vi "main4Ch_GainAtSameTime.vi"() -> ()   [LabVIEW 2024]
doc: "Main VI for FLS imaging system."
uses:
  <userlib>/_OpenG.lib/file/file.llb/openg_file.lvlib
  <vilib>/event_ctls.llb/usereventprio.ctl
  <instrlib>/niScope/Acquire/Fetch/niScope Multi Fetch Binary 16.vi
  <instrlib>/niScope/Controls/niScope trigger source.ctl
  <userlib>/_OpenG.lib/time/time.llb/openg_time.lvlib
  LaguerreDeconLib/DeconEngineClass/LaguerreDeconEngineClass.lvclass
  SubVI/GlobalVariables.vi
  SubVI/LabJack/LJ Pin Setting.ctl
  <vilib>/Utility/error.llb/DialogType.ctl
  <vilib>/Analysis/NI_AALBase.lvlib
  <vilib>/Utility/miscctls.llb/LVMinMaxIncTypeDef.ctl
  <vilib>/Analysis/baseanly.llb/Mean (DBL).vi
  <vilib>/Utility/miscctls.llb/LVPointTypeDef.ctl
  SubVI/APD/APDClass.lvclass
  ConfigFiles/AimingBeamVideoConfig.ctl
  <vilib>/addons/control/pid/NI_PID_pid.lvlib
  <vilib>/addons/control/pid/pid.llb/PID (DBL).vi
  <vilib>/Instr/_visa.llb/VISA Configure Serial Port (Instr).vi
  SubVI/DigitizerConfiguration/FLImDAQ.ctl
panel:
  out "Record Backlog 2":i32
  in  "Auto gain ch4":bool=TRUE caption="Auto gain ch3"
  in  "V 4":dbl caption="Gain 3" min=0.0 max=4.66 step=0.1
  out "Gain4":dbl
  out "Lifetime 4":dbl caption="Lifetime 3"
  out "IntR4":dbl format="%#_2g"
  out "SNR4":dbl format="%#_3g"
  out "Channel 4":dbl[][](graph) caption="Channel 3"
  out "RunStartTime":u32
  out "Dig1 Temp":dbl
  out "Dig2 Temp":dbl
  out "Visualization PC video source":T1
  in  "V target(1.0)":dbl=1.0 caption="V target(1.5)" min=0.3 max=1.5 step=0.1 format="%#_4g"
  out "SNR3":dbl format="%#_3g"
  out "SNR2":dbl format="%#_3g"
  out "SNR1":dbl format="%#_3g"
  in  "Show BG removed?":bool=TRUE
  out "IntR3":dbl format="%#_2g"
  out "IntR2":dbl format="%#_2g"
  out "IntR1":dbl format="%#_2g"
  in  "Video Display":bool
  out "Gain3":dbl
  out "Gain2":dbl
  out "Gain1":dbl
  in  "Skip Data Save?":bool
  out "Aq Loop?":bool
  out "ML?":bool
  out "aquisition loop Error Out":errorcluster
  out "Laser f (Hz)":dbl
  out "Record Backlog":i32
  out "Fetch Record #":i32
  out "Sync Success?":bool
  out "Disclamer":picture
  out "Calibration #":i8
  out "BG #":i8
  in  "TCP Connect":bool
  out "Help":string
  in  "355nm Laser toggle":bool caption="355nm 460Hz"
  in  "Cali&iRF alignment":bool
  in  "Background":bool
  in  "Aiming beam toggle":bool caption="445nm 15Hz 20mA"
  out "Lifetime 3":dbl
  out "Lifetime 2":dbl
  in  "Auto gain ch3":bool=TRUE
  in  "Auto gain ch2":bool=TRUE
  in  "Auto gain ch1":bool=TRUE
  out "Run #":i8
  in  "StopButton":bool caption="Stop"
  out "Aquisition Status:":bool
  in  "StartButton":bool caption="Start"
  in  "V 3":dbl caption="Gain 3" min=0.0 max=4.65 step=0.1
  in  "V 2":dbl caption="Gain 2" min=0.0 max=4.59 step=0.1
  out "Lifetime 1":dbl
  in  "V 1":dbl caption="Gain 1" min=0.0 max=4.63 step=0.1 format="%#_4g"
  in  "Video Source":enum32{"Camera", "FrameGrabber"}(radio)
  out "Case #":string
  out "System Hardware Connection Status":T2
  out "Channel 3":dbl[][](graph)
  out "Channel 2":dbl[][](graph)
  out "Channel 1":dbl[][](graph)
  in  "Tab Control":T3(tab)
  out "display loop timing(ms)":u32
  out "Aquisition loop timing(ms)":u32 format="%.2f"
  out "DisplayLoop":i32
  out "PID loop":i32 caption="processing loop"
  out "PID loop timing(ms)":u32 caption="processing loop timing(ms)"
  out "Communication loop(ms)":u32
  out "laser EM lamp V":dbl format="%0.6f"
  out "Decon Loop timing (ms)":dbl
  out "Auisition Loop idx":i32
  out "LJ process (ms)":u32
  out "LJ time(ms)":u32[](array[numeric])
  in  "Show BG":bool
  out "iRF length":i32
  out "BG length":i32
  out "data length":i32
  out "SysConfigCluster":T4
  out "LJ Pinout":T5={"Ch1 Bias"="DAC0", "Ch2 Bias"="DAC1", "Ch3 Bias"="DAC2", "Ch4 Bias"="DAC0", "355 PWM"="FIO0", "AimingBeam PWM"="FIO2", "Laser Ready"="FIO3", "Interlock"="FIO1", "Laser Start/Stop"="FIO1", "Red LED"="FIO1", "Green LED"="DIO3", "Foot Pedal"="DIO15"}
  out "FLImDAQ":T6={"Digitizer 1"="", "Digitizer 2"="", "Channel"=enum."Channel 0", "trigger source"="VAL_EXTERNAL", "trigger level"=0.5, "trigger delay"=1.35e-07, "min sample rate"=12500000000.0, "min record length"=2500, "vertical range"=1.0, "vertical offset"=-0.25, "Waveform to Avg"=2000} caption="FLIm DAQ Configuration" {"trigger delay" format="%^#.4e"; "trigger level" min=0.0 max=3.5 step=0.5 format="%.2f"; "vertical offset" format="%.4f"; "vertical range" format="%.2f"; "min sample rate" format="%#.2p"}
  in  "Sys Reconfig":bool
  out "data out(communcation loop)":string
  out "PID loop error out":errorcluster caption="processing Error Out"
  out "decon error out":errorcluster
  out "Laser Rep Rate":dbl
  out "V4 Size":i32 caption="V3 Size"
  in  "Data Class":enum16{"Data", "BG", "Cali"}(ring)
  out "V1 Size":i32
  out "V2 Size":i32
  out "V3 Size":i32
  out "data Size":i32[](array[numeric])
  out "State log":string
  in  "Ch4 PID gains":T8={"proportional gain (Kc)"=30.0, "integral time (Ti, min)"=0.0003, "derivative time (Td, min)"=1e-05}
  in  "Ch3 PID gains":T8={"proportional gain (Kc)"=30.0, "integral time (Ti, min)"=0.0003, "derivative time (Td, min)"=1e-05}
  in  "Ch2 PID gains":T8={"proportional gain (Kc)"=30.0, "integral time (Ti, min)"=0.0003, "derivative time (Td, min)"=1e-05}
  in  "Ch1 PID gains":T8={"proportional gain (Kc)"=30.0, "integral time (Ti, min)"=0.0003, "derivative time (Td, min)"=1e-05}
  in  "Quit":bool
  in  "Radio Buttons":T9(radio)=enum."Ch2" caption="DeCon Chan"
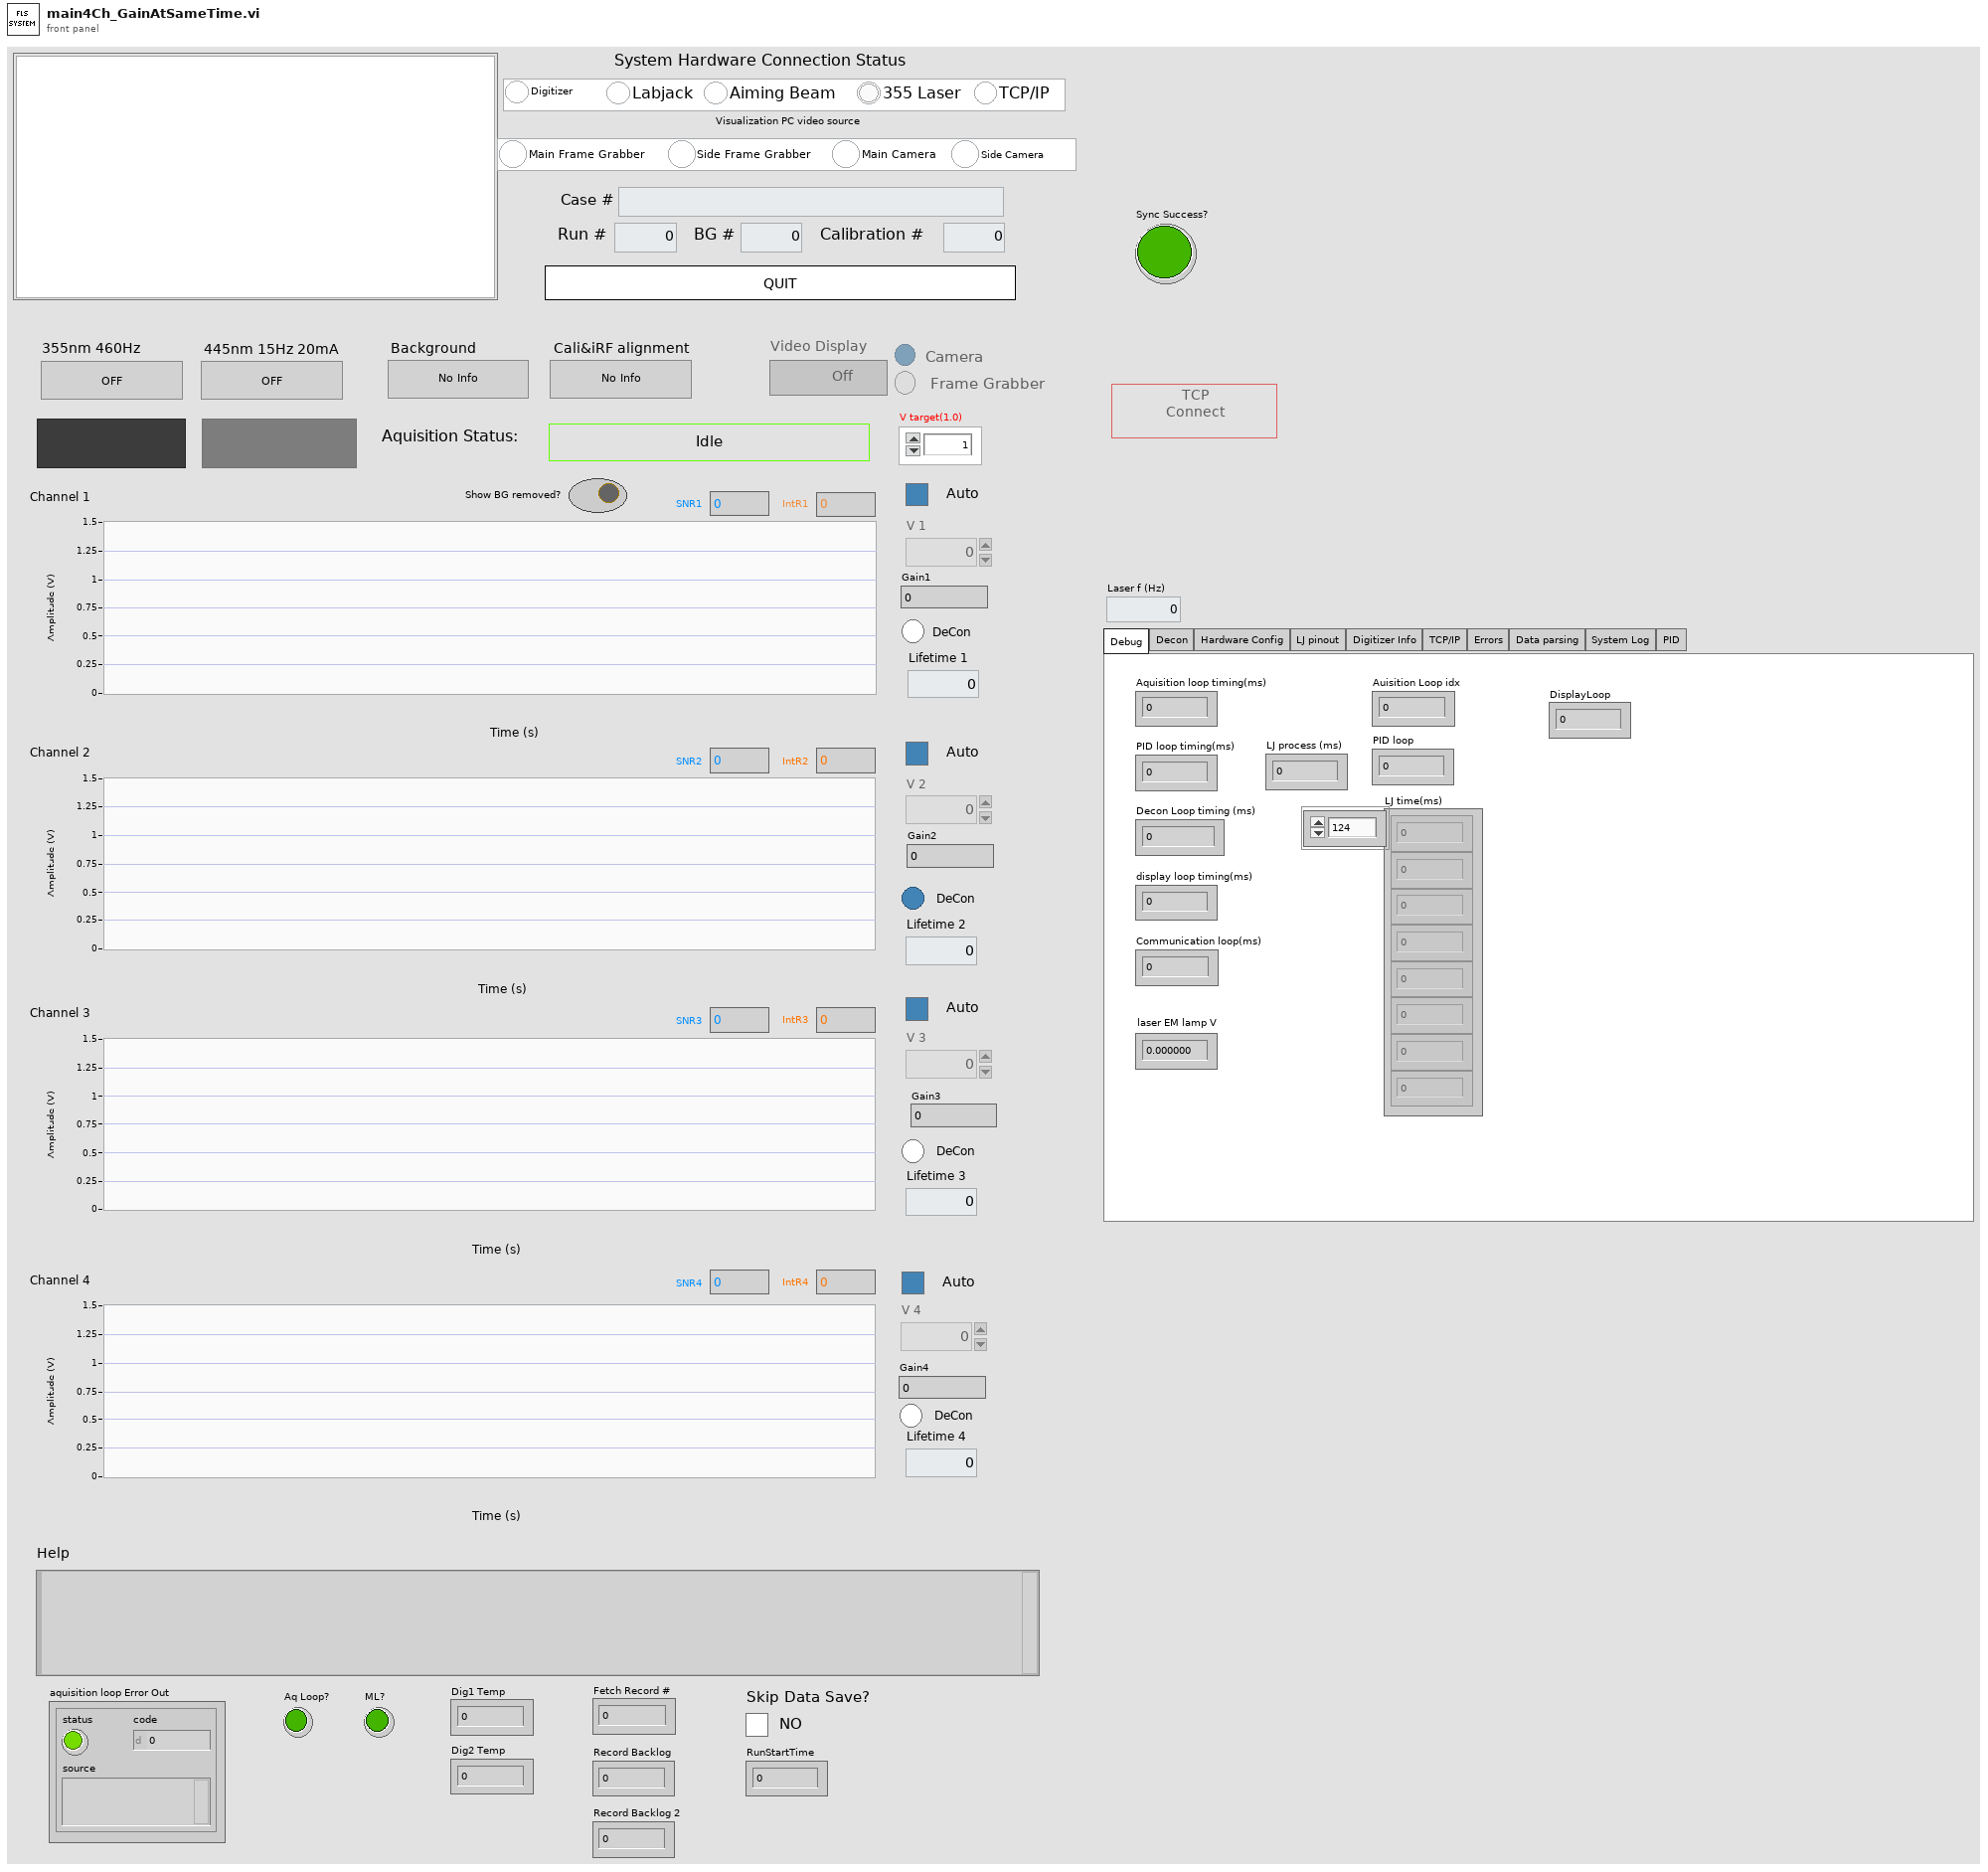
[diagram p1: front panel]
types:
  T1 = cluster{"Main Frame Grabber":bool, "Side Frame Grabber":bool, "Main Camera":bool, "Side Camera":bool}
  T2 = cluster{"Digitizer":bool, "Labjack":bool, "Aiming Beam":bool, "355 Laser":bool, "TCP/IP":bool}
  T3 = enum32{"Debug", "Decon", "Hardware Config", "LJ pinout", "Digitizer Info", "TCP/IP", "Errors", "Data parsing", "System Log", "PID"}
  T4 = cluster{"Ch1Enable?":bool, "Ch2Enable?":bool, "Ch3Enable?":bool, "Ch1AutoGain?":bool, "Ch2AutoGain?":bool, "Ch3AutoGain?":bool, "AimingBeamEnable?":bool}
  T5 = typedef "LJ Pin Setting.ctl" = cluster{"Ch1 Bias":string, "Ch2 Bias":string, "Ch3 Bias":string, "Ch4 Bias":string, "355 PWM":string, "AimingBeam PWM":string, "Laser Ready":string, "Interlock":string, "Laser Start/Stop":string, "Red LED":string, "Green LED":string, "Foot Pedal":string}
  T6 = typedef "FLImDAQ.ctl" = cluster{"Digitizer 1":refnum<k15>, "Digitizer 2":refnum<k15>, "Channel":enum16{"Channel 0", "Channel 1", "Channel 0&1"}, "trigger source":T7, "trigger level":dbl, "trigger delay":dbl, "min sample rate":dbl, "min record length":i32, "vertical range":dbl, "vertical offset":dbl, "Waveform to Avg":i16}
  T7 = typedef "niScope trigger source.ctl" = string
  T8 = cluster{"proportional gain (Kc)":dbl, "integral time (Ti, min)":dbl, "derivative time (Td, min)":dbl}
  T9 = enum32{"No Selection", "Ch1", "Ch2", "Ch3", "Ch4"}
  T10 = cluster{"remote start event":refnum<user-event>, "remote stop  event":refnum<user-event>}
  T11 = enum8{"Enabled", "Disabled", "Disabled and Grayed Out"}
  T12 = enum16{"open", "replace", "create", "open or create", "replace or create", "replace or create with confirmation"}
  T13 = cluster{"CH1":dbl[][], "CH2":dbl[][], "CH3":dbl[][], "CH4":dbl[][], "Gain cluster":cluster{"V1":dbl, "V2":dbl, "V3":dbl, "V4":dbl}}
  T14 = cluster{"idx":i32, "CH1&2":dbl[][], "CH3":dbl[][], "V cluster":cluster{"V1":dbl, "V2":dbl, "V3":dbl, "V4":dbl}}
  T15 = cluster{"Ch1 iRF":dbl[], "Ch2 iRF":dbl[], "Ch3 iRF":dbl[], "Ch4 iRF":dbl[]}
  T16 = enum16{"open", "open or create", "create or replace", "create", "open (read-only)"}
  T17 = enum32{"Invalid", "Standard", "Closed", "Hidden", "Minimized", "Maximized"}
  T18 = enum32{"invalid app kind", "Development System", "Run Time System", "Student Edition", "Embedded LabVIEW", "Evaluation", "Custom"}
  T19 = typedef "usereventprio.ctl" = enum32{"high priority", "normal priority"}
  T20 = enum32{"Bad", "Idle", "Run top level", "Running"}
  T21 = enum16{"Standard", "Buffered", "CRLF", "Immediate"}
  T22 = typedef "AimingBeamVideoConfig.ctl" = cluster{"DeCon Channel":enum16{"1", "2", "3"}, "Scale Bar":bool, "Scale Low":dbl, "Scale High":dbl, "ANSI":dbl, "Radius":dbl, "3D?":bool, "Firefly?":bool, "Pentero?":bool}
  T23 = cluster{"Core":cluster{"Current VI Reference":refnum<vi>, "Close Panel on Exit?":bool}, "SysConfigCluster":cluster{"Ch1Enable?":bool, "Ch2Enable?":bool, "Ch3Enable?":bool, "Ch1AutoGain?":bool, "Ch2AutoGain?":bool, "Ch3AutoGain?":bool, "AimingBeamEnable?":bool}, "System Status":cluster{"Digitizer":bool, "Labjack":bool, "Aiming Beam":bool, "355 Laser":bool, "TCP/IP":bool}, "IDs":cluster{"RunID":i8, "BG ID":i8, "Cali ID":i8}, "CaseID":string, "DefaultPath":path, "Pathes":cluster{"DataPath":path, "BG Path":path, "iRFPath":path, "CaliPath":path}, "FLImDAQ":cluster{"resource name":refnum<k15>, "resource name 2":refnum<k15>, "Channel":enum16{"Channel 0", "Channel 1", "Channel 0&1"}, "trigger source":T7, "trigger level":dbl, "trigger delay":dbl, "min sample rate":dbl, "min record length":i32, "vertical range":dbl, "vertical offset":dbl, "Waveform to Avg":i32}, "SysRunning?":bool, "AB Cluster":cluster{"Aiming Beam COM Port":refnum<visa-resource-name>, "Min Current":dbl, "Max Current":dbl, "Default Current":dbl, "Freq":i32}, "LJ Pinout":T5, "355 PWM setting":cluster{"DIO_EF_CLOCK1_DIVISOR":i16, "DIO_EF_CLOCK1_ROLL_VALUE":i32, "DIO#_EF_INDEX":i16, "DIO#_EF_OPTIONS":i16, "DIO#_EF_CONFIG_A":i32}, "AB PWM setting":cluster{"DIO_EF_CLOCK1_DIVISOR":i16, "DIO_EF_CLOCK1_ROLL_VALUE":i32, "DIO#_EF_INDEX":i16, "DIO#_EF_OPTIONS":i16, "DIO#_EF_CONFIG_A":i32}, "Last Trigger":u32, "niTClk sessions":refnum<k20>[], "Laser start tic":u32, "TCP attempt count":i32, "Ch1Data":dbl[][], "Ch2Data":dbl[][], "Ch3Data":dbl[][], "Ch4Data":dbl[][], "V1":dbl[], "V2":dbl[], "V3":dbl[], "V4":dbl[], "SlowTimer":u32, "FastTimer":u32, "listener ID":refnum<k5>, "TempPath":path, "CaliPath":path, "LED vi reference":refnum<vi>, "Aquisition Timer":u32, "APDSerialNum":cluster{"Ch1APDSerial#":string, "Ch2APDSerial#":string, "Ch3APDSerial#":string, "Ch4APDSerial#":string}, "VideoConfig":T22, "LED vi ref open?":bool, "video source":cluster{"Main Frame Grabber":bool, "Side Frame Grabber":bool, "Main Camera":bool, "Side Camera":bool}, "bothVidSourceAvail":bool}
  T24 = typedef "LVCursorListTypeDef.ctl" = cluster{"Name":string, "Color":u32, "Style":u8, "Point Style":u8, "Name Visible":bool, "Allow Drag":bool, "Cursor Mode":u32, "Plot":i32, "Index":i32, "Position":cluster{"X":dbl, "Y":dbl}, "X Scale":u32, "Y Scale":u32, "Watch Plots":i32[], "Watch All Plots":bool, "Plot Area":i32, "Label Offset":cluster{"X":dbl, "Y":dbl}}[]
  T25 = cluster{"Name":string, "Color":u32, "Style":u8, "Point Style":u8, "Name Visible":bool, "Allow Drag":bool, "Cursor Mode":u32, "Plot":i32, "Index":i32, "Position":cluster{"X":dbl, "Y":dbl}, "X Scale":u32, "Y Scale":u32, "Watch Plots":i32[], "Watch All Plots":bool, "Plot Area":i32, "Label Offset":cluster{"X":dbl, "Y":dbl}}
  T26 = cluster{"Ch1APDSerial#":string, "Ch2APDSerial#":string, "Ch3APDSerial#":string, "Ch4APDSerial#":string}
  T27 = cluster{"DataPath":path, "BG Path":path, "iRFPath":path, "CaliPath":path}
  T28 = cluster{"DIO_EF_CLOCK1_DIVISOR":i16, "DIO_EF_CLOCK1_ROLL_VALUE":i32, "DIO#_EF_INDEX":i16, "DIO#_EF_OPTIONS":i16, "DIO#_EF_CONFIG_A":i32}
  T29 = cluster{"Aiming Beam COM Port":refnum<visa-resource-name>, "Min Current":dbl, "Max Current":dbl, "Default Current":dbl, "Freq":i32}
  T30 = cluster{"resource name":refnum<k15>, "resource name 2":refnum<k15>, "Channel":enum16{"Channel 0", "Channel 1", "Channel 0&1"}, "trigger source":T7, "trigger level":dbl, "trigger delay":dbl, "min sample rate":dbl, "min record length":i32, "vertical range":dbl, "vertical offset":dbl, "Waveform to Avg":i32}
  T31 = cluster{"Current VI Reference":refnum<vi>, "Close Panel on Exit?":bool}
  T32 = typedef "iRFData.ctl" = cluster{"dt":dbl, "NumOfWFs":i32, "WFLength":i32, "iRFCtrlV":dbl[], "iRFWFsAvg":dbl[][], "iRFRaw":dbl[][]}
  T33 = cluster{"V 1":dbl[], "V 2":dbl[], "V 3":dbl[], "V 4":dbl[]}
  T34 = cluster{"Channel 1":dbl[], "Channel 2":dbl[], "Channel 3":dbl[], "Channel 4":dbl[]}
  T35 = cluster{"Ch1 WF":dbl[], "Ch2 WF":dbl[], "Ch3 WF":dbl[], "Ch4 WF":dbl[], "V1":dbl, "V2":dbl, "V3":dbl, "V4":dbl}
  T36 = cluster{"mean":dbl, "mean":dbl, "mean":dbl, "mean":dbl}
  T37 = cluster{"V1":dbl, "V2":dbl, "V3":dbl, "V4":dbl}[]
  T38 = cluster{"DataPath":path, "CaseID":string, "RunID":i16, "Ch1Data":dbl[][], "Ch2Data":dbl[][], "Ch3Data":dbl[][], "Ch4Data":dbl[][], "V1":dbl[], "V2":dbl[], "V3":dbl[], "V4":dbl[], "LaserRepRate":u16, "WFAverage":i16, "RunStartTime":u64}
  T39 = typedef "DialogType.ctl" = u16
  T40 = typedef "LJ PWM Setting.ctl" = cluster{"DIO_EF_CLOCK1_DIVISOR":i16, "DIO_EF_CLOCK1_ROLL_VALUE":i32, "DIO#_EF_INDEX":i16, "DIO#_EF_OPTIONS":i16, "DIO#_EF_CONFIG_A":i32}
  T41 = typedef "AimingBeam.ctl" = cluster{"Aiming Beam COM Port":refnum<visa-resource-name>, "Min Current":dbl, "Max Current":dbl, "Default Current":dbl, "Frequency(Hz)":u32}
  T42 = cluster{"DC1":i32, "DC2":i32, "BG1":i32, "BG2":i32}
  T43 = typedef "LVMinMaxIncTypeDef.ctl" = cluster{"Minimum":dbl, "Maximum":dbl, "Increment":dbl}
  T44 = typedef "LVBoundsTypeDef.ctl" = cluster{"Width":u32, "Height":u32}
  T45 = typedef "imagedata.ctl" = cluster{"image type":i32, "image depth":i32, "image":u8[], "mask":u8[], "colors":u32[], "Rectangle":cluster{"left":i16, "top":i16, "right":i16, "bottom":i16}}
  T46 = cluster{"DC Idx1":i32, "DC Idx2":i32, "BG Idx1":i32, "BG Idx2":i32}
  T47 = cluster{dbl[][], dbl[][], dbl[][], dbl[][], "V cluster":cluster{"V1":dbl, "V2":dbl, "V3":dbl, "V4":dbl}}
  T48 = typedef "LVPointTypeDef.ctl" = cluster{"Horizontal":i16, "Vertical":i16}
  T49 = cluster{"actualSamples":i32, "absoluteInitialX":dbl, "relativeInitialX":dbl, "xIncrement":dbl, "offset":dbl, "gain":dbl, "reserved1":dbl, "reserved2":dbl}[]
  T50 = cluster{"V1 out":dbl, "V2 out":dbl, "V3 out":dbl, "V3 out":dbl}
  T51 = cluster{i32, dbl[][], dbl[][], cluster{"V1 out":dbl, "V2 out":dbl, "V3 out":dbl, "V3 out":dbl}}
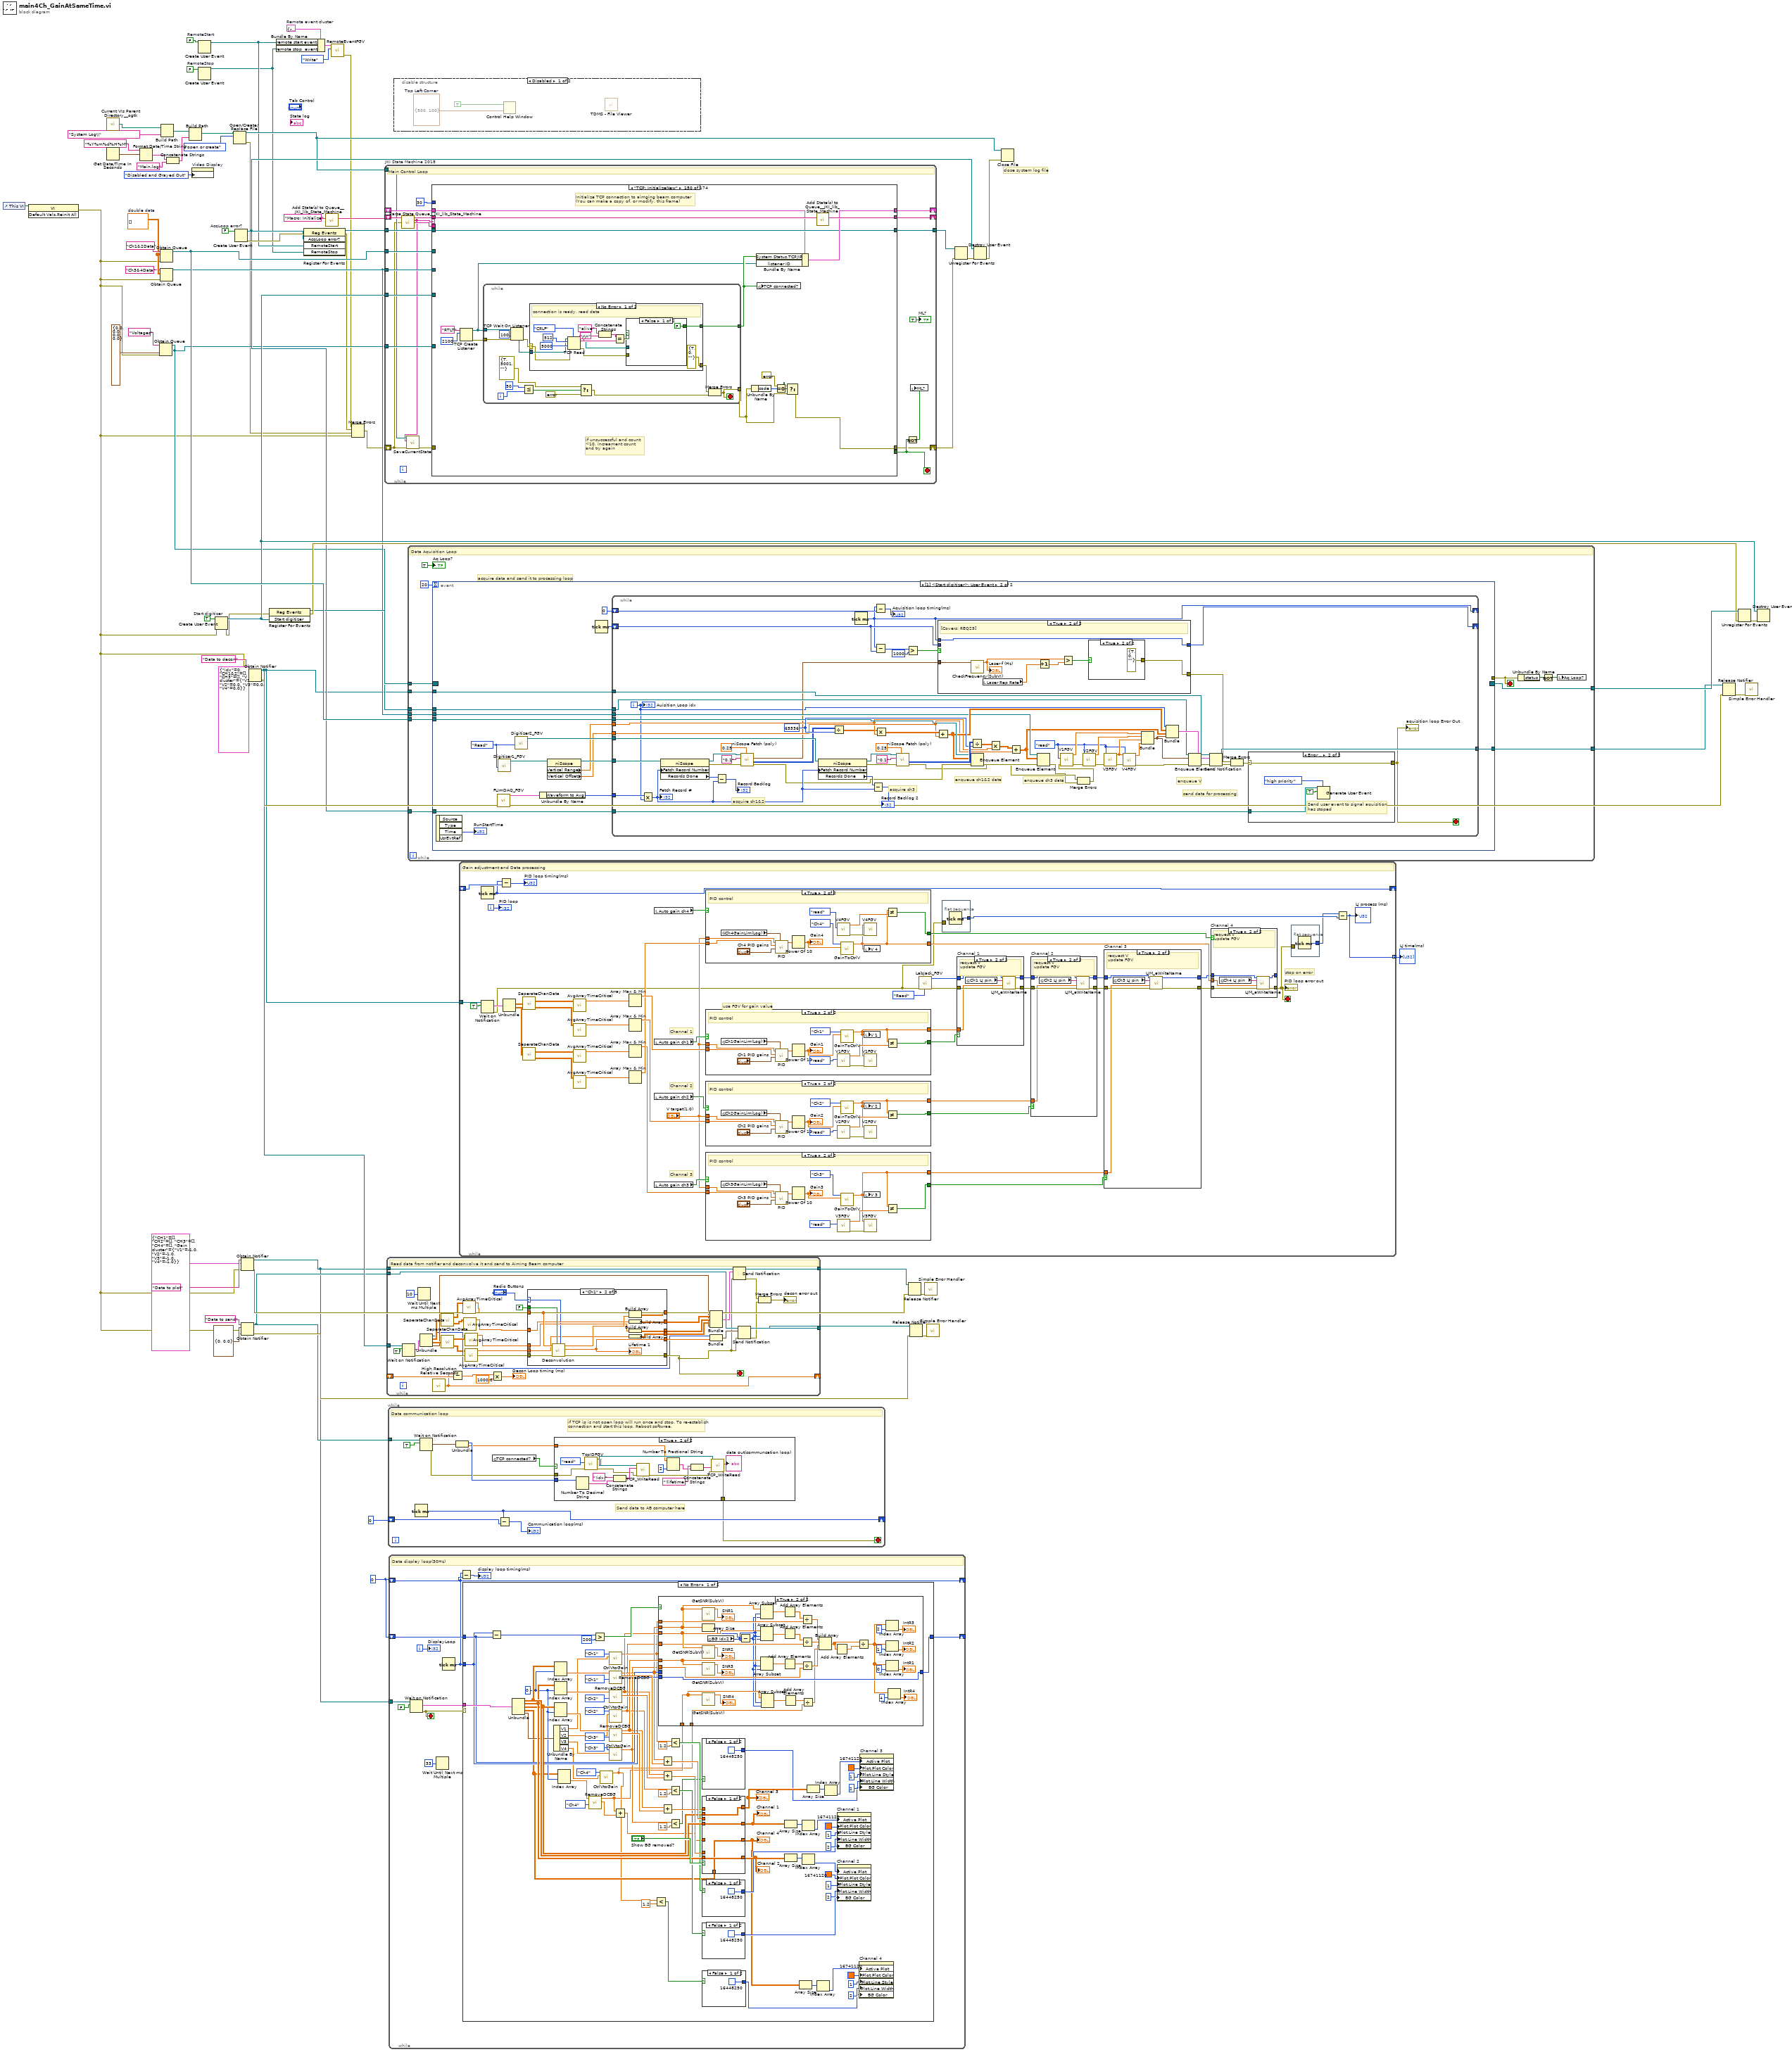
[diagram p0: block diagram]
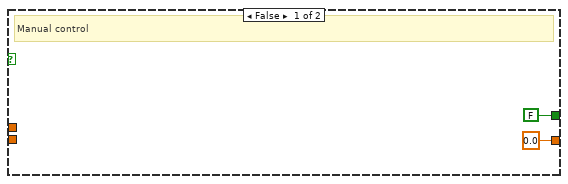
[diagram p6: hidden frame]
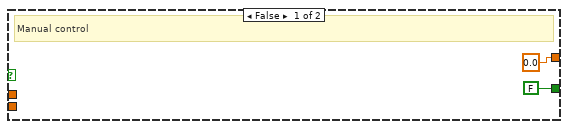
[diagram p7: hidden frame]
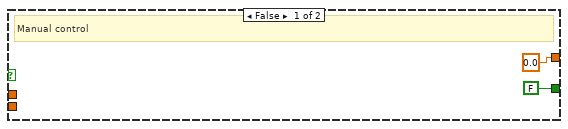
[diagram p8: hidden frame]
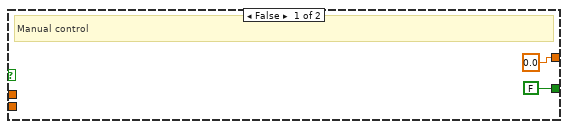
[diagram p9: hidden frame]
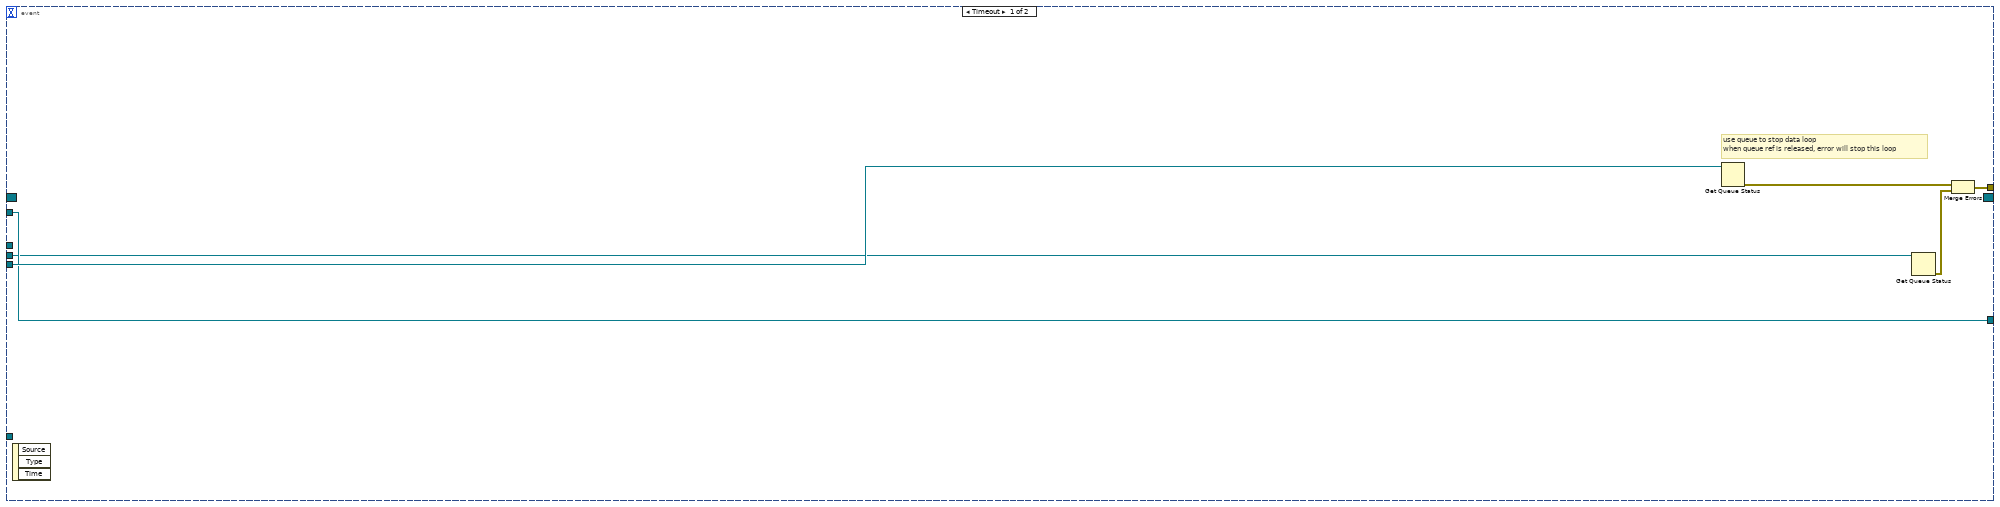
[diagram p10: hidden frame]
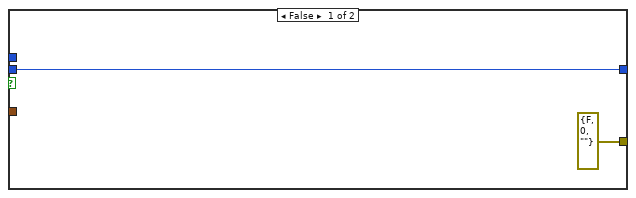
[diagram p11: hidden frame]
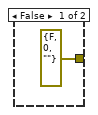
[diagram p12: hidden frame]
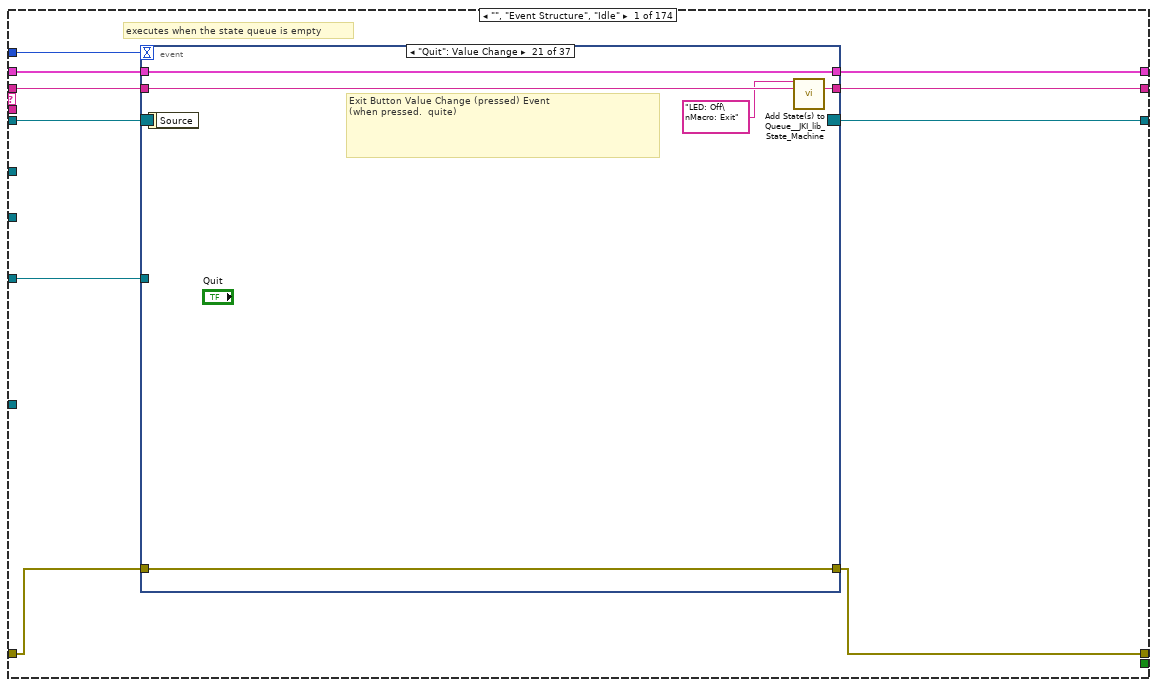
[diagram p14: hidden frame]
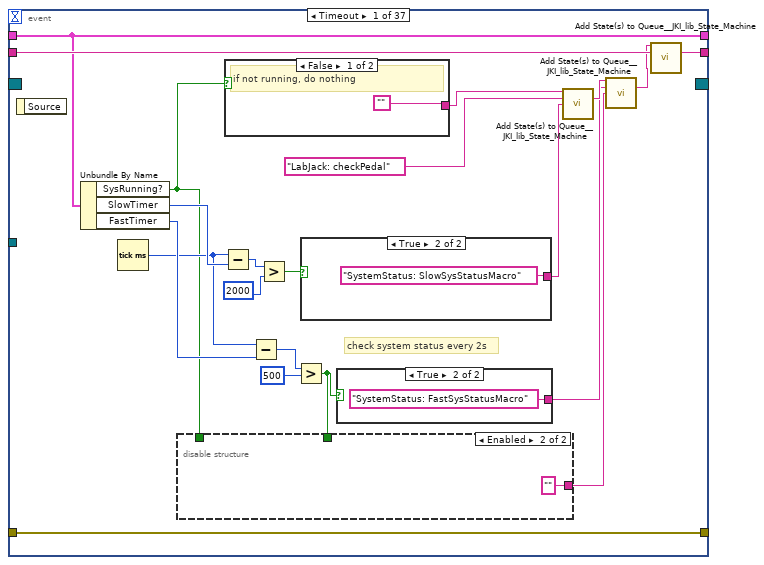
[diagram p15: hidden frame]
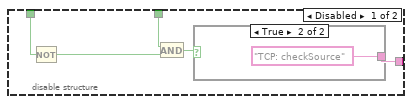
[diagram p16: hidden frame]
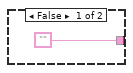
[diagram p17: hidden frame]
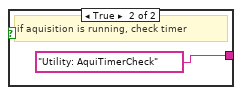
[diagram p18: hidden frame]
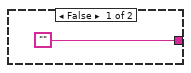
[diagram p19: hidden frame]
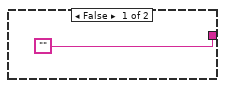
[diagram p20: hidden frame]
diagram:
  w8 = T10 {"remote start event"=refnum, "remote stop  event"=refnum}  # Remote event cluster
  w11 = FALSE  # RemoteStop
  w12 = FALSE  # RemoteStart
  w15 = u32 0 ("millisecond timer value")
  w54 = FALSE  # AcqLoop error?
  w64 = TRUE  # Start digitizer
  w67 = dbl[][] []  # double data
  # "close system log file"
  n1 = control-ref of="This VI"() -> (w69:refnum<vi>)
  n2 = invoke on="Invoke Node" class="VI" method="Default Vals.Reinit All"(reference=w69) -> (error out=w23:errorcluster)  [unwired: 2 in, 2 out]
  n3 = call <userlib>:"Current VIs Parent Directory__ogtk.vi"() -> ("Parent Directory (+ Relative)"=w34:path)  [unwired: 5 in]
  n4 = Get Date/Time In Seconds() -> (seconds since 1Jan1904=w32:timestamp)
  n5 = Format Date/Time String(time format string (%c)="%Y%m%d%H%M", seconds (now)=w32) -> (date/time string=w29:string)  [unwired: 1 in]
  n6 = Obtain Queue(name (unnamed)="Voltages", element data type=cluster{"V1":dbl, "V2":dbl, "V3":dbl, "V4":dbl} {"V1"=0.0, "V2"=0.0, "V3"=0.0, "V4"=0.0}, error in (no error)=w23) -> (queue out=w35:refnum<queue>)  [unwired: 2 in, 2 out]
  n7 = Obtain Queue(name (unnamed)="Ch3&4Data", element data type=w67, error in (no error)=w23) -> (queue out=w48:refnum<queue>)  [unwired: 2 in, 2 out]
  n8 = Obtain Queue(name (unnamed)="Ch1&2Data", element data type=w67, error in (no error)=w23) -> (queue out=w65:refnum<queue>)  [unwired: 2 in, 2 out]
  n9 = Build Path(base path=w34, name or relative path="System Log\\") -> (appended path=w25:path)
  n10 = Concatenate Strings(w29, "Main.log" ("string")) -> (w27:string)
  n11 = Build Path(base path=w25, name or relative path=w27) -> (appended path=w30:path)
  n12 = property on="Video Display" class="Bool (strict)"("DisabledEnum"=T11."Disabled and Grayed Out" ("Disabled")) -> ()  [unwired: 2 in, 2 out]
  n13 = Create User Event(user event datatype=w12) -> (user event=w10:refnum<user-event>)  [unwired: 1 in, 1 out]
  n14 = Create User Event(user event datatype=w11) -> (user event=w9:refnum<user-event>)  [unwired: 1 in, 1 out]
  n15 = Create User Event(user event datatype=w64, error in=w23) -> (user event=w53:refnum<user-event>, error out=w40:errorcluster)
  n16 = Open/Create/Replace File(file path (use dialog)=w30, operation (0:open)=T12."open or create") -> (refnum out=w21:refnum<file>, error out=w22:errorcluster)  [unwired: 4 in, 1 out]
  n17 = Create User Event(user event datatype=w54) -> (user event=w39:refnum<user-event>, error out=w41:errorcluster)  [unwired: 1 in]
  n18 = Obtain Notifier(name (unnamed)="Data to plot", notification data type=T13 {"CH1"=[], "CH2"=[], "CH3"=[], "CH4"=[], "Gain cluster"={"V1"=-1.0, "V2"=-1.0, "V3"=-1.0, "V4"=-1.0}}, error in (no error)=w23) -> (notifier out=w13:refnum<notifier>, error out=w49:errorcluster)  [unwired: 1 in, 1 out]
  n19 = Obtain Notifier(name (unnamed)="Data to send", notification data type=cluster{"idx":i32, "lifetime":dbl} {"idx"=0, "lifetime"=0.0}, error in (no error)=w23) -> (notifier out=w18:refnum<notifier>, error out=w38:errorcluster)  [unwired: 1 in, 1 out]
  n20 = Obtain Notifier(name (unnamed)="Data to decon", notification data type=T14 {"idx"=0, "CH1&2"=[], "CH3"=[], "V cluster"={"V1"=0.0, "V2"=0.0, "V3"=0.0, "V4"=0.0}}, error in (no error)=w23) -> (notifier out=w19:refnum<notifier>, error out=w58:errorcluster)  [unwired: 1 in, 1 out]
  n21 = register-events(error in=w40, w53) -> (reference out=w55:refnum<event-registration>, error out=w61:errorcluster)  [unwired: 1 in]
  n22 = Bundle By Name(cluster=w8, "remote start event"=w10, "remote stop  event"=w9) -> (w6:T10)
  n23 = register-events(error in=w41, w39, w10, w9) -> (reference out=w47:refnum<event-registration>, error out=w5:errorcluster)  [unwired: 1 in]
  n24 = call <vilib>:"Add State(s) to Queue__JKI_lib_State_Machine.vi"("State(s) in (\"\")"="Macro: Initialize") -> ("States Out"=w71:string)  [unwired: 14 in]
  n25 = call "RemoteEventFGV.vi"("Operation (Read)"=enum16{"Read", "Write"}."Write", "Remote Event in"=w6) -> ("Error Out"=w2:errorcluster)  [unwired: 8 in, 1 out]
  n26 = Merge Errors(w2, w5, w22, w23) -> (w24:errorcluster)
  n27 = while "JKI State Machine 2018" {
    shift-right: [w88] -> _
    shift-left: _ -> [w87]
    shift-right: [w72] -> w4
    shift-left: w24 -> [w74]
    shift-right: [w89] -> _
    shift-left: w71 -> [w90]
    tunnel: w65 -> [w85]
    tunnel: w48 -> [w84]
    tunnel: w53 -> [w83]
    tunnel: w47 -> [w82]
    tunnel: [w81] -> w46
    tunnel: w35 -> [w77]
    tunnel: w21 -> [w76]
    stop <- w80 stop-if-true
    # "Main Control Loop"
    n28 = call <vilib>:"Parse State Queue__JKI_lib_State_Machine.vi"("State Queue"=w90, "Error In (no error)"=w74) -> ("Remaining States"=w92:string, "Current State"=w75:string, "Arguments"=w91:string)  [unwired: 11 in]
    n29 = call "SaveCurrentState.vi"("error in (no error)"=w74, "Current State"=w75, "Byte Stream File in"=w76) -> ("error out"=w73:errorcluster)  [unwired: 8 in]
    n30 = case shown="\"TCP: InitializeNew\"" w75 {
      selector: w75 -> [_ _ _ _ _ _ _ _ _ _ _ _ _ _ _ _ _ _ _ _ _ _ _ w1018 _ _ _ _ _ _ _ _ _ _ _ _ _ _ _ _ _ _ _ _ _ _ _ _ _ _ _ _ _ _ _ _ _ _ _ _ _ _ _ _ _ _ _ _ _ _ _ _ _ _ _ _ _ _ _ _ _ _ _ _ _ _ _ _ _ _ _ _ _ _ _ _ _ _ _ _ _ _ _ _ _ _ _ _ _ _ _ _ _ _ _ _ _ _ _ _ _ _ _ _ _ _ _ _ _ _ _ _ _ _ _ _ _ _ _ _ _ _ _ _ _ _ _ _ _ _ _ _ _ _ _ _ _ _ _ _ _ _ _ _ _ _ _ _ _ _ _ _ _ _]
      tunnel: w92 -> [w102 w478 w487 w493 w499 w521 w534 w576 w620 w635 w665 w708 w721 w748 w780 w794 w823 w837 w922 w959 w998 w1011 w1016 w1022 w1049 w1057 w1080 w1085 w1098 w1117 w1145 w1173 w1211 w1216 w1222 w1248 w1274 w1300 w1326 w1331 w1348 w1395 w1417 w1433 w1448 w1468 w1473 w1485 w1514 w1540 w1552 w1590 w1603 w1609 w1620 w1632 w1663 w1676 w1690 w1705 w1724 w1759 w1764 w1778 w1788 w1804 w1816 w1828 w1856 w1871 w1876 w1887 w1899 w1904 w1912 w1920 w1929 w1938 w1943 w1951 w1960 w1978 w1995 w2015 w2026 w2048 w2063 w2080 w2085 w2093 w2101 w2106 w2114 w2121 w2129 w2136 w2146 w2174 w2182 w2189 w2197 w2202 w2210 w2217 w2223 w2232 w2248 w2253 w2260 w2272 w2342 w2354 w2363 w2380 w2389 w2412 w2429 w2440 w2453 w2478 w2501 w2507 w2523 w2545 w2553 w2559 w2564 w2571 w2581 w2593 w2602 w2607 w2619 w2624 w2634 w2640 w2646 w2651 w2656 w2661 w2671 w2693 w2712 w2717 w2728 w2753 w2780 w2803 w2808 w2823 w2874 w2920 w2965 w2976 w2994 w3014 w3028 w3041 w3049 w3066 w3088 w3112 w3131 w3149 w3167 w3185 w3199 w3213 w3232 w3246 w3261 w3276 w3285 w3290]
      tunnel: w91 -> [_ _ _ _ _ _ _ _ _ _ _ _ _ _ _ _ _ _ _ _ _ _ _ _ _ _ _ _ _ _ _ _ _ _ _ _ _ _ _ _ _ _ _ _ _ _ _ _ _ _ _ _ _ _ _ w1630 _ _ _ _ _ _ _ _ _ _ _ _ _ _ _ _ _ _ _ _ _ _ _ _ _ _ _ _ _ _ _ _ _ _ _ _ _ _ _ _ w2137 _ _ _ _ _ _ _ _ _ _ _ w2255 w2266 _ _ _ _ w2386 _ _ _ _ _ w2497 _ _ _ _ _ _ w2566 _ _ _ _ _ _ w2630 _ _ _ _ _ _ _ _ _ _ _ _ _ _ _ _ _ _ _ _ _ _ _ _ _ _ _ _ _ _ _ _ _ _ _ _ _ _ _]
      tunnel: w87 -> [w100 w475 w483 w490 w496 w518 w531 _ w617 w625 w661 w704 w717 w740 w771 w791 w820 w834 w882 w951 w986 w1006 w1013 w1020 w1042 w1054 w1078 w1082 w1086 w1107 w1137 w1165 w1207 w1213 w1219 w1226 w1253 w1279 w1305 w1328 w1341 w1385 w1414 w1418 w1445 w1465 w1470 w1474 w1503 w1530 w1545 w1573 w1601 w1606 w1613 w1628 w1646 w1671 w1682 w1700 w1717 w1742 w1761 w1774 w1782 w1801 w1813 w1825 w1844 w1860 w1873 w1885 w1897 w1901 w1906 w1913 w1925 w1934 w1940 w1947 w1957 w1965 w1982 w2010 w2016 w2045 w2056 w2078 w2082 w2086 w2094 w2103 w2112 w2118 w2126 w2133 w2143 w2171 w2179 w2186 w2194 w2199 w2204 w2215 w2220 w2226 w2245 w2250 w2258 w2268 w2339 w2344 w2357 w2378 w2387 w2402 w2426 w2437 w2447 w2471 w2498 w2504 w2516 w2541 w2550 w2556 w2561 w2568 w2575 w2589 w2599 w2604 w2616 w2621 w2627 w2637 w2643 w2648 w2653 w2658 w2668 w2691 w2710 w2714 w2726 w2751 w2778 w2801 w2805 w2816 w2868 w2916 w2962 w2972 w2989 w3009 w3023 w3037 w3043 w3061 w3083 w3107 w3126 w3144 w3162 w3180 w3194 w3208 w3227 w3241 w3256 w3273 w3283 w3287]
      tunnel: [w93 w476 w485 w491 w497 w519 w532 w574 w586 w633 w657 w700 w719 w728 w760 w784 w811 w835 w858 w948 w985 w1007 w1014 w1024 w1046 errorcluster {"status"=FALSE, "code"=0, "source"=""} ("error out") w1077 w1083 w1096 w1115 w1129 w1152 w1209 w1214 w1220 w1227 w1254 w1280 w1306 w1329 w1332 w1377 w1408 w1422 w1446 w1456 w1471 w1477 w1501 w1529 w1544 w1560 w1595 w1607 w1618 w1622 w1637 w1666 w1678 w1696 w1716 w1733 w1762 w1766 w1784 w1799 w1811 w1823 w1846 w1861 w1874 w1877 w1894 w1902 w1910 w1918 w1922 w1931 w1941 w1944 w1953 w1968 w1990 w2009 w2020 w2038 w2060 w2076 w2083 w2091 w2099 w2104 w2111 w2119 w2127 w2134 w2144 w2172 w2180 w2187 w2195 w2200 w2208 w2214 w2221 w2229 w2246 w2251 w2256 w2269 w2340 w2348 w2360 w2370 w2383 w2403 w2427 w2436 w2449 w2473 w2499 w2505 w2513 w2535 w2551 w2557 w2562 w2569 w2579 w2591 w2600 w2605 w2617 w2622 w2632 w2638 w2644 w2649 w2654 w2659 w2669 w2681 w2703 w2715 w2719 w2738 w2770 w2795 w2806 w2810 w2869 w2917 w2963 w2971 w2991 w3011 w3025 w3039 w3045 w3063 w3085 w3109 w3128 w3146 w3164 w3182 w3196 w3210 w3229 w3243 w3257 w3274 w3281 w3288] -> w72
      tunnel: w73 -> [w99 w476 w485 w491 w497 w519 w532 w574 w586 w633 w655 w701 w719 w729 w767 w784 w801 w835 w858 w949 w988 w1008 w1014 w1023 w1046 w1050 w1077 w1083 w1096 w1115 w1128 w1164 w1209 w1214 w1220 w1231 w1258 w1284 w1310 w1329 w1339 w1380 w1407 w1421 w1446 w1458 w1471 w1476 w1502 w1520 w1550 w1571 w1594 w1607 w1615 w1625 w1636 w1665 w1681 w1695 w1715 w1732 w1762 w1772 w1785 w1798 w1810 w1822 w1845 w1862 w1874 w1881 w1889 w1902 w1910 w1918 w1921 w1930 w1941 w1945 w1954 w1973 w1989 w2008 w2019 w2044 w2059 w2075 w2083 w2091 w2099 w2104 w2111 w2119 w2127 w2134 w2144 w2172 w2180 w2187 w2195 w2200 w2208 w2214 w2221 w2229 w2246 w2251 w2257 w2270 w2340 w2349 w2359 w2366 w2382 w2404 w2427 w2436 w2444 w2476 w2499 w2505 w2518 w2534 w2551 w2557 w2562 w2569 w2579 w2591 w2600 w2605 w2617 w2622 w2632 w2638 w2644 w2649 w2654 w2659 w2669 w2680 w2702 w2715 w2718 w2737 w2760 w2786 w2806 _ w2870 w2917 w2963 w2970 w2990 w3010 w3024 w3039 w3044 w3062 w3084 w3108 w3127 w3145 w3163 w3181 w3195 w3209 w3228 w3242 w3255 w3274 w3280 w3288]
      tunnel: [w101 w477 w486 w492 w498 w520 w533 w575 w619 w634 w664 w707 w720 w747 w779 w793 w822 w836 w921 w958 w997 w1010 w1015 w1021 w1048 w1056 w1079 w1084 w1097 w1116 w1144 w1172 w1210 w1215 w1221 w1247 w1273 w1299 w1325 w1330 w1347 w1394 w1416 w1432 w1447 w1467 w1472 w1484 w1513 w1539 w1551 w1589 w1602 w1608 w1619 w1631 w1662 w1675 w1689 w1704 w1723 w1758 w1763 w1777 w1787 w1803 w1815 w1827 w1855 w1870 w1875 w1886 w1898 w1903 w1911 w1919 w1928 w1937 w1942 w1950 w1959 w1977 w1994 w2014 w2025 w2047 w2062 w2079 w2084 w2092 w2100 w2105 w2113 w2120 w2128 w2135 w2145 w2173 w2181 w2188 w2196 w2201 w2209 w2216 w2222 w2231 w2247 w2252 w2259 w2271 w2341 w2353 w2362 w2379 w2388 w2411 w2428 w2439 w2452 w2477 w2500 w2506 w2522 w2544 w2552 w2558 w2563 w2570 w2580 w2592 w2601 w2606 w2618 w2623 w2633 w2639 w2645 w2650 w2655 w2660 w2670 w2692 w2711 w2716 w2727 w2752 w2779 w2802 w2807 w2822 w2873 w2919 w2964 w2975 w2993 w3013 w3027 w3040 w3048 w3065 w3087 w3111 w3130 w3148 w3166 w3184 w3198 w3212 w3231 w3245 w3260 w3275 w3284 w3289] -> w89
      tunnel: [_ _ _ _ _ _ _ _ _ _ _ _ _ _ _ _ _ _ _ _ _ _ _ _ _ _ TRUE _ _ _ _ _ _ _ _ _ _ _ _ _ _ _ _ _ _ _ _ _ _ _ _ _ _ _ _ _ _ _ _ _ _ _ _ _ _ _ _ _ _ _ _ _ _ _ _ _ _ _ _ _ _ _ _ _ _ _ _ _ _ _ _ _ _ _ _ _ _ _ _ _ _ _ _ _ _ _ _ _ _ _ _ _ _ _ _ _ _ _ _ _ _ _ _ _ _ _ _ _ _ _ _ _ _ _ _ _ _ _ _ _ _ _ _ _ _ _ _ _ _ _ _ _ _ _ _ _ _ _ _ _ _ _ _ _ _ _ _ _ _ _ _ _ _ _] -> w80
      tunnel: [w98 w475 w483 w490 w496 w518 w531 w549 w617 w625 w661 w704 w717 w740 w771 w791 w820 w834 w882 w952 w987 w1006 w1013 w1020 w1047 w1054 w1078 w1082 w1087 w1108 w1138 w1166 w1208 w1213 w1219 w1226 w1253 w1279 w1305 w1328 w1341 w1386 w1414 w1419 w1445 w1466 w1470 w1475 w1503 w1530 w1549 w1573 w1601 w1606 w1616 w1628 w1646 w1671 w1682 w1700 w1717 w1742 w1761 w1775 w1782 w1801 w1813 w1825 w1844 w1860 w1873 w1885 w1897 w1901 w1907 w1914 w1926 w1935 w1940 w1948 w1958 w1966 w1988 w1997 w2021 w2046 w2057 w2078 w2082 w2087 w2095 w2103 w2112 w2118 w2126 w2133 w2143 w2171 w2179 w2186 w2194 w2199 w2204 w2215 w2220 w2226 w2245 w2250 w2258 w2268 w2339 w2345 w2358 w2378 w2387 w2402 w2426 w2437 w2448 w2472 w2498 w2504 w2517 w2541 w2550 w2556 w2561 w2568 w2576 w2589 w2599 w2604 w2616 w2621 w2627 w2637 w2643 w2648 w2653 w2658 w2668 w2691 w2710 w2714 w2726 w2751 w2778 w2801 w2805 w2821 w2867 w2916 w2962 w2972 w2989 w3009 w3023 w3037 w3043 w3061 w3083 w3107 w3126 w3144 w3162 w3180 w3194 w3208 w3227 w3241 w3258 w3273 w3283 w3287] -> w88
      tunnel: 30 ("Timeout") -> [w97 _ _ _ _ _ _ _ _ _ _ _ _ _ _ _ _ _ _ _ _ _ _ _ _ _ _ _ _ _ _ _ _ _ _ _ _ _ _ _ _ _ _ _ _ _ _ _ _ _ _ _ _ _ _ _ _ _ _ _ _ _ _ _ _ _ _ _ _ _ _ _ _ _ _ _ _ _ _ _ _ _ _ _ _ _ _ _ _ _ _ _ _ _ _ _ _ _ _ _ _ _ _ _ _ _ _ _ _ _ _ _ _ _ _ _ _ _ _ _ _ _ _ _ _ _ _ _ _ _ _ _ _ _ _ _ _ _ _ _ _ _ _ _ _ _ _ _ _ _ _ _ _ _ _ _ _ _ _ _ _ _ _ _ _ _ _ _ _ _ _ _ _ _]
      tunnel: w85 -> [_ _ _ _ _ _ _ _ _ _ _ _ _ _ _ _ _ _ _ w956 _ _ _ _ _ _ _ _ _ _ _ _ _ _ _ _ _ _ _ _ _ _ _ _ _ _ _ _ _ _ _ _ _ _ _ _ _ _ _ _ _ _ _ _ _ _ _ _ _ _ _ w1882 w1893 _ _ _ _ _ _ _ _ _ _ _ _ _ _ _ _ _ _ _ _ _ _ _ _ _ _ _ _ _ _ _ _ _ _ _ _ _ _ _ _ _ _ _ _ _ _ _ _ _ _ _ _ _ _ _ _ _ _ _ _ _ _ _ _ _ _ _ _ _ _ _ _ _ _ _ _ _ _ _ _ _ _ _ _ _ _ _ _ _ _ _ _ _ _ _ _ _ _ _ _ _]
      tunnel: w84 -> [_ _ _ _ _ _ _ _ _ _ _ _ _ _ _ _ _ _ _ w955 _ _ _ _ _ _ _ _ _ _ _ _ _ _ _ _ _ _ _ _ _ _ _ _ _ _ _ _ _ _ _ _ _ _ _ _ _ _ _ _ _ _ _ _ _ _ _ _ _ _ _ w1883 w1892 _ _ _ _ _ _ _ _ _ _ _ _ _ _ _ _ _ _ _ _ _ _ _ _ _ _ _ _ _ _ _ _ _ _ _ _ _ _ _ _ _ _ _ _ _ _ _ _ _ _ _ _ _ _ _ _ _ _ _ _ _ _ _ _ _ _ _ _ _ _ _ _ _ _ _ _ _ _ _ _ _ _ _ _ _ _ _ _ _ _ _ _ _ _ _ _ _ _ _ _ _]
      tunnel: w83 -> [w96 _ _ _ _ _ _ _ _ _ _ _ _ _ _ _ _ _ _ _ _ _ _ _ _ _ _ _ _ _ _ _ _ _ _ _ _ _ _ _ _ _ w1410 _ _ _ _ _ _ _ _ _ _ _ _ _ _ _ _ _ _ _ _ _ _ _ _ _ _ _ _ _ _ _ _ _ _ _ _ _ _ _ _ _ _ _ _ _ _ _ _ _ _ _ _ _ _ _ _ _ _ _ _ _ _ _ _ _ _ _ _ _ _ _ _ _ _ _ _ _ _ _ _ _ _ _ _ _ _ _ _ _ _ _ _ _ _ _ _ _ _ _ _ _ _ _ _ _ _ _ _ _ _ _ _ _ _ _ _ _ _ _ _ _ _ _ _ _ _ _ _ _ _ _]
      tunnel: w82 -> [w95 w474 w484 w489 w495 w510 w530 w559 w618 w632 w663 w706 w718 w746 w778 w792 w821 w833 w920 w957 w996 w1005 w1012 w1017 w1034 w1053 w1076 w1081 w1095 w1114 w1143 w1163 w1206 w1212 w1218 w1225 w1252 w1278 w1304 w1327 w1336 w1360 w1415 w1431 w1444 w1453 w1469 w1483 w1512 w1538 w1543 w1588 w1593 w1605 w1612 w1621 w1633 w1664 w1680 w1694 w1714 w1729 w1760 w1776 w1786 w1802 w1814 w1826 w1854 w1857 w1872 w1884 w1891 w1900 w1909 w1917 w1924 w1933 w1939 w1949 w1952 w1964 w1983 w1998 w2017 w2043 w2061 w2077 w2081 w2089 w2097 w2102 w2110 w2117 w2125 w2132 w2142 w2170 w2178 w2185 w2190 w2198 w2207 w2213 w2219 w2228 w2240 w2249 w2254 w2265 w2338 w2343 w2355 w2365 w2381 w2410 w2425 w2438 w2450 w2474 w2494 w2502 w2515 w2543 w2548 w2554 w2560 w2567 w2578 w2590 w2598 w2603 w2615 w2620 w2631 w2636 w2642 w2647 w2652 w2657 w2667 w2690 w2709 w2713 w2725 w2750 w2777 w2800 w2804 w2820 w2872 w2918 w2959 w2974 w2992 w3012 w3026 w3038 w3047 w3064 w3086 w3110 w3129 w3147 w3165 w3183 w3197 w3211 w3230 w3244 w3259 w3272 w3282 w3286]
      tunnel: [w94 w474 w484 w489 w495 w510 w530 w559 w618 w632 w663 w706 w718 w746 w778 w792 w821 w833 w920 w957 w996 w1005 w1012 w1017 w1034 w1053 w1076 w1081 w1095 w1114 w1143 w1163 w1206 w1212 w1218 w1225 w1252 w1278 w1304 w1327 w1336 w1360 w1415 w1431 w1444 w1453 w1469 w1483 w1512 w1538 w1543 w1588 w1593 w1605 w1612 w1621 w1633 w1664 w1680 w1694 w1714 w1729 w1760 w1776 w1786 w1802 w1814 w1826 w1854 w1857 w1872 w1884 w1891 w1900 w1909 w1917 w1924 w1933 w1939 w1949 w1952 w1964 w1983 w1998 w2017 w2043 w2061 w2077 w2081 w2089 w2097 w2102 w2110 w2117 w2125 w2132 w2142 w2170 w2178 w2185 w2190 w2198 w2207 w2213 w2219 w2228 w2240 w2249 w2254 w2265 w2338 w2343 w2355 w2365 w2381 w2410 w2425 w2438 w2450 w2474 w2494 w2502 w2515 w2543 w2548 w2554 w2560 w2567 w2578 w2590 w2598 w2603 w2615 w2620 w2631 w2636 w2642 w2647 w2652 w2657 w2667 w2690 w2709 w2713 w2725 w2750 w2777 w2800 w2804 w2820 w2872 w2918 w2959 w2974 w2992 w3012 w3026 w3038 w3047 w3064 w3086 w3110 w3129 w3147 w3165 w3183 w3197 w3211 w3230 w3244 w3259 w3272 w3282 w3286] -> w81
      tunnel: w77 -> [_ _ _ _ _ _ _ _ _ _ _ _ _ _ _ _ _ _ _ w950 _ _ _ _ _ _ _ _ _ _ _ _ _ _ _ _ _ _ _ _ _ _ _ _ _ _ _ _ _ _ _ _ _ _ _ _ _ _ _ _ _ _ _ _ _ _ _ _ _ _ _ w1879 w1890 _ _ _ _ _ _ _ _ _ _ _ _ _ _ _ _ _ _ _ _ _ _ _ _ _ _ _ _ _ _ _ _ _ _ _ _ _ _ _ _ _ _ _ _ _ _ _ _ _ _ _ _ _ _ _ _ _ _ _ _ _ _ _ _ _ _ _ _ _ _ _ _ _ _ _ _ _ _ _ _ _ _ _ _ _ _ _ _ _ _ _ _ _ _ _ _ _ _ _ _ _]
      frame "", "Event Structure", "Idle" {
        # "executes when the state queue is empty"
        n31 = event shown="[20] \"Quit\": Value Change" {
          selector: w95 -> [_ _ _ _ _ _ _ _ _ _ _ _ _ _ _ _ _ _ _ _ _ _ _ _ _ _ _ _ _ _ _ _ _ _ _ _ _]
          dyn-events: [_ _ _ _ _ _ _ _ _ _ _ _ _ _ _ _ _ _ _ _ _ _ _ _ _ _ _ _ _ _ _ _ _ _ _ _ _] -> w94
          timeout: w97 -> [_ _ _ _ _ _ _ _ _ _ _ _ _ _ _ _ _ _ _ _ _ _ _ _ _ _ _ _ _ _ _ _ _ _ _ _ _]
          tunnel: w102 -> [w122 w141 w149 w153 w157 w165 w171 w179 w187 w197 w204 w229 w245 w261 w265 w272 w295 w309 w323 w337 w342 w345 w351 w358 w365 w371 w377 w383 w390 w403 w414 w426 w433 w437 w441 w457 w473]
          tunnel: [w123 w141 w148 w153 w156 w165 w171 w179 w187 w197 w203 w229 w245 w261 w265 w271 w295 w309 w323 w337 w341 w344 w351 w359 w366 w370 w376 w383 w391 w404 w414 w427 w433 w437 w440 w458 w472] -> w101
          tunnel: w100 -> [w106 w139 w143 w151 w158 w164 w172 w180 w188 w195 w199 w227 w243 w259 w263 w267 w294 w308 w322 w336 w338 w346 w349 w354 w361 w373 w378 w381 w385 w398 w412 w422 w431 w435 w442 w455 w470]
          tunnel: [w121 w140 w144 w152 w159 w163 w170 w178 w186 w196 w205 w228 w244 w260 w264 w273 w292 w296 w319 w334 w340 w347 w350 w355 w362 w374 w379 w382 w389 w402 w413 w423 w432 w436 w443 w459 w471] -> w93
          tunnel: w99 -> [w121 w140 w144 w152 w159 w163 w170 w178 w186 w196 w205 w228 w244 w260 w264 w273 w289 w298 w310 w326 w340 w347 w350 w355 w362 w374 w379 w382 w389 w402 w413 w425 w432 w436 w443 w459 w471]
          tunnel: [w106 w139 w143 w151 w158 w164 w172 w180 w188 w195 w200 w227 w243 w259 w263 w268 w294 w308 w322 w336 w338 w346 w349 w356 w363 w373 w378 w381 w386 w399 w412 w428 w431 w435 w442 w456 w470] -> w98
          tunnel: w96 -> [_ _ _ _ _ _ _ _ _ _ _ _ _ _ _ _ _ _ _ _ _ _ _ _ _ _ _ _ _ _ _ _ _ _ _ _ _]
          event Timeout {
            # "check system status every 2s"
            n32 = event-data() -> ()  [unwired: 1 in, 1 out]
            n33 = Unbundle By Name(w106) -> ("SysRunning?"=w104:bool, "SlowTimer"=w120:u32, "FastTimer"=w114:u32)
            n34 = Tick Count (ms)() -> (millisecond timer value=w107:u32)
            n35 = Subtract(x=w107, y=w120) -> (x-y=w117:u32)
            n36 = case shown="False" w104 {
              tunnel: ["" "Utility: AquiTimerCheck" ("State(s) in Front (\"\")")] -> w112
              frame False {
                # "if not running, do nothing"
              }
              frame True {
                # "if aquisition is running, check timer"
              }
            }
            n37 = Subtract(x=w107, y=w114) -> (x-y=w115:u32)
            n38 = Greater?(x=w117, y=u32 2000) -> (0:w118:bool)
            n39 = Greater?(x=w115, y=u32 500) -> (0:w105:bool)
            n40 = disable-structure shown="Enabled" {
              disable-tunnel: w105 -> [w128 _]
              disable-tunnel: w104 -> [w127 _]
              disable-tunnel: [w124 "" ("State(s) at Back (\"\")")] -> w103
              frame Disabled {
                n41 = Not(x=w127) -> (.not. x?=w126:bool)
                n42 = And(x=w128, y=w126) -> (x .and. y?=w125:bool)
                n43 = case shown="True" w125 {
                  tunnel: ["" ("Empty String Constant") "TCP: checkSource" ("State(s) in Front (\"\")")] -> w124
                  frame False {
                  }
                  frame True {
                  }
                }
              }
              frame Enabled {
              }
            }
            n44 = case shown="True" w118 {
              tunnel: ["" ("Empty String Constant") "SystemStatus: SlowSysStatusMacro" ("State(s) in Front (\"\")")] -> w110
              frame False {
              }
              frame True {
              }
            }
            n45 = case shown="True" w105 {
              tunnel: ["" ("Empty String Constant") "SystemStatus: FastSysStatusMacro" ("State(s) in Front (\"\")")] -> w108
              frame False {
              }
              frame True {
              }
            }
            n46 = call <vilib>:"Add State(s) to Queue__JKI_lib_State_Machine.vi"("State(s) in Front (\"\")"=w112, "State(s) in (\"\")"="LabJack: checkPedal" ("State(s) in Front (\"\")"), "State(s) at Back (\"\")"=w110) -> ("States Out"=w109:string)  [unwired: 12 in]
            n47 = call <vilib>:"Add State(s) to Queue__JKI_lib_State_Machine.vi"("State(s) in Front (\"\")"=w109, "State(s) in (\"\")"=w108, "State(s) at Back (\"\")"=w103) -> ("States Out"=w113:string)  [unwired: 12 in]
            n48 = call <vilib>:"Add State(s) to Queue__JKI_lib_State_Machine.vi"("State(s) in Front (\"\")"=w113, "State(s) in (\"\")"=w122) -> ("States Out"=w123:string)  [unwired: 13 in]
          }
          event "355nm Laser toggle": Mouse Enter {
            n49 = event-data() -> ()  [unwired: 1 in, 4 out]
            n50 = local write "Help"("Toggle 355nm laser." ("Help")) -> ()
          }
          event "355nm Laser toggle": Value Change {
            # "[Covers: REQ34]"
            n51 = event-data() -> ()  [unwired: 1 in, 6 out]
            n52 = Select(t="LabJack: 355_PWM_Start\nLabJack: AB_Start", s="355nm Laser toggle", f="LabJack: 355_PWM_Stop\nLabJack: AB_Stop") -> (s? t:f=w146:string)
            n53 = call <vilib>:"Add State(s) to Queue__JKI_lib_State_Machine.vi"("State(s) in Front (\"\")"=w146, "State(s) in (\"\")"=w149) -> ("States Out"=w148:string)  [unwired: 13 in]
          }
          event "Aiming beam toggle": Mouse Enter {
            n54 = event-data() -> ()  [unwired: 1 in, 4 out]
            n55 = local write "Help"("Toggle aiming beam laser." ("Help")) -> ()
          }
          event "Aiming beam toggle": Value Change {
            # "[Covers: REQ33]"
            n56 = event-data() -> ()  [unwired: 1 in, 6 out]
            n57 = case shown="True" "Aiming beam toggle" {
              tunnel: ["LabJack: AB_Stop" ("State(s) in Front (\"\")") "LabJack: AB_Start" ("State(s) in Front (\"\")")] -> w155
              frame False {
              }
              frame True {
              }
            }
            n58 = call <vilib>:"Add State(s) to Queue__JKI_lib_State_Machine.vi"("State(s) in Front (\"\")"=w155, "State(s) in (\"\")"=w157) -> ("States Out"=w156:string)  [unwired: 13 in]
          }
          event "Auto gain ch1": Value Change {
            n59 = event-data() -> ("NewVal"=w162:bool)  [unwired: 1 in, 5 out]
            n60 = case shown="True" w162 {
              frame False {
                n61 = local read "V 1"() -> (w166:dbl)
                n62 = call "V1FGV.vi"("action (write)"=enum16{"write", "read"}."write" ("action"), "V1 in"=w166) -> ()  [unwired: 8 in, 2 out]
                n63 = property on="V 1" class="DigNum (strict)"("DisabledEnum"=T11."Enabled" ("Disabled")) -> ()  [unwired: 2 in, 2 out]
              }
              frame True {
                n64 = property on="V 1" class="DigNum (strict)"("DisabledEnum"=T11."Disabled and Grayed Out" ("Disabled")) -> ()  [unwired: 2 in, 2 out]
              }
            }
          }
          event "Auto gain ch2": Value Change {
            n65 = event-data() -> ("NewVal"=w173:bool)  [unwired: 1 in, 5 out]
            n66 = case shown="False" w173 {
              frame False {
                n67 = local read "V 2"() -> (w174:dbl)
                n68 = property on="V 2" class="DigNum (strict)"("DisabledEnum"=T11."Enabled" ("Disabled")) -> ()  [unwired: 2 in, 2 out]
                n69 = call "V2FGV.vi"("action(write)"=enum16{"write", "read"}."write" ("action"), "V2 in"=w174) -> ()  [unwired: 8 in, 2 out]
              }
              frame True {
                n70 = property on="V 2" class="DigNum (strict)"("DisabledEnum"=T11."Disabled and Grayed Out" ("Disabled")) -> ()  [unwired: 2 in, 2 out]
              }
            }
          }
          event "Auto gain ch3": Value Change {
            n71 = event-data() -> ("NewVal"=w181:bool)  [unwired: 1 in, 5 out]
            n72 = case shown="False" w181 {
              frame False {
                n73 = local read "V 3"() -> (w182:dbl)
                n74 = property on="V 3" class="DigNum (strict)"("DisabledEnum"=T11."Enabled" ("Disabled")) -> ()  [unwired: 2 in, 2 out]
                n75 = call "V3FGV.vi"("action(write)"=enum16{"write", "read"}."write" ("action"), "V3 in"=w182) -> ()  [unwired: 8 in, 2 out]
              }
              frame True {
                n76 = property on="V 3" class="DigNum (strict)"("DisabledEnum"=T11."Disabled and Grayed Out" ("Disabled")) -> ()  [unwired: 2 in, 2 out]
              }
            }
          }
          event "Auto gain ch4": Value Change {
            n77 = event-data() -> ("NewVal"=w189:bool)  [unwired: 1 in, 5 out]
            n78 = case shown="False" w189 {
              frame False {
                n79 = local read "V 4"() -> (w190:dbl)
                n80 = property on="V 4" class="DigNum (strict)"("DisabledEnum"=T11."Enabled" ("Disabled")) -> ()  [unwired: 2 in, 2 out]
                n81 = call "V4FGV.vi"("action(write)"=enum16{"write", "read"}."write" ("action"), "V3 in"=w190) -> ()  [unwired: 8 in, 2 out]
              }
              frame True {
                n82 = property on="V 4" class="DigNum (strict)"("DisabledEnum"=T11."Disabled and Grayed Out" ("Disabled")) -> ()  [unwired: 2 in, 2 out]
              }
            }
          }
          event "Background": Mouse Enter {
            n83 = event-data() -> ()  [unwired: 1 in, 4 out]
            n84 = local write "Help"("Click to record a background." ("Help")) -> ()
          }
          event "Background": Value Change {
            n85 = event-data() -> ("NewVal"=w201:bool)  [unwired: 1 in, 5 out]
            n86 = case shown="True" w201 {
              tunnel: ["Utility: SetAllChanManualGain\nQueue: Flash\nUtility: Dewelling >> 2500\nLabJack: 355_PWM_Stop\nLabJack: AB_Stop" "Utility: SetDataClass >> Bg\nUI: Update\nLabJack: 355_PWM_Start\nLabJack: AB_Start\nUtility: SaveDeconChan\nUtility: Dewelling >> 50\nLabJack: SetV\nDigitizer: Start\nUtility: AquiTimerReset\nLED: BreathGreen\nUI: duringBGAcquire"] -> w202
              tunnel: [FALSE TRUE] -> w198
              frame False {
                n87 = local read "Skip Data Save?"() -> (w206:bool)
                n88 = case shown="False" w206 {
                  frame False {
                    n89 = property on="Background" class="Bool (strict)"("BoolText.Text"="Done!" ("Boolean Text.Text")) -> ()  [unwired: 2 in, 2 out]
                  }
                  frame True {
                  }
                }
              }
              frame True {
                # "[Covers: REQ6]"
                n90 = property on="Background" class="Bool (strict)"("BoolText.Text"="Running" ("Boolean Text.Text"), "Colors [4]"=cluster{u32, u32}[] [{6618880, 6618880}, {16711680, 16711680}]) -> ()  [unwired: 2 in, 2 out]
              }
            }
            n91 = Bundle By Name(cluster=w199, "SysRunning?"=w198) -> (w200:T23)
            n92 = call <vilib>:"Add State(s) to Queue__JKI_lib_State_Machine.vi"("State(s) in Front (\"\")"=w202, "State(s) in (\"\")"=w204) -> ("States Out"=w203:string)  [unwired: 13 in]
          }
          event "Channel 1": Cursor Move {
            n93 = event-data() -> ("CursIdx"=w218:i32, "CursLoc"=w225:cluster{"X":dbl, "Y":dbl})  [unwired: 1 in, 7 out]
            n94 = Unbundle By Name(w225) -> ("X"=w223:dbl)
            n95 = property on="Channel 2" class="WFGraph (strict)"() -> ("CrsrList"=w222:T24)  [unwired: 2 in, 2 out]
            n96 = property on="Channel 3" class="WFGraph (strict)"() -> ("CrsrList"=w219:T24)  [unwired: 2 in, 2 out]
            n97 = Index Array(array=w222, index=w218) -> (element=w226:T25)
            n98 = Index Array(array=w219, index=w218) -> (element=w224:T25)
            n99 = Bundle By Name(cluster=w224, "Position.X"=w223) -> (w217:T25)
            n100 = Bundle By Name(cluster=w226, "Position.X"=w223) -> (w221:T25)
            n101 = control-ref of="Channel 1"() -> (w214:refnum<vi>)
            n102 = Replace Array Subset(array=w222, new element=w221, index=w218) -> (w220:T24)
            n103 = Replace Array Subset(array=w219, new element=w217, index=w218) -> (w216:T24)
            n104 = property on="Channel 2" class="WFGraph (strict)"("CrsrList"=w220) -> ()  [unwired: 2 in, 2 out]
            n105 = property on="Channel 3" class="WFGraph (strict)"("CrsrList"=w216) -> (error out=w215:errorcluster)  [unwired: 2 in, 1 out]
            n106 = call "UpdateCurserIdx(SubVI).vi"("error in (no error)"=w215, "WaveformGraph in"=w214) -> ()  [unwired: 9 in, 1 out]
          }
          event "Channel 2": Cursor Move {
            n107 = event-data() -> ("CursIdx"=w236:i32, "CursLoc"=w242:cluster{"X":dbl, "Y":dbl})  [unwired: 1 in, 7 out]
            n108 = Unbundle By Name(w242) -> ("X"=w239:dbl)
            n109 = property on="Channel 1" class="WFGraph (strict)"() -> ("CrsrList"=w234:T24)  [unwired: 2 in, 2 out]
            n110 = property on="Channel 3" class="WFGraph (strict)"() -> ("CrsrList"=w237:T24)  [unwired: 2 in, 2 out]
            n111 = Index Array(array=w234, index=w236) -> (element=w241:T25)
            n112 = Index Array(array=w237, index=w236) -> (element=w240:T25)
            n113 = Bundle By Name(cluster=w241, "Position.X"=w239) -> (w238:T25)
            n114 = Bundle By Name(cluster=w240, "Position.X"=w239) -> (w235:T25)
            n115 = Replace Array Subset(array=w234, new element=w238, index=w236) -> (w233:T24)
            n116 = Replace Array Subset(array=w237, new element=w235, index=w236) -> (w232:T24)
            n117 = control-ref of="Channel 1"() -> (w231:refnum<vi>)
            n118 = property on="Channel 1" class="WFGraph (strict)"("CrsrList"=w233) -> ()  [unwired: 2 in, 2 out]
            n119 = property on="Channel 3" class="WFGraph (strict)"("CrsrList"=w232) -> (error out=w230:errorcluster)  [unwired: 2 in, 1 out]
            n120 = call "UpdateCurserIdx(SubVI).vi"("error in (no error)"=w230, "WaveformGraph in"=w231) -> ()  [unwired: 9 in, 1 out]
          }
          event "Channel 3": Cursor Move {
            n121 = event-data() -> ("CursIdx"=w251:i32, "CursLoc"=w258:cluster{"X":dbl, "Y":dbl})  [unwired: 1 in, 7 out]
            n122 = Unbundle By Name(w258) -> ("X"=w255:dbl)
            n123 = property on="Channel 1" class="WFGraph (strict)"() -> ("CrsrList"=w254:T24)  [unwired: 2 in, 2 out]
            n124 = property on="Channel 2" class="WFGraph (strict)"() -> ("CrsrList"=w252:T24)  [unwired: 2 in, 2 out]
            n125 = Index Array(array=w254, index=w251) -> (element=w257:T25)
            n126 = Index Array(array=w252, index=w251) -> (element=w256:T25)
            n127 = Bundle By Name(cluster=w257, "Position.X"=w255) -> (w253:T25)
            n128 = Bundle By Name(cluster=w256, "Position.X"=w255) -> (w250:T25)
            n129 = Replace Array Subset(array=w254, new element=w253, index=w251) -> (w249:T24)
            n130 = Replace Array Subset(array=w252, new element=w250, index=w251) -> (w248:T24)
            n131 = control-ref of="Channel 1"() -> (w246:refnum<vi>)
            n132 = property on="Channel 1" class="WFGraph (strict)"("CrsrList"=w249) -> ()  [unwired: 2 in, 2 out]
            n133 = property on="Channel 2" class="WFGraph (strict)"("CrsrList"=w248) -> (error out=w247:errorcluster)  [unwired: 2 in, 1 out]
            n134 = call "UpdateCurserIdx(SubVI).vi"("error in (no error)"=w247, "WaveformGraph in"=w246) -> ()  [unwired: 9 in, 1 out]
          }
          event "Cali&iRF alignment": Mouse Enter {
            n135 = event-data() -> ()  [unwired: 1 in, 4 out]
            n136 = local write "Help"("Click to run system intensity calibration and irf alignment" ("Help")) -> ()
          }
          event "Cali&iRF alignment": Value Change {
            n137 = event-data() -> ("NewVal"=w269:bool)  [unwired: 1 in, 5 out]
            n138 = case shown="False" w269 {
              tunnel: ["Utility: SetAllChanManualGain\nQueue: Flash\nUtility: Dewelling >> 2500\nLabJack: 355_PWM_Stop\nLabJack: AB_Stop" "Utility: SetDataClass >> Cali\nUI: Update\nUtility: SaveDeconChan\nLabJack: 355_PWM_Start\nLabJack: AB_Start\nLabJack: SetV\nDigitizer: Start\nUtility: AquiTimerReset\nLED: BreathGreen\nUI: duringIRFAlign"] -> w270
              tunnel: [FALSE TRUE] -> w266
              frame False {
                n139 = local read "Skip Data Save?"() -> (w274:bool)
                n140 = case shown="False" w274 {
                  frame False {
                    n141 = property on="Cali&iRF alignment" class="Bool (strict)"("BoolText.Text"="Done!" ("Boolean Text.Text")) -> ()  [unwired: 2 in, 2 out]
                  }
                  frame True {
                  }
                }
              }
              frame True {
                n142 = property on="Cali&iRF alignment" class="Bool (strict)"("BoolText.Text"="Running" ("Boolean Text.Text"), "Colors [4]"=cluster{u32, u32}[] [{6618880, 6618880}, {16711680, 16711680}]) -> ()  [unwired: 2 in, 2 out]
              }
            }
            n143 = Bundle By Name(cluster=w267, "SysRunning?"=w266) -> (w268:T23)
            n144 = call <vilib>:"Add State(s) to Queue__JKI_lib_State_Machine.vi"("State(s) in Front (\"\")"=w270, "State(s) in (\"\")"=w272) -> ("States Out"=w271:string)  [unwired: 13 in]
          }
          event "V 1": Value Change {
            n145 = event-data() -> ()  [unwired: 1 in, 6 out]
            n146 = call "LabJack_FGV.vi"("Operation(Read)"=enum16{"Write", "Read"}."Read" ("Operation"), "error in (no error)"=w289) -> ("error out"=w286:errorcluster, "Read data"=w287:i32)  [unwired: 8 in]
            n147 = global read "GlobalVariables.vi" "Ch1 LJ pin"() -> (w285:string)
            n148 = call "LJM_eWriteName.vi"("Handle In"=w287, "Name"=w285, "Value"="V 1", "error in"=w286) -> ("error out"=w283:errorcluster)  [unwired: 10 in, 1 out]
            n149 = call "V1FGV.vi"("Error In"=w283, "action (write)"=enum16{"write", "read"}."write" ("action"), "V1 in"="V 1") -> ("Error Out"=w282:errorcluster)  [unwired: 7 in, 1 out]
            n150 = call "CtrlVtoGain.vi"("error in (no error)"=w282, "CtrlV(V)"="V 1", "Channel"=enum16{"Ch1", "Ch2", "Ch3"}."Ch1" ("Enum")) -> ("error out"=w292:errorcluster, "Gain"=w291:dbl)  [unwired: 7 in]
            n151 = local write "Gain1"(w291) -> ()
          }
          event "V 2": Value Change {
            n152 = event-data() -> ()  [unwired: 1 in, 6 out]
            n153 = call "LabJack_FGV.vi"("Operation(Read)"=enum16{"Write", "Read"}."Read" ("Operation"), "error in (no error)"=w298) -> ("error out"=w303:errorcluster, "Read data"=w304:i32)  [unwired: 8 in]
            n154 = global read "GlobalVariables.vi" "Ch2 LJ pin"() -> (w302:string)
            n155 = call "LJM_eWriteName.vi"("Handle In"=w304, "Name"=w302, "Value"="V 2", "error in"=w303) -> ("error out"=w301:errorcluster)  [unwired: 10 in, 1 out]
            n156 = call "V2FGV.vi"("Error In"=w301, "action(write)"=enum16{"write", "read"}."write" ("action"), "V2 in"="V 2") -> ("Error Out"=w300:errorcluster)  [unwired: 7 in, 1 out]
            n157 = call "CtrlVtoGain.vi"("error in (no error)"=w300, "CtrlV(V)"="V 2", "Channel"=enum16{"Ch1", "Ch2", "Ch3"}."Ch2" ("Enum")) -> ("error out"=w296:errorcluster, "Gain"=w297:dbl)  [unwired: 7 in]
            n158 = local write "Gain2"(w297) -> ()
          }
          event "V 3": Value Change {
            n159 = event-data() -> ()  [unwired: 1 in, 6 out]
            n160 = call "LabJack_FGV.vi"("Operation(Read)"=enum16{"Write", "Read"}."Read" ("Operation"), "error in (no error)"=w310) -> ("error out"=w315:errorcluster, "Read data"=w316:i32)  [unwired: 8 in]
            n161 = global read "GlobalVariables.vi" "Ch3 LJ pin"() -> (w314:string)
            n162 = call "LJM_eWriteName.vi"("Handle In"=w316, "Name"=w314, "Value"="V 3", "error in"=w315) -> ("error out"=w312:errorcluster)  [unwired: 10 in, 1 out]
            n163 = call "V3FGV.vi"("Error In"=w312, "action(write)"=enum16{"write", "read"}."write" ("action"), "V3 in"="V 3") -> ("Error Out"=w311:errorcluster)  [unwired: 7 in, 1 out]
            n164 = call "CtrlVtoGain.vi"("error in (no error)"=w311, "CtrlV(V)"="V 3", "Channel"=enum16{"Ch1", "Ch2", "Ch3"}."Ch3" ("Enum")) -> ("error out"=w319:errorcluster, "Gain"=w318:dbl)  [unwired: 7 in]
            n165 = local write "Gain3"(w318) -> ()
          }
          event "V 4": Value Change {
            n166 = event-data() -> ()  [unwired: 1 in, 6 out]
            n167 = call "LabJack_FGV.vi"("Operation(Read)"=enum16{"Write", "Read"}."Read" ("Operation"), "error in (no error)"=w326) -> ("error out"=w330:errorcluster, "Read data"=w331:i32)  [unwired: 8 in]
            n168 = global read "GlobalVariables.vi" "Ch4 LJ pin"() -> (w329:string)
            n169 = call "LJM_eWriteName.vi"("Handle In"=w331, "Name"=w329, "Value"="V 4", "error in"=w330) -> ("error out"=w328:errorcluster)  [unwired: 10 in, 1 out]
            n170 = call "V4FGV.vi"("Error In"=w328, "action(write)"=enum16{"write", "read"}."write" ("action"), "V3 in"="V 4") -> ("Error Out"=w327:errorcluster)  [unwired: 7 in, 1 out]
            n171 = call "CtrlVtoGain.vi"("error in (no error)"=w327, "CtrlV(V)"="V 4", "Channel"=enum16{"Ch1", "Ch2", "Ch3", "Ch4"}."Ch4") -> ("error out"=w334:errorcluster, "Gain"=w333:dbl)  [unwired: 7 in]
            n172 = local write "Gain4"(w333) -> ()
          }
          event "Quit": Value Change {
            # "Exit Button Value Change (pressed) Event\n(when pressed.  quite)"
            n173 = event-data() -> ()  [unwired: 1 in, 1 out]
            n174 = call <vilib>:"Add State(s) to Queue__JKI_lib_State_Machine.vi"("State(s) in Front (\"\")"="LED: Off\nMacro: Exit", "State(s) in (\"\")"=w342) -> ("States Out"=w341:string)  [unwired: 13 in]
          }
          event "Show BG": Value Change {
            n175 = event-data() -> ()  [unwired: 1 in, 6 out]
            n176 = call <vilib>:"Add State(s) to Queue__JKI_lib_State_Machine.vi"("State(s) in Front (\"\")"="Data: showBG" ("State(s) in Front (\"\")"), "State(s) in (\"\")"=w345) -> ("States Out"=w344:string)  [unwired: 13 in]
          }
          event "StartButton": Mouse Enter {
            n177 = event-data() -> ()  [unwired: 1 in, 4 out]
            n178 = local write "Help"("Press to start aquisition." ("Help")) -> ()
          }
          event "StartButton": Value Change {
            # "[Covers: REQ32]"
            # "start PWM before acquisition"
            # "Initialize both digitizer aquisition and\n send user event to trigger aquisition loop"
            n179 = event-data() -> ()  [unwired: 1 in, 6 out]
            n180 = local write "StartButton"(FALSE ("StartButton")) -> ()
            n181 = Bundle By Name(cluster=w354, "SysRunning?"=TRUE) -> (w356:T23)
            n182 = call <vilib>:"Add State(s) to Queue__JKI_lib_State_Machine.vi"("State(s) in Front (\"\")"="TCP: stopCam\nUtility: SetDataClass >> Data\nQueue: Flash\nUI: Update\nUtility: StartBeep\nLabJack: 355_PWM_Start\nLabJack: AB_Start\nLabJack: SetV\nDigitizer: Start\nUtility: AquiTimerReset\nUI: DuringAquisition\nLED: BreathGreen\nTCP: sendRunNum\nTCP: sendVideoSource\nTCP: sendChannel\nTCP: startRun", "State(s) in (\"\")"=w358) -> ("States Out"=w359:string)  [unwired: 13 in]
          }
          event User Event {
            # "[Covers: REQ32]"
            # "start PWM before acquisition"
            # "Initialize both digitizer aquisition and\n send user event to trigger aquisition loop"
            n183 = event-data() -> ()  [unwired: 1 in, 5 out]
            n184 = Bundle By Name(cluster=w361, "SysRunning?"=TRUE) -> (w363:T23)
            n185 = call <vilib>:"Add State(s) to Queue__JKI_lib_State_Machine.vi"("State(s) in Front (\"\")"="TCP: stopCam\nUtility: SetDataClass >> Data\nQueue: Flash\nUI: Update\nUtility: StartBeep\nLabJack: 355_PWM_Start\nLabJack: AB_Start\nLabJack: SetV\nDigitizer: Start\nUtility: AquiTimerReset\nUI: DuringAquisition\nLED: BreathGreen\nTCP: sendRunNum\nTCP: sendVideoSource\nTCP: sendChannel\nTCP: startRun", "State(s) in (\"\")"=w365) -> ("States Out"=w366:string)  [unwired: 13 in]
          }
          event "Video Display": Value Change {
            n186 = event-data() -> ("NewVal"=w372:bool)  [unwired: 1 in, 5 out]
            n187 = Select(t="TCP: startCam", s=w372, f="TCP: stopCam") -> (s? t:f=w369:string)
            n188 = call <vilib>:"Add State(s) to Queue__JKI_lib_State_Machine.vi"("State(s) in (\"\")"=w371, "State(s) at Back (\"\")"=w369) -> ("States Out"=w370:string)  [unwired: 13 in]
          }
          event "Video Source": Value Change {
            n189 = event-data() -> ()  [unwired: 1 in, 6 out]
            n190 = call <vilib>:"Add State(s) to Queue__JKI_lib_State_Machine.vi"("State(s) in Front (\"\")"="TCP: sendVideoSource" ("State(s) in Front (\"\")"), "State(s) in (\"\")"=w377) -> ("States Out"=w376:string)  [unwired: 13 in]
          }
          event "StopButton": Mouse Enter {
            n191 = event-data() -> ()  [unwired: 1 in, 4 out]
            n192 = local write "Help"("Press to stop data aquisition." ("Help")) -> ()
          }
          event "StopButton": Value Change {
            # "if system is running, send stop command, if not do nothing."
            # "stop aquisition\nupdate UI"
            n193 = event-data() -> ()  [unwired: 1 in, 6 out]
            n194 = Unbundle By Name(w385) -> ("SysRunning?"=w387:bool)
            n195 = case shown="True" w387 {
              tunnel: ["" ("Empty String Constant") "LabJack: AB_Stop\nLabJack: 355_PWM_Stop\n/*Digitizer: Abort"] -> w388
              tunnel: w385 -> [w392 w396]
              tunnel: [w392 w395] -> w386
              frame False {
              }
              frame True {
                n196 = Bundle By Name(cluster=w396, "SysRunning?"=FALSE) -> (w395:T23)
              }
            }
            n197 = call <vilib>:"Add State(s) to Queue__JKI_lib_State_Machine.vi"("State(s) in Front (\"\")"=w388, "State(s) in (\"\")"=w390) -> ("States Out"=w391:string)  [unwired: 13 in]
            n198 = local write "StopButton"(FALSE ("StopButton")) -> ()
          }
          event User Event {
            # "if system is running, send stop command, if not do nothing."
            # "stop aquisition\nupdate UI"
            n199 = event-data() -> ()  [unwired: 1 in, 5 out]
            n200 = Unbundle By Name(w398) -> ("SysRunning?"=w400:bool)
            n201 = case shown="True" w400 {
              tunnel: ["" ("Empty String Constant") "LabJack: AB_Stop\nLabJack: 355_PWM_Stop\n/*Digitizer: Abort"] -> w401
              tunnel: w398 -> [w405 w409]
              tunnel: [w405 w408] -> w399
              frame False {
              }
              frame True {
                n202 = Bundle By Name(cluster=w409, "SysRunning?"=FALSE) -> (w408:T23)
              }
            }
            n203 = call <vilib>:"Add State(s) to Queue__JKI_lib_State_Machine.vi"("State(s) in Front (\"\")"=w401, "State(s) in (\"\")"=w403) -> ("States Out"=w404:string)  [unwired: 13 in]
          }
          event "Sys Reconfig": Mouse Enter {
            n204 = event-data() -> ()  [unwired: 1 in, 4 out]
            n205 = local write "Help"("Click to reconfig digitizer settings." ("Help")) -> ()
          }
          event "Sys Reconfig": Value Change {
            # "everytime the user change data aquisition setting, need to reinitilize decon engine and realign iRF.\ncheck whether data length has changed, if changed, reinitialize Decon engine\nreset BG ready, need a new BG"
            # "update DAQ FGV"
            n206 = event-data() -> ()  [unwired: 1 in, 6 out]
            n207 = call "SystemConfigEditorV6.vi"("error in"=w425) -> ("error out"=w424:errorcluster, "FLImDAQ out"=w419:T6)  [unwired: 1 in]
            n208 = Unbundle By Name(w422) -> ("FLImDAQ.min record length"=w421:i32)
            n209 = Unbundle By Name(w419) -> ("min record length"=w420:i32)
            n210 = call "FLImDAQ_FGV.vi"("error in (no error)"=w424, "Operation (Read)"=enum16{"Write", "Read"}."Write" ("Operation"), "Write data"=w419) -> ("error out"=w423:errorcluster, "Read data"=w418:T6)  [unwired: 7 in]
            n211 = Equal?(x=w421, y=w420) -> (x = y?=w417:bool)
            n212 = case shown="False" w417 {
              tunnel: ["UI: Cursor Set >> Busy\nDigitizer: Config\nDeconEngine: InitializeCh1\nDeconEngine: InitializeCh2\nDeconEngine: InitializeCh3\nUI: CaliAndiRFNotReady\n/*UI iRF not ready\nUI: Update\nUI: Cursor Set >> Idle" "UI: Cursor Set >> Busy\nDigitizer: Config\nUI: Update\nUI: Cursor Set >> Idle"] -> w416
              frame False {
              }
              frame True {
              }
            }
            n213 = Bundle By Name(cluster=w422, "FLImDAQ"=w418) -> (w428:T23)
            n214 = call <vilib>:"Add State(s) to Queue__JKI_lib_State_Machine.vi"("State(s) in Front (\"\")"=w416, "State(s) in (\"\")"=w426) -> ("States Out"=w427:string)  [unwired: 13 in]
          }
          event "System Hardware Connection Status", "StartButton", "StopButton", "355nm Laser toggle", "Aiming beam toggle", "Cali&iRF alignment", "Background", "Sys Reconfig": Mouse Leave {
            n215 = event-data() -> ()  [unwired: 1 in, 4 out]
            n216 = invoke on="Help" class="Str" method="Reinit To Default"() -> ()  [unwired: 3 in, 3 out]
          }
          event "System Hardware Connection Status.Digitizer": Mouse Enter {
            n217 = event-data() -> ()  [unwired: 1 in, 4 out]
            n218 = local write "Help"("Status of hardware connections. TCP/IP is optional." ("Help")) -> ()
          }
          event "TCP Connect": Value Change {
            n219 = event-data() -> ("NewVal"=w438:bool)  [unwired: 1 in, 5 out]
            n220 = case shown="True" w438 {
              tunnel: ["TCP: Close\nUI: Update" ("State(s) in Front (\"\")") "TCP: SendSettingMacro\nUI: Update" ("State(s) in Front (\"\")")] -> w439
              frame False {
              }
              frame True {
              }
            }
            n221 = call <vilib>:"Add State(s) to Queue__JKI_lib_State_Machine.vi"("State(s) in Front (\"\")"=w439, "State(s) in (\"\")"=w441) -> ("States Out"=w440:string)  [unwired: 13 in]
          }
          event User Event {
            # "if aquisition loop is error out. Stop digitizer, update front panel indicator, stop both laser and \nOption 1: parse and save data\nOption 2: Flash queue if scout run. [Covers: REQ23]"
            n222 = event-data() -> ()  [unwired: 1 in, 5 out]
            n223 = case shown="\"Data\", Default" "Data Class" {
              tunnel: [w463 "UI: Cursor Set >> Busy\nUtility: SetAllChanAutoGain\nUtility: RestoreDeConChan\nData: parseRunData\nData: irfAlignment\nUI: Cursor Set >> Idle" "UI: Cursor Set >> Busy\nUtility: SetAllChanAutoGain\nUtility: RestoreDeConChan\nData: parseRunData\nData: saveBGtoFGV\nData: saveBGtoFile\nUI: Cursor Set >> Idle\nData: showBG\nRun: BGIncrement"] -> w453
              frame "Data", Default {
                n224 = local read "Video Display"() -> (w465:bool)
                n225 = Select(t="TCP: startCam", s=w465, f="") -> (s? t:f=w461:string)
                n226 = call <vilib>:"Add State(s) to Queue__JKI_lib_State_Machine.vi"("State(s) in Front (\"\")"="UI: Cursor Set >> Busy\nData: parseRunData\nData: saveRunData\nUI: Cursor Set>>Idle" ("State(s) in Front (\"\")"), "State(s) in (\"\")"=w461) -> ("States Out"=w463:string)  [unwired: 13 in]
              }
              frame "Cali" {
              }
              frame "BG" {
              }
            }
            n227 = Bundle By Name(cluster=w455, "SysRunning?"=FALSE) -> (w456:T23)
            n228 = Select(t="" ("State(s) in Front (\"\")"), s="Skip Data Save?", f=w453) -> (s? t:f=w450:string)
            n229 = call <vilib>:"Add State(s) to Queue__JKI_lib_State_Machine.vi"("State(s) in Front (\"\")"="TCP: stopRun\nUI: Update\nLabJack: AB_Stop\nLabJack: 355_PWM_Stop\nDigitizer: Abort\nLabJack: ZeroV\nUtility: EndBeep\nLED: BreathOff" ("State(s) in Front (\"\")"), "State(s) in (\"\")"=w450, "State(s) at Back (\"\")"="Macro: SysReadyForAq\nUI: Update" ("State(s) in Front (\"\")")) -> ("States Out"=w448:string)  [unwired: 12 in]
            n230 = call <vilib>:"Add State(s) to Queue__JKI_lib_State_Machine.vi"("State(s) in Front (\"\")"=w448, "State(s) in (\"\")"=w457) -> ("States Out"=w458:string)  [unwired: 13 in]
          }
          event Panel Close? {
            # "Discard the event because we'll close the front panel ourselves in Macro: Exit"
            # "Close Panel button (pressed) Event\n(this executes Macro: Exit to terminate the VI)"
            n231 = event-data() -> ()  [unwired: 1 in, 1 out]
            n232 = event-data ("Event Filter Node")("Discard?"=TRUE) -> ()  [unwired: 1 in, 1 out]
            n233 = call <vilib>:"Add State(s) to Queue__JKI_lib_State_Machine.vi"("State(s) in Front (\"\")"="Macro: Exit", "State(s) in (\"\")"=w473) -> ("States Out"=w472:string)  [unwired: 13 in]
          }
        }
      }
      frame "---------- Macro ----------" {
        # "Do not put any code in this frame.\n(It is a separator no-op. You can make a copy of this frame to create a new Macro frame)"
        n234 = call <vilib>:"Add State(s) to Queue__JKI_lib_State_Machine.vi"("State(s) in (\"\")"=w478) -> ("States Out"=w477:string)  [unwired: 14 in]
      }
      frame "Macro: Initialize" {
        # "load Labjack setting 1st as it contaisn laser pin infortmation"
        # "start laser 1st, need 7.5s for laser to get ready"
        # "Initialization Macro\n(This is called once, when the VI starts)"
        n235 = call <vilib>:"Add State(s) to Queue__JKI_lib_State_Machine.vi"("State(s) in Front (\"\")"="UI: showDisclaimer\nUI: Cursor Set >> Busy\nData: Initialize\nInitialize Core Data\nUI: Initialize\nUI: Front Panel State >> Open\nMacro: LoadSysConfig\nTCP: InitializeNew\nTCP: checkSource\nUI: Update\nLabJack: Open\nLabJack: SetDefaultSub\nLED: OpenVIRef\nLED: BreathOrange\nUI: Update\n355 Laser: CheckControllerStatus\n355 Laser: Laser enable\n355 Laser: Dewelling>>500\n355 Laser: CheckControllerStatus\nUI: Update\nLabJack: 355_PWM_Config\nLabJack: AB_PWM_Config\nUI: Update", "State(s) in (\"\")"="Digitizer: Initialize\nDigitizer: Config\nUI: Update\n/*AimingBeam: Initialize\n/*AimingBeam: Set Status>>Enable\n/*AimingBeam: Set Current\nUI: Update\n355 Laser: Check Dewelling\nUI: Cursor Set >> Idle\nCase: GetID\nUI: Update\nTCP: SendSettingMacro\nCase: CreatFileStruct\nUI: Update\nData: loadLastUseMacro\nDeconEngine: InitilizeMacro\nGraph: SetXMultiplier\nGraph: AddCursors\nAPD: Initialize\nAPD: LoadFromSerial\nAPD: UpdateCtrlVLimit\nAPD: GetGainLimits\nPID: loadPID\nLED: BreathOff\nMacro: SysReadyForAq") -> ("States Out"=w479:string)  [unwired: 13 in]
        n236 = call <vilib>:"Add State(s) to Queue__JKI_lib_State_Machine.vi"("State(s) in Front (\"\")"=w479, "State(s) in (\"\")"=w487) -> ("States Out"=w486:string)  [unwired: 13 in]
        "Help" <- "Hover over controls to see help!" ("Help")
      }
      frame "Macro: LoadSysConfig" {
        # "System configuration Macro. [Covers: REQ15]\n(Load configurations for different component of the system)"
        n237 = call <vilib>:"Add State(s) to Queue__JKI_lib_State_Machine.vi"("State(s) in Front (\"\")"="SysConfig: Load Sys Config\nSysConfig: Load Digitizer Setting\nSysConfig: Load AB setting\nSysConfig: Load LJ Pinout\nSysConfig: Load 355 PWM\nSysConfig: LoadAPDSerialNumber\nSysConfig: LoadABVideoSetting\nSysConfig: LoadCursorLocation", "State(s) in (\"\")"=w493) -> ("States Out"=w492:string)  [unwired: 13 in]
      }
      frame "Macro: SysReadyForAq" {
        # "Macro for system ready\n(It is a separator no-op. You can make a copy of this frame to create a new Macro frame)"
        n238 = call <vilib>:"Add State(s) to Queue__JKI_lib_State_Machine.vi"("State(s) in Front (\"\")"="UI: ReadyForAquisition\nLED: Green" ("State(s) in Front (\"\")"), "State(s) in (\"\")"=w499) -> ("States Out"=w498:string)  [unwired: 13 in]
      }
      frame "Macro: Exit" {
        # "close LJ last"
        # "check whether hardware is initilized, if so close, if not do nothing"
        # "Exit Macro, close all hardware\n(This is called once, when the VI exits)"
        n239 = Unbundle By Name(w518) -> ("System Status.Digitizer"=w514:bool, "System Status.Aiming Beam"=w513:bool, "System Status.355 Laser"=w512:bool, "System Status.Labjack"=w503:bool, "Core.Close Panel on Exit?"=w507:bool)
        n240 = case shown="True" w514 {
          tunnel: ["" ("Empty String Constant") "Digitizer: Close"] -> w509
          frame False {
          }
          frame True {
          }
        }
        n241 = case shown="True" w503 {
          tunnel: ["" ("Empty String Constant") "LabJack: SetDefaultAndClose"] -> w500
          frame False {
          }
          frame True {
          }
        }
        n242 = case shown="True" w513 {
          tunnel: ["" ("Empty String Constant") "/*AimingBeam: Set Status >> Disable\n/*AimingBeam: Close"] -> w502
          frame False {
          }
          frame True {
          }
        }
        n243 = case shown="True" w512 {
          tunnel: ["" ("Empty String Constant") "355 Laser: Close\n355 Laser: CheckControllerStatus"] -> w501
          frame False {
          }
          frame True {
          }
        }
        n244 = Select(t="UI: Front Panel State >> Close", s=w507, f="" ("Empty String Constant")) -> (s? t:f=w504:string)
        n245 = call <vilib>:"Add State(s) to Queue__JKI_lib_State_Machine.vi"("State(s) in Front (\"\")"="TCP: Close", "State(s) in (\"\")"=w509, "State(s) at Back (\"\")"=w502) -> ("States Out"=w511:string)  [unwired: 12 in]
        n246 = call <vilib>:"Add State(s) to Queue__JKI_lib_State_Machine.vi"("State(s) in Front (\"\")"=w511, "State(s) in (\"\")"=w501, "State(s) at Back (\"\")"=w500) -> ("States Out"=w506:string)  [unwired: 12 in]
        n247 = call <vilib>:"Add State(s) to Queue__JKI_lib_State_Machine.vi"("State(s) in Front (\"\")"=w506, "State(s) in (\"\")"="UI: Update\nUI: Reset\nGraph: SaveCursorLoc\nLED: CloseVIRef\nQueue: Destory\nData: Cleanup\nExit", "State(s) at Back (\"\")"=w504) -> ("States Out"=w515:string)  [unwired: 12 in]
        n248 = call <vilib>:"Add State(s) to Queue__JKI_lib_State_Machine.vi"("State(s) in Front (\"\")"=w515, "State(s) in (\"\")"=w521) -> ("States Out"=w520:string)  [unwired: 13 in]
      }
      frame "---------- Data ----------" {
        # "Do not put any code in this frame.\n(It is a separator no-op. You can make a copy of this frame to create a new Data frame)"
        n249 = call <vilib>:"Add State(s) to Queue__JKI_lib_State_Machine.vi"("State(s) in (\"\")"=w534) -> ("States Out"=w533:string)  [unwired: 14 in]
      }
      frame "Data: Initialize" {
        w535 = path ""  # CaliPath
        w536 = dbl[] []  # V4
        w537 = dbl[][] []  # Ch4Data
        w538 = FALSE  # bothVidSourceAvail
        w539 = T1 {"Main Frame Grabber"=FALSE, "Side Frame Grabber"=FALSE, "Main Camera"=FALSE, "Side Camera"=FALSE}  # video source
        w540 = FALSE  # LED vi ref open?
        w542 = T22 {"DeCon Channel"=enum."1", "Scale Bar"=FALSE, "Scale Low"=3.0, "Scale High"=8.0, "ANSI"=20.0, "Radius"=1.0, "3D?"=FALSE, "Firefly?"=FALSE, "Pentero?"=FALSE}  # VideoConfig
        w543 = T26 {"Ch1APDSerial#"="", "Ch2APDSerial#"="", "Ch3APDSerial#"="", "Ch4APDSerial#"=""}  # APDSerialNum
        w544 = u32 0  # Aquisition Timer
        w545 = cluster{"RunID":i8, "BG ID":i8, "Cali ID":i8} {"RunID"=1, "BG ID"=1, "Cali ID"=1}  # IDs
        w546 = refnum<vi> refnum  # LED vi reference
        w547 = path ""  # TempPath
        w548 = T27 {"DataPath"=path "", "BG Path"=path "", "iRFPath"=path "", "CaliPath"=path ""}  # Pathes
        w550 = dbl[] []  # V3
        w551 = dbl[] []  # V2
        w552 = dbl[] []  # V1
        w554 = u32 0  # FastTimer
        w555 = u32 0  # SlowTimer
        w556 = dbl[][] []  # Ch3Data
        w557 = dbl[][] []  # Ch2Data
        w541 = dbl[][] []  # Ch1Data
        w560 = T2 {"Digitizer"=FALSE, "Labjack"=FALSE, "Aiming Beam"=FALSE, "355 Laser"=FALSE, "TCP/IP"=FALSE}  # System Status
        w561 = T28 {"DIO_EF_CLOCK1_DIVISOR"=16, "DIO_EF_CLOCK1_ROLL_VALUE"=25000, "DIO#_EF_INDEX"=0, "DIO#_EF_OPTIONS"=1, "DIO#_EF_CONFIG_A"=6250}  # AB PWM setting
        w562 = T5 {"Ch1 Bias"="TDA11", "Ch2 Bias"="DAC10", "Ch3 Bias"="DAC0", "Ch4 Bias"="DAC0", "355 PWM"="FIO0", "AimingBeam PWM"="FIO2", "Laser Ready"="FIO3", "Interlock"="FIO1", "Laser Start/Stop"="FIO1", "Red LED"="FIO1", "Green LED"="FIO1", "Foot Pedal"="DIO15"}  # LJ Pinout
        w563 = 0  # TCP attempt count
        w564 = u32 0  # Laser start tic
        w565 = refnum<k20>[] []  # niTClk sessions
        w566 = u32 0  # Last Trigger
        w567 = T28 {"DIO_EF_CLOCK1_DIVISOR"=16, "DIO_EF_CLOCK1_ROLL_VALUE"=25000, "DIO#_EF_INDEX"=0, "DIO#_EF_OPTIONS"=1, "DIO#_EF_CONFIG_A"=6250}  # 355 PWM setting
        w568 = T29 {"Aiming Beam COM Port"="COM3", "Min Current"=0.0, "Max Current"=63.0, "Default Current"=20.0, "Freq"=0}  # AB Cluster
        w569 = T30 {"resource name"="", "resource name 2"="", "Channel"=enum."Channel 0", "trigger source"="VAL_EXTERNAL", "trigger level"=0.5, "trigger delay"=1.35e-07, "min sample rate"=12500000000.0, "min record length"=2500, "vertical range"=1.0, "vertical offset"=-0.25, "Waveform to Avg"=2000}  # FLImDAQ
        w570 = FALSE  # SysRunning?
        w558 = path ""  # DefaultPath
        w571 = ""  # CaseID
        w572 = T4 {"Ch1Enable?"=FALSE, "Ch2Enable?"=FALSE, "Ch3Enable?"=FALSE, "Ch1AutoGain?"=FALSE, "Ch2AutoGain?"=FALSE, "Ch3AutoGain?"=FALSE, "AimingBeamEnable?"=FALSE}  # SysConfigCluster
        w573 = T31 {"Current VI Reference"=refnum, "Close Panel on Exit?"=FALSE}  # Core
        # "Initialize the shift-register data, here.\n(data names are defined by what you wire into the bundle function)"
        n250 = Bundle("Core"=w573, "SysConfigCluster"=w572, "System Status"=w560, "IDs"=w545, "CaseID"=w571, "DefaultPath"=w558, "Pathes"=w548, "FLImDAQ"=w569, "SysRunning?"=w570, "AB Cluster"=w568, "LJ Pinout"=w562, "355 PWM setting"=w567, "AB PWM setting"=w561, "Last Trigger"=w566, "niTClk sessions"=w565, "Laser start tic"=w564, "TCP attempt count"=w563, "Ch1Data"=w541, "Ch2Data"=w557, "Ch3Data"=w556, "Ch4Data"=w537, "V1"=w552, "V2"=w551, "V3"=w550, "V4"=w536, "SlowTimer"=w555, "FastTimer"=w554, "listener ID"=refnum<k5> refnum, "TempPath"=w547, "CaliPath"=w535, "LED vi reference"=w546, "Aquisition Timer"=w544, "APDSerialNum"=w543, "VideoConfig"=w542, "LED vi ref open?"=w540, "video source"=w539, "bothVidSourceAvail"=w538) -> (w549:T23)  [unwired: 1 in]
        n251 = call <vilib>:"Add State(s) to Queue__JKI_lib_State_Machine.vi"("State(s) in (\"\")"=w576) -> ("States Out"=w575:string)  [unwired: 14 in]
      }
      frame "Data: LoadAPDData" {
        w587 = T15 {"Ch1 iRF"=[], "Ch2 iRF"=[], "Ch3 iRF"=[], "Ch4 iRF"=[]}  # LastUseiRF
        # "only load the last iRF for the moment"
        # "Load APD detector data\n(It is a separator no-op. You can make a copy of this frame to create a new Data frame)"
        n252 = Unbundle By Name(w617) -> ("APDSerialNum.Ch1APDSerial#"=w616:string, "APDSerialNum.Ch2APDSerial#"=w590:string, "APDSerialNum.Ch3APDSerial#"=w589:string, "APDSerialNum.Ch4APDSerial#"=w585:string)
        n253 = call "CreatFromSerialNumNoRaw.vi"("error in (no error)"=w586, "APD Serial #"=w616) -> ("error out"=w614:errorcluster, "APDClass out"=w615:refnum<class "APDClass.lvclass">)  [unwired: 8 in]
        n254 = call "CreatFromSerialNumNoRaw.vi"("error in (no error)"=w586, "APD Serial #"=w590) -> ("error out"=w603:errorcluster, "APDClass out"=w604:refnum<class "APDClass.lvclass">)  [unwired: 8 in]
        n255 = call "CreatFromSerialNumNoRaw.vi"("error in (no error)"=w586, "APD Serial #"=w589) -> ("error out"=w596:errorcluster, "APDClass out"=w597:refnum<class "APDClass.lvclass">)  [unwired: 8 in]
        n256 = call "CreatFromSerialNumNoRaw.vi"("error in (no error)"=w586, "APD Serial #"=w585) -> ("error out"=w583:errorcluster, "APDClass out"=w584:refnum<class "APDClass.lvclass">)  [unwired: 8 in]
        n257 = call-dynamic "Read iRFData.vi"("error in (no error)"=w614, "APDClass in"=w615) -> ("iRFData"=w613:T32)  [unwired: 7 in, 2 out]
        n258 = call-dynamic "Read iRFData.vi"("error in (no error)"=w603, "APDClass in"=w604) -> ("iRFData"=w608:T32)  [unwired: 7 in, 2 out]
        n259 = call-dynamic "Read iRFData.vi"("error in (no error)"=w596, "APDClass in"=w597) -> ("iRFData"=w601:T32)  [unwired: 7 in, 2 out]
        n260 = call-dynamic "Read iRFData.vi"("error in (no error)"=w583, "APDClass in"=w584) -> ("iRFData"=w582:T32)  [unwired: 7 in, 2 out]
        n261 = Unbundle By Name(w613) -> ("iRFWFsAvg"=w612:dbl[][])
        n262 = Unbundle By Name(w608) -> ("iRFWFsAvg"=w607:dbl[][])
        n263 = Unbundle By Name(w601) -> ("iRFWFsAvg"=w600:dbl[][])
        n264 = Unbundle By Name(w582) -> ("iRFWFsAvg"=w578:dbl[][])
        n265 = Array Size(array=w612) -> (size(s)=w611:i32[])
        n266 = Array Size(array=w607) -> (size(s)=w602:i32[])
        n267 = Array Size(array=w600) -> (size(s)=w595:i32[])
        n268 = Array Size(array=w578) -> (size(s)=w579:i32[])
        n269 = Index Array(array=w611, index=1) -> (element=w609:i32)
        n270 = Index Array(array=w602, index=1) -> (element=w605:i32)
        n271 = Index Array(array=w595, index=1) -> (element=w598:i32)
        n272 = Index Array(array=w579, index=1) -> (element=w580:i32)
        n273 = Index Array(array=w612, index (row)=w609) -> (element=w594:dbl[])  [unwired: 1 in]
        n274 = Index Array(array=w607, index (row)=w605) -> (element=w593:dbl[])  [unwired: 1 in]
        n275 = Index Array(array=w600, index (row)=w598) -> (element=w592:dbl[])  [unwired: 1 in]
        n276 = Index Array(array=w578, index (row)=w580) -> (element=w577:dbl[])  [unwired: 1 in]
        n277 = Bundle(cluster=w587, "Ch1 iRF"=w594, "Ch2 iRF"=w593, "Ch3 iRF"=w592, "Ch4 iRF"=w577) -> (w588:T15)
        n278 = global write "GlobalVariables.vi" "LastUseiRF"(w588) -> ()
        n279 = call <vilib>:"Add State(s) to Queue__JKI_lib_State_Machine.vi"("State(s) in Front (\"\")"="UI: CaliAndiRFLoaded" ("State(s) in Front (\"\")"), "State(s) in (\"\")"=w620) -> ("States Out"=w619:string)  [unwired: 13 in]
      }
      frame "Data: loadLastUseiRF" {
        # "Load last use iRF.\n()"
        n280 = Unbundle By Name(w625) -> ("TempPath"=w624:path)
        n281 = Build Path(base path=w624, name or relative path="iRF.tdms") -> (appended path=w630:path)
        n282 = TDMS Open(11:w630) -> (0:w628:errorcluster, 3:w629:refnum<k34>)  [unwired: 6 in]
        n283 = TDMS Read(0:w629, 11:w628, 12:dbl[][] []) -> (4:w622:refnum<k34>, 10:w626:dbl[][], 15:w621:errorcluster)  [unwired: 5 in, 3 out]
        n284 = TDMS Close(8:w621, 11:w622) -> ()  [unwired: 2 out]
        n285 = case shown="No Error" w621 {
          tunnel: w626 -> [w649 _]
          tunnel: ["UI: CaliAndiRFLoaded" ("State(s) in Front (\"\")") "" ("Empty String Constant")] -> w623
          frame No Error {
            w636 = T15 {"Ch1 iRF"=[], "Ch2 iRF"=[], "Ch3 iRF"=[], "Ch4 iRF"=[]}  # LastUseiRF
            n286 = Index Array(array=w649, index (row)=0) -> (element=w645:dbl[])  [unwired: 1 in]
            n287 = Index Array(array=w649, index (row)=1) -> (element=w642:dbl[])  [unwired: 1 in]
            n288 = Index Array(array=w649, index (row)=2) -> (element=w639:dbl[])  [unwired: 1 in]
            n289 = Add Array Elements(numeric array=w645) -> (sum=w644:dbl)
            n290 = Add Array Elements(numeric array=w642) -> (sum=w641:dbl)
            n291 = Add Array Elements(numeric array=w639) -> (sum=w638:dbl)
            n292 = Divide(x=w645, y=w644) -> (x/y=w643:dbl[])
            n293 = Divide(x=w642, y=w641) -> (x/y=w640:dbl[])
            n294 = Divide(x=w639, y=w638) -> (x/y=w637:dbl[])
            n295 = Bundle(cluster=w636, "Ch1 iRF"=w643, "Ch2 iRF"=w640, "Ch3 iRF"=w637) -> (w648:T15)  [unwired: 1 in]
            n296 = Array Size(array=w645) -> (size(s)=→"iRF length":i32)
            n297 = global write "GlobalVariables.vi" "LastUseiRF"(w648) -> ()
          }
          frame Error {
          }
        }
        n298 = call <vilib>:"Add State(s) to Queue__JKI_lib_State_Machine.vi"("State(s) in Front (\"\")"=w623, "State(s) in (\"\")"=w635) -> ("States Out"=w634:string)  [unwired: 13 in]
      }
      frame "Data: loadSystemCali" {
        # "Load last use calibration.\n()"
        n299 = Unbundle By Name(w661) -> ("CaliPath"=w660:path)
        n300 = Build Path(base path=w660, name or relative path="Calibration.tdms") -> (appended path=w656:path)
        n301 = call "ReadBGorCali (SubVI).vi"("DataType"=enum16{"BG", "Cali"}."Cali", "error in (no error)"=w655, "file path in"=w656) -> ("error out"=w657:errorcluster, "CtrlVCluster"=w659:T33, "AvgDataCluster"=w658:T34)  [unwired: 6 in]
        n302 = case shown="No Error" w657 {
          tunnel: w659 -> [w680 _]
          tunnel: w658 -> [w679 _]
          frame No Error {
            w670 = T35 {"Ch1 WF"=[], "Ch2 WF"=[], "Ch3 WF"=[], "Ch4 WF"=[], "V1"=0.0, "V2"=0.0, "V3"=0.0, "V4"=0.0}  # SysCaliData
            n303 = Unbundle By Name(w679) -> ("Channel 1"=w678:dbl[], "Channel 2"=w677:dbl[], "Channel 3"=w676:dbl[], "Channel 4"=w669:dbl[])
            n304 = Unbundle By Name(w680) -> ("V 1"=w675:dbl[], "V 2"=w674:dbl[], "V 3"=w668:dbl[], "V 4"=w666:dbl[])
            n305 = Index Array(array=w675) -> (element=w673:dbl)  [unwired: 1 in]
            n306 = Index Array(array=w674) -> (element=w672:dbl)  [unwired: 1 in]
            n307 = Index Array(array=w668) -> (element=w671:dbl)  [unwired: 1 in]
            n308 = Index Array(array=w666) -> (element=w667:dbl)  [unwired: 1 in]
            n309 = Bundle By Name(cluster=w670, "Ch1 WF"=w678, "Ch2 WF"=w677, "Ch3 WF"=w676, "Ch4 WF"=w669, "V1"=w673, "V2"=w672, "V3"=w671, "V4"=w667) -> (w681:T35)
            n310 = global write "GlobalVariables.vi" "SysCaliData"(w681) -> ()
          }
          frame Error {
          }
        }
        n311 = call <vilib>:"Add State(s) to Queue__JKI_lib_State_Machine.vi"("State(s) in (\"\")"=w665) -> ("States Out"=w664:string)  [unwired: 14 in]
      }
      frame "Data: loadLastUseBG" {
        w684 = enum16{"write", "read"}."write" ("action")
        # "Load last use BG.\n()"
        n312 = Unbundle By Name(w704) -> ("TempPath"=w703:path)
        n313 = call "FLImDAQ_FGV.vi"() -> ("Read data"=w699:T6)  [unwired: 10 in, 1 out]
        n314 = Build Path(base path=w703, name or relative path="Background.tdms") -> (appended path=w702:path)
        n315 = call "ReadBGorCali (SubVI).vi"("DataType"=enum16{"BG", "Cali"}."BG", "error in (no error)"=w701, "file path in"=w702) -> ("error out"=w700:errorcluster, "AvgDataCluster"=w695:T34)  [unwired: 6 in, 1 out]
        n316 = Unbundle By Name(w695) -> ("Channel 1"=w687:dbl[], "Channel 2"=w694:dbl[], "Channel 3"=w686:dbl[], "Channel 4"=w683:dbl[])
        n317 = Unbundle By Name(w699) -> ("min record length"=w691:i32)
        n318 = Array Size(array=w686) -> (size(s)=w693:i32)
        "BG length" <- w693
        n319 = Equal?(x=w693, y=w691) -> (x = y?=w692:bool)
        n320 = Select(t="UI: BGLoaded" ("State(s) in Front (\"\")"), s=w692, f="UI: BGSizeError" ("State(s) in Front (\"\")")) -> (s? t:f=w696:string)
        n321 = case shown="False" w692 {
          tunnel: w687 -> [_ w715]
          tunnel: w694 -> [_ w714]
          tunnel: w686 -> [_ w713]
          tunnel: w691 -> [w710 _]
          tunnel: [w709 w715] -> w690
          tunnel: [w709 w714] -> w689
          tunnel: [w709 w713] -> w688
          tunnel: w683 -> [_ w712]
          tunnel: [w709 w712] -> w682
          frame False {
            # "If error set BG all 0, update UI"
            n322 = for {
              N: w710 -> [_]
              tunnel: [0.0] -> w709 mode=indexing
            }
          }
          frame True {
            # "If no error, check size match"
          }
        }
        n323 = call "BG4FGV.vi"("action"=w684, "BG4 in"=w682) -> ()  [unwired: 8 in, 2 out]
        n324 = call "BG3FGV.vi"("action"=w684, "BG3 in"=w688) -> ()  [unwired: 8 in, 2 out]
        n325 = call "BG1FGV.vi"("action"=w684, "BG1 in"=w690) -> ()  [unwired: 8 in, 2 out]
        n326 = call "BG2FGV.vi"("action"=w684, "BG2 in"=w689) -> ()  [unwired: 8 in, 2 out]
        n327 = call <vilib>:"Add State(s) to Queue__JKI_lib_State_Machine.vi"("State(s) in Front (\"\")"=w696, "State(s) in (\"\")"=w708) -> ("States Out"=w707:string)  [unwired: 13 in]
      }
      frame "Data: loadLastUseMacro" {
        # "Load last use BG and Cali and iRF.\n(It is a separator no-op. You can make a copy of this frame to create a new Data frame)"
        n328 = call <vilib>:"Add State(s) to Queue__JKI_lib_State_Machine.vi"("State(s) in Front (\"\")"="Data: loadLastUseBG\nData: loadSystemCali\nData: loadLastUseiRF\n/*Data: LoadAPDData" ("State(s) in Front (\"\")"), "State(s) in (\"\")"=w721) -> ("States Out"=w720:string)  [unwired: 13 in]
      }
      frame "Data: saveCalibration" {
        # "Average data and save calibration file. [Covers: REQ11]\n(It is a separator no-op. You can make a copy of this frame to create a new Data frame)"
        n329 = Unbundle By Name(w740) -> ("Ch1Data"=w739:dbl[][], "V1"=w738:dbl[], "Ch2Data"=w737:dbl[][], "V2"=w736:dbl[], "Ch3Data"=w735:dbl[][], "V3"=w734:dbl[], "Ch4Data"=w725:dbl[][], "V4"=w724:dbl[], "Pathes.CaliPath"=w743:path, "IDs.Cali ID"=w742:i8)
        n330 = Increment(x=w742) -> (x+1=w726:i8)
        n331 = Bundle("Ch1Data"=w739, "V1"=w738) -> (w733:cluster{"Ch1Data":dbl[][], "V1":dbl[]})  [unwired: 1 in]
        n332 = Bundle("Ch4Data"=w725, "V4"=w724) -> (w723:cluster{"Ch4Data":dbl[][], "V4":dbl[]})  [unwired: 1 in]
        n333 = Bundle("Ch2Data"=w737, "V2"=w736) -> (w732:cluster{"Ch2Data":dbl[][], "V2":dbl[]})  [unwired: 1 in]
        n334 = Bundle("Ch3Data"=w735, "V3"=w734) -> (w731:cluster{"Ch3Data":dbl[][], "V3":dbl[]})  [unwired: 1 in]
        n335 = Format Value(string ("")="Calibration" ("default name"), format string="%02d", value (0)=w726) -> (output string=w745:string)
        n336 = Build Path(base path=w743, name or relative path=w745) -> (appended path=w730:path)
        n337 = call "SaveBGorCali (SubVI).vi"("Channel1"=w733, "BG path"=w730, "DataType"=enum16{"BG", "Cali"}."Cali", "Channel 2"=w732, "Channel 3"=w731, "Channel 4"=w723, "error in (no error)"=w729, "SytemID"="UCDVetMed") -> ("error out"=w728:errorcluster)  [unwired: 7 in]
        n338 = call <vilib>:"Add State(s) to Queue__JKI_lib_State_Machine.vi"("State(s) in (\"\")"=w748) -> ("States Out"=w747:string)  [unwired: 14 in]
      }
      frame "Data: saveiRF" {
        w754 = enum16{"write", "read"}."read" ("action")
        # "Get iRF from decon stracture and save it on disk.\n(It is a separator no-op. You can make a copy of this frame to create a new Data frame)"
        n339 = Unbundle By Name(w771) -> ("TempPath"=w770:path)
        n340 = call "Ch1DeconEngineFGV.vi"("action(read)"=w754) -> ("Error Out"=w776:errorcluster, "Ch1DeconEngine out"=w777:refnum<class "LaguerreDeconEngineClass.lvclass">)  [unwired: 9 in]
        n341 = call "Ch2DeconEngineFGV.vi"("action(read)"=w754) -> ("Error Out"=w774:errorcluster, "Ch2DeconEngine out"=w775:refnum<class "LaguerreDeconEngineClass.lvclass">)  [unwired: 9 in]
        n342 = call "Ch3DeconEngineFGV.vi"("action(read)"=w754) -> ("Error Out"=w772:errorcluster, "Ch3DeconEngine out"=w773:refnum<class "LaguerreDeconEngineClass.lvclass">)  [unwired: 9 in]
        n343 = call "Ch4DeconEngineFGV.vi"("action(read)"=w754) -> ("Error Out"=w753:errorcluster, "Ch3DeconEngine out"=w752:refnum<class "LaguerreDeconEngineClass.lvclass">)  [unwired: 9 in]
        n344 = Build Path(base path=w770, name or relative path="iRF" ("default name")) -> (appended path=w768:path)
        n345 = call "getIRF.vi"("error in (no error)"=w753, "LaguerreDeconEngineClass in"=w752) -> ("iRF"=w751:dbl[])  [unwired: 7 in, 2 out]
        n346 = call "getIRF.vi"("error in (no error)"=w776, "LaguerreDeconEngineClass in"=w777) -> ("iRF"=w759:dbl[])  [unwired: 7 in, 2 out]
        n347 = call "getIRF.vi"("error in (no error)"=w774, "LaguerreDeconEngineClass in"=w775) -> ("iRF"=w758:dbl[])  [unwired: 7 in, 2 out]
        n348 = call "getIRF.vi"("error in (no error)"=w772, "LaguerreDeconEngineClass in"=w773) -> ("iRF"=w757:dbl[])  [unwired: 7 in, 2 out]
        n349 = TDMS Open(8:w767, 10:T16."create or replace" ("operation (0:open)"), 11:w768) -> (0:w764:errorcluster, 3:w765:refnum<k34>)  [unwired: 4 in]
        n350 = Bundle(cluster=T15 {"Ch1 iRF"=[], "Ch2 iRF"=[], "Ch3 iRF"=[], "Ch4 iRF"=[]} ("LastUseiRF"), "Ch1 iRF"=w759, "Ch2 iRF"=w758, "Ch3 iRF"=w757, "Ch4 iRF"=w751) -> (w755:T15)
        n351 = Build Array(w759, w758, w757, w751) -> (w763:dbl[][])
        n352 = global write "GlobalVariables.vi" "LastUseiRF"(w755) -> ()
        n353 = TDMS Write(0:w765, 5:"iRF" ("group name in (Untitled)"), 7:string[] ["Ch1", "Ch2", "Ch3", "Ch4"] ("channel name(s) in (Untitled)"), 9:w763, 11:w764) -> (4:w762:refnum<k34>, 15:w761:errorcluster)  [unwired: 1 in, 2 out]
        n354 = TDMS Close(8:w761, 11:w762) -> (0:w760:errorcluster)  [unwired: 1 out]
        n355 = call <vilib>:"Add State(s) to Queue__JKI_lib_State_Machine.vi"("State(s) in (\"\")"=w780) -> ("States Out"=w779:string)  [unwired: 14 in]
      }
      frame "Data: saveBGtoFGV" {
        w781 = enum16{"write", "read"}."write" ("action")
        # "Save BG and pass it to FGV.\n(save BG to disk and set it to FGV)"
        n356 = Unbundle By Name(w791) -> ("Ch1Data"=w790:dbl[][], "Ch2Data"=w789:dbl[][], "Ch3Data"=w788:dbl[][], "Ch4Data"=w783:dbl[][])
        n357 = call "AvgArrayTimeCritical.vi"("2D array"=w790) -> ("1D Avg"=w787:dbl[])  [unwired: 10 in]
        n358 = call "AvgArrayTimeCritical.vi"("2D array"=w789) -> ("1D Avg"=w786:dbl[])  [unwired: 10 in]
        n359 = call "AvgArrayTimeCritical.vi"("2D array"=w788) -> ("1D Avg"=w785:dbl[])  [unwired: 10 in]
        n360 = call "AvgArrayTimeCritical.vi"("2D array"=w783) -> ("1D Avg"=w782:dbl[])  [unwired: 10 in]
        n361 = call "BG1FGV.vi"("action"=w781, "BG1 in"=w787) -> ()  [unwired: 8 in, 2 out]
        n362 = call "BG2FGV.vi"("action"=w781, "BG2 in"=w786) -> ()  [unwired: 8 in, 2 out]
        n363 = call "BG3FGV.vi"("action"=w781, "BG3 in"=w785) -> ()  [unwired: 8 in, 2 out]
        n364 = call "BG4FGV.vi"("action"=w781, "BG4 in"=w782) -> ()  [unwired: 8 in, 2 out]
        n365 = call <vilib>:"Add State(s) to Queue__JKI_lib_State_Machine.vi"("State(s) in (\"\")"=w794) -> ("States Out"=w793:string)  [unwired: 14 in]
      }
      frame "Data: saveBGtoFile" {
        w816 = "Background" ("name or relative path")
        # "Save BG to file.\n(save BG to disk both data folder and temp folder)"
        n366 = Unbundle By Name(w820) -> ("Pathes.BG Path"=w813:path, "IDs.BG ID"=w812:i8, "Ch1Data"=w810:dbl[][], "V1"=w809:dbl[], "Ch2Data"=w808:dbl[][], "V2"=w807:dbl[], "Ch3Data"=w806:dbl[][], "V3"=w805:dbl[], "Ch4Data"=w797:dbl[][], "V4"=w796:dbl[], "TempPath"=w818:path)
        n367 = Increment(x=w812) -> (x+1=w817:i8)
        n368 = Format Value(string ("")=w816, format string="%02d", value (0)=w817) -> (output string=w815:string)
        n369 = Build Path(base path=w818, name or relative path=w816) -> (appended path=w799:path)
        n370 = call "File Dialog2"("start path"=w813, "prompt"="Please select BG name, DO NOT CANCEL!", "default name"=w815) -> ("selected path"=w800:path)  [unwired: 9 in, 3 out]
        n371 = Bundle("Ch1Data"=w810, "V1"=w809) -> (w804:cluster{"Ch1Data":dbl[][], "V1":dbl[]})  [unwired: 1 in]
        n372 = Bundle("Ch4Data"=w797, "V4"=w796) -> (w795:cluster{"Ch4Data":dbl[][], "V4":dbl[]})  [unwired: 1 in]
        n373 = Bundle("Ch2Data"=w808, "V2"=w807) -> (w803:cluster{"Ch2Data":dbl[][], "V2":dbl[]})  [unwired: 1 in]
        n374 = Bundle("Ch3Data"=w806, "V3"=w805) -> (w802:cluster{"Ch3Data":dbl[][], "V3":dbl[]})  [unwired: 1 in]
        n375 = Build Array(w800, w799) -> (w798:path[])
        n376 = for {
          tunnel: w804 -> [w831]
          tunnel: w803 -> [w830]
          tunnel: w802 -> [w829]
          shift-right: [w832] -> w811
          shift-left: w801 -> [w828]
          tunnel: w798 -> [w827] mode=indexing
          tunnel: w795 -> [w825]
          n377 = call "SaveBGorCali (SubVI).vi"("Channel1"=w831, "BG path"=w827, "DataType"=enum16{"BG", "Cali"}."BG", "Channel 2"=w830, "Channel 3"=w829, "Channel 4"=w825, "error in (no error)"=w828, "SytemID"="UCDVetMed") -> ("error out"=w832:errorcluster)  [unwired: 7 in]
        }
        n378 = call <vilib>:"Add State(s) to Queue__JKI_lib_State_Machine.vi"("State(s) in (\"\")"=w823) -> ("States Out"=w822:string)  [unwired: 14 in]
      }
      frame "Data: showBG" {
        # "Show BG in seperate window.\n()"
        n379 = call "showBG.vi"() -> ()  [unwired: 12 in]
        n380 = call <vilib>:"Add State(s) to Queue__JKI_lib_State_Machine.vi"("State(s) in (\"\")"=w837) -> ("States Out"=w836:string)  [unwired: 14 in]
      }
      frame "Data: irfAlignment" {
        w904 = enum16{"write", "read"}."write" ("action")
        # "do iRF alignment in this state\n(It is a separator no-op. You can make a copy of this frame to create a new Data frame)"
        n381 = Unbundle By Name(w882) -> ("Ch1Data"=w919:dbl[][], "Ch2Data"=w918:dbl[][], "Ch3Data"=w917:dbl[][], "Ch4Data"=w859:dbl[][])
        n382 = call "Ch1DeconEngineFGV.vi"("Error In"=w858) -> ("Error Out"=w915:errorcluster, "Ch1DeconEngine out"=w916:refnum<class "LaguerreDeconEngineClass.lvclass">)  [unwired: 9 in]
        n383 = call "Ch2DeconEngineFGV.vi"("Error In"=w858) -> ("Error Out"=w913:errorcluster, "Ch2DeconEngine out"=w914:refnum<class "LaguerreDeconEngineClass.lvclass">)  [unwired: 9 in]
        n384 = call "Ch3DeconEngineFGV.vi"("Error In"=w858) -> ("Error Out"=w911:errorcluster, "Ch3DeconEngine out"=w912:refnum<class "LaguerreDeconEngineClass.lvclass">)  [unwired: 9 in]
        n385 = call "Ch4DeconEngineFGV.vi"("Error In"=w858) -> ("Error Out"=w849:errorcluster, "Ch3DeconEngine out"=w848:refnum<class "LaguerreDeconEngineClass.lvclass">)  [unwired: 9 in]
        n386 = call "AvgArray.vi"("2D array in"=w918) -> ("1D Avg out"=w864:dbl[])  [unwired: 10 in]
        n387 = call "AvgArray.vi"("2D array in"=w917) -> ("1D Avg out"=w863:dbl[])  [unwired: 10 in]
        n388 = call "AvgArray.vi"("2D array in"=w859) -> ("1D Avg out"=w838:dbl[])  [unwired: 10 in]
        n389 = call "AvgArray.vi"("2D array in"=w919) -> ("1D Avg out"=w865:dbl[])  [unwired: 10 in]
        n390 = call "RemoveDCBG.vi"("WF in"=w865) -> ("DC"=w872:dbl, "WF out"=w862:dbl[])  [unwired: 8 in, 1 out]
        n391 = call "RemoveDCBG.vi"("WF in"=w864) -> ("DC"=w869:dbl, "WF out"=w875:dbl[])  [unwired: 8 in, 1 out]
        n392 = call "RemoveDCBG.vi"("WF in"=w863) -> ("DC"=w867:dbl, "WF out"=w874:dbl[])  [unwired: 8 in, 1 out]
        n393 = call "RemoveDCBG.vi"("WF in"=w838) -> ("DC"=w842:dbl, "WF out"=w840:dbl[])  [unwired: 8 in, 1 out]
        n394 = call "computeIRFAlignment.vi"("error in (no error)"=w915, "fIRF temp"=w862, "LaguerreDeconEngineClass in"=w916) -> ("error out"=w907:errorcluster, "LaguerreDeconEngineClass out"=w908:refnum<class "LaguerreDeconEngineClass.lvclass">)  [unwired: 6 in, 1 out]
        n395 = call "computeIRFAlignment.vi"("error in (no error)"=w913, "fIRF temp"=w875, "LaguerreDeconEngineClass in"=w914) -> ("error out"=w905:errorcluster, "LaguerreDeconEngineClass out"=w906:refnum<class "LaguerreDeconEngineClass.lvclass">)  [unwired: 6 in, 1 out]
        n396 = call "computeIRFAlignment.vi"("error in (no error)"=w911, "fIRF temp"=w874, "LaguerreDeconEngineClass in"=w912) -> ("error out"=w909:errorcluster, "LaguerreDeconEngineClass out"=w910:refnum<class "LaguerreDeconEngineClass.lvclass">)  [unwired: 6 in, 1 out]
        n397 = call "computeIRFAlignment.vi"("error in (no error)"=w849, "fIRF temp"=w840, "LaguerreDeconEngineClass in"=w848) -> ("error out"=w856:errorcluster, "LaguerreDeconEngineClass out"=w857:refnum<class "LaguerreDeconEngineClass.lvclass">)  [unwired: 6 in, 1 out]
        n398 = call "Ch1DeconEngineFGV.vi"("Error In"=w907, "action(read)"=w904, "Ch1DeconEngine in"=w908) -> ("Error Out"=w902:errorcluster, "Ch1DeconEngine out"=w903:refnum<class "LaguerreDeconEngineClass.lvclass">)  [unwired: 7 in]
        n399 = call "Ch2DeconEngineFGV.vi"("Error In"=w905, "action(read)"=w904, "Ch2DeconEngine in"=w906) -> ("Error Out"=w892:errorcluster, "Ch2DeconEngine out"=w893:refnum<class "LaguerreDeconEngineClass.lvclass">)  [unwired: 7 in]
        n400 = call "Ch3DeconEngineFGV.vi"("Error In"=w909, "action(read)"=w904, "Ch3DeconEngine in"=w910) -> ("Error Out"=w886:errorcluster, "Ch3DeconEngine out"=w887:refnum<class "LaguerreDeconEngineClass.lvclass">)  [unwired: 7 in]
        n401 = call "Ch3DeconEngineFGV.vi"("Error In"=w856, "Ch3DeconEngine in"=w857) -> ("Error Out"=w850:errorcluster, "Ch3DeconEngine out"=w851:refnum<class "LaguerreDeconEngineClass.lvclass">)  [unwired: 8 in]
        n402 = call "setfIRF.vi"("error in (no error)"=w886, "fIRF"=w874, "LaguerreDeconEngineClass in"=w887) -> ("error out"=w890:errorcluster, "LaguerreDeconEngineClass out"=w891:refnum<class "LaguerreDeconEngineClass.lvclass">)  [unwired: 7 in]
        n403 = call "setfIRF.vi"("error in (no error)"=w850, "fIRF"=w840, "LaguerreDeconEngineClass in"=w851) -> ("error out"=w854:errorcluster, "LaguerreDeconEngineClass out"=w855:refnum<class "LaguerreDeconEngineClass.lvclass">)  [unwired: 7 in]
        n404 = call "setfIRF.vi"("error in (no error)"=w892, "fIRF"=w875, "LaguerreDeconEngineClass in"=w893) -> ("error out"=w896:errorcluster, "LaguerreDeconEngineClass out"=w897:refnum<class "LaguerreDeconEngineClass.lvclass">)  [unwired: 7 in]
        n405 = call "setfIRF.vi"("error in (no error)"=w902, "fIRF"=w862, "LaguerreDeconEngineClass in"=w903) -> ("error out"=w900:errorcluster, "LaguerreDeconEngineClass out"=w901:refnum<class "LaguerreDeconEngineClass.lvclass">)  [unwired: 7 in]
        n406 = Unbundle By Name(w882) -> ("V1"=w861:dbl[], "V2"=w881:dbl[], "V3"=w880:dbl[], "V4"=w847:dbl[])
        n407 = call "computeLCs.vi"("error in (no error)"=w900, "LaguerreDeconClass in"=w901) -> ("error out"=w898:errorcluster, "LaguerreDeconClass out"=w899:refnum<class "LaguerreDeconEngineClass.lvclass">)  [unwired: 8 in]
        n408 = call "computeLCs.vi"("error in (no error)"=w896, "LaguerreDeconClass in"=w897) -> ("error out"=w894:errorcluster, "LaguerreDeconClass out"=w895:refnum<class "LaguerreDeconEngineClass.lvclass">)  [unwired: 8 in]
        n409 = call "computeLCs.vi"("error in (no error)"=w890, "LaguerreDeconClass in"=w891) -> ("error out"=w888:errorcluster, "LaguerreDeconClass out"=w889:refnum<class "LaguerreDeconEngineClass.lvclass">)  [unwired: 8 in]
        n410 = call "computeLCs.vi"("error in (no error)"=w854, "LaguerreDeconClass in"=w855) -> ("error out"=w852:errorcluster, "LaguerreDeconClass out"=w853:refnum<class "LaguerreDeconEngineClass.lvclass">)  [unwired: 8 in]
        n411 = call-poly <vilib>:"Mean.vi"("X"=w861) -> ("mean"=w860:dbl)  [unwired: 1 out]
        n412 = call-poly <vilib>:"Mean.vi"("X"=w847) -> ("mean"=w846:dbl)  [unwired: 1 out]
        n413 = call-poly <vilib>:"Mean.vi"("X"=w881) -> ("mean"=w879:dbl)  [unwired: 1 out]
        n414 = call "getFitting.vi"("error in (no error)"=w898, "LaguerreDeconEngineClass in"=w899) -> ("Fitting"=w871:dbl[])  [unwired: 7 in, 2 out]
        n415 = call "getFitting.vi"("error in (no error)"=w894, "LaguerreDeconEngineClass in"=w895) -> ("Fitting"=w868:dbl[])  [unwired: 7 in, 2 out]
        n416 = call "getFitting.vi"("error in (no error)"=w888, "LaguerreDeconEngineClass in"=w889) -> ("Fitting"=w844:dbl[])  [unwired: 7 in, 2 out]
        n417 = call "getFitting.vi"("error in (no error)"=w852, "LaguerreDeconEngineClass in"=w853) -> ("Fitting"=w843:dbl[])  [unwired: 7 in, 2 out]
        n418 = Add(x=w872, y=w871) -> (x+y=w873:dbl[])
        n419 = Add(x=w869, y=w868) -> (x+y=w870:dbl[])
        n420 = call-poly <vilib>:"Mean.vi"("X"=w880) -> ("mean"=w878:dbl)  [unwired: 1 out]
        n421 = Add(x=w867, y=w844) -> (x+y=w866:dbl[])
        n422 = Build Array(w865, w873) -> (w885:dbl[][])
        n423 = Build Array(w864, w870) -> (w884:dbl[][])
        n424 = Build Array(w863, w866) -> (w883:dbl[][])
        n425 = Add(x=w842, y=w843) -> (x+y=w841:dbl[])
        n426 = Bundle("mean"=w860, "mean"=w879, "mean"=w878, "mean"=w846) -> (w845:T36)  [unwired: 1 in]
        n427 = Build Array(w838, w841) -> (w839:dbl[][])
        n428 = call "Calib_and_iRFAlign_confirm.vi"("Current V"=w845, "Ch4 Data"=w839, "Ch3 Data"=w883, "Ch2 Data"=w884, "Ch1 Data"=w885) -> ("Save?"=w877:bool)  [unwired: 6 in]
        n429 = case shown="True" w877 {
          tunnel: ["" ("Empty String Constant") "Data: saveCalibration\nData: saveiRF\nRun: CaliIncrement"] -> w876
          frame False {
          }
          frame True {
            # "[Covers: REQ2]"
          }
        }
        n430 = call <vilib>:"Add State(s) to Queue__JKI_lib_State_Machine.vi"("State(s) in Front (\"\")"=w876, "State(s) in (\"\")"=w922) -> ("States Out"=w921:string)  [unwired: 13 in]
      }
      frame "Data: parseRunData" {
        # "All APD bias"
        # "flash queue"
        # "Ch3&4"
        # "Ch1&2"
        # "Flash data from queue and save it in structure\n()"
        n431 = Flush Queue(queue=w950, error in (no error)=w949) -> (remaining elements=w944:T37, error out=w945:errorcluster)  [unwired: 1 out]
        n432 = Flush Queue(queue=w955, error in (no error)=w949) -> (remaining elements=w953:cluster{"double data":dbl[][]}[], error out=w946:errorcluster)  [unwired: 1 out]
        n433 = Flush Queue(queue=w956, error in (no error)=w949) -> (remaining elements=w954:cluster{"double data":dbl[][]}[], error out=w947:errorcluster)  [unwired: 1 out]
        n434 = for {
          tunnel: w954 -> [w972] mode=indexing
          tunnel: [w970] -> w939 mode=concatenating
          tunnel: [w969] -> w940 mode=concatenating
          n435 = Unbundle By Name(w972) -> ("double data"=w971:dbl[][])
          n436 = call "SeperateChanData.vi"("Input (Ch1&2)"=w971) -> ("Ch1"=w970:dbl[][], "Ch2"=w969:dbl[][])
        }
        n437 = for {
          tunnel: w953 -> [w968] mode=indexing
          tunnel: [w967] -> w929 mode=concatenating
          tunnel: [w965] -> w930 mode=concatenating
          n438 = Unbundle By Name(w968) -> ("double data"=w966:dbl[][])
          n439 = call "SeperateChanData.vi"("Input (Ch1&2)"=w966) -> ("Ch1"=w967:dbl[][], "Ch2"=w965:dbl[][])
        }
        n440 = call "FLImDAQ_FGV.vi"() -> ("Read data"=w937:T6)  [unwired: 10 in, 1 out]
        n441 = Unbundle By Name(w937) -> ("Waveform to Avg"=w927:i16)
        n442 = for {
          tunnel: w944 -> [w964] mode=indexing
          tunnel: [w963] -> w936 mode=indexing
          tunnel: [w962] -> w934 mode=indexing
          tunnel: [w961] -> w932 mode=indexing
          tunnel: [w960] -> w928 mode=indexing
          n443 = Unbundle By Name(w964) -> ("V1"=w963:dbl, "V2"=w962:dbl, "V3"=w961:dbl, "V4"=w960:dbl)
        }
        n444 = call "DuplicateV(SubVI).vi"("Averaging"=w927, "V in"=w936) -> ("V out"=w935:dbl[])  [unwired: 9 in]
        n445 = Array Size(array=w929) -> (size(s)=→"data Size":i32[])
        n446 = call "DuplicateV(SubVI).vi"("Averaging"=w927, "V in"=w934) -> ("V out"=w933:dbl[])  [unwired: 9 in]
        n447 = call "DuplicateV(SubVI).vi"("Averaging"=w927, "V in"=w932) -> ("V out"=w931:dbl[])  [unwired: 9 in]
        n448 = call "DuplicateV(SubVI).vi"("Averaging"=w927, "V in"=w928) -> ("V out"=w925:dbl[])  [unwired: 9 in]
        n449 = Bundle By Name(cluster=w951, "Ch1Data"=w939, "Ch2Data"=w940, "Ch3Data"=w929, "Ch4Data"=w930, "V1"=w935, "V2"=w933, "V3"=w931, "V4"=w925) -> (w952:T23)
        n450 = Merge Errors(w947, w946, w945) -> (w948:errorcluster)
        n451 = Array Size(array=w935) -> (size(s)=→"V1 Size":i32)
        n452 = Array Size(array=w933) -> (size(s)=→"V2 Size":i32)
        n453 = Array Size(array=w931) -> (size(s)=→"V3 Size":i32)
        n454 = Array Size(array=w925) -> (size(s)=→"V4 Size":i32)
        n455 = call <vilib>:"Add State(s) to Queue__JKI_lib_State_Machine.vi"("State(s) in (\"\")"=w959) -> ("States Out"=w958:string)  [unwired: 14 in]
      }
      frame "Data: saveRunData" {
        w975 = T38 {"DataPath"=path "", "CaseID"="", "RunID"=0, "Ch1Data"=[], "Ch2Data"=[], "Ch3Data"=[], "Ch4Data"=[], "V1"=[], "V2"=[], "V3"=[], "V4"=[], "LaserRepRate"=0, "WFAverage"=0, "RunStartTime"=0}  # Data cluster
        # "Save FLIm data to disk.\n(Save to LV tdms file format)"
        n456 = Unbundle By Name(w986) -> ("Pathes.DataPath"=w982:path, "CaseID"=w994:string, "IDs.RunID"=w984:i8, "Ch1Data"=w993:dbl[][], "Ch2Data"=w992:dbl[][], "Ch3Data"=w981:dbl[][], "Ch4Data"=w974:dbl[][], "V1"=w976:dbl[], "V2"=w991:dbl[], "V3"=w990:dbl[], "V4"=w973:dbl[])
        n457 = call "FLImDAQ_FGV.vi"() -> ("Read data"=w979:T6)  [unwired: 10 in, 1 out]
        n458 = Unbundle By Name(w979) -> ("Waveform to Avg"=w978:i16)
        n459 = local read "RunStartTime"() -> (w977:u32)
        n460 = local read "Laser Rep Rate"() -> (w980:dbl)
        n461 = Increment(x=w984) -> (x+1=w983:i8)
        n462 = Bundle By Name(cluster=w975, "DataPath"=w982, "CaseID"=w994, "RunID"=w983, "Ch1Data"=w993, "Ch2Data"=w992, "Ch3Data"=w981, "Ch4Data"=w974, "V1"=w976, "V2"=w991, "V3"=w990, "V4"=w973, "LaserRepRate"=w980, "WFAverage"=w978, "RunStartTime"=w977) -> (w989:T38)
        n463 = call "SaveRunData(SubVI).vi"("Data cluster"=w989, "error in (no error)"=w988) -> ("error out"=w985:errorcluster)  [unwired: 13 in]
        n464 = flat-sequence {
          tunnel: w986 -> [w1002]
          tunnel: [w1001] -> w987
          tunnel: w985 -> [_]
          frame #0 {
            w999 = dbl[][] [] ("Ch1Data")
            w1000 = dbl[] [] ("V1")
            # "reset local data"
            n465 = Bundle By Name(cluster=w1002, "Ch1Data"=w999, "Ch2Data"=w999, "Ch3Data"=w999, "Ch4Data"=w999, "V1"=w1000, "V2"=w1000, "V3"=w1000, "V4"=w1000) -> (w1001:T23)
          }
        }
        n466 = case shown="No Error" w985 {
          tunnel: ["Run: Increment" "" ("Empty String Constant")] -> w995
          frame No Error {
          }
          frame Error {
          }
        }
        n467 = call <vilib>:"Add State(s) to Queue__JKI_lib_State_Machine.vi"("State(s) in Front (\"\")"=w995, "State(s) in (\"\")"=w998) -> ("States Out"=w997:string)  [unwired: 13 in]
      }
      frame "Data: Cleanup" {
        # "Cleanup any data and references, here.\n(this is called automatically, by the Macro: Exit)"
        n468 = Unbundle By Name(w1006) -> ("Core.Current VI Reference"=w1009:refnum<vi>)
        n469 = Close Reference(reference=w1009, error in (no error)=w1008) -> (error out=w1007:errorcluster)
        n470 = call <vilib>:"Add State(s) to Queue__JKI_lib_State_Machine.vi"("State(s) in (\"\")"=w1011) -> ("States Out"=w1010:string)  [unwired: 14 in]
      }
      frame "---------- Core ----------" {
        # "Do not put any code in this frame.\n(it is a separator no-op)"
        n471 = call <vilib>:"Add State(s) to Queue__JKI_lib_State_Machine.vi"("State(s) in (\"\")"=w1016) -> ("States Out"=w1015:string)  [unwired: 14 in]
      }
      frame Default {
        w1027 = 42 items=["No error", "Argument error", "Memory is full", "Out of zone", "End of file", "File already open", "Generic file I/O error", "File not found", "File permission error", "Disk is full", "Duplicate path", "Too many files open", "System feature not enabled", "Resource file not found", "Cannot add resource", "Resource not found", "Image not found", "Image memory error", "Pen does not exist", "Config type invalid", "Config token not found", "Config parse error", "Config memory error", "Bad external code format", "Bad external code offset", "External code not present", "Null window", "Destroy window error", "Null menu", "Print aborted", "Bad print record", "Print driver error", "Windows error during printing", "Memory error during printing", "Print dialog error", "Generic print error", "Invalid device refnum", "Device not found", "Device parameter error", "Device unit error", "Cannot open device", "Device call aborted", "Generic error", "Cancelled by user", "Object ID too low", "Object ID too high", "Object not in heap", "Unknown heap", "Unknown object (invalid DefProc)", "Unknown object (DefProc not in table)", "Message out of range", "Invalid (null) method", "Unknown message", "Manager call not supported", "Bad address", "Network operation in progress", "Network operation timed out", "Connection is busy", "Network attribute not supported", "Network error", "Address in use", "System out of memory", "Connection aborted", "Connection refused", "Not connected", "Already connected", "Connection closed", "Initialization error (interapplication manager)", "Bad occurrence", "Wait on unbound occurrence handler", "Occurrence queue overflow", "Datalog type conflict", "Unused", "Unrecognized type (interapplication manager)", "Memory corrupt", "Failed to make temporary DLL", "Old CIN version", "Drag socket not found", "Failed to load drop-object", "Failed to register OLE object", "Failed to release OLE object", "Format specifier type mismatch", "Unknown format specifier", "Too few format specifiers", "Too many format specifiers", "Scan failed", "Newer CIN version", "Error converting to variant", "Runtime menu error", "Password tampered", "Variant attribute not found", "Incompatible variant data type", "Event data is not available", "Event Store is not present", "Occurrence is not found", "Event Queue is not created", "Event info is not available", "Refnum passed is NULL", "Error retrieving Class GUID", "Error retrieving CoClass GUID", "Error retrieving TypeLib GUID.", "Bad built application magic bytes.", "Specific driver is different from the specific driver associated with the Logical Name.", "There is no session opened to the class driver.", "Max Error", "MAX - Error with config objects", "MAX - Error loading configuration", "MAX - Group not supported"]
        # "Current State"
        # "Do not delete, rename, or modify this frame.\n(this is used to capture unhandled states and typos)"
        # "Handle mistyped state name (developer tool)"
        n472 = Format Into String(format string="Software Exception: Unhandled State \"%s\"." ("message"), error in=w1023, w1018) -> (resulting string=w1026:string, error out=w1025:errorcluster)  [unwired: 1 in]
        n473 = call <vilib>:"Error Cluster From Error Code.vi"("show call chain? (False)"=TRUE, "error in (no error)"=w1025, "error message (\"\")"=w1026, "error code (0)"=w1027) -> ("error out"=w1024:errorcluster)  [unwired: 5 in]
        n474 = call <vilib>:"Add State(s) to Queue__JKI_lib_State_Machine.vi"("State(s) in (\"\")"=w1022) -> ("States Out"=w1021:string)  [unwired: 14 in]
      }
      frame "Initialize Core Data" {
        # "Build default path based on the location of project"
        # "Do not delete, rename, or modify this frame.\n(this is used to determine panel behavior on exit)"
        # "originally closed?"
        # "exe?"
        # "If panel starts closed or is an EXE, then close it when we exit"
        n475 = call <vilib>:"Application Directory.vi"() -> ("Application Directory"=w1031:path)
        n476 = property on="Property Node" class="App"() -> ("App.Kind"=w1045:T18)  [unwired: 2 in, 2 out]
        n477 = property on="Property Node" class="VI"() -> ("FP.State"=w1039:T17)  [unwired: 2 in, 2 out]
        n478 = control-ref of="Current VI Reference"() -> (w1040:refnum<vi>)
        n479 = Equal?(x=w1039, y=T17."Closed" ("Front Panel Window:State")) -> (x = y?=w1037:bool)
        n480 = Equal?(x=w1045, y=T18."Run Time System" ("Application:Kind")) -> (x = y?=w1043:bool)
        n481 = Build Path(base path=w1031, name or relative path="Data") -> (appended path=w1035:path)
        n482 = Build Path(base path=w1031, name or relative path="SystemTemp") -> (appended path=w1032:path)
        n483 = Build Path(base path=w1031, name or relative path="SystemCalibrationFile") -> (appended path=w1029:path)
        n484 = Or(x=w1037, y=w1043) -> (x .or. y?=w1041:bool)
        n485 = Bundle By Name(cluster=w1042, "Core.Current VI Reference"=w1040, "Core.Close Panel on Exit?"=w1041, "DefaultPath"=w1035, "TempPath"=w1032, "CaliPath"=w1029) -> (w1047:T23)
        n486 = call <vilib>:"Add State(s) to Queue__JKI_lib_State_Machine.vi"("State(s) in (\"\")"=w1049) -> ("States Out"=w1048:string)  [unwired: 14 in]
      }
      frame "Error Handler" {
        # "Unhandled Error -- Display it"
        # "Handle any errors here.\nYou can also output any states to clean-up after errors occur"
        # "Clear error"
        n487 = Unbundle By Name(w1050) -> ("code"=w1052:i32)
        n488 = case shown="Default" w1052 {
          tunnel: ["Macro: Exit" w1062 w1068] -> w1051
          tunnel: w1050 -> [w1058 _ _]
          frame Default {
            w1060 = T39 1 items=["no dialog", "OK message", "continue or stop message", "OK message + warnings", "continue/stop + warnings"] ("type of dialog (OK msg:1)")
            n489 = call <vilib>:"General Error Handler.vi"("type of dialog (OK msg:1)"=w1060, "error in (no error)"=w1058) -> ()  [unwired: 9 in, 5 out]
          }
          frame 5002 {
            n490 = Two Button Dialog(message="Laser interlock open! Please close interlock and try again! ", 1:"Safely Shutdown" ("F button name (\"Cancel\")"), 2:"OK" ("T button name (\"OK\")")) -> (T button?=w1063:bool)
            n491 = case shown="True" w1063 {
              tunnel: ["Macro: Exit" "355 Laser: CheckControllerStatus"] -> w1062
              frame False {
              }
              frame True {
              }
            }
          }
          frame 5001 {
            n492 = Two Button Dialog(message="Unable to connect to imaging computer, do you want to run data aquisiton alone? ", 1:"No" ("F button name (\"Cancel\")"), 2:"Yes" ("T button name (\"OK\")")) -> (T button?=w1069:bool)
            n493 = case shown="False" w1069 {
              tunnel: ["Macro: Exit" "" ("Empty String Constant")] -> w1068
              frame False {
              }
              frame True {
              }
            }
          }
        }
        n494 = call <vilib>:"Add State(s) to Queue__JKI_lib_State_Machine.vi"("State(s) in Front (\"\")"=w1051, "State(s) in (\"\")"=w1057) -> ("States Out"=w1056:string)  [unwired: 13 in]
      }
      frame "Exit" {
        # "Do not put any code in this frame.\n(No errors that occur here will be handled.)"
        n495 = call <vilib>:"Add State(s) to Queue__JKI_lib_State_Machine.vi"("State(s) in (\"\")"=w1080) -> ("States Out"=w1079:string)  [unwired: 14 in]
      }
      frame "---------- Case ----------" {
        # "Template Separator\n(You can make a copy of, or modify, this frame)"
        n496 = call <vilib>:"Add State(s) to Queue__JKI_lib_State_Machine.vi"("State(s) in (\"\")"=w1085) -> ("States Out"=w1084:string)  [unwired: 14 in]
      }
      frame "Case: getCaliID" {
        # "Get Calibration file #\n(You can make a copy of, or modify, this frame)"
        n497 = Unbundle By Name(w1086) -> ("Pathes.CaliPath"=w1089:path)
        n498 = call <vilib>:"Recursive File List.vi"("pattern"="*.tdms", "Treat LLBs as Folders?"=FALSE, "Folder Path"=w1089) -> ("All Files in Dir"=w1094:path[])  [unwired: 4 in, 4 out]
        n499 = for {
          tunnel: w1094 -> [w1104] mode=indexing
          tunnel: [w1103] -> w1093 mode=indexing
          tunnel: "Calibration" -> [w1100]
          n500 = Strip Path(path=w1104) -> (name=w1101:string)  [unwired: 1 out]
          n501 = Search and Replace String(input string=w1101, search string=w1100) -> (result string=w1099:string)  [unwired: 6 in, 3 out]
          n502 = Scan From String(format string="%d" ("string"), input string=w1099) -> (output 1=w1103:i32)  [unwired: 3 in, 3 out]
        }
        n503 = Array Max & Min(array=w1093) -> (max value=w1092:i32)  [unwired: 3 out]
        n504 = Bundle By Name(cluster=w1086, "IDs.Cali ID"=w1092) -> (w1087:T23)
        n505 = call <vilib>:"Add State(s) to Queue__JKI_lib_State_Machine.vi"("State(s) in (\"\")"=w1098) -> ("States Out"=w1097:string)  [unwired: 14 in]
      }
      frame "Case: getBGID" {
        # "Get background #\n(You can make a copy of, or modify, this frame)"
        n506 = Unbundle By Name(w1107) -> ("Pathes.BG Path"=w1112:path)
        n507 = call <vilib>:"Recursive File List.vi"("pattern"="*.tdms", "Treat LLBs as Folders?"=FALSE, "Folder Path"=w1112) -> ("All Files in Dir"=w1110:path[])  [unwired: 4 in, 4 out]
        n508 = for {
          tunnel: w1110 -> [w1127] mode=indexing
          tunnel: "Background" ("name or relative path") -> [w1125]
          shift-right: [w1118] -> w1105
          shift-left: 0 -> [w1122]
          n509 = Strip Path(path=w1127) -> (name=w1126:string)  [unwired: 1 out]
          n510 = Search and Replace String(input string=w1126, search string=w1125) -> (number of replacements=w1124:i32)  [unwired: 6 in, 3 out]
          n511 = Greater Than 0?(x=w1124) -> (x > 0?=w1123:bool)
          n512 = Select(t=1, s=w1123, f=0) -> (s? t:f=w1121:i32)
          n513 = Add(x=w1121, y=w1122) -> (x+y=w1118:i32)
        }
        n514 = Bundle By Name(cluster=w1107, "IDs.BG ID"=w1105) -> (w1108:T23)
        n515 = call <vilib>:"Add State(s) to Queue__JKI_lib_State_Machine.vi"("State(s) in (\"\")"=w1117) -> ("States Out"=w1116:string)  [unwired: 14 in]
      }
      frame "Case: getRunID" {
        # "Check folder for run ID\n(You can make a copy of, or modify, this frame)"
        n516 = Unbundle By Name(w1137) -> ("Pathes.DataPath"=w1136:path, "CaseID"=w1132:string)
        n517 = Build Array("Background" ("name or relative path"), "Calibration", "3DScanData" ("element")) -> (w1142:string[])
        n518 = call <vilib>:"Recursive File List.vi"("Folders to Exclude"=w1142, "pattern"="*.tdms", "Treat LLBs as Folders?"=FALSE, "Folder Path"=w1136) -> ("All Files in Dir"=w1133:path[])  [unwired: 3 in, 4 out]
        n519 = for {
          tunnel: w1133 -> [w1151] mode=indexing
          tunnel: [w1150] -> w1139 mode=indexing
          tunnel: w1132 -> [w1147]
          n520 = Strip Path(path=w1151) -> (name=w1148:string)  [unwired: 1 out]
          n521 = Search and Replace String(input string=w1148, search string=w1147) -> (result string=w1146:string)  [unwired: 6 in, 3 out]
          n522 = Scan From String(format string="_%d" ("string"), input string=w1146) -> (output 1=w1150:i32)  [unwired: 3 in, 3 out]
        }
        n523 = Array Max & Min(array=w1139) -> (max value=w1130:i32)  [unwired: 3 out]
        n524 = Bundle By Name(cluster=w1137, "IDs.RunID"=w1130) -> (w1138:T23)
        n525 = call "RunIDFGV.vi"("Error In"=w1128, "RunID in"=w1130) -> ("Error Out"=w1129:errorcluster)  [unwired: 8 in, 1 out]
        n526 = call <vilib>:"Add State(s) to Queue__JKI_lib_State_Machine.vi"("State(s) in (\"\")"=w1145) -> ("States Out"=w1144:string)  [unwired: 14 in]
      }
      frame "Case: CreatFileStruct" {
        # "Creat case file structure"
        n527 = Unbundle By Name(w1165) -> ("DefaultPath"=w1171:path, "CaseID"=w1158:string)
        n528 = Build Path(base path=w1171, name or relative path=w1158) -> (appended path=w1170:path)
        n529 = call <vilib>:"Check if File or Folder Exists.vi"("error in (no error)"=w1164, "path"=w1170) -> ("error out"=w1167:errorcluster, "file or folder exists?"=w1169:bool, "dup path"=w1168:path)  [unwired: 7 in]
        n530 = case shown="True" w1169 {
          tunnel: w1168 -> [w1188 w1196]
          tunnel: w1167 -> [w1186 w1191]
          tunnel: [w1180 w1196] -> w1156
          tunnel: [w1184 w1198] -> w1155
          tunnel: [u32 0 u32 0] -> w1154
          tunnel: [w1182 w1201] -> w1162
          tunnel: "Background" ("name or relative path") -> [w1181 w1193]
          tunnel: "Calibration" -> [w1179 w1192]
          tunnel: [w1175 w1194] -> w1159
          tunnel: w1158 -> [_ _]
          tunnel: ["" ("Empty String Constant") "Case: getRunID\nCase: getBGID\nCase: getCaliID\nUI: Update"] -> w1157
          frame False {
            # "Folder not exist. Creat folders."
            n531 = Create Folder(path (use dialog)=w1188, error in=w1186) -> (created path=w1180:path, error out=w1177:errorcluster)  [unwired: 1 in, 1 out]
            n532 = Build Path(base path=w1180, name or relative path=w1179) -> (appended path=w1178:path)
            n533 = Build Path(base path=w1180, name or relative path=w1181) -> (appended path=w1187:path)
            n534 = Create Folder(path (use dialog)=w1187, error in=w1177) -> (created path=w1182:path, error out=w1183:errorcluster)  [unwired: 1 in, 1 out]
            n535 = Create Folder(path (use dialog)=w1178, error in=w1177) -> (created path=w1175:path, error out=w1176:errorcluster)  [unwired: 1 in, 1 out]
            n536 = Merge Errors(w1183, w1176) -> (w1184:errorcluster)
          }
          frame True {
            # "Folder exsit, check file #"
            n537 = Build Path(base path=w1196, name or relative path=w1192) -> (appended path=w1197:path)
            n538 = Build Path(base path=w1196, name or relative path=w1193) -> (appended path=w1202:path)
            n539 = call <vilib>:"Check if File or Folder Exists.vi"("path"=w1197) -> ("file or folder exists?"=w1195:bool, "dup path"=w1194:path)  [unwired: 8 in, 1 out]
            n540 = call <vilib>:"Check if File or Folder Exists.vi"("path"=w1202) -> ("file or folder exists?"=w1200:bool, "dup path"=w1201:path)  [unwired: 8 in, 1 out]
            n541 = And(x=w1200, y=w1195) -> (x .and. y?=w1199:bool)
            n542 = case shown="False" w1199 {
              tunnel: w1191 -> [_ w1204]
              tunnel: [errorcluster {"status"=TRUE, "code"=5003, "source"="File structure error."} ("error out") w1204] -> w1198
              frame False {
              }
              frame True {
              }
            }
          }
        }
        n543 = Bundle By Name(cluster=w1165, "Pathes.DataPath"=w1156, "Pathes.BG Path"=w1162, "Pathes.CaliPath"=w1159, "IDs.RunID"=w1154, "IDs.BG ID"=w1154, "IDs.Cali ID"=w1154) -> (w1166:T23)
        n544 = call "DataRootPathFGV.vi"("Error In"=w1155, "PathIn"=w1156) -> ("Error Out"=w1153:errorcluster)  [unwired: 8 in, 1 out]
        n545 = call "RunIDFGV.vi"("Error In"=w1153, "RunID in"=w1154) -> ("Error Out"=w1152:errorcluster)  [unwired: 8 in, 1 out]
        n546 = call <vilib>:"Add State(s) to Queue__JKI_lib_State_Machine.vi"("State(s) in Front (\"\")"=w1157, "State(s) in (\"\")"=w1173) -> ("States Out"=w1172:string)  [unwired: 13 in]
      }
      frame "Case: GetID" {
        # "Template Separator\n(You can make a copy of, or modify, this frame)"
        n547 = call "set_subjectID.vi"() -> ("subject_id"=w1205:string)  [unwired: 10 in]
        n548 = Bundle By Name(cluster=w1207, "CaseID"=w1205) -> (w1208:T23)
        n549 = call <vilib>:"Add State(s) to Queue__JKI_lib_State_Machine.vi"("State(s) in (\"\")"=w1211) -> ("States Out"=w1210:string)  [unwired: 14 in]
      }
      frame "---------- DeconEngine ----------" {
        # "start data aquisition and then set irfAligh to ture and decon channel to 1,2 and 3."
        # "Template Separator\n(You can make a copy of, or modify, this frame)"
        n550 = call <vilib>:"Add State(s) to Queue__JKI_lib_State_Machine.vi"("State(s) in (\"\")"=w1216) -> ("States Out"=w1215:string)  [unwired: 14 in]
      }
      frame "DeconEngine: InitilizeMacro" {
        # "start data aquisition and then set irfAligh to ture and decon channel to 1,2 and 3."
        # "Initilize Decon Engine for all channel\n(You can make a copy of, or modify, this frame)"
        n551 = call <vilib>:"Add State(s) to Queue__JKI_lib_State_Machine.vi"("State(s) in Front (\"\")"="DeconEngine: InitializeCh1\nDeconEngine: InitializeCh2\nDeconEngine: InitializeCh3\nDeconEngine: InitializeCh4" ("State(s) in Front (\"\")"), "State(s) in (\"\")"=w1222) -> ("States Out"=w1221:string)  [unwired: 13 in]
      }
      frame "DeconEngine: InitializeCh1" {
        w1246 = refnum<class "LaguerreDeconEngineClass.lvclass"> refnum  # Ch1DeconObj
        # "Initilize Laguerre Deconvolution engine Object\n(You can make a copy of, or modify, this frame)"
        n552 = call "FLImDAQ_FGV.vi"("error in (no error)"=w1231) -> ("error out"=w1242:errorcluster, "Read data"=w1241:T6)  [unwired: 9 in]
        n553 = global read "GlobalVariables.vi" "LastUseiRF"() -> (w1224:T15)
        n554 = Unbundle By Name(w1241) -> ("min record length"=w1240:i32)
        n555 = call "setLaguerreOrder.vi"("error in (no error)"=w1242, "LaguerreOrder"=u32 12, "LaguerreDeconClass in"=w1246) -> ("error out"=w1243:errorcluster, "LaguerreDeconClass out"=w1244:refnum<class "LaguerreDeconEngineClass.lvclass">)  [unwired: 7 in]
        n556 = Unbundle By Name(w1224) -> ("Ch1 iRF"=w1223:dbl[])
        n557 = call "setDataLength.vi"("error in (no error)"=w1243, "dataLength"=w1240, "LaguerreDeconClass in"=w1244) -> ("error out"=w1239:errorcluster, "LaguerreDeconClass out"=w1238:refnum<class "LaguerreDeconEngineClass.lvclass">)  [unwired: 7 in]
        n558 = call "setIRF.vi"("error in (no error)"=w1239, "iRF"=w1223, "LaguerreDeconClass in"=w1238) -> ("error out"=w1236:errorcluster, "LaguerreDeconClass out"=w1237:refnum<class "LaguerreDeconEngineClass.lvclass">)  [unwired: 7 in]
        n559 = call "computeAlpha.vi"("error in (no error)"=w1236, "LaguerreDeconClass in"=w1237) -> ("error out"=w1234:errorcluster, "LaguerreDeconClass out"=w1235:refnum<class "LaguerreDeconEngineClass.lvclass">)  [unwired: 8 in]
        n560 = call "dataInitilize.vi"("error in (no error)"=w1234, "LaguerreDeconClass in"=w1235) -> ("error out"=w1232:errorcluster, "LaguerreDeconClass out"=w1233:refnum<class "LaguerreDeconEngineClass.lvclass">)  [unwired: 8 in]
        n561 = call "computeDeconMatrix.vi"("error in (no error)"=w1232, "LaguerreDeconClass in"=w1233) -> ("error out"=w1228:errorcluster, "LaguerreDeconClass out"=w1230:refnum<class "LaguerreDeconEngineClass.lvclass">)  [unwired: 8 in]
        n562 = call "Ch1DeconEngineFGV.vi"("Error In"=w1228, "action(read)"=enum16{"write", "read"}."write" ("action"), "Ch1DeconEngine in"=w1230) -> ("Error Out"=w1227:errorcluster)  [unwired: 7 in, 1 out]
        n563 = call <vilib>:"Add State(s) to Queue__JKI_lib_State_Machine.vi"("State(s) in (\"\")"=w1248) -> ("States Out"=w1247:string)  [unwired: 14 in]
      }
      frame "DeconEngine: InitializeCh2" {
        w1272 = refnum<class "LaguerreDeconEngineClass.lvclass"> refnum  # Ch2DeconObj
        # "Initilize Laguerre Deconvolution engine Object\n(You can make a copy of, or modify, this frame)"
        n564 = global read "GlobalVariables.vi" "LastUseiRF"() -> (w1250:T15)
        n565 = call "FLImDAQ_FGV.vi"("error in (no error)"=w1258) -> ("error out"=w1251:errorcluster, "Read data"=w1268:T6)  [unwired: 9 in]
        n566 = call "setLaguerreOrder.vi"("error in (no error)"=w1251, "LaguerreOrder"=u32 12, "LaguerreDeconClass in"=w1272) -> ("error out"=w1269:errorcluster, "LaguerreDeconClass out"=w1270:refnum<class "LaguerreDeconEngineClass.lvclass">)  [unwired: 7 in]
        n567 = Unbundle By Name(w1268) -> ("min record length"=w1267:i32)
        n568 = Unbundle By Name(w1250) -> ("Ch2 iRF"=w1249:dbl[])
        n569 = call "setDataLength.vi"("error in (no error)"=w1269, "dataLength"=w1267, "LaguerreDeconClass in"=w1270) -> ("error out"=w1266:errorcluster, "LaguerreDeconClass out"=w1265:refnum<class "LaguerreDeconEngineClass.lvclass">)  [unwired: 7 in]
        n570 = call "setIRF.vi"("error in (no error)"=w1266, "iRF"=w1249, "LaguerreDeconClass in"=w1265) -> ("error out"=w1263:errorcluster, "LaguerreDeconClass out"=w1264:refnum<class "LaguerreDeconEngineClass.lvclass">)  [unwired: 7 in]
        n571 = call "computeAlpha.vi"("error in (no error)"=w1263, "LaguerreDeconClass in"=w1264) -> ("error out"=w1261:errorcluster, "LaguerreDeconClass out"=w1262:refnum<class "LaguerreDeconEngineClass.lvclass">)  [unwired: 8 in]
        n572 = call "dataInitilize.vi"("error in (no error)"=w1261, "LaguerreDeconClass in"=w1262) -> ("error out"=w1259:errorcluster, "LaguerreDeconClass out"=w1260:refnum<class "LaguerreDeconEngineClass.lvclass">)  [unwired: 8 in]
        n573 = call "computeDeconMatrix.vi"("error in (no error)"=w1259, "LaguerreDeconClass in"=w1260) -> ("error out"=w1255:errorcluster, "LaguerreDeconClass out"=w1257:refnum<class "LaguerreDeconEngineClass.lvclass">)  [unwired: 8 in]
        n574 = call "Ch2DeconEngineFGV.vi"("Error In"=w1255, "action(read)"=enum16{"write", "read"}."write" ("action"), "Ch2DeconEngine in"=w1257) -> ("Error Out"=w1254:errorcluster)  [unwired: 7 in, 1 out]
        n575 = call <vilib>:"Add State(s) to Queue__JKI_lib_State_Machine.vi"("State(s) in (\"\")"=w1274) -> ("States Out"=w1273:string)  [unwired: 14 in]
      }
      frame "DeconEngine: InitializeCh3" {
        w1275 = refnum<class "LaguerreDeconEngineClass.lvclass"> refnum  # Ch3DeconObj
        # "Initilize Laguerre Deconvolution engine Object\n(You can make a copy of, or modify, this frame)"
        n576 = call "FLImDAQ_FGV.vi"("error in (no error)"=w1284) -> ("error out"=w1295:errorcluster, "Read data"=w1294:T6)  [unwired: 9 in]
        n577 = global read "GlobalVariables.vi" "LastUseiRF"() -> (w1277:T15)
        n578 = call "setLaguerreOrder.vi"("error in (no error)"=w1295, "LaguerreOrder"=u32 12, "LaguerreDeconClass in"=w1275) -> ("error out"=w1296:errorcluster, "LaguerreDeconClass out"=w1297:refnum<class "LaguerreDeconEngineClass.lvclass">)  [unwired: 7 in]
        n579 = Unbundle By Name(w1294) -> ("min record length"=w1293:i32)
        n580 = Unbundle By Name(w1277) -> ("Ch3 iRF"=w1276:dbl[])
        n581 = call "setDataLength.vi"("error in (no error)"=w1296, "dataLength"=w1293, "LaguerreDeconClass in"=w1297) -> ("error out"=w1292:errorcluster, "LaguerreDeconClass out"=w1291:refnum<class "LaguerreDeconEngineClass.lvclass">)  [unwired: 7 in]
        n582 = call "setIRF.vi"("error in (no error)"=w1292, "iRF"=w1276, "LaguerreDeconClass in"=w1291) -> ("error out"=w1289:errorcluster, "LaguerreDeconClass out"=w1290:refnum<class "LaguerreDeconEngineClass.lvclass">)  [unwired: 7 in]
        n583 = call "computeAlpha.vi"("error in (no error)"=w1289, "LaguerreDeconClass in"=w1290) -> ("error out"=w1287:errorcluster, "LaguerreDeconClass out"=w1288:refnum<class "LaguerreDeconEngineClass.lvclass">)  [unwired: 8 in]
        n584 = call "dataInitilize.vi"("error in (no error)"=w1287, "LaguerreDeconClass in"=w1288) -> ("error out"=w1285:errorcluster, "LaguerreDeconClass out"=w1286:refnum<class "LaguerreDeconEngineClass.lvclass">)  [unwired: 8 in]
        n585 = call "computeDeconMatrix.vi"("error in (no error)"=w1285, "LaguerreDeconClass in"=w1286) -> ("error out"=w1281:errorcluster, "LaguerreDeconClass out"=w1283:refnum<class "LaguerreDeconEngineClass.lvclass">)  [unwired: 8 in]
        n586 = call "Ch3DeconEngineFGV.vi"("Error In"=w1281, "action(read)"=enum16{"write", "read"}."write" ("action"), "Ch3DeconEngine in"=w1283) -> ("Error Out"=w1280:errorcluster)  [unwired: 7 in, 1 out]
        n587 = call <vilib>:"Add State(s) to Queue__JKI_lib_State_Machine.vi"("State(s) in (\"\")"=w1300) -> ("States Out"=w1299:string)  [unwired: 14 in]
      }
      frame "DeconEngine: InitializeCh4" {
        w1301 = refnum<class "LaguerreDeconEngineClass.lvclass"> refnum  # Ch3DeconObj
        # "Initilize Laguerre Deconvolution engine Object\n(You can make a copy of, or modify, this frame)"
        n588 = call "FLImDAQ_FGV.vi"("error in (no error)"=w1310) -> ("error out"=w1321:errorcluster, "Read data"=w1320:T6)  [unwired: 9 in]
        n589 = global read "GlobalVariables.vi" "LastUseiRF"() -> (w1303:T15)
        n590 = call "setLaguerreOrder.vi"("error in (no error)"=w1321, "LaguerreOrder"=u32 12, "LaguerreDeconClass in"=w1301) -> ("error out"=w1322:errorcluster, "LaguerreDeconClass out"=w1323:refnum<class "LaguerreDeconEngineClass.lvclass">)  [unwired: 7 in]
        n591 = Unbundle By Name(w1320) -> ("min record length"=w1319:i32)
        n592 = Unbundle By Name(w1303) -> ("Ch3 iRF"=w1302:dbl[])
        n593 = call "setDataLength.vi"("error in (no error)"=w1322, "dataLength"=w1319, "LaguerreDeconClass in"=w1323) -> ("error out"=w1318:errorcluster, "LaguerreDeconClass out"=w1317:refnum<class "LaguerreDeconEngineClass.lvclass">)  [unwired: 7 in]
        n594 = call "setIRF.vi"("error in (no error)"=w1318, "iRF"=w1302, "LaguerreDeconClass in"=w1317) -> ("error out"=w1315:errorcluster, "LaguerreDeconClass out"=w1316:refnum<class "LaguerreDeconEngineClass.lvclass">)  [unwired: 7 in]
        n595 = call "computeAlpha.vi"("error in (no error)"=w1315, "LaguerreDeconClass in"=w1316) -> ("error out"=w1313:errorcluster, "LaguerreDeconClass out"=w1314:refnum<class "LaguerreDeconEngineClass.lvclass">)  [unwired: 8 in]
        n596 = call "dataInitilize.vi"("error in (no error)"=w1313, "LaguerreDeconClass in"=w1314) -> ("error out"=w1311:errorcluster, "LaguerreDeconClass out"=w1312:refnum<class "LaguerreDeconEngineClass.lvclass">)  [unwired: 8 in]
        n597 = call "computeDeconMatrix.vi"("error in (no error)"=w1311, "LaguerreDeconClass in"=w1312) -> ("error out"=w1307:errorcluster, "LaguerreDeconClass out"=w1309:refnum<class "LaguerreDeconEngineClass.lvclass">)  [unwired: 8 in]
        n598 = call "Ch3DeconEngineFGV.vi"("Error In"=w1307, "action(read)"=enum16{"write", "read"}."write" ("action"), "Ch3DeconEngine in"=w1309) -> ("Error Out"=w1306:errorcluster)  [unwired: 7 in, 1 out]
        n599 = call <vilib>:"Add State(s) to Queue__JKI_lib_State_Machine.vi"("State(s) in (\"\")"=w1326) -> ("States Out"=w1325:string)  [unwired: 14 in]
      }
      frame "---------- Digitizer ----------" {
        # "Template Separator\n(You can make a copy of, or modify, this frame)"
        n600 = call <vilib>:"Add State(s) to Queue__JKI_lib_State_Machine.vi"("State(s) in (\"\")"=w1331) -> ("States Out"=w1330:string)  [unwired: 14 in]
      }
      frame "Digitizer: Initialize" {
        # "reset digitizer to everytime the system runs"
        # "reset digitizer to everytime the system runs"
        # "Initialize digitizer.\nInitialize both digitizer and update status."
        n601 = call "FLImDAQ_FGV.vi"("error in (no error)"=w1339) -> ("error out"=w1333:errorcluster, "Read data"=w1338:T6)  [unwired: 9 in]
        n602 = Unbundle By Name(w1341) -> ("SysConfigCluster.Ch1Enable?"=w1346:bool, "SysConfigCluster.Ch2Enable?"=w1345:bool, "SysConfigCluster.Ch3Enable?"=w1343:bool)
        n603 = Unbundle By Name(w1338) -> ("Digitizer 1"=w1334:refnum<k15>, "Digitizer 2"=w1337:refnum<k15>)
        n604 = property on="Digitizer" class="Bool (strict)"("Blinking"=TRUE) -> ()  [unwired: 2 in, 2 out]
        n605 = Or(x=w1346, y=w1345) -> (x .or. y?=w1344:bool)
        n606 = case shown="True" w1344 {
          tunnel: w1333 -> [w1354 w1357]
          tunnel: [w1354 w1356] -> w1335
          tunnel: w1334 -> [_ w1358]
          frame False {
          }
          frame True {
            n607 = call <instrlib>:"niScope Initialize.vi"("resource name"=w1358, "reset device"=TRUE, "error in"=w1357) -> ("error out"=w1356:errorcluster)  [unwired: 11 in, 1 out]
          }
        }
        n608 = case shown="True" w1343 {
          tunnel: w1333 -> [w1349 w1351]
          tunnel: [w1349 w1353] -> w1340
          tunnel: w1337 -> [_ w1352]
          frame False {
          }
          frame True {
            n609 = call <instrlib>:"niScope Initialize.vi"("resource name"=w1352, "reset device"=TRUE, "error in"=w1351) -> ("error out"=w1353:errorcluster)  [unwired: 11 in, 1 out]
          }
        }
        n610 = Merge Errors(w1335, w1340) -> (w1332:errorcluster)
        n611 = call <vilib>:"Add State(s) to Queue__JKI_lib_State_Machine.vi"("State(s) in (\"\")"=w1348) -> ("States Out"=w1347:string)  [unwired: 14 in]
      }
      frame "Digitizer: Config" {
        # "Synchronize is taking time ~3s."
        # "Config  digitizer\nCall subVi to config digitizer"
        n612 = call "FLImDAQ_FGV.vi"() -> ("Read data"=w1376:T6)  [unwired: 10 in, 1 out]
        n613 = Unbundle By Name(w1385) -> ("SysConfigCluster.Ch1Enable?"=w1393:bool, "SysConfigCluster.Ch2Enable?"=w1392:bool, "SysConfigCluster.Ch3Enable?"=w1390:bool, "FLImDAQ"=w1387:T30)
        n614 = Unbundle By Name(w1376) -> ("Digitizer 1"=w1379:refnum<k15>, "Digitizer 2"=w1378:refnum<k15>)
        n615 = property on="Digitizer" class="Bool (strict)"(error in=w1380, "Blinking"=TRUE) -> (error out=w1381:errorcluster)  [unwired: 1 in, 1 out]
        n616 = Or(x=w1393, y=w1392) -> (x .or. y?=w1391:bool)
        n617 = case shown="True" w1391 {
          tunnel: w1387 -> [_ w1406]
          tunnel: w1381 -> [w1402 w1405]
          tunnel: [w1402 w1404] -> w1388
          tunnel: w1379 -> [_ w1403]
          frame False {
          }
          frame True {
            n618 = call "DigitizerConfig.vi"("error in (no error)"=w1405, "FLImDAQ"=w1406, "IVI Refnum in"=w1403) -> ("error out"=w1404:errorcluster)  [unwired: 7 in, 1 out]
          }
        }
        n619 = case shown="True" w1390 {
          tunnel: w1387 -> [_ w1401]
          tunnel: w1388 -> [w1396 w1400]
          tunnel: [w1396 w1399] -> w1364
          tunnel: w1378 -> [_ w1397]
          frame False {
          }
          frame True {
            n620 = call "DigitizerConfig.vi"("Config Trigger? (T)"=FALSE ("Config Trigge(T)r:"), "error in (no error)"=w1400, "FLImDAQ"=w1401, "IVI Refnum in"=w1397) -> ("error out"=w1399:errorcluster)  [unwired: 6 in, 1 out]
          }
        }
        n621 = call "Digitizer1_FGV.vi"("error in (no error)"=w1364) -> ("error out"=w1374:errorcluster, "Read data"=w1375:refnum<k15>)  [unwired: 9 in]
        n622 = call <instrlib>:"niScope Get Session Reference.vi"("instrument handle"=w1375, "error in"=w1374) -> ("session reference"=w1368:refnum<k20>, "error out"=w1366:errorcluster)  [unwired: 11 in, 1 out]
        n623 = call "Digitizer2_FGV.vi"("error in (no error)"=w1366) -> ("error out"=w1372:errorcluster, "Read data"=w1373:refnum<k15>)  [unwired: 9 in]
        n624 = call <instrlib>:"niScope Get Session Reference.vi"("instrument handle"=w1373, "error in"=w1372) -> ("session reference"=w1367:refnum<k20>, "error out"=w1365:errorcluster)  [unwired: 11 in, 1 out]
        n625 = Build Array(w1368, w1367) -> (w1371:refnum<k20>[])
        n626 = call <instrlib>:"niTClk Configure For Homogeneous Triggers.vi"("error in (no error)"=w1365, "sessions"=w1371) -> ("error out"=w1370:errorcluster, "sessions out"=w1369:refnum<k20>[])  [unwired: 8 in]
        n627 = call <instrlib>:"niTClk Synchronize.vi"("error in (no error)"=w1370, "sessions"=w1369) -> ("error out"=w1363:errorcluster, "sessions out"=w1361:refnum<k20>[])  [unwired: 8 in]
        n628 = call <userlib>:"Wait (ms)__ogtk.vi"("error in (no error)"=w1363, "milliseconds to wait"=u32 1500) -> ("error out"=w1359:errorcluster)  [unwired: 8 in, 1 out]
        n629 = Unbundle By Name(w1359) -> ("status"=w1384:bool)
        n630 = Not(x=w1384) -> (.not. x?=w1383:bool)
        n631 = Bundle By Name(cluster=w1385, "System Status.Digitizer"=w1383, "niTClk sessions"=w1361) -> (w1386:T23)
        n632 = property on="Digitizer" class="Bool (strict)"(error in=w1359, "Blinking"=FALSE) -> (error out=w1377:errorcluster)  [unwired: 1 in, 1 out]
        n633 = call <vilib>:"Add State(s) to Queue__JKI_lib_State_Machine.vi"("State(s) in (\"\")"=w1395) -> ("States Out"=w1394:string)  [unwired: 14 in]
      }
      frame "Digitizer: Start" {
        # "send trigger to start acquisition loop"
        # "initilize aquisition"
        # "Start Digitizer\n(TClk start)"
        n634 = Unbundle By Name(w1414) -> ("niTClk sessions"=w1413:refnum<k20>[])
        n635 = call <instrlib>:"niTClk Initiate.vi"("error in (no error)"=w1407, "sessions"=w1413) -> ("error out"=w1409:errorcluster)  [unwired: 8 in, 1 out]
        n636 = Generate User Event(priority (normal)=usereventprio."high priority", user event=w1410, event data cluster=TRUE ("event data"), error in=w1409) -> (error out=w1408:errorcluster)  [unwired: 1 out]
        n637 = call <vilib>:"Add State(s) to Queue__JKI_lib_State_Machine.vi"("State(s) in (\"\")"=w1417) -> ("States Out"=w1416:string)  [unwired: 14 in]
      }
      frame "Digitizer: Abort" {
        # "Template Separator\n(You can make a copy of, or modify, this frame)"
        n638 = call "Digitizer1_FGV.vi"("error in (no error)"=w1421, "Operation (Read)"=enum16{"Write", "Read"}."Read" ("Operation")) -> ("error out"=w1428:errorcluster, "Read data"=w1425:refnum<k15>)  [unwired: 8 in]
        n639 = call "Digitizer2_FGV.vi"("error in (no error)"=w1421, "Operation (Read)"=enum16{"Write", "Read"}."Read" ("Operation")) -> ("error out"=w1424:errorcluster, "Read data"=w1426:refnum<k15>)  [unwired: 8 in]
        n640 = Bundle By Name(cluster=w1418, "SysRunning?"=FALSE ("System Status")) -> (w1419:T23)
        n641 = call <instrlib>:"niScope Abort.vi"("instrument handle"=w1425, "error in"=w1428) -> ("error out"=w1430:errorcluster)  [unwired: 12 in, 1 out]
        n642 = call <instrlib>:"niScope Abort.vi"("instrument handle"=w1426, "error in"=w1424) -> ("error out"=w1429:errorcluster)  [unwired: 12 in, 1 out]
        n643 = Merge Errors(w1430, w1429) -> (w1422:errorcluster)
        n644 = call <vilib>:"Add State(s) to Queue__JKI_lib_State_Machine.vi"("State(s) in (\"\")"=w1433) -> ("States Out"=w1432:string)  [unwired: 14 in]
      }
      frame "Digitizer: checkTemp" {
        w1436 = 65.0 ("y")
        w1441 = enum16{"Write", "Read"}."Read" ("Operation")
        # "Template Separator\n(You can make a copy of, or modify, this frame)"
        n645 = call "Digitizer1_FGV.vi"("Operation (Read)"=w1441) -> ("error out"=w1442:errorcluster, "Read data"=w1443:refnum<k15>)  [unwired: 9 in]
        n646 = call "Digitizer2_FGV.vi"("Operation (Read)"=w1441) -> ("error out"=w1439:errorcluster, "Read data"=w1440:refnum<k15>)  [unwired: 9 in]
        n647 = property on="Property Node" class="niScope"(reference=w1440, error in=w1439) -> ("Device Temperature"=w1437:dbl)  [unwired: 2 out]
        "Dig2 Temp" <- w1437
        n648 = property on="Property Node" class="niScope"(reference=w1443, error in=w1442) -> ("Device Temperature"=w1438:dbl)  [unwired: 2 out]
        "Dig1 Temp" <- w1438
        n649 = Greater?(x=w1438, y=w1436) -> (0:w1435:bool)
        n650 = Greater?(x=w1437, y=w1436) -> (0:w1434:bool)
        n651 = case shown="True" w1435 {
          frame False {
          }
          frame True {
            n652 = One Button Dialog(message="Digitizer 1 over heating!", button name ("OK")="OK") -> ()  [unwired: 1 out]
          }
        }
        n653 = case shown="True" w1434 {
          frame False {
          }
          frame True {
            n654 = One Button Dialog(message="Digitizer 2 over heating!", button name ("OK")="OK") -> ()  [unwired: 1 out]
          }
        }
        n655 = call <vilib>:"Add State(s) to Queue__JKI_lib_State_Machine.vi"("State(s) in (\"\")"=w1448) -> ("States Out"=w1447:string)  [unwired: 14 in]
      }
      frame "Digitizer: Close" {
        # "Close Digitizer"
        n656 = call "Digitizer1_FGV.vi"("error in (no error)"=w1458, "Operation (Read)"=enum16{"Write", "Read"}."Read" ("Operation")) -> ("error out"=w1460:errorcluster, "Read data"=w1464:refnum<k15>)  [unwired: 8 in]
        n657 = call "Digitizer2_FGV.vi"("error in (no error)"=w1458, "Operation (Read)"=enum16{"Write", "Read"}."Read" ("Operation")) -> ("error out"=w1459:errorcluster, "Read data"=w1462:refnum<k15>)  [unwired: 8 in]
        n658 = call <instrlib>:"niScope Close.vi"("instrument handle"=w1464, "error in"=w1460) -> ("error out"=w1457:errorcluster)  [unwired: 13 in]
        n659 = call <instrlib>:"niScope Close.vi"("instrument handle"=w1462, "error in"=w1459) -> ("error out"=w1456:errorcluster)  [unwired: 13 in]
        n660 = Merge Errors(w1457, w1456) -> (w1455:errorcluster)
        n661 = Unbundle By Name(w1455) -> ("status"=w1454:bool)
        n662 = Bundle By Name(cluster=w1465, "System Status.Digitizer"=w1454) -> (w1466:T23)
        n663 = call <vilib>:"Add State(s) to Queue__JKI_lib_State_Machine.vi"("State(s) in (\"\")"=w1468) -> ("States Out"=w1467:string)  [unwired: 14 in]
      }
      frame "---------- LabJack ----------" {
        # "Template Separator\n(You can make a copy of, or modify, this frame)"
        n664 = call <vilib>:"Add State(s) to Queue__JKI_lib_State_Machine.vi"("State(s) in (\"\")"=w1473) -> ("States Out"=w1472:string)  [unwired: 14 in]
      }
      frame "LabJack: checkPedal" {
        # "Template Separator\n(You can make a copy of, or modify, this frame)"
        n665 = Unbundle By Name(w1474) -> ("LJ Pinout.Foot Pedal"=w1478:string)
        n666 = call "LabJack_FGV.vi"("Operation(Read)"=enum16{"Write", "Read"}."Read" ("Operation"), "error in (no error)"=w1476) -> ("error out"=w1480:errorcluster, "Read data"=w1481:i32)  [unwired: 8 in]
        n667 = call "LJM_eReadName.vi"("Handle In"=w1481, "Name"=w1478, "error in"=w1480) -> ("Value"=w1479:dbl, "error out"=w1477:errorcluster)  [unwired: 10 in, 1 out]
        n668 = case shown="1" w1479 {
          tunnel: w1474 -> [w1486 w1489]
          tunnel: [w1486 w1487] -> w1475
          frame 0, Default {
          }
          frame 1 {
            # "If Pedal pressed"
            n669 = Tick Count (ms)() -> (millisecond timer value=w1493:u32)
            n670 = Unbundle By Name(w1489) -> ("Last Trigger"=w1488:u32)
            n671 = Subtract(x=w1493, y=w1488) -> (x-y=w1492:u32)
            n672 = Greater Or Equal?(x=w1492, y=u32 2000) -> (x >= y?=w1490:bool)
            n673 = case shown="True" w1490 {
              tunnel: w1489 -> [w1494 w1495]
              tunnel: w1488 -> [_ _]
              tunnel: [w1494 w1496] -> w1487
              frame False {
              }
              frame True {
                n674 = Tick Count (ms)() -> (millisecond timer value=w1497:u32)
                n675 = Unbundle By Name(w1495) -> ("SysRunning?"=w1498:bool)
                n676 = case shown="False" w1498 {
                  frame False {
                    n677 = property on="StartButton" class="Bool (strict)"("Val(Sgnl)"=TRUE ("Value (Signaling)")) -> ()  [unwired: 2 in, 2 out]
                  }
                  frame True {
                    n678 = property on="StopButton" class="Bool (strict)"("Val(Sgnl)"=TRUE ("Value (Signaling)")) -> ()  [unwired: 2 in, 2 out]
                  }
                }
                n679 = Bundle By Name(cluster=w1495, "Last Trigger"=w1497) -> (w1496:T23)
              }
            }
          }
        }
        n680 = call <vilib>:"Add State(s) to Queue__JKI_lib_State_Machine.vi"("State(s) in (\"\")"=w1485) -> ("States Out"=w1484:string)  [unwired: 14 in]
      }
      frame "LabJack: ZeroV" {
        # "Just Zero V\nDO not update FGV and front panel\nWIll resume from last V"
        # "set bias to 0"
        # "Zero APD bias\n(You can make a copy of, or modify, this frame)"
        n681 = Unbundle By Name(w1503) -> ("LJ Pinout.Ch1 Bias"=w1508:string, "LJ Pinout.Ch2 Bias"=w1507:string, "LJ Pinout.Ch3 Bias"=w1506:string)
        n682 = Build Array(w1508, w1507, w1506) -> (w1505:string[])
        n683 = call "LabJack_FGV.vi"("Operation(Read)"=enum16{"Write", "Read"}."Read" ("Operation"), "error in (no error)"=w1502) -> ("error out"=w1509:errorcluster, "Read data"=w1510:i32)  [unwired: 8 in]
        n684 = call "LJM_eWriteNames.vi"("Handle In"=w1510, "aNames"=w1505, "aValuesIn"=dbl[] [0.0, 0.0, 0.0], "error in"=w1509) -> ("error out"=w1501:errorcluster)  [unwired: 9 in, 2 out]
        n685 = call <vilib>:"Add State(s) to Queue__JKI_lib_State_Machine.vi"("State(s) in (\"\")"=w1514) -> ("States Out"=w1513:string)  [unwired: 14 in]
      }
      frame "LabJack: SetV" {
        w1521 = enum16{"write", "read"}."read" ("action (write)")
        # "set bias to user specifid"
        # "Set APD bias\n(You can make a copy of, or modify, this frame)"
        n686 = Unbundle By Name(w1530) -> ("LJ Pinout.Ch1 Bias"=w1534:string, "LJ Pinout.Ch2 Bias"=w1533:string, "LJ Pinout.Ch3 Bias"=w1532:string, "LJ Pinout.Ch4 Bias"=w1524:string)
        n687 = call "V2FGV.vi"("Error In"=w1520, "action(write)"=w1521) -> ("Error Out"=w1518:errorcluster, "V2 out"=w1526:dbl)  [unwired: 8 in]
        n688 = call "V4FGV.vi"("Error In"=w1520, "action(write)"=w1521) -> ("Error Out"=w1516:errorcluster, "V3 out"=w1522:dbl)  [unwired: 8 in]
        n689 = call "V1FGV.vi"("Error In"=w1520, "action (write)"=w1521) -> ("Error Out"=w1519:errorcluster, "V1 out"=w1523:dbl)  [unwired: 8 in]
        n690 = call "V3FGV.vi"("Error In"=w1520, "action(write)"=w1521) -> ("Error Out"=w1517:errorcluster, "V3 out"=w1525:dbl)  [unwired: 8 in]
        n691 = local write "V 3"(w1525) -> ()
        n692 = local write "V 2"(w1526) -> ()
        n693 = local write "V 4"(w1522) -> ()
        n694 = local write "V 1"(w1523) -> ()
        n695 = Build Array(w1534, w1533, w1532, w1524) -> (w1531:string[])
        n696 = call "LabJack_FGV.vi"("Operation(Read)"=enum16{"Write", "Read"}."Read" ("Operation"), "error in (no error)"=w1520) -> ("error out"=w1535:errorcluster, "Read data"=w1536:i32)  [unwired: 8 in]
        n697 = Build Array(w1523, w1526, w1525, w1522) -> (w1527:dbl[])
        n698 = call "LJM_eWriteNames.vi"("Handle In"=w1536, "aNames"=w1531, "aValuesIn"=w1527, "error in"=w1535) -> ("error out"=w1528:errorcluster)  [unwired: 9 in, 2 out]
        n699 = Merge Errors(w1519, w1518, w1517, w1516) -> (w1515:errorcluster)
        n700 = call <vilib>:"Add State(s) to Queue__JKI_lib_State_Machine.vi"("State(s) in (\"\")"=w1540) -> ("States Out"=w1539:string)  [unwired: 14 in]
        n701 = Merge Errors(w1515, w1528) -> (w1529:errorcluster)
      }
      frame "LabJack: Open" {
        # "Initialize LabJack T7\nEstablish connection and initialize pins"
        n702 = call "LJ_Open.vi"("error in"=w1550, "DeviceType"="LJM_dtT7") -> ("error out"=w1547:errorcluster, "Success?"=w1548:bool, "Handle Out"=w1542:i32)  [unwired: 7 in]
        n703 = call "LabJack_FGV.vi"("Operation(Read)"=enum16{"Write", "Read"}."Write" ("Operation"), "error in (no error)"=w1547, "Write data"=w1542) -> ("error out"=w1544:errorcluster)  [unwired: 7 in, 1 out]
        n704 = Bundle By Name(cluster=w1545, "System Status.Labjack"=w1548) -> (w1549:T23)
        n705 = call <vilib>:"Add State(s) to Queue__JKI_lib_State_Machine.vi"("State(s) in (\"\")"=w1552) -> ("States Out"=w1551:string)  [unwired: 14 in]
      }
      frame "LabJack: SetDefaultSub" {
        w1562 = enum16{"write", "read"}."write" ("action")
        w1563 = 0.0 ("V1 in")
        w1576 = "_EF_ENABLE" ("string")
        # "1. Disable PWM\n2. Set all V to 0\n3. Set 355 relay to open\n4. Set LED to off"
        # "read once to set DIO to input"
        # "set all initila V to 0. Set footpedal to input. Set PWM to low. Set laser relay to open. Set LEDs to yellow."
        # "Set Labjack to correct input and output state and initial values"
        n706 = disable-structure shown="Disabled" {
          frame Disabled {
            (unwired) dbl[] [0.0, 0.0, 0.0, 0.0, 0.0, 0.0, 0.0, 0.0, 0.0] ("aValuesIn")
          }
          frame Enabled {
          }
        }
        n707 = Unbundle By Name(w1573) -> ("LJ Pinout.355 PWM"=w1578:string, "LJ Pinout.AimingBeam PWM"=w1577:string, "LJ Pinout.Ch1 Bias"=w1583:string, "LJ Pinout.Ch2 Bias"=w1553:string, "LJ Pinout.Ch3 Bias"=w1587:string, "LJ Pinout.Ch4 Bias"=w1567:string, "LJ Pinout.Laser Start/Stop"=w1586:string, "LJ Pinout.Red LED"=w1585:string, "LJ Pinout.Green LED"=w1584:string)
        n708 = call "V1FGV.vi"("Error In"=w1571, "action (write)"=w1562, "V1 in"=w1563) -> ("Error Out"=w1566:errorcluster, "V1 out"=w1570:dbl)  [unwired: 7 in]
        n709 = local write "V 1"(w1570) -> ()
        n710 = call "V2FGV.vi"("Error In"=w1566, "action(write)"=w1562, "V2 in"=w1563) -> ("Error Out"=w1565:errorcluster, "V2 out"=w1569:dbl)  [unwired: 7 in]
        n711 = call "LabJack_FGV.vi"("Operation(Read)"=enum16{"Write", "Read"}."Read" ("Operation"), "error in (no error)"=w1571) -> ("error out"=w1559:errorcluster, "Read data"=w1581:i32)  [unwired: 8 in]
        n712 = Concatenate Strings(w1578, w1576) -> (w1575:string)
        n713 = Concatenate Strings(w1577, w1576) -> (w1574:string)
        n714 = local write "V 2"(w1569) -> ()
        n715 = call "V3FGV.vi"("Error In"=w1565, "action(write)"=w1562, "V3 in"=w1563) -> ("Error Out"=w1564:errorcluster, "V3 out"=w1568:dbl)  [unwired: 7 in]
        n716 = Build Array(w1575, w1574, w1583, w1553, w1587, w1567, w1586, w1585, w1584) -> (w1557:string[])
        n717 = local write "V 3"(w1568) -> ()
        n718 = call "V4FGV.vi"("Error In"=w1564, "action(write)"=w1562, "V3 in"=w1563) -> ("Error Out"=w1560:errorcluster, "V3 out"=w1561:dbl)  [unwired: 7 in]
        n719 = Array Size(array=w1557) -> (size(s)=w1556:i32)
        n720 = local write "V 4"(w1561) -> ()
        n721 = Initialize Array(0.0 ("element"), w1556) -> (w1554:dbl[])
        n722 = Unbundle By Name(w1573) -> ("LJ Pinout.Foot Pedal"=w1572:string)
        n723 = call "LJM_eWriteNames.vi"("Handle In"=w1581, "aNames"=w1557, "aValuesIn"=w1554, "error in"=w1559) -> ("Handle Out"=w1580:i32, "error out"=w1579:errorcluster)  [unwired: 9 in, 1 out]
        n724 = call "LJM_eReadName.vi"("Handle In"=w1580, "Name"=w1572, "error in"=w1579) -> ("error out"=w1558:errorcluster)  [unwired: 10 in, 2 out]
        n725 = case shown="Error .." w1558 {
          frame No Error {
            # "no error"
          }
          frame Error {
            # "handle error"
            n726 = One Button Dialog(message="Labjack error! The pin assignment is likely wrong. Please check pin setting of Labjack. Program will terminate.", button name ("OK")="OK") -> ()  [unwired: 1 out]
          }
        }
        n727 = call <vilib>:"Add State(s) to Queue__JKI_lib_State_Machine.vi"("State(s) in (\"\")"=w1590) -> ("States Out"=w1589:string)  [unwired: 14 in]
      }
      frame "LabJack: FootPedalConfig" {
        # "Setup footPedal\n(You can make a copy of, or modify, this frame)"
        n728 = call "LabJack_FGV.vi"("Operation(Read)"=enum16{"Write", "Read"}."Read" ("Operation"), "error in (no error)"=w1594) -> ("error out"=w1598:errorcluster, "Read data"=w1599:i32)  [unwired: 8 in]
        n729 = call "LJM_eWriteName.vi"("Handle In"=w1599, "Name"="DIO15", "Value"=1.0, "error in"=w1598) -> ("error out"=w1595:errorcluster)  [unwired: 10 in, 1 out]
        n730 = call <vilib>:"Add State(s) to Queue__JKI_lib_State_Machine.vi"("State(s) in (\"\")"=w1603) -> ("States Out"=w1602:string)  [unwired: 14 in]
      }
      frame "LabJack: SetDefaultAndClose" {
        # "Template Separator\n(You can make a copy of, or modify, this frame)"
        n731 = call <vilib>:"Add State(s) to Queue__JKI_lib_State_Machine.vi"("State(s) in Front (\"\")"="LabJack: SetDefaultSub\nLabJack: Close" ("State(s) in Front (\"\")"), "State(s) in (\"\")"=w1609) -> ("States Out"=w1608:string)  [unwired: 13 in]
      }
      frame "LabJack: Close" {
        # "Close LabJack Refnum"
        n732 = call "LabJack_FGV.vi"("Operation(Read)"=enum16{"Write", "Read"}."Read" ("Operation"), "error in (no error)"=w1615) -> ("error out"=w1610:errorcluster, "Read data"=w1611:i32)  [unwired: 8 in]
        n733 = Bundle By Name(cluster=w1613, "System Status.Labjack"=FALSE ("System Status.Gain Control")) -> (w1616:T23)
        n734 = call "LJM_Close.vi"("error in"=w1610, "Handle"=w1611) -> ("error out"=w1618:errorcluster)  [unwired: 9 in]
        n735 = call <vilib>:"Add State(s) to Queue__JKI_lib_State_Machine.vi"("State(s) in (\"\")"=w1620) -> ("States Out"=w1619:string)  [unwired: 14 in]
      }
      frame "LabJack: Interlock enable/disable" {
        w1629 = i8 0  # int8
        # "[Covers: REQ8]"
        # "Interlock enable/disable\n(Usage: \"LabJack: Interlock enable/disable >> 1|0\")"
        n736 = Fract/Exp String To Number(string=w1630, default (0 dbl)=w1629) -> (number=w1626:i8)  [unwired: 2 in, 1 out]
        n737 = Unbundle By Name(w1628) -> ("LJ Pinout.Interlock"=w1627:string)
        n738 = call "LabJack_FGV.vi"("Operation(Read)"=enum16{"Write", "Read"}."Read" ("Operation")) -> ("Read data"=w1624:i32)  [unwired: 9 in, 1 out]
        n739 = call "LJM_eWriteName.vi"("Handle In"=w1624, "Name"=w1627, "Value"=w1626, "error in"=w1625) -> ("error out"=w1622:errorcluster)  [unwired: 10 in, 1 out]
        n740 = call <vilib>:"Add State(s) to Queue__JKI_lib_State_Machine.vi"("State(s) in (\"\")"=w1632) -> ("States Out"=w1631:string)  [unwired: 14 in]
      }
      frame "LabJack: 355_PWM_Config" {
        w1634 = 0.0 ("element")
        w1654 = "DIO_EF_CLOCK1_ENABLE"
        # "Config PWM frequency"
        n741 = Unbundle By Name(w1646) -> ("LJ Pinout.355 PWM"=w1653:string)
        n742 = Unbundle By Name(w1646) -> ("355 PWM setting.DIO_EF_CLOCK1_DIVISOR"=w1645:i16, "355 PWM setting.DIO_EF_CLOCK1_ROLL_VALUE"=w1644:i32, "355 PWM setting.DIO#_EF_INDEX"=w1641:i16, "355 PWM setting.DIO#_EF_OPTIONS"=w1640:i16, "355 PWM setting.DIO#_EF_CONFIG_A"=w1639:i32)
        n743 = Concatenate Strings(w1653, "_EF_ENABLE" ("string")) -> (w1649:string)
        n744 = Concatenate Strings(w1653, "_EF_INDEX") -> (w1652:string)
        n745 = Concatenate Strings(w1653, "_EF_OPTIONS") -> (w1651:string)
        n746 = Concatenate Strings(w1653, "_EF_CONFIG_A") -> (w1650:string)
        n747 = call "LabJack_FGV.vi"("Operation(Read)"=enum16{"Write", "Read"}."Read" ("Operation")) -> ("Read data"=w1647:i32)  [unwired: 9 in, 1 out]
        n748 = Build Array(w1634, w1634, w1645, w1644, 1.0 ("element"), 0.0 ("element"), w1641, w1640, w1639) -> (w1638:dbl[])
        n749 = Build Array("DIO_EF_CLOCK0_ENABLE", w1654, "DIO_EF_CLOCK1_DIVISOR", "DIO_EF_CLOCK1_ROLL_VALUE", w1654, w1649, w1652, w1651, w1650) -> (w1648:string[])
        n750 = call "LJM_eWriteNames.vi"("Handle In"=w1647, "aNames"=w1648, "aValuesIn"=w1638, "error in"=w1636) -> ("error out"=w1637:errorcluster)  [unwired: 9 in, 2 out]
        n751 = call <vilib>:"Add State(s) to Queue__JKI_lib_State_Machine.vi"("State(s) in (\"\")"=w1663) -> ("States Out"=w1662:string)  [unwired: 14 in]
      }
      frame "LabJack: 355_PWM_Start" {
        # "Template Separator\n(You can make a copy of, or modify, this frame)"
        n752 = Unbundle By Name(w1671) -> ("LJ Pinout.355 PWM"=w1670:string)
        n753 = call "LabJack_FGV.vi"("Operation(Read)"=enum16{"Write", "Read"}."Read" ("Operation"), "error in (no error)"=w1665) -> ("error out"=w1672:errorcluster, "Read data"=w1673:i32)  [unwired: 8 in]
        n754 = Concatenate Strings(w1670, "_EF_ENABLE" ("string")) -> (w1668:string)
        n755 = call "LJM_eWriteName.vi"("Handle In"=w1673, "Name"=w1668, "Value"=1.0, "error in"=w1672) -> ("error out"=w1666:errorcluster)  [unwired: 10 in, 1 out]
        n756 = call <vilib>:"Add State(s) to Queue__JKI_lib_State_Machine.vi"("State(s) in (\"\")"=w1676) -> ("States Out"=w1675:string)  [unwired: 14 in]
      }
      frame "LabJack: 355_PWM_Stop" {
        # "Template Separator\n(You can make a copy of, or modify, this frame)"
        n757 = Unbundle By Name(w1682) -> ("LJ Pinout.355 PWM"=w1686:string)
        n758 = call "LabJack_FGV.vi"("Operation(Read)"=enum16{"Write", "Read"}."Read" ("Operation"), "error in (no error)"=w1681) -> ("error out"=w1687:errorcluster, "Read data"=w1679:i32)  [unwired: 8 in]
        n759 = Concatenate Strings(w1686, "_EF_ENABLE" ("string")) -> (w1684:string)
        n760 = call "LJM_eWriteName.vi"("Handle In"=w1679, "Name"=w1684, "Value"=0.0, "error in"=w1687) -> ("error out"=w1678:errorcluster)  [unwired: 10 in, 1 out]
        n761 = local write "355nm Laser toggle"(FALSE ("355nm Laser toggle")) -> ()
        n762 = call <vilib>:"Add State(s) to Queue__JKI_lib_State_Machine.vi"("State(s) in (\"\")"=w1690) -> ("States Out"=w1689:string)  [unwired: 14 in]
      }
      frame "LabJack: AB_Start" {
        # "Aiming Beam Start\n(Based on aimging beam frequency, set LabJack pin)"
        n763 = Unbundle By Name(w1700) -> ("AB Cluster.Freq"=w1692:i32, "LJ Pinout.AimingBeam PWM"=w1699:string)
        n764 = Greater Than 0?(x=w1692) -> (x > 0?=w1691:bool)
        n765 = case shown="False" w1691 {
          tunnel: w1699 -> [w1706 w1709]
          tunnel: [w1706 w1707] -> w1698
          frame False {
            # "if 0 freq, set PWM pin"
          }
          frame True {
            # "if non zero freq, set PWM enable"
            n766 = Concatenate Strings(w1709, "_EF_ENABLE" ("string")) -> (w1707:string)
          }
        }
        n767 = call "LabJack_FGV.vi"("Operation(Read)"=enum16{"Write", "Read"}."Read" ("Operation"), "error in (no error)"=w1695) -> ("error out"=w1701:errorcluster, "Read data"=w1702:i32)  [unwired: 8 in]
        n768 = call "LJM_eWriteName.vi"("Handle In"=w1702, "Name"=w1698, "Value"=1.0, "error in"=w1701) -> ("error out"=w1696:errorcluster)  [unwired: 10 in, 1 out]
        n769 = local write "Aiming beam toggle"(TRUE ("Aiming beam toggle")) -> ()
        n770 = call <vilib>:"Add State(s) to Queue__JKI_lib_State_Machine.vi"("State(s) in (\"\")"=w1705) -> ("States Out"=w1704:string)  [unwired: 14 in]
      }
      frame "LabJack: AB_Stop" {
        # "Aiming Beam Stop\n(Based on aiming beam frequency, set LabJack pin low)"
        n771 = Unbundle By Name(w1717) -> ("AB Cluster.Freq"=w1712:i32, "LJ Pinout.AimingBeam PWM"=w1719:string)
        n772 = Greater Than 0?(x=w1712) -> (x > 0?=w1711:bool)
        n773 = case shown="False" w1711 {
          tunnel: w1719 -> [w1725 w1728]
          tunnel: [w1725 w1726] -> w1710
          frame False {
          }
          frame True {
            n774 = Concatenate Strings(w1728, "_EF_ENABLE" ("string")) -> (w1726:string)
          }
        }
        n775 = call "LabJack_FGV.vi"("Operation(Read)"=enum16{"Write", "Read"}."Read" ("Operation"), "error in (no error)"=w1715) -> ("error out"=w1720:errorcluster, "Read data"=w1721:i32)  [unwired: 8 in]
        n776 = call "LJM_eWriteName.vi"("Handle In"=w1721, "Name"=w1710, "Value"=0.0, "error in"=w1720) -> ("error out"=w1716:errorcluster)  [unwired: 10 in, 1 out]
        n777 = local write "Aiming beam toggle"(FALSE ("Aiming beam toggle")) -> ()
        n778 = call <vilib>:"Add State(s) to Queue__JKI_lib_State_Machine.vi"("State(s) in (\"\")"=w1724) -> ("States Out"=w1723:string)  [unwired: 14 in]
      }
      frame "LabJack: AB_PWM_Config" {
        w1730 = 0.0 ("element")
        w1750 = "DIO_EF_CLOCK2_ENABLE"
        # "Config PWM frequency"
        n779 = Unbundle By Name(w1742) -> ("LJ Pinout.AimingBeam PWM"=w1749:string)
        n780 = Unbundle By Name(w1742) -> ("AB PWM setting.DIO_EF_CLOCK1_DIVISOR"=w1741:i16, "AB PWM setting.DIO_EF_CLOCK1_ROLL_VALUE"=w1740:i32, "AB PWM setting.DIO#_EF_INDEX"=w1737:i16, "AB PWM setting.DIO#_EF_OPTIONS"=w1736:i16, "AB PWM setting.DIO#_EF_CONFIG_A"=w1735:i32)
        n781 = Concatenate Strings(w1749, "_EF_ENABLE" ("string")) -> (w1745:string)
        n782 = Concatenate Strings(w1749, "_EF_INDEX") -> (w1748:string)
        n783 = Concatenate Strings(w1749, "_EF_OPTIONS") -> (w1747:string)
        n784 = Concatenate Strings(w1749, "_EF_CONFIG_A") -> (w1746:string)
        n785 = call "LabJack_FGV.vi"("Operation(Read)"=enum16{"Write", "Read"}."Read" ("Operation")) -> ("Read data"=w1743:i32)  [unwired: 9 in, 1 out]
        n786 = Build Array(w1730, w1730, w1741, w1740, 1.0 ("element"), 0.0 ("element"), w1737, w1736, w1735) -> (w1734:dbl[])
        n787 = Build Array("DIO_EF_CLOCK0_ENABLE", w1750, "DIO_EF_CLOCK2_DIVISOR", "DIO_EF_CLOCK2_ROLL_VALUE", w1750, w1745, w1748, w1747, w1746) -> (w1744:string[])
        n788 = call "LJM_eWriteNames.vi"("Handle In"=w1743, "aNames"=w1744, "aValuesIn"=w1734, "error in"=w1732) -> ("error out"=w1733:errorcluster)  [unwired: 9 in, 2 out]
        n789 = call <vilib>:"Add State(s) to Queue__JKI_lib_State_Machine.vi"("State(s) in (\"\")"=w1759) -> ("States Out"=w1758:string)  [unwired: 14 in]
      }
      frame "---------- LED ----------" {
        # "Template Separator\n(You can make a copy of, or modify, this frame)"
        n790 = call <vilib>:"Add State(s) to Queue__JKI_lib_State_Machine.vi"("State(s) in (\"\")"=w1764) -> ("States Out"=w1763:string)  [unwired: 14 in]
      }
      frame "LED: OpenVIRef" {
        # "Template Separator\n(You can make a copy of, or modify, this frame)"
        n791 = call <vilib>:"Application Directory.vi"() -> ("Application Directory"=w1771:path)
        n792 = Build Path(base path=w1771, name or relative path="SubVI") -> (appended path=w1769:path)
        n793 = Build Path(base path=w1769, name or relative path="LEDBreath.vi") -> (appended path=w1767:path)
        n794 = Open VI Reference(vi path=w1767, error in (no error)=w1772) -> (vi reference=w1773:refnum<vi>, error out=w1766:errorcluster)  [unwired: 4 in]
        n795 = case shown="Error .." w1766 {
          tunnel: [TRUE FALSE] -> w1765
          frame No Error {
          }
          frame Error {
          }
        }
        n796 = Bundle By Name(cluster=w1774, "LED vi reference"=w1773, "LED vi ref open?"=w1765) -> (w1775:T23)
        n797 = call <vilib>:"Add State(s) to Queue__JKI_lib_State_Machine.vi"("State(s) in (\"\")"=w1778) -> ("States Out"=w1777:string)  [unwired: 14 in]
      }
      frame "LED: CloseVIRef" {
        # "Template Separator\n(You can make a copy of, or modify, this frame)"
        n798 = Unbundle By Name(w1782) -> ("LED vi reference"=w1783:refnum<vi>, "LED vi ref open?"=w1781:bool)
        n799 = case shown="True" w1781 {
          tunnel: w1785 -> [w1789 w1792]
          tunnel: [w1789 w1791] -> w1784
          tunnel: w1783 -> [_ w1790]
          frame False {
          }
          frame True {
            n800 = Close Reference(reference=w1790, error in (no error)=w1792) -> (error out=w1791:errorcluster)
          }
        }
        n801 = call <vilib>:"Add State(s) to Queue__JKI_lib_State_Machine.vi"("State(s) in (\"\")"=w1788) -> ("States Out"=w1787:string)  [unwired: 14 in]
      }
      frame "LED: BreathGreen" {
        w1793 = FALSE ("Wait Until Done")
        # "Breath system LED\n(LED: Breath >> True/False)"
        n802 = Unbundle By Name(w1801) -> ("LED vi reference"=w1800:refnum<vi>)
        n803 = invoke class="VI" method="Ctrl Val.Set"(reference=w1800, error in=w1798, "Control Name"="Color", "Value"=0) -> (reference out=w1797:refnum<vi>, error out=w1796:errorcluster)  [unwired: 1 in, 3 out]
        n804 = invoke on="Invoke Node" class="VI" method="Run VI"(reference=w1797, error in=w1796, "Wait until done"=w1793, "Auto Dispose Ref"=w1793) -> (error out=w1799:errorcluster)  [unwired: 1 in, 4 out]
        n805 = call <vilib>:"Add State(s) to Queue__JKI_lib_State_Machine.vi"("State(s) in (\"\")"=w1804) -> ("States Out"=w1803:string)  [unwired: 14 in]
      }
      frame "LED: BreathOrange" {
        w1805 = FALSE ("Wait Until Done")
        # "Breath system LED\n(LED: Breath >> True/False)"
        n806 = Unbundle By Name(w1813) -> ("LED vi reference"=w1812:refnum<vi>)
        n807 = invoke class="VI" method="Ctrl Val.Set"(reference=w1812, error in=w1810, "Control Name"="Color", "Value"=1) -> (reference out=w1809:refnum<vi>, error out=w1808:errorcluster)  [unwired: 1 in, 3 out]
        n808 = invoke on="Invoke Node" class="VI" method="Run VI"(reference=w1809, error in=w1808, "Wait until done"=w1805, "Auto Dispose Ref"=w1805) -> (error out=w1811:errorcluster)  [unwired: 1 in, 4 out]
        n809 = call <vilib>:"Add State(s) to Queue__JKI_lib_State_Machine.vi"("State(s) in (\"\")"=w1816) -> ("States Out"=w1815:string)  [unwired: 14 in]
      }
      frame "LED: BreathOff" {
        # "System LED Breath Off\n(Breath off, check VI status to make sure it is off)"
        n810 = Unbundle By Name(w1825) -> ("LED vi reference"=w1824:refnum<vi>)
        n811 = invoke on="Invoke Node" class="VI" method="Ctrl Val.Set"(reference=w1824, error in=w1822, "Control Name"="Stop", "Value"=TRUE) -> (reference out=w1817:refnum<vi>, error out=w1818:errorcluster)  [unwired: 1 in, 3 out]
        n812 = case shown="No Error" w1818 {
          selector: w1818 -> [w1830 _]
          tunnel: [w1829 errorcluster {"status"=FALSE, "code"=0, "source"=""} ("error IO")] -> w1823
          tunnel: ["" ("State(s) in Front (\"\")") "LED: BreathOff" ("State(s) in Front (\"\")")] -> w1821
          tunnel: w1817 -> [w1831 _]
          frame No Error {
            # "No error, wait for VI to stop"
            n813 = while {
              tunnel: w1831 -> [w1839]
              shift-right: [w1833] -> w1829
              shift-left: w1830 -> [w1838]
              stop <- w1835 stop-if-true
              # "continue check whether vi is running"
              n814 = property class="VI"(reference=w1839, error in=w1838) -> (error out=w1833:errorcluster, "Exec.State"=w1837:T20)  [unwired: 1 out]
              n815 = Wait (ms)(milliseconds to wait=u32 50) -> ()  [unwired: 1 out]
              n816 = Equal?(x=w1837, y=T20."Idle") -> (x = y?=w1835:bool)
            }
          }
          frame Error {
            # "try again when error"
          }
        }
        n817 = call <vilib>:"Add State(s) to Queue__JKI_lib_State_Machine.vi"("State(s) in Front (\"\")"=w1821, "State(s) in (\"\")"=w1828) -> ("States Out"=w1827:string)  [unwired: 13 in]
      }
      frame "LED: Off" {
        # "set LED to red"
        # "Template Separator\n(You can make a copy of, or modify, this frame)"
        n818 = Unbundle By Name(w1844) -> ("LJ Pinout.Red LED"=w1843:string, "LJ Pinout.Green LED"=w1842:string)
        n819 = call "LabJack_FGV.vi"("Operation(Read)"=enum16{"Write", "Read"}."Read" ("Operation"), "error in (no error)"=w1845) -> ("error out"=w1852:errorcluster, "Read data"=w1851:i32)  [unwired: 8 in]
        n820 = call "LJM_eWriteName.vi"("Handle In"=w1851, "Name"=w1843, "Value"=0.0, "error in"=w1852) -> ("Handle Out"=w1849:i32, "error out"=w1848:errorcluster)  [unwired: 10 in]
        n821 = call "LJM_eWriteName.vi"("Handle In"=w1849, "Name"=w1842, "Value"=0.0, "error in"=w1848) -> ("error out"=w1846:errorcluster)  [unwired: 10 in, 1 out]
        n822 = call <vilib>:"Add State(s) to Queue__JKI_lib_State_Machine.vi"("State(s) in (\"\")"=w1856) -> ("States Out"=w1855:string)  [unwired: 14 in]
      }
      frame "LED: Green" {
        # "set LED to green"
        # "Template Separator\n(You can make a copy of, or modify, this frame)"
        n823 = Unbundle By Name(w1860) -> ("LJ Pinout.Red LED"=w1858:string, "LJ Pinout.Green LED"=w1859:string)
        n824 = call "LabJack_FGV.vi"("Operation(Read)"=enum16{"Write", "Read"}."Read" ("Operation"), "error in (no error)"=w1862) -> ("error out"=w1868:errorcluster, "Read data"=w1867:i32)  [unwired: 8 in]
        n825 = call "LJM_eWriteName.vi"("Handle In"=w1867, "Name"=w1858, "Value"=0.0, "error in"=w1868) -> ("Handle Out"=w1865:i32, "error out"=w1864:errorcluster)  [unwired: 10 in]
        n826 = call "LJM_eWriteName.vi"("Handle In"=w1865, "Name"=w1859, "Value"=9.0, "error in"=w1864) -> ("error out"=w1861:errorcluster)  [unwired: 10 in, 1 out]
        n827 = call <vilib>:"Add State(s) to Queue__JKI_lib_State_Machine.vi"("State(s) in (\"\")"=w1871) -> ("States Out"=w1870:string)  [unwired: 14 in]
      }
      frame "---------- Queue ----------" {
        # "Template Separator\n(You can make a copy of, or modify, this frame)"
        n828 = call <vilib>:"Add State(s) to Queue__JKI_lib_State_Machine.vi"("State(s) in (\"\")"=w1876) -> ("States Out"=w1875:string)  [unwired: 14 in]
      }
      frame "Queue: Flash" {
        # "Clear queue contnet\n(clear queue content by flash it)"
        n829 = Flush Queue(queue=w1882, error in (no error)=w1881) -> (error out=w1880:errorcluster)  [unwired: 2 out]
        n830 = Flush Queue(queue=w1883, error in (no error)=w1880) -> (error out=w1878:errorcluster)  [unwired: 2 out]
        n831 = Flush Queue(queue=w1879, error in (no error)=w1878) -> (error out=w1877:errorcluster)  [unwired: 2 out]
        n832 = call <vilib>:"Add State(s) to Queue__JKI_lib_State_Machine.vi"("State(s) in (\"\")"=w1887) -> ("States Out"=w1886:string)  [unwired: 14 in]
      }
      frame "Queue: Destory" {
        # "Destory Data Queue\nDistory data queue ref so the aquisition loop stop"
        n833 = Release Queue(queue=w1893, error in (no error)=w1889) -> (error out=w1896:errorcluster)  [unwired: 1 in, 2 out]
        n834 = Release Queue(queue=w1892, error in (no error)=w1889) -> (error out=w1895:errorcluster)  [unwired: 1 in, 2 out]
        n835 = Release Queue(queue=w1890, error in (no error)=w1889) -> (error out=w1888:errorcluster)  [unwired: 1 in, 2 out]
        n836 = Merge Errors(w1896, w1895, w1888) -> (w1894:errorcluster)
        n837 = call <vilib>:"Simple Error Handler.vi"("error in (no error)"=w1894) -> ()  [unwired: 4 in, 5 out]
        n838 = call <vilib>:"Add State(s) to Queue__JKI_lib_State_Machine.vi"("State(s) in (\"\")"=w1899) -> ("States Out"=w1898:string)  [unwired: 14 in]
      }
      frame "---------- Run ----------" {
        # "Template Separator\n(You can make a copy of, or modify, this frame)"
        n839 = call <vilib>:"Add State(s) to Queue__JKI_lib_State_Machine.vi"("State(s) in (\"\")"=w1904) -> ("States Out"=w1903:string)  [unwired: 14 in]
      }
      frame "Run: CaliIncrement" {
        # "Increment Calibration #\n(You can make a copy of, or modify, this frame)"
        n840 = Unbundle By Name(w1906) -> ("IDs.Cali ID"=w1908:i8)
        n841 = Increment(x=w1908) -> (x+1=w1905:i8)
        n842 = Bundle By Name(cluster=w1906, "IDs.Cali ID"=w1905) -> (w1907:T23)
        n843 = call <vilib>:"Add State(s) to Queue__JKI_lib_State_Machine.vi"("State(s) in (\"\")"=w1912) -> ("States Out"=w1911:string)  [unwired: 14 in]
      }
      frame "Run: BGIncrement" {
        # "Increment BG #\n(You can make a copy of, or modify, this frame)"
        n844 = Unbundle By Name(w1913) -> ("IDs.BG ID"=w1916:i8)
        n845 = Increment(x=w1916) -> (x+1=w1915:i8)
        n846 = Bundle By Name(cluster=w1913, "IDs.BG ID"=w1915) -> (w1914:T23)
        n847 = call <vilib>:"Add State(s) to Queue__JKI_lib_State_Machine.vi"("State(s) in (\"\")"=w1920) -> ("States Out"=w1919:string)  [unwired: 14 in]
      }
      frame "Run: Increment" {
        # "Increase Run# by 1"
        n848 = Unbundle By Name(w1925) -> ("IDs.RunID"=w1927:i8)
        n849 = Increment(x=w1927) -> (x+1=w1923:i8)
        n850 = Bundle By Name(cluster=w1925, "IDs.RunID"=w1923) -> (w1926:T23)
        n851 = call "RunIDFGV.vi"("Error In"=w1921, "RunID in"=w1923) -> ("Error Out"=w1922:errorcluster)  [unwired: 8 in, 1 out]
        n852 = call <vilib>:"Add State(s) to Queue__JKI_lib_State_Machine.vi"("State(s) in (\"\")"=w1929) -> ("States Out"=w1928:string)  [unwired: 14 in]
      }
      frame "Run: Decrement" {
        # "Increase Run# by 1"
        n853 = Unbundle By Name(w1934) -> ("IDs.RunID"=w1936:i8)
        n854 = Decrement(x=w1936) -> (x-1=w1932:i8)
        n855 = Bundle By Name(cluster=w1934, "IDs.RunID"=w1932) -> (w1935:T23)
        n856 = call "RunIDFGV.vi"("Error In"=w1930, "RunID in"=w1932) -> ("Error Out"=w1931:errorcluster)  [unwired: 8 in, 1 out]
        n857 = call <vilib>:"Add State(s) to Queue__JKI_lib_State_Machine.vi"("State(s) in (\"\")"=w1938) -> ("States Out"=w1937:string)  [unwired: 14 in]
      }
      frame "---------- SysConfig ----------" {
        # "Template Separator\n(You can make a copy of, or modify, this frame)"
        n858 = call <vilib>:"Add State(s) to Queue__JKI_lib_State_Machine.vi"("State(s) in (\"\")"=w1943) -> ("States Out"=w1942:string)  [unwired: 14 in]
      }
      frame "SysConfig: LoadAPDSerialNumber" {
        # "Template Separator\n(You can make a copy of, or modify, this frame)"
        n859 = call "readAPDSerial.vi"("Error In"=w1945) -> ("Error Out"=w1944:errorcluster, "output cluster"=w1946:T26)  [unwired: 9 in]
        n860 = Bundle By Name(cluster=w1947, "APDSerialNum"=w1946) -> (w1948:T23)
        n861 = call <vilib>:"Add State(s) to Queue__JKI_lib_State_Machine.vi"("State(s) in (\"\")"=w1951) -> ("States Out"=w1950:string)  [unwired: 14 in]
      }
      frame "SysConfig: Load Sys Config" {
        # "[Covers: REQ5]"
        # "Load System config"
        # "Load system configuration\n(Load both hardware and DAQ config)"
        n862 = call "LoadSysConfig.vi"("Error In"=w1954, "Enum"=enum16{"LastUse", "Default"}."LastUse") -> ("Error Out"=w1953:errorcluster, "SysConfigCluster"=w1956:T4)  [unwired: 8 in]
        "SysConfigCluster" <- w1956
        n863 = Bundle By Name(cluster=w1957, "SysConfigCluster"=w1956) -> (w1958:T23)
        n864 = call <vilib>:"Add State(s) to Queue__JKI_lib_State_Machine.vi"("State(s) in (\"\")"=w1960) -> ("States Out"=w1959:string)  [unwired: 14 in]
      }
      frame "SysConfig: Load Digitizer Setting" {
        w1961 = enum16{"Write", "Read"}."Write" ("Operation")
        # "Load DAQ config\nSave to FGV"
        # "Template Separator\n(You can make a copy of, or modify, this frame)"
        n865 = call <userlib>:"Current VIs Parent Directory__ogtk.vi"() -> ("Parent Directory (+ Relative)"=w1975:path)  [unwired: 5 in]
        n866 = Build Path(base path=w1975, name or relative path="SubVI\\DigitizerConfiguration\\V6_Scope_last_use.config") -> (appended path=w1976:path)
        n867 = call "ReadDigitizerConfig(SubVI).vi"("error in (no error)"=w1973, "appended path"=w1976) -> ("error out"=w1969:errorcluster, "FLImDAQ"=w1967:T6)  [unwired: 8 in]
        n868 = call "FLImDAQ_FGV.vi"("error in (no error)"=w1969, "Operation (Read)"=w1961, "Write data"=w1967) -> ("error out"=w1971:errorcluster)  [unwired: 7 in, 1 out]
        n869 = Unbundle By Name(w1967) -> ("min record length"=→"data length":i32, "Digitizer 1"=w1963:refnum<k15>, "Digitizer 2"=w1970:refnum<k15>)
        n870 = Bundle By Name(cluster=w1965, "FLImDAQ"=w1967) -> (w1966:T23)
        n871 = call "Digitizer1_FGV.vi"("error in (no error)"=w1971, "Operation (Read)"=w1961, "Write data"=w1963) -> ("error out"=w1972:errorcluster)  [unwired: 7 in, 1 out]
        n872 = call "Digitizer2_FGV.vi"("error in (no error)"=w1972, "Operation (Read)"=w1961, "Write data"=w1970) -> ("error out"=w1968:errorcluster)  [unwired: 7 in, 1 out]
        n873 = call <vilib>:"Add State(s) to Queue__JKI_lib_State_Machine.vi"("State(s) in (\"\")"=w1978) -> ("States Out"=w1977:string)  [unwired: 14 in]
      }
      frame "SysConfig: Load LJ Pinout" {
        # "Template Separator\n(You can make a copy of, or modify, this frame)"
        n874 = call <userlib>:"Current VIs Parent Directory__ogtk.vi"() -> ("Parent Directory (+ Relative)"=w1993:path)  [unwired: 5 in]
        n875 = Build Path(base path=w1993, name or relative path="SubVI\\LabJack\\LJ_pin_setting.config") -> (appended path=w1991:path)
        n876 = call "ReadLabjackConfig(SubVI).vi"("error in (no error)"=w1989, "appended path"=w1991) -> ("error out"=w1990:errorcluster, "Utility"=w1987:T5)  [unwired: 8 in]
        n877 = Unbundle By Name(w1987) -> ("Ch1 Bias"=w1986:string, "Ch2 Bias"=w1985:string, "Ch3 Bias"=w1984:string, "Ch4 Bias"=w1979:string, "Red LED"=w1981:string, "Green LED"=w1980:string)
        n878 = global write "GlobalVariables.vi" "LED Green pin"(w1980) -> ()
        n879 = global write "GlobalVariables.vi" "Ch1 LJ pin"(w1986) -> ()
        n880 = global write "GlobalVariables.vi" "Ch2 LJ pin"(w1985) -> ()
        n881 = global write "GlobalVariables.vi" "Ch3 LJ pin"(w1984) -> ()
        n882 = global write "GlobalVariables.vi" "Ch4 LJ pin"(w1979) -> ()
        n883 = global write "GlobalVariables.vi" "LED Red pin"(w1981) -> ()
        n884 = Bundle By Name(cluster=w1982, "LJ Pinout"=w1987) -> (w1988:T23)
        n885 = call <vilib>:"Add State(s) to Queue__JKI_lib_State_Machine.vi"("State(s) in (\"\")"=w1995) -> ("States Out"=w1994:string)  [unwired: 14 in]
      }
      frame "SysConfig: Load 355 PWM" {
        # "Template Separator\n(You can make a copy of, or modify, this frame)"
        n886 = call <userlib>:"Current VIs Parent Directory__ogtk.vi"() -> ("Parent Directory (+ Relative)"=w2013:path)  [unwired: 5 in]
        n887 = Build Path(base path=w2013, name or relative path="SubVI\\LabJack\\PWM_setting_355.config") -> (appended path=w2011:path)
        n888 = call "ReadPWMConfig(SubVI).vi"("error in (no error)"=w2008, "appended path"=w2011) -> ("error out"=w2009:errorcluster, "PWM Setting"=w2007:T40)  [unwired: 8 in]
        n889 = Unbundle By Name(w2007) -> ("DIO_EF_CLOCK1_DIVISOR"=w2004:i16, "DIO_EF_CLOCK1_ROLL_VALUE"=w2003:i32)
        n890 = Multiply(x=w2004, y=w2003) -> (x*y=w2005:i32)
        n891 = Bundle By Name(cluster=w2010, "355 PWM setting"=w2007) -> (w1997:T23)
        n892 = Divide(x=80000000.0, y=w2005) -> (x/y=w2002:dbl)
        "Laser Rep Rate" <- w2002
        n893 = Number To Decimal String(number=w2002) -> (decimal integer string=w2001:string)  [unwired: 1 in]
        n894 = Concatenate Strings("355nm " ("string"), w2001, "Hz" ("string")) -> (w1999:string)
        n895 = property on="355nm Laser toggle" class="Bool (strict)"("Caption.Text"=w1999) -> ()  [unwired: 2 in, 2 out]
        n896 = call <vilib>:"Add State(s) to Queue__JKI_lib_State_Machine.vi"("State(s) in (\"\")"=w2015) -> ("States Out"=w2014:string)  [unwired: 14 in]
      }
      frame "SysConfig: Load AB PWM" {
        # "Template Separator\n(You can make a copy of, or modify, this frame)"
        n897 = call <userlib>:"Current VIs Parent Directory__ogtk.vi"() -> ("Parent Directory (+ Relative)"=w2024:path)  [unwired: 5 in]
        n898 = Build Path(base path=w2024, name or relative path="SubVI\\LabJack\\PWM_setting_AB.config") -> (appended path=w2022:path)
        n899 = call "ReadPWMConfig(SubVI).vi"("error in (no error)"=w2019, "appended path"=w2022) -> ("error out"=w2020:errorcluster, "PWM Setting"=w2018:T40)  [unwired: 8 in]
        n900 = Bundle By Name(cluster=w2016, "AB PWM setting"=w2018) -> (w2021:T23)
        n901 = call <vilib>:"Add State(s) to Queue__JKI_lib_State_Machine.vi"("State(s) in (\"\")"=w2026) -> ("States Out"=w2025:string)  [unwired: 14 in]
      }
      frame "SysConfig: Load AB setting" {
        # "load aming beam setting\n(check frequency, if 0 do nothing, if not zero, config PWM)"
        n902 = call "readAimingBeamSetting.vi"("error in (no error)"=w2044) -> ("error out"=w2039:errorcluster, "Aiming Beam Setting"=w2031:T41)  [unwired: 9 in]
        n903 = Unbundle By Name(w2031) -> ("Default Current"=w2030:dbl)
        n904 = Unbundle By Name(w2031) -> ("Frequency(Hz)"=w2027:u32)
        n905 = Equal To 0?(x=w2027) -> (x = 0?=w2037:bool)
        n906 = Select(t="", s=w2037, f="SysConfig: Load AB PWM" ("State(s) in Front (\"\")")) -> (s? t:f=w2040:string)
        n907 = Number To Decimal String(number=w2027) -> (decimal integer string=w2036:string)  [unwired: 1 in]
        n908 = Number To Decimal String(number=w2030, width (-)=i16 2) -> (decimal integer string=w2029:string)
        n909 = Concatenate Strings("445nm " ("string"), w2036, "Hz " ("string"), w2029, "mA" ("string")) -> (w2035:string)
        n910 = property on="Aiming beam toggle" class="Bool (strict)"("Caption.Text"=w2035) -> ()  [unwired: 2 in, 2 out]
        n911 = case shown="False" w2037 {
          tunnel: w2039 -> [w2052 w2055]
          tunnel: [w2051 w2055] -> w2038
          tunnel: w2027 -> [w2050 _]
          frame False {
            n912 = call "LJ_calculate_PWM_parameters.vi"("Duty Cycle (%)"=u32 10, "Error In"=w2052, "Show Confirmation"=FALSE, "Laser Rep Rate (Hz)"=w2050, "Laser"=enum16{"355nm", "AimingBeam"}."AimingBeam") -> ("Error Out"=w2051:errorcluster)  [unwired: 5 in, 1 out]
          }
          frame True {
          }
        }
        n913 = Bundle By Name(cluster=w2045, "AB Cluster"=w2031) -> (w2046:T23)
        n914 = call <vilib>:"Add State(s) to Queue__JKI_lib_State_Machine.vi"("State(s) in Front (\"\")"=w2040, "State(s) in (\"\")"=w2048) -> ("States Out"=w2047:string)  [unwired: 13 in]
      }
      frame "SysConfig: LoadABVideoSetting" {
        # "Load AB video setting form ini file\n()"
        n915 = call "readVideoConfig.vi"("error in (no error)"=w2059) -> ("error out"=w2060:errorcluster, "Aiming Beam Config"=w2058:T22)  [unwired: 8 in, 1 out]
        n916 = Bundle By Name(cluster=w2056, "VideoConfig"=w2058) -> (w2057:T23)
        n917 = call <vilib>:"Add State(s) to Queue__JKI_lib_State_Machine.vi"("State(s) in (\"\")"=w2063) -> ("States Out"=w2062:string)  [unwired: 14 in]
      }
      frame "SysConfig: LoadCursorLocation" {
        # "Load cursor location from ini file\n(load cursor from system setting ini file)"
        n918 = call "readCursorConfigMain.vi"("error in (no error)"=w2075) -> ("error out"=w2076:errorcluster, "Cursor Locations"=w2074:T42)  [unwired: 9 in]
        n919 = Unbundle By Name(w2074) -> ("DC1"=w2073:i32, "DC2"=w2072:i32, "BG1"=w2067:i32, "BG2"=w2066:i32)
        n920 = Build Array(w2073, w2072) -> (w2071:i32[])
        n921 = Build Array(w2067, w2066) -> (w2068:i32[])
        n922 = Array Max & Min(array=w2071) -> (max value=w2070:i32, min value=w2069:i32)  [unwired: 2 out]
        n923 = Array Max & Min(array=w2068) -> (max value=w2065:i32, min value=w2064:i32)  [unwired: 2 out]
        n924 = global write "GlobalVariables.vi" "DC Idx2"(w2070) -> ()
        n925 = global write "GlobalVariables.vi" "DC Idx1"(w2069) -> ()
        n926 = global write "GlobalVariables.vi" "BG Idx2"(w2065) -> ()
        n927 = global write "GlobalVariables.vi" "BG Idx1"(w2064) -> ()
        n928 = call <vilib>:"Add State(s) to Queue__JKI_lib_State_Machine.vi"("State(s) in (\"\")"=w2080) -> ("States Out"=w2079:string)  [unwired: 14 in]
      }
      frame "---------- SystemStatus ----------" {
        # "Template Separator\n(You can make a copy of, or modify, this frame)"
        n929 = call <vilib>:"Add State(s) to Queue__JKI_lib_State_Machine.vi"("State(s) in (\"\")"=w2085) -> ("States Out"=w2084:string)  [unwired: 14 in]
      }
      frame "SystemStatus: SlowSysStatusMacro" {
        # "store system check time"
        # "Template Separator\n(You can make a copy of, or modify, this frame)"
        n930 = Tick Count (ms)() -> (millisecond timer value=w2088:u32)
        n931 = Bundle By Name(cluster=w2086, "SlowTimer"=w2088) -> (w2087:T23)
        n932 = call <vilib>:"Add State(s) to Queue__JKI_lib_State_Machine.vi"("State(s) in Front (\"\")"="Digitizer: checkTemp\nTCP: CheckConnection" ("State(s) in Front (\"\")"), "State(s) in (\"\")"=w2093) -> ("States Out"=w2092:string)  [unwired: 13 in]
      }
      frame "SystemStatus: FastSysStatusMacro" {
        # "store system check time"
        # "Template Separator\n(You can make a copy of, or modify, this frame)"
        n933 = Tick Count (ms)() -> (millisecond timer value=w2096:u32)
        n934 = Bundle By Name(cluster=w2094, "FastTimer"=w2096) -> (w2095:T23)
        n935 = call <vilib>:"Add State(s) to Queue__JKI_lib_State_Machine.vi"("State(s) in Front (\"\")"="355 Laser: CheckPWMStatus\n/*AimingBeam: GetPWMStatus\n/*355 Laser: CheckControllerStatus" ("State(s) in Front (\"\")"), "State(s) in (\"\")"=w2101) -> ("States Out"=w2100:string)  [unwired: 13 in]
      }
      frame "---------- UI ----------" {
        # "Do not put any code in this frame.\n(It is a separator no-op. You can make a copy of this frame to create a new UI frame)"
        n936 = call <vilib>:"Add State(s) to Queue__JKI_lib_State_Machine.vi"("State(s) in (\"\")"=w2106) -> ("States Out"=w2105:string)  [unwired: 14 in]
      }
      frame "UI: Initialize" {
        w2108 = T43 {"Minimum"=0.0, "Maximum"=4.6, "Increment"=0.1} ("Data Entry Limits")
        w2107 = T11."Disabled and Grayed Out" ("Disabled")
        # "Disable all button on startup"
        # "Initialize the User Interface, here.\n(this is called automatically, by the Macro: Init)"
        n937 = property on="V 1" class="DigNum (strict)"("DisabledEnum"=w2107) -> ()  [unwired: 2 in, 2 out]
        n938 = property on="V 2" class="DigNum (strict)"("DisabledEnum"=w2107) -> ()  [unwired: 2 in, 2 out]
        n939 = property on="StopButton" class="Bool (strict)"("DisabledEnum"=w2107) -> ()  [unwired: 2 in, 2 out]
        n940 = property on="Sys Reconfig" class="Bool"("DisabledEnum"=w2107) -> ()  [unwired: 2 in, 2 out]
        n941 = property on="StartButton" class="Bool (strict)"("DisabledEnum"=w2107) -> ()  [unwired: 2 in, 2 out]
        n942 = property on="355nm Laser toggle" class="Bool (strict)"("DisabledEnum"=w2107) -> ()  [unwired: 2 in, 2 out]
        n943 = property on="Aiming beam toggle" class="Bool (strict)"("DisabledEnum"=w2107) -> ()  [unwired: 2 in, 2 out]
        n944 = property on="Background" class="Bool (strict)"("DisabledEnum"=w2107) -> ()  [unwired: 2 in, 2 out]
        n945 = property on="Cali&iRF alignment" class="Bool (strict)"("DisabledEnum"=w2107) -> ()  [unwired: 2 in, 2 out]
        n946 = property on="V 3" class="DigNum (strict)"("DisabledEnum"=w2107) -> ()  [unwired: 2 in, 2 out]
        n947 = property on="Video Source" class="RadioBtnsControl (strict)"("DisabledEnum"=w2107) -> ()  [unwired: 2 in, 2 out]
        n948 = property on="V 1" class="DigNum (strict)"("Data Range"=w2108) -> ()  [unwired: 2 in, 2 out]
        n949 = property on="V 2" class="DigNum (strict)"("Data Range"=w2108) -> ()  [unwired: 2 in, 2 out]
        n950 = property on="V 3" class="DigNum (strict)"("Data Range"=w2108) -> ()  [unwired: 2 in, 2 out]
        n951 = call <vilib>:"Add State(s) to Queue__JKI_lib_State_Machine.vi"("State(s) in Front (\"\")"="UI: CaliAndiRFNotReady" ("State(s) in Front (\"\")"), "State(s) in (\"\")"=w2114) -> ("States Out"=w2113:string)  [unwired: 13 in]
      }
      frame "UI: BGLoaded" {
        # "[Covers: REQ24]"
        # "Do not put any code in this frame.\n(It is a separator no-op. You can make a copy of this frame to create a new UI frame)"
        n952 = property on="Background" class="Bool (strict)"("BoolText.Text"="Loaded!" ("Boolean Text.Text"), "Colors [4]"=cluster{u32, u32}[] [{15764023, 15764023}, {16711680, 16711680}]) -> ()  [unwired: 2 in, 2 out]
        n953 = call <vilib>:"Add State(s) to Queue__JKI_lib_State_Machine.vi"("State(s) in (\"\")"=w2121) -> ("States Out"=w2120:string)  [unwired: 14 in]
      }
      frame "UI: BGSizeError" {
        # "[Covers: REQ24]"
        # "Do not put any code in this frame.\n(It is a separator no-op. You can make a copy of this frame to create a new UI frame)"
        n954 = property on="Background" class="Bool (strict)"("BoolText.Text"="Loaded!" ("Boolean Text.Text"), "Colors [4]"=cluster{u32, u32}[] [{7171459, 7171459}, {16711680, 16711680}]) -> ()  [unwired: 2 in, 2 out]
        n955 = One Button Dialog(message="Background waveform length and current digitizer setting mismatch! Please take a new background before any aquisition!") -> ()  [unwired: 1 in, 1 out]
        n956 = call <vilib>:"Add State(s) to Queue__JKI_lib_State_Machine.vi"("State(s) in (\"\")"=w2129) -> ("States Out"=w2128:string)  [unwired: 14 in]
      }
      frame "UI: CaliAndiRFLoaded" {
        # "[Covers: REQ24]"
        # "Do not put any code in this frame.\n(It is a separator no-op. You can make a copy of this frame to create a new UI frame)"
        n957 = property on="Cali&iRF alignment" class="Bool (strict)"("BoolText.Text"="Loaded!" ("Boolean Text.Text"), "Colors [4]"=cluster{u32, u32}[] [{15764023, 15764023}, {16711680, 16711680}]) -> ()  [unwired: 2 in, 2 out]
        n958 = call <vilib>:"Add State(s) to Queue__JKI_lib_State_Machine.vi"("State(s) in (\"\")"=w2136) -> ("States Out"=w2135:string)  [unwired: 14 in]
      }
      frame "UI: WFAutoScale" {
        # "Set graph auto scale.\n(UI: WFAutoScale >> T/F)"
        n959 = Equal?(x=w2137, y="F") -> (x = y?=w2138:bool)
        n960 = Equal?(x=w2137, y="T") -> (x = y?=w2140:bool)
        n961 = case shown="True" w2140 {
          frame False {
          }
          frame True {
            w2156 = u8 2 ("Y Scale.Scale Fit")
            n962 = property on="Channel 1" class="WFGraph (strict)"("YScale.ScaleFit"=w2156) -> ()  [unwired: 2 in, 2 out]
            n963 = property on="Channel 2" class="WFGraph (strict)"("YScale.ScaleFit"=w2156) -> ()  [unwired: 2 in, 2 out]
            n964 = property on="Channel 3" class="WFGraph (strict)"("YScale.ScaleFit"=w2156) -> ()  [unwired: 2 in, 2 out]
          }
        }
        n965 = case shown="True" w2138 {
          frame False {
          }
          frame True {
            w2153 = 0.0 ("Y Scale.Range:Maximum")
            w2154 = 2.0 ("Y Scale.Range:Maximum")
            w2155 = u8 0 ("Y Scale.Scale Fit")
            n966 = property on="Channel 1" class="WFGraph (strict)"("YScale.ScaleFit"=w2155) -> (error out=w2152:errorcluster)  [unwired: 2 in, 1 out]
            n967 = property on="Channel 2" class="WFGraph (strict)"("YScale.ScaleFit"=w2155) -> (error out=w2151:errorcluster)  [unwired: 2 in, 1 out]
            n968 = property on="Channel 3" class="WFGraph (strict)"("YScale.ScaleFit"=w2155) -> (error out=w2150:errorcluster)  [unwired: 2 in, 1 out]
            n969 = property on="Channel 1" class="WFGraph (strict)"(error in=w2152, "YScale.Maximum"=w2154) -> (error out=w2149:errorcluster)  [unwired: 1 in, 1 out]
            n970 = property on="Channel 2" class="WFGraph (strict)"(error in=w2151, "YScale.Maximum"=w2154) -> (error out=w2148:errorcluster)  [unwired: 1 in, 1 out]
            n971 = property on="Channel 3" class="WFGraph (strict)"(error in=w2150, "YScale.Maximum"=w2154) -> (error out=w2147:errorcluster)  [unwired: 1 in, 1 out]
            n972 = property on="Channel 1" class="WFGraph (strict)"(error in=w2149, "YScale.Minimum"=w2153) -> ()  [unwired: 1 in, 2 out]
            n973 = property on="Channel 2" class="WFGraph (strict)"(error in=w2148, "YScale.Minimum"=w2153) -> ()  [unwired: 1 in, 2 out]
            n974 = property on="Channel 3" class="WFGraph (strict)"(error in=w2147, "YScale.Minimum"=w2153) -> ()  [unwired: 1 in, 2 out]
          }
        }
        n975 = call <vilib>:"Add State(s) to Queue__JKI_lib_State_Machine.vi"("State(s) in (\"\")"=w2146) -> ("States Out"=w2145:string)  [unwired: 14 in]
      }
      frame "UI: showDisclaimer" {
        # "Show disclamer window.\n(It is a separator no-op. You can make a copy of this frame to create a new UI frame)"
        n976 = call <vilib>:"Application Directory.vi"() -> ("Application Directory"=w2169:path)
        n977 = Build Path(base path=w2169, name or relative path="Disclamer.png") -> (appended path=w2167:path)
        n978 = property on="Disclamer" class="Pict"() -> ("Draw Area Size"=w2165:T44)  [unwired: 2 in, 2 out]
        n979 = disable-structure "Diagram Disable Structure" shown="Disabled" {
          frame Disabled {
            n980 = flat-sequence {
              frame #0 {
                n981 = call "disclaimer.vi"() -> ()  [unwired: 12 in]
              }
              frame #1 {
                n982 = Wait (ms)(milliseconds to wait=u32 250) -> ()  [unwired: 1 out]
              }
              frame #2 {
                n983 = call "SoftwareNote.vi"() -> ()  [unwired: 12 in]
              }
            }
          }
          frame Enabled {
          }
        }
        n984 = call <vilib>:"Read PNG File.vi"("path to PNG file"=w2167) -> ("image data"=w2164:T45)  [unwired: 8 in, 2 out]
        n985 = Unbundle By Name(w2164) -> ("Rectangle.right"=w2162:i16, "Rectangle.bottom"=w2160:i16)
        n986 = Unbundle By Name(w2165) -> ("Width"=w2163:u32, "Height"=w2161:u32)
        n987 = call <vilib>:"Draw Flattened Pixmap.vi"("image data"=w2164) -> ("new picture"=→"Disclamer":picture)  [unwired: 8 in]
        n988 = Divide(x=w2163, y=w2162) -> (x/y=w2159:dbl)
        n989 = Divide(x=w2161, y=w2160) -> (x/y=w2158:dbl)
        n990 = Max & Min(x=w2159, y=w2158) -> (min(x,y)=w2157:dbl)  [unwired: 1 out]
        n991 = property on="Disclamer" class="Pict"("ZoomFactor"=w2157) -> ()  [unwired: 2 in, 2 out]
        n992 = call <vilib>:"Add State(s) to Queue__JKI_lib_State_Machine.vi"("State(s) in (\"\")"=w2174) -> ("States Out"=w2173:string)  [unwired: 14 in]
      }
      frame "UI: CaliAndiRFNotReady" {
        # "Do not put any code in this frame.\n(It is a separator no-op. You can make a copy of this frame to create a new UI frame)"
        n993 = property on="Cali&iRF alignment" class="Bool (strict)"("BoolText.Text"="No Info" ("Boolean Text.Text"), "Colors [4]"=cluster{u32, u32}[] [{13816530, 13816530}, {16711680, 16711680}]) -> ()  [unwired: 2 in, 2 out]
        n994 = call <vilib>:"Add State(s) to Queue__JKI_lib_State_Machine.vi"("State(s) in (\"\")"=w2182) -> ("States Out"=w2181:string)  [unwired: 14 in]
      }
      frame "UI: BGnotReady" {
        # "Do not put any code in this frame.\n(It is a separator no-op. You can make a copy of this frame to create a new UI frame)"
        n995 = property on="Background" class="Bool (strict)"("BoolText.Text"="No Info" ("Boolean Text.Text"), "Colors [4]"=cluster{u32, u32}[] [{13816530, 13816530}, {16711680, 16711680}]) -> ()  [unwired: 2 in, 2 out]
        n996 = call <vilib>:"Add State(s) to Queue__JKI_lib_State_Machine.vi"("State(s) in (\"\")"=w2189) -> ("States Out"=w2188:string)  [unwired: 14 in]
      }
      frame "UI: Reset" {
        w2191 = cluster{u32, u32}[] [{13816530, 13816530}, {13816530, 13816530}] ("Colors [4]")
        # "Do not put any code in this frame.\n(It is a separator no-op. You can make a copy of this frame to create a new UI frame)"
        n997 = property on="Cali&iRF alignment" class="Bool (strict)"("BoolText.Text"="No Info" ("Boolean Text.Text"), "Colors [4]"=w2191) -> ()  [unwired: 2 in, 2 out]
        n998 = property on="Background" class="Bool (strict)"("BoolText.Text"="No Info" ("Boolean Text.Text"), "Colors [4]"=w2191) -> ()  [unwired: 2 in, 2 out]
        n999 = call <vilib>:"Add State(s) to Queue__JKI_lib_State_Machine.vi"("State(s) in (\"\")"=w2197) -> ("States Out"=w2196:string)  [unwired: 14 in]
      }
      frame "UI: SetButtonText" {
        # "Set button text of 355nm laser and aiming beam."
        n1000 = call <vilib>:"Add State(s) to Queue__JKI_lib_State_Machine.vi"("State(s) in (\"\")"=w2202) -> ("States Out"=w2201:string)  [unwired: 14 in]
      }
      frame "UI: DuringAquisition" {
        w2205 = T11."Disabled and Grayed Out" ("Disabled")
        # "Do not put any code in this frame.\n(It is a separator no-op. You can make a copy of this frame to create a new UI frame)"
        n1001 = Unbundle By Name(w2204) -> ("bothVidSourceAvail"=w2203:bool)
        n1002 = case shown="True" w2203 {
          tunnel: w2205 -> [_ w2211]
          frame False {
          }
          frame True {
            n1003 = property on="Video Source" class="RadioBtnsControl (strict)"("DisabledEnum"=w2211) -> ()  [unwired: 2 in, 2 out]
          }
        }
        n1004 = property on="StartButton" class="Bool (strict)"("DisabledEnum"=w2205) -> ()  [unwired: 2 in, 2 out]
        n1005 = property on="Sys Reconfig" class="Bool"("DisabledEnum"=w2205) -> ()  [unwired: 2 in, 2 out]
        n1006 = property on="355nm Laser toggle" class="Bool (strict)"("DisabledEnum"=w2205) -> ()  [unwired: 2 in, 2 out]
        n1007 = property on="Aiming beam toggle" class="Bool (strict)"("DisabledEnum"=w2205) -> ()  [unwired: 2 in, 2 out]
        n1008 = property on="Background" class="Bool (strict)"("DisabledEnum"=w2205) -> ()  [unwired: 2 in, 2 out]
        n1009 = property on="Radio Buttons" class="RadioBtnsControl (strict)"("DisabledEnum"=w2205) -> ()  [unwired: 2 in, 2 out]
        n1010 = property on="Cali&iRF alignment" class="Bool (strict)"("DisabledEnum"=w2205) -> ()  [unwired: 2 in, 2 out]
        n1011 = property on="Quit" class="Bool"("DisabledEnum"=w2205) -> ()  [unwired: 2 in, 2 out]
        n1012 = property on="Skip Data Save?" class="Bool (strict)"("DisabledEnum"=w2205) -> ()  [unwired: 2 in, 2 out]
        n1013 = property on="Video Display" class="Bool (strict)"("DisabledEnum"=w2205) -> ()  [unwired: 2 in, 2 out]
        n1014 = property on="StopButton" class="Bool (strict)"("DisabledEnum"=T11."Enabled" ("Disabled")) -> ()  [unwired: 2 in, 2 out]
        n1015 = call <vilib>:"Add State(s) to Queue__JKI_lib_State_Machine.vi"("State(s) in (\"\")"=w2210) -> ("States Out"=w2209:string)  [unwired: 14 in]
      }
      frame "UI: duringIRFAlign" {
        w2212 = T11."Disabled and Grayed Out" ("Disabled")
        # "Set UI to during iRF alignment\n(It is a separator no-op. You can make a copy of this frame to create a new UI frame)"
        n1016 = property on="StartButton" class="Bool (strict)"("DisabledEnum"=w2212) -> ()  [unwired: 2 in, 2 out]
        n1017 = property on="Sys Reconfig" class="Bool"("DisabledEnum"=w2212) -> ()  [unwired: 2 in, 2 out]
        n1018 = property on="355nm Laser toggle" class="Bool (strict)"("DisabledEnum"=w2212) -> ()  [unwired: 2 in, 2 out]
        n1019 = property on="Aiming beam toggle" class="Bool (strict)"("DisabledEnum"=w2212) -> ()  [unwired: 2 in, 2 out]
        n1020 = property on="Background" class="Bool (strict)"("DisabledEnum"=w2212) -> ()  [unwired: 2 in, 2 out]
        n1021 = property on="StopButton" class="Bool (strict)"("DisabledEnum"=w2212) -> ()  [unwired: 2 in, 2 out]
        n1022 = call <vilib>:"Add State(s) to Queue__JKI_lib_State_Machine.vi"("State(s) in (\"\")"=w2217) -> ("States Out"=w2216:string)  [unwired: 14 in]
      }
      frame "UI: duringBGAcquire" {
        w2218 = T11."Disabled and Grayed Out" ("Disabled")
        # "Do not put any code in this frame.\n(It is a separator no-op. You can make a copy of this frame to create a new UI frame)"
        n1023 = property on="StartButton" class="Bool (strict)"("DisabledEnum"=w2218) -> ()  [unwired: 2 in, 2 out]
        n1024 = property on="StopButton" class="Bool (strict)"("DisabledEnum"=w2218) -> ()  [unwired: 2 in, 2 out]
        n1025 = property on="Sys Reconfig" class="Bool"("DisabledEnum"=w2218) -> ()  [unwired: 2 in, 2 out]
        n1026 = property on="355nm Laser toggle" class="Bool (strict)"("DisabledEnum"=w2218) -> ()  [unwired: 2 in, 2 out]
        n1027 = property on="Aiming beam toggle" class="Bool (strict)"("DisabledEnum"=w2218) -> ()  [unwired: 2 in, 2 out]
        n1028 = property on="Cali&iRF alignment" class="Bool (strict)"("DisabledEnum"=w2218) -> ()  [unwired: 2 in, 2 out]
        n1029 = call <vilib>:"Add State(s) to Queue__JKI_lib_State_Machine.vi"("State(s) in (\"\")"=w2223) -> ("States Out"=w2222:string)  [unwired: 14 in]
      }
      frame "UI: ReadyForAquisition" {
        w2227 = T11."Enabled" ("Disabled")
        # "Do not put any code in this frame.\n(It is a separator no-op. You can make a copy of this frame to create a new UI frame)"
        n1030 = Unbundle By Name(w2226) -> ("System Status.TCP/IP"=w2225:bool, "bothVidSourceAvail"=w2224:bool)
        n1031 = property on="StartButton" class="Bool (strict)"("DisabledEnum"=w2227) -> ()  [unwired: 2 in, 2 out]
        n1032 = property on="Sys Reconfig" class="Bool"("DisabledEnum"=w2227) -> ()  [unwired: 2 in, 2 out]
        n1033 = property on="355nm Laser toggle" class="Bool (strict)"("DisabledEnum"=w2227) -> ()  [unwired: 2 in, 2 out]
        n1034 = property on="Aiming beam toggle" class="Bool (strict)"("DisabledEnum"=w2227) -> ()  [unwired: 2 in, 2 out]
        n1035 = property on="Cali&iRF alignment" class="Bool (strict)"("DisabledEnum"=w2227) -> ()  [unwired: 2 in, 2 out]
        n1036 = property on="Background" class="Bool (strict)"("DisabledEnum"=w2227) -> ()  [unwired: 2 in, 2 out]
        n1037 = property on="Quit" class="Bool"("DisabledEnum"=w2227) -> ()  [unwired: 2 in, 2 out]
        n1038 = property on="Radio Buttons" class="RadioBtnsControl (strict)"("DisabledEnum"=w2227) -> ()  [unwired: 2 in, 2 out]
        n1039 = case shown="True" w2224 {
          tunnel: w2227 -> [_ w2233]
          frame False {
          }
          frame True {
            n1040 = property on="Video Source" class="RadioBtnsControl (strict)"("DisabledEnum"=w2233) -> ()  [unwired: 2 in, 2 out]
          }
        }
        n1041 = property on="Skip Data Save?" class="Bool (strict)"("DisabledEnum"=w2227) -> ()  [unwired: 2 in, 2 out]
        n1042 = case shown="True" w2225 {
          tunnel: w2227 -> [_ w2234]
          frame False {
          }
          frame True {
            n1043 = property on="Video Display" class="Bool (strict)"("DisabledEnum"=w2234) -> ()  [unwired: 2 in, 2 out]
          }
        }
        n1044 = property on="StopButton" class="Bool (strict)"("DisabledEnum"=T11."Disabled and Grayed Out" ("Disabled")) -> ()  [unwired: 2 in, 2 out]
        n1045 = call <vilib>:"Add State(s) to Queue__JKI_lib_State_Machine.vi"("State(s) in (\"\")"=w2232) -> ("States Out"=w2231:string)  [unwired: 14 in]
      }
      frame "UI: Update" {
        # "Do not put any code in this frame.\n(It is a separator no-op. You can make a copy of this frame to create a new UI frame)"
        n1046 = Unbundle By Name(w2245) -> ("System Status"=→"System Hardware Connection Status":T2, "IDs.RunID"=→"Run #":i8, "CaseID"=→"Case #":string, "FLImDAQ"=→"FLImDAQ":T30, "SysRunning?"=→"Aquisition Status:":bool, "LJ Pinout"=→"LJ Pinout":T5, "IDs.BG ID"=→"BG #":i8, "IDs.Cali ID"=→"Calibration #":i8, "video source"=→"Visualization PC video source":T1)
        n1047 = call <vilib>:"Add State(s) to Queue__JKI_lib_State_Machine.vi"("State(s) in (\"\")"=w2248) -> ("States Out"=w2247:string)  [unwired: 14 in]
      }
      frame "UI: updateVideoToggle" {
        # "Set video toggle based on visualization PC video source.\n(take )"
        n1048 = call <vilib>:"Add State(s) to Queue__JKI_lib_State_Machine.vi"("State(s) in (\"\")"=w2253) -> ("States Out"=w2252:string)  [unwired: 14 in]
      }
      frame "UI: Cursor Set" {
        # "Argument"
        # "Set and Unset Cursor Busy.\n(Usage: \"UI: Cursor Set >> Busy|Idle\")"
        n1049 = case shown="\"Idle\", Default" w2255 {
          tunnel: w2257 -> [w2262 w2264]
          tunnel: [w2261 w2263] -> w2256
          frame "Idle", Default {
            n1050 = call <vilib>:"Unset Busy.vi"("error in (no error)"=w2262) -> ("error out"=w2261:errorcluster)  [unwired: 10 in]
          }
          frame "Busy" {
            n1051 = call <vilib>:"Set Busy.vi"("error in (no error)"=w2264) -> ("error out"=w2263:errorcluster)  [unwired: 9 in, 1 out]
          }
        }
        n1052 = call <vilib>:"Add State(s) to Queue__JKI_lib_State_Machine.vi"("State(s) in (\"\")"=w2260) -> ("States Out"=w2259:string)  [unwired: 14 in]
      }
      frame "UI: Front Panel State" {
        # "Argument"
        # "Set Front Panel Open or Closed\n(Usage: \"UI: Front Panel State >> Open|Close\")"
        n1053 = Unbundle By Name(w2268) -> ("Core.Current VI Reference"=w2267:refnum<vi>)
        n1054 = case shown="\"Open\", \"Standard\", Default" w2266 {
          tunnel: w2270 -> [w2278 w2293 w2304 w2317 w2330]
          tunnel: [w2280 w2294 w2306 w2319 w2332] -> w2269
          tunnel: w2267 -> [w2279 w2291 w2305 w2318 w2331]
          frame "Open", "Standard", Default {
            w2273 = T17."Standard" ("State")
            n1055 = property on="Property Node" class="VI"(reference=w2279, error in=w2278) -> (reference out=w2276:refnum<vi>, error out=w2277:errorcluster, "FP.State"=w2275:T17)
            n1056 = Not Equal?(x=w2275, y=w2273) -> (x != y?=w2274:bool)
            n1057 = case shown="True" w2274 {
              tunnel: [w2284 w2286] -> w2280
              tunnel: w2277 -> [w2283 w2286]
              tunnel: w2276 -> [w2282 _]
              tunnel: w2273 -> [w2281 _]
              frame True {
                n1058 = invoke on="Invoke Node" class="VI" method="FP.Open"(reference=w2282, error in=w2283, "Activate"=TRUE, "State"=w2281) -> (error out=w2284:errorcluster)  [unwired: 1 in, 4 out]
              }
              frame False {
              }
            }
          }
          frame "Close", "Closed" {
            n1059 = property on="Property Node" class="VI"(reference=w2291, error in=w2293) -> (reference out=w2290:refnum<vi>, error out=w2292:errorcluster, "FP.State"=w2288:T17)
            n1060 = Not Equal?(x=w2288, y=T17."Closed" ("Front Panel Window:State")) -> (x != y?=w2287:bool)
            n1061 = case shown="True" w2287 {
              tunnel: [w2295 w2298] -> w2294
              tunnel: w2292 -> [w2295 w2297]
              tunnel: w2290 -> [_ w2296]
              frame False {
              }
              frame True {
                n1062 = invoke on="Invoke Node" class="VI" method="FP.Close"(reference=w2296, error in=w2297) -> (error out=w2298:errorcluster)  [unwired: 1 in, 2 out]
              }
            }
          }
          frame "Hidden", "Hide" {
            w2299 = T17."Hidden" ("State")
            n1063 = property on="Property Node" class="VI"(reference=w2305, error in=w2304) -> (reference out=w2302:refnum<vi>, error out=w2303:errorcluster, "FP.State"=w2301:T17)
            n1064 = Not Equal?(x=w2301, y=w2299) -> (x != y?=w2300:bool)
            n1065 = case shown="True" w2300 {
              tunnel: [w2310 w2311] -> w2306
              tunnel: w2303 -> [w2309 w2311]
              tunnel: w2302 -> [w2308 _]
              tunnel: w2299 -> [w2307 _]
              frame True {
                n1066 = invoke on="Invoke Node" class="VI" method="FP.Open"(reference=w2308, error in=w2309, "State"=w2307) -> (error out=w2310:errorcluster)  [unwired: 2 in, 4 out]
              }
              frame False {
              }
            }
          }
          frame "Minimize", "Minimized" {
            w2312 = T17."Minimized" ("State")
            n1067 = property on="Property Node" class="VI"(reference=w2318, error in=w2317) -> (reference out=w2315:refnum<vi>, error out=w2316:errorcluster, "FP.State"=w2314:T17)
            n1068 = Not Equal?(x=w2314, y=w2312) -> (x != y?=w2313:bool)
            n1069 = case shown="True" w2313 {
              tunnel: [w2323 w2324] -> w2319
              tunnel: w2316 -> [w2322 w2324]
              tunnel: w2315 -> [w2321 _]
              tunnel: w2312 -> [w2320 _]
              frame True {
                n1070 = invoke on="Invoke Node" class="VI" method="FP.Open"(reference=w2321, error in=w2322, "State"=w2320) -> (error out=w2323:errorcluster)  [unwired: 2 in, 4 out]
              }
              frame False {
              }
            }
          }
          frame "Maximize", "Maximized" {
            w2325 = T17."Maximized" ("State")
            n1071 = property on="Property Node" class="VI"(reference=w2331, error in=w2330) -> (reference out=w2328:refnum<vi>, error out=w2329:errorcluster, "FP.State"=w2327:T17)
            n1072 = Not Equal?(x=w2327, y=w2325) -> (x != y?=w2326:bool)
            n1073 = case shown="True" w2326 {
              tunnel: [w2336 w2337] -> w2332
              tunnel: w2329 -> [w2335 w2337]
              tunnel: w2328 -> [w2334 _]
              tunnel: w2325 -> [w2333 _]
              frame True {
                n1074 = invoke on="Invoke Node" class="VI" method="FP.Open"(reference=w2334, error in=w2335, "State"=w2333) -> (error out=w2336:errorcluster)  [unwired: 2 in, 4 out]
              }
              frame False {
              }
            }
          }
        }
        n1075 = call <vilib>:"Add State(s) to Queue__JKI_lib_State_Machine.vi"("State(s) in (\"\")"=w2272) -> ("States Out"=w2271:string)  [unwired: 14 in]
      }
      frame "---------- AimingBeam ----------" {
        # "Template Separator\n(You can make a copy of, or modify, this frame)"
        n1076 = call <vilib>:"Add State(s) to Queue__JKI_lib_State_Machine.vi"("State(s) in (\"\")"=w2342) -> ("States Out"=w2341:string)  [unwired: 14 in]
      }
      frame "AimingBeam: Initialize" {
        # "set aiming beam button color"
        # "Open COM port for Aiming Beam\n(Require USB connection)"
        n1077 = Unbundle By Name(w2344) -> ("AB Cluster.Aiming Beam COM Port"=w2352:refnum<visa-resource-name>)
        n1078 = call-poly "VISA Configure Serial Port"("VISA resource name"=w2352, "Enable Termination\nChar (T)"=TRUE ("Enable Termination\nChar (T)"), "baud rate (9600)"=u32 9600, "error in (no error)"=w2349) -> ("error out"=w2348:errorcluster)  [unwired: 10 in, 1 out]
        n1079 = Unbundle By Name(w2348) -> ("status"=w2347:bool)
        n1080 = Not(x=w2347) -> (.not. x?=w2346:bool)
        n1081 = Bundle By Name(cluster=w2344, "System Status.Aiming Beam"=w2346) -> (w2345:T23)
        n1082 = call <vilib>:"Add State(s) to Queue__JKI_lib_State_Machine.vi"("State(s) in (\"\")"=w2354) -> ("States Out"=w2353:string)  [unwired: 14 in]
      }
      frame "AimingBeam: Close" {
        # "Close Aiming Beam COM port\n(Require USB connection to Aiming Beam Laser)"
        n1083 = Unbundle By Name(w2357) -> ("AB Cluster.Aiming Beam COM Port"=w2361:refnum<visa-resource-name>)
        n1084 = VISA Close(VISA resource name=w2361, error in (no error)=w2359) -> (error out=w2360:errorcluster)
        n1085 = Bundle By Name(cluster=w2357, "System Status.Aiming Beam"=FALSE) -> (w2358:T23)
        n1086 = call <vilib>:"Add State(s) to Queue__JKI_lib_State_Machine.vi"("State(s) in (\"\")"=w2363) -> ("States Out"=w2362:string)  [unwired: 14 in]
      }
      frame "AimingBeam: Set Current" {
        # "Set Aiming Beam Current\n(You can make a copy of, or modify, this frame)"
        n1087 = Unbundle By Name(w2378) -> ("AB Cluster.Aiming Beam COM Port"=w2371:refnum<visa-resource-name>, "AB Cluster.Max Current"=w2367:dbl, "AB Cluster.Default Current"=w2369:dbl, "AB Cluster.Min Current"=w2368:dbl)
        n1088 = In Range and Coerce(upper limit=w2367, x=w2369, lower limit=w2368) -> (coerced(x)=w2364:dbl)  [unwired: 1 out]
        n1089 = Number To Fractional String(number=w2364, precision (6)=i16 2) -> (F-format string=w2372:string)  [unwired: 2 in]
        n1090 = Concatenate Strings("slc:", w2372, "\r" ("Carriage Return Constant"), "\n" ("Line Feed Constant")) -> (w2375:string)
        n1091 = VISA Write(VISA resource name=w2371, write buffer=w2375, error in (no error)=w2366) -> (error out=w2370:errorcluster)  [unwired: 2 out]
        n1092 = call <vilib>:"Add State(s) to Queue__JKI_lib_State_Machine.vi"("State(s) in (\"\")"=w2380) -> ("States Out"=w2379:string)  [unwired: 14 in]
      }
      frame "AimingBeam: Set Status" {
        # "Enable Aiming Beam\n(Usage: \"AimingBeam: Set >> Enable|Disable\")"
        n1093 = Unbundle By Name(w2387) -> ("AB Cluster.Aiming Beam COM Port"=w2384:refnum<visa-resource-name>)
        n1094 = case shown="\"Enable\"" w2386 {
          tunnel: [w2390 w2394] -> w2385
          frame "Disable", Default {
            n1095 = Concatenate Strings("cof", "\r" ("Carriage Return Constant"), "\n" ("Line Feed Constant")) -> (w2390:string)
          }
          frame "Enable" {
            n1096 = Concatenate Strings("con", "\r" ("Carriage Return Constant"), "\n" ("Line Feed Constant")) -> (w2394:string)
          }
        }
        n1097 = VISA Write(VISA resource name=w2384, write buffer=w2385, error in (no error)=w2382) -> (error out=w2383:errorcluster)  [unwired: 2 out]
        n1098 = call <vilib>:"Add State(s) to Queue__JKI_lib_State_Machine.vi"("State(s) in (\"\")"=w2389) -> ("States Out"=w2388:string)  [unwired: 14 in]
      }
      frame "AimingBeam: GetPWMStatus" {
        # "Get aiming beam PWM status\n()"
        n1099 = Unbundle By Name(w2402) -> ("AB Cluster.Freq"=w2401:i32, "LJ Pinout.AimingBeam PWM"=w2408:string)
        n1100 = Equal To 0?(x=w2401) -> (x = 0?=w2400:bool)
        n1101 = call "LabJack_FGV.vi"("Operation(Read)"=enum16{"Write", "Read"}."Read" ("Operation"), "error in (no error)"=w2404) -> ("error out"=w2406:errorcluster, "Read data"=w2407:i32)  [unwired: 8 in]
        n1102 = case shown="True" w2400 {
          tunnel: w2408 -> [w2421 _]
          tunnel: [w2419 "DIO_STATE"] -> w2405
          frame False {
            n1103 = Concatenate Strings(w2421, "_EF_ENABLE" ("string")) -> (w2419:string)
          }
          frame True {
          }
        }
        n1104 = call "LJM_eReadName.vi"("Handle In"=w2407, "Name"=w2405, "error in"=w2406) -> ("Value"=w2399:dbl, "error out"=w2403:errorcluster)  [unwired: 10 in, 1 out]
        n1105 = case shown="True" w2400 {
          tunnel: w2399 -> [w2414 w2418]
          tunnel: [w2413 w2415] -> w2398
          frame False {
            n1106 = Greater Than 0?(x=w2414) -> (x > 0?=w2413:bool)
          }
          frame True {
            n1107 = Number To Boolean Array(number=w2418) -> (Boolean array=w2417:bool[])
            n1108 = Index Array(array=w2417, index=3) -> (element=w2415:bool)
          }
        }
        n1109 = case shown="False" w2398 {
          frame False {
            # "PWM is off\nset color to dark green"
            n1110 = local write "Aiming beam toggle"(FALSE ("Aimging beam")) -> ()
          }
          frame True {
            # "PWM is on\nset color to light green"
            n1111 = local write "Aiming beam toggle"(TRUE ("Aimging beam")) -> ()
          }
        }
        n1112 = call <vilib>:"Add State(s) to Queue__JKI_lib_State_Machine.vi"("State(s) in (\"\")"=w2412) -> ("States Out"=w2411:string)  [unwired: 14 in]
      }
      frame "---------- 355 Laser ----------" {
        # "Template Separator\n(You can make a copy of, or modify, this frame)"
        n1113 = call <vilib>:"Add State(s) to Queue__JKI_lib_State_Machine.vi"("State(s) in (\"\")"=w2429) -> ("States Out"=w2428:string)  [unwired: 14 in]
      }
      frame "355 Laser: Check Dewelling" {
        # "if time laser start time is less than 7.5s before, wait 250ms then check again."
        # "Template Separator\n(You can make a copy of, or modify, this frame)"
        n1114 = Unbundle By Name(w2437) -> ("Laser start tic"=w2434:u32)
        n1115 = Tick Count (ms)() -> (millisecond timer value=w2435:u32)
        n1116 = Subtract(x=w2435, y=w2434) -> (x-y=w2433:u32)
        n1117 = Greater?(x=w2433, y=u32 5000) -> (0:w2431:bool)
        n1118 = case shown="False" w2431 {
          tunnel: ["355 Laser: Check Dewelling" ""] -> w2430
          frame False {
            n1119 = Wait (ms)(milliseconds to wait=u32 250) -> ()  [unwired: 1 out]
          }
          frame True {
          }
        }
        n1120 = call <vilib>:"Add State(s) to Queue__JKI_lib_State_Machine.vi"("State(s) in Front (\"\")"=w2430, "State(s) in (\"\")"=w2440) -> ("States Out"=w2439:string)  [unwired: 13 in]
      }
      frame "355 Laser: Laser enable" {
        # "Laser enable/disable\n(Usage: \"LabJack: Laser enable/disable >> 1|0\")"
        n1121 = Unbundle By Name(w2447) -> ("LJ Pinout.Laser Start/Stop"=w2451:string, "System Status.355 Laser"=w2445:bool)
        n1122 = case shown="False" w2445 {
          tunnel: w2444 -> [w2466 w2467]
          tunnel: w2451 -> [w2460 _]
          tunnel: [w2455 w2467] -> w2449
          tunnel: [w2454 u32 0 ("millisecond timer value")] -> w2446
          frame False {
            n1123 = call "LabJack_FGV.vi"("Operation(Read)"=enum16{"Write", "Read"}."Read" ("Operation")) -> ("Read data"=w2462:i32)  [unwired: 9 in, 1 out]
            n1124 = call "LJM_eWriteName.vi"("Handle In"=w2462, "Name"=w2460, "Value"=1.0, "error in"=w2466) -> ("Handle Out"=w2461:i32, "error out"=w2459:errorcluster)  [unwired: 10 in]
            n1125 = call <userlib>:"Wait (ms)__ogtk.vi"("error in (no error)"=w2459, "milliseconds to wait"=u32 250) -> ("error out"=w2458:errorcluster)  [unwired: 8 in, 1 out]
            n1126 = call "LJM_eWriteName.vi"("Handle In"=w2461, "Name"=w2460, "Value"=0.0, "error in"=w2458) -> ("error out"=w2456:errorcluster)  [unwired: 10 in, 1 out]
            n1127 = call <userlib>:"Tick Count (ms)__ogtk.vi"("error in (no error)"=w2456) -> ("error out"=w2455:errorcluster, "millisecond timer value"=w2454:u32)  [unwired: 9 in]
          }
          frame True {
          }
        }
        n1128 = Bundle By Name(cluster=w2447, "Laser start tic"=w2446) -> (w2448:T23)
        n1129 = call <vilib>:"Add State(s) to Queue__JKI_lib_State_Machine.vi"("State(s) in (\"\")"=w2453) -> ("States Out"=w2452:string)  [unwired: 14 in]
      }
      frame "355 Laser: Laser disable" {
        # "Laser enable/disable\n(Usage: \"LabJack: Laser enable/disable >> 1|0\")"
        n1130 = Unbundle By Name(w2471) -> ("LJ Pinout.Laser Start/Stop"=w2475:string, "System Status.355 Laser"=w2469:bool)
        n1131 = case shown="True" w2469 {
          tunnel: w2476 -> [w2479 w2493]
          tunnel: w2475 -> [_ w2487]
          tunnel: [w2479 w2482] -> w2473
          tunnel: [u32 0 ("millisecond timer value") w2481] -> w2470
          frame False {
          }
          frame True {
            n1132 = call "LabJack_FGV.vi"("Operation(Read)"=enum16{"Write", "Read"}."Read" ("Operation")) -> ("Read data"=w2489:i32)  [unwired: 9 in, 1 out]
            n1133 = call "LJM_eWriteName.vi"("Handle In"=w2489, "Name"=w2487, "Value"=1.0, "error in"=w2493) -> ("Handle Out"=w2488:i32, "error out"=w2486:errorcluster)  [unwired: 10 in]
            n1134 = call <userlib>:"Wait (ms)__ogtk.vi"("error in (no error)"=w2486, "milliseconds to wait"=u32 250) -> ("error out"=w2485:errorcluster)  [unwired: 8 in, 1 out]
            n1135 = call "LJM_eWriteName.vi"("Handle In"=w2488, "Name"=w2487, "Value"=0.0, "error in"=w2485) -> ("error out"=w2483:errorcluster)  [unwired: 10 in, 1 out]
            n1136 = call <userlib>:"Tick Count (ms)__ogtk.vi"("error in (no error)"=w2483) -> ("error out"=w2482:errorcluster, "millisecond timer value"=w2481:u32)  [unwired: 9 in]
          }
        }
        n1137 = Bundle By Name(cluster=w2471, "Laser start tic"=w2470) -> (w2472:T23)
        n1138 = call <vilib>:"Add State(s) to Queue__JKI_lib_State_Machine.vi"("State(s) in (\"\")"=w2478) -> ("States Out"=w2477:string)  [unwired: 14 in]
      }
      frame "355 Laser: Dewelling" {
        # "Wait some time (ms)\n(355 Laser: Dewelling >> #)"
        n1139 = Fract/Exp String To Number(string=w2497, default (0 dbl)=0) -> (number=w2495:i32)  [unwired: 2 in, 1 out]
        n1140 = Wait (ms)(milliseconds to wait=w2495) -> ()  [unwired: 1 out]
        n1141 = call <vilib>:"Add State(s) to Queue__JKI_lib_State_Machine.vi"("State(s) in (\"\")"=w2501) -> ("States Out"=w2500:string)  [unwired: 14 in]
      }
      frame "355 Laser: Close" {
        # "Template Separator\n(You can make a copy of, or modify, this frame)"
        n1142 = call <vilib>:"Add State(s) to Queue__JKI_lib_State_Machine.vi"("State(s) in Front (\"\")"="355 Laser: CheckControllerStatus\n355 Laser: Laser disable\n355 Laser: Dewelling >>1000", "State(s) in (\"\")"=w2507) -> ("States Out"=w2506:string)  [unwired: 13 in]
      }
      frame "355 Laser: CheckControllerStatus" {
        # "if average < 2, laser no power\nif average 2 < average < 9.3, laser on\nif 9.3<average<10, interlock open, blink indicator\nif average > 10, laser off\n[Covers: REQ30]"
        # "take 10 measuremt and look at average"
        # "Check 355 laser controller status\nBy probing Emisison Lamp negative terminal voltage"
        n1143 = Unbundle By Name(w2516) -> ("LJ Pinout.Laser Ready"=w2519:string)
        n1144 = call "LabJack_FGV.vi"("Operation(Read)"=enum16{"Write", "Read"}."Read" ("Operation")) -> ("Read data"=w2520:i32)  [unwired: 9 in, 1 out]
        n1145 = for {
          N: 20 -> [_]
          tunnel: w2520 -> [w2531]
          tunnel: w2519 -> [w2530]
          shift-right: [w2529] -> w2512
          shift-left: w2518 -> [w2528]
          tunnel: [w2526] -> w2511 mode=indexing
          n1146 = call "LJM_eReadName.vi"("Handle In"=w2531, "Name"=w2530, "error in"=w2528) -> ("Value"=w2526:dbl, "error out"=w2529:errorcluster)  [unwired: 10 in, 1 out]
          n1147 = Wait (ms)(milliseconds to wait=u32 25) -> ()  [unwired: 1 out]
        }
        n1148 = call "checkLaserStatus.vi"("error in (no error)"=w2512, "Laser LED voltage"=w2511) -> ("error out"=w2513:errorcluster, "Interlock open?"=w2508:bool, "Laser on?"=w2510:bool, "Mean voltage"=→"laser EM lamp V":dbl)  [unwired: 6 in]
        n1149 = Bundle By Name(cluster=w2516, "System Status.355 Laser"=w2510) -> (w2517:T23)
        n1150 = case shown="True" w2508 {
          frame False {
            n1151 = property on="355 Laser" class="Bool (strict)"("Blinking"=FALSE) -> ()  [unwired: 2 in, 2 out]
          }
          frame True {
            n1152 = property on="355 Laser" class="Bool (strict)"("Blinking"=TRUE) -> ()  [unwired: 2 in, 2 out]
          }
        }
        n1153 = call <vilib>:"Add State(s) to Queue__JKI_lib_State_Machine.vi"("State(s) in (\"\")"=w2523) -> ("States Out"=w2522:string)  [unwired: 14 in]
      }
      frame "355 Laser: CheckPWMStatus" {
        # "Check 355 laser PWM status\n(Read LJ DIO#EF_ENABLE register to determine PWM status)"
        n1154 = Unbundle By Name(w2541) -> ("LJ Pinout.355 PWM"=w2540:string)
        n1155 = call "LabJack_FGV.vi"("Operation(Read)"=enum16{"Write", "Read"}."Read" ("Operation"), "error in (no error)"=w2534) -> ("error out"=w2537:errorcluster, "Read data"=w2538:i32)  [unwired: 8 in]
        n1156 = Concatenate Strings(w2540, "_EF_ENABLE" ("string")) -> (w2536:string)
        n1157 = call "LJM_eReadName.vi"("Handle In"=w2538, "Name"=w2536, "error in"=w2537) -> ("Value"=w2533:dbl, "error out"=w2535:errorcluster)  [unwired: 10 in, 1 out]
        n1158 = Greater Than 0?(x=w2533) -> (x > 0?=w2532:bool)
        n1159 = case shown="False" w2532 {
          frame False {
            # "PWM is off\nset color to gray"
            n1160 = local write "355nm Laser toggle"(FALSE ("355nm Laser")) -> ()
          }
          frame True {
            # "PWM is on\nset color to light green"
            n1161 = local write "355nm Laser toggle"(TRUE ("355nm Laser")) -> ()
          }
        }
        n1162 = call <vilib>:"Add State(s) to Queue__JKI_lib_State_Machine.vi"("State(s) in (\"\")"=w2545) -> ("States Out"=w2544:string)  [unwired: 14 in]
      }
      frame "355 Laser: Start" {
        # "Template Separator\n(You can make a copy of, or modify, this frame)"
        n1163 = call <vilib>:"Add State(s) to Queue__JKI_lib_State_Machine.vi"("State(s) in Front (\"\")"="LabJack: 355_PWM_Start", "State(s) in (\"\")"=w2553) -> ("States Out"=w2552:string)  [unwired: 13 in]
      }
      frame "355 Laser: Stop" {
        # "Template Separator\n(You can make a copy of, or modify, this frame)"
        n1164 = call <vilib>:"Add State(s) to Queue__JKI_lib_State_Machine.vi"("State(s) in Front (\"\")"="LabJack: 355_PWM_Stop", "State(s) in (\"\")"=w2559) -> ("States Out"=w2558:string)  [unwired: 13 in]
      }
      frame "---------- Utility ----------" {
        # "Template Separator\n(You can make a copy of, or modify, this frame)"
        n1165 = call <vilib>:"Add State(s) to Queue__JKI_lib_State_Machine.vi"("State(s) in (\"\")"=w2564) -> ("States Out"=w2563:string)  [unwired: 14 in]
      }
      frame "Utility: SetDataClass" {
        # "Set Data Class in Queues\n(Set data class to either Data, Bg or Cali)"
        n1166 = case shown="\"Cali\"" w2566 {
          tunnel: [enum16{"Data", "BG", "Cali"}."Data" ("Data Class") enum16{"Data", "BG", "Cali"}."BG" ("Data Class") enum16{"Data", "BG", "Cali"}."Cali" ("Data Class")] -> w2565
          frame "Data", Default {
          }
          frame "Bg" {
          }
          frame "Cali" {
          }
        }
        n1167 = local write "Data Class"(w2565) -> ()
        n1168 = call <vilib>:"Add State(s) to Queue__JKI_lib_State_Machine.vi"("State(s) in (\"\")"=w2571) -> ("States Out"=w2570:string)  [unwired: 14 in]
      }
      frame "Utility: AquiTimerReset" {
        # "Set Aquisition Timer\n(You can make a copy of, or modify, this frame)"
        n1169 = Tick Count (ms)() -> (millisecond timer value=w2577:u32)
        n1170 = Bundle By Name(cluster=w2575, "Aquisition Timer"=w2577) -> (w2576:T23)
        n1171 = call <vilib>:"Add State(s) to Queue__JKI_lib_State_Machine.vi"("State(s) in (\"\")"=w2581) -> ("States Out"=w2580:string)  [unwired: 14 in]
      }
      frame "Utility: AquiTimerCheck" {
        # "5min to ms"
        # "Set Aquisition Timer\n([Covers: REQ35])"
        n1172 = Unbundle By Name(w2589) -> ("Aquisition Timer"=w2587:u32)
        n1173 = Tick Count (ms)() -> (millisecond timer value=w2588:u32)
        n1174 = Subtract(x=w2588, y=w2587) -> (x-y=w2586:u32)
        n1175 = Multiply(x=1000, y=300) -> (x*y=w2583:i32)
        n1176 = Greater Or Equal?(x=w2586, y=w2583) -> (x >= y?=w2582:bool)
        n1177 = case shown="True" w2582 {
          frame False {
            # "do nothing"
          }
          frame True {
            # "if timed out, stop aquisition"
            n1178 = property on="StopButton" class="Bool (strict)"("Val(Sgnl)"=TRUE ("Value (Signaling)")) -> ()  [unwired: 2 in, 2 out]
          }
        }
        n1179 = call <vilib>:"Add State(s) to Queue__JKI_lib_State_Machine.vi"("State(s) in (\"\")"=w2593) -> ("States Out"=w2592:string)  [unwired: 14 in]
      }
      frame "Utility: StartBeep" {
        # "Beep\n([Covers: REQ18])"
        n1180 = call <vilib>:"Beep.vi"("use system alert? (T)"=FALSE, "duration (msec)"=u32 1000, "frequency (Hz)"=u32 2000) -> ()  [unwired: 9 in]
        n1181 = call <vilib>:"Add State(s) to Queue__JKI_lib_State_Machine.vi"("State(s) in (\"\")"=w2602) -> ("States Out"=w2601:string)  [unwired: 14 in]
      }
      frame "Utility: EndBeep" {
        # "Beep\n([Covers: REQ18])"
        n1182 = flat-sequence {
          frame #0 {
            n1183 = call <vilib>:"Beep.vi"("use system alert? (T)"=FALSE, "duration (msec)"=u32 500, "frequency (Hz)"=u32 2000) -> ()  [unwired: 9 in]
          }
          frame #1 {
            n1184 = call <vilib>:"Beep.vi"("use system alert? (T)"=FALSE, "duration (msec)"=u32 500, "frequency (Hz)"=u32 2000) -> ()  [unwired: 9 in]
          }
        }
        n1185 = call <vilib>:"Add State(s) to Queue__JKI_lib_State_Machine.vi"("State(s) in (\"\")"=w2607) -> ("States Out"=w2606:string)  [unwired: 14 in]
      }
      frame "Utility: RestoreDeConChan" {
        # "Template Separator\n(You can make a copy of, or modify, this frame)"
        n1186 = global read "GlobalVariables.vi" "DeconChan Temp"() -> (w2614:T9)
        n1187 = local write "Radio Buttons"(w2614) -> ()
        n1188 = call <vilib>:"Add State(s) to Queue__JKI_lib_State_Machine.vi"("State(s) in (\"\")"=w2619) -> ("States Out"=w2618:string)  [unwired: 14 in]
      }
      frame "Utility: SaveDeconChan" {
        # "Save Decon Channel to global temp\n(You can make a copy of, or modify, this frame)"
        n1189 = flat-sequence {
          frame #0 {
            n1190 = local read "Radio Buttons"() -> (w2625:T9)
            n1191 = global write "GlobalVariables.vi" "DeconChan Temp"(w2625) -> ()
          }
          frame #1 {
            n1192 = local write "Radio Buttons"(T9."No Selection" ("Radio Buttons")) -> ()
          }
        }
        n1193 = flat-sequence {
          frame #0 {
          }
          frame #1 {
            (unwired) enum32{"No Selection", "Ch1", "Ch2", "Ch3"}."No Selection" ("Radio Buttons")
          }
        }
        n1194 = call <vilib>:"Add State(s) to Queue__JKI_lib_State_Machine.vi"("State(s) in (\"\")"=w2624) -> ("States Out"=w2623:string)  [unwired: 14 in]
      }
      frame "Utility: Dewelling" {
        # "Main loop dewell\n(Dewelling >> #)"
        n1195 = Fract/Exp String To Number(string=w2630, default (0 dbl)=0) -> (number=w2628:i32)  [unwired: 2 in, 1 out]
        n1196 = Wait (ms)(milliseconds to wait=w2628) -> ()  [unwired: 1 out]
        n1197 = call <vilib>:"Add State(s) to Queue__JKI_lib_State_Machine.vi"("State(s) in (\"\")"=w2634) -> ("States Out"=w2633:string)  [unwired: 14 in]
      }
      frame "Utility: SetAllChanManualGain" {
        w2635 = FALSE ("Value (Signaling)")
        # "Set all channel to manual gain\n(You can make a copy of, or modify, this frame)"
        n1198 = property on="Auto gain ch1" class="Bool (strict)"("Val(Sgnl)"=w2635) -> ()  [unwired: 2 in, 2 out]
        n1199 = property on="Auto gain ch2" class="Bool (strict)"("Val(Sgnl)"=w2635) -> ()  [unwired: 2 in, 2 out]
        n1200 = property on="Auto gain ch3" class="Bool (strict)"("Val(Sgnl)"=w2635) -> ()  [unwired: 2 in, 2 out]
        n1201 = property on="Auto gain ch4" class="Bool (strict)"("Val(Sgnl)"=w2635) -> ()  [unwired: 2 in, 2 out]
        n1202 = call <vilib>:"Add State(s) to Queue__JKI_lib_State_Machine.vi"("State(s) in (\"\")"=w2640) -> ("States Out"=w2639:string)  [unwired: 14 in]
      }
      frame "Utility: SetAllChanAutoGain" {
        w2641 = TRUE ("Value (Signaling)")
        # "Set all channels to auto gain\n(You can make a copy of, or modify, this frame)"
        n1203 = property on="Auto gain ch1" class="Bool (strict)"("Val(Sgnl)"=w2641) -> ()  [unwired: 2 in, 2 out]
        n1204 = property on="Auto gain ch2" class="Bool (strict)"("Val(Sgnl)"=w2641) -> ()  [unwired: 2 in, 2 out]
        n1205 = property on="Auto gain ch3" class="Bool (strict)"("Val(Sgnl)"=w2641) -> ()  [unwired: 2 in, 2 out]
        n1206 = property on="Auto gain ch4" class="Bool (strict)"("Val(Sgnl)"=w2641) -> ()  [unwired: 2 in, 2 out]
        n1207 = call <vilib>:"Add State(s) to Queue__JKI_lib_State_Machine.vi"("State(s) in (\"\")"=w2646) -> ("States Out"=w2645:string)  [unwired: 14 in]
      }
      frame "---------- SysLog ----------" {
        # "Template Separator\n(You can make a copy of, or modify, this frame)"
        n1208 = call <vilib>:"Add State(s) to Queue__JKI_lib_State_Machine.vi"("State(s) in (\"\")"=w2651) -> ("States Out"=w2650:string)  [unwired: 14 in]
      }
      frame "SysLog: OpenLogFile" {
        # "Template Separator\n(You can make a copy of, or modify, this frame)"
        n1209 = call <vilib>:"Add State(s) to Queue__JKI_lib_State_Machine.vi"("State(s) in (\"\")"=w2656) -> ("States Out"=w2655:string)  [unwired: 14 in]
      }
      frame "---------- Graph ----------" {
        # "Template Separator\n(You can make a copy of, or modify, this frame)"
        n1210 = call <vilib>:"Add State(s) to Queue__JKI_lib_State_Machine.vi"("State(s) in (\"\")"=w2661) -> ("States Out"=w2660:string)  [unwired: 14 in]
      }
      frame "Graph: SetXMultiplier" {
        # "Set X multiplier of WF graphs\n(You can make a copy of, or modify, this frame)"
        n1211 = call "Digitizer1_FGV.vi"() -> ("error out"=w2665:errorcluster, "Read data"=w2666:refnum<k15>)  [unwired: 10 in]
        n1212 = property class="niScope"(reference=w2666, error in=w2665) -> ("Min Sample Rate"=w2664:dbl)  [unwired: 2 out]
        n1213 = Divide(x=1.0, y=w2664) -> (x/y=w2662:dbl)
        n1214 = property on="Channel 1" class="WFGraph (strict)"("XScale.Multiplier"=w2662) -> ()  [unwired: 2 in, 2 out]
        n1215 = property on="Channel 2" class="WFGraph (strict)"("XScale.Multiplier"=w2662) -> ()  [unwired: 2 in, 2 out]
        n1216 = property on="Channel 3" class="WFGraph (strict)"("XScale.Multiplier"=w2662) -> ()  [unwired: 2 in, 2 out]
        n1217 = call <vilib>:"Add State(s) to Queue__JKI_lib_State_Machine.vi"("State(s) in (\"\")"=w2671) -> ("States Out"=w2670:string)  [unwired: 14 in]
      }
      frame "Graph: AddCursors" {
        # "Add BG and DC cursor to all graphs\n(You can make a copy of, or modify, this frame)"
        n1218 = property on="Channel 1" class="WFGraph (strict)"() -> ("XScale.Multiplier"=w2678:dbl)  [unwired: 2 in, 2 out]
        n1219 = global read "GlobalVariables.vi" "DC Idx1"() -> (w2677:i32)
        n1220 = global read "GlobalVariables.vi" "DC Idx2"() -> (w2676:i32)
        n1221 = global read "GlobalVariables.vi" "BG Idx1"() -> (w2675:i32)
        n1222 = global read "GlobalVariables.vi" "BG Idx2"() -> (w2674:i32)
        n1223 = property on="Channel 2" class="WFGraph (strict)"() -> ("CrsrList"=w2686:T24)  [unwired: 2 in, 2 out]
        n1224 = property on="Channel 3" class="WFGraph (strict)"() -> ("CrsrList"=w2685:T24)  [unwired: 2 in, 2 out]
        n1225 = property on="Channel 1" class="WFGraph (strict)"(error in=w2680) -> ("CrsrList"=w2689:T24)  [unwired: 1 in, 2 out]
        n1226 = Build Array(w2677, w2676, w2675, w2674) -> (w2673:i32[])
        n1227 = Multiply(x=w2673, y=w2678) -> (x*y=w2672:dbl[])
        n1228 = for {
          tunnel: w2689 -> [w2701] mode=indexing
          tunnel: w2672 -> [w2697] mode=indexing
          tunnel: [w2700] -> w2688 mode=indexing
          tunnel: u32[] [6618880, 6618880, 16711680, 16711680] -> [w2696] mode=indexing
          tunnel: w2686 -> [w2699] mode=indexing
          tunnel: w2685 -> [w2698] mode=indexing
          tunnel: [w2695] -> w2684 mode=indexing
          tunnel: [w2694] -> w2683 mode=indexing
          n1229 = Bundle By Name(cluster=w2701, "Position.X"=w2697, "Color"=w2696) -> (w2700:T25)
          n1230 = Bundle By Name(cluster=w2699, "Position.X"=w2697, "Color"=w2696) -> (w2695:T25)
          n1231 = Bundle By Name(cluster=w2698, "Position.X"=w2697, "Color"=w2696) -> (w2694:T25)
        }
        n1232 = control-ref of="Channel 1"() -> (w2682:refnum<vi>)
        n1233 = property on="Channel 1" class="WFGraph (strict)"("CrsrList"=w2688) -> (error out=w2679:errorcluster)  [unwired: 2 in, 1 out]
        n1234 = property on="Channel 2" class="WFGraph (strict)"("CrsrList"=w2684) -> ()  [unwired: 2 in, 2 out]
        n1235 = property on="Channel 3" class="WFGraph (strict)"("CrsrList"=w2683) -> ()  [unwired: 2 in, 2 out]
        n1236 = call "UpdateCurserIdx(SubVI).vi"("error in (no error)"=w2679, "WaveformGraph in"=w2682) -> ("error out"=w2681:errorcluster)  [unwired: 9 in]
        n1237 = call <vilib>:"Add State(s) to Queue__JKI_lib_State_Machine.vi"("State(s) in (\"\")"=w2693) -> ("States Out"=w2692:string)  [unwired: 14 in]
      }
      frame "Graph: SaveCursorLoc" {
        # "Save cursor location to ini file\n(Save cursor location to system setting ini file)"
        n1238 = global read "GlobalVariables.vi" "DC Idx1"() -> (w2708:i32)
        n1239 = global read "GlobalVariables.vi" "DC Idx2"() -> (w2707:i32)
        n1240 = global read "GlobalVariables.vi" "BG Idx1"() -> (w2706:i32)
        n1241 = global read "GlobalVariables.vi" "BG Idx2"() -> (w2705:i32)
        n1242 = Bundle("DC Idx1"=w2708, "DC Idx2"=w2707, "BG Idx1"=w2706, "BG Idx2"=w2705) -> (w2704:T46)  [unwired: 1 in]
        n1243 = call "writeCursorConfigMain.vi"("error in (no error)"=w2702, "Cursor Locations"=w2704) -> ("error out"=w2703:errorcluster)  [unwired: 9 in]
        n1244 = call <vilib>:"Add State(s) to Queue__JKI_lib_State_Machine.vi"("State(s) in (\"\")"=w2712) -> ("States Out"=w2711:string)  [unwired: 14 in]
      }
      frame "---------- APD ----------" {
        # "Template Separator\n(You can make a copy of, or modify, this frame)"
        n1245 = call <vilib>:"Add State(s) to Queue__JKI_lib_State_Machine.vi"("State(s) in (\"\")"=w2717) -> ("States Out"=w2716:string)  [unwired: 14 in]
      }
      frame "APD: Initialize" {
        w2724 = enum16{"Read", "Write"}."Write" ("Operation (Read)")
        w2723 = refnum<class "APDClass.lvclass"> refnum  # APDClass.lvclass
        # "Initialize APD FGV\n(Initialized APD FGV for holding data)"
        n1246 = call "APD1FGV.vi"("Error In"=w2718, "Operation (Read)"=w2724, "APDClass in"=w2723) -> ("Error Out"=w2722:errorcluster)  [unwired: 7 in, 1 out]
        n1247 = call "APD2FGV.vi"("Error In"=w2718, "Operation (Read)"=w2724, "APDClass in"=w2723) -> ("Error Out"=w2721:errorcluster)  [unwired: 7 in, 1 out]
        n1248 = call "APD3FGV.vi"("Error In"=w2718, "Operation (Read)"=w2724, "APDClass in"=w2723) -> ("Error Out"=w2720:errorcluster)  [unwired: 7 in, 1 out]
        n1249 = Merge Errors(w2722, w2721, w2720) -> (w2719:errorcluster)
        n1250 = call <vilib>:"Add State(s) to Queue__JKI_lib_State_Machine.vi"("State(s) in (\"\")"=w2728) -> ("States Out"=w2727:string)  [unwired: 14 in]
      }
      frame "APD: LoadFromSerial" {
        w2730 = enum16{"Read", "Write"}."Write" ("Operation (Read)")
        # "Load APD data from tdms file\n(load and update FGV)"
        n1251 = call "readAPDSerial.vi"("Error In"=w2737) -> ("Error Out"=w2733:errorcluster, "output cluster"=w2736:T26)  [unwired: 9 in]
        n1252 = Unbundle By Name(w2736) -> ("Ch1APDSerial#"=w2749:string, "Ch2APDSerial#"=w2735:string, "Ch3APDSerial#"=w2748:string, "Ch4APDSerial#"=w2734:string)
        n1253 = call "CreatFromSerialNumNoRaw.vi"("error in (no error)"=w2733, "APD Serial #"=w2749) -> ("error out"=w2746:errorcluster, "APDClass out"=w2747:refnum<class "APDClass.lvclass">)  [unwired: 8 in]
        n1254 = call "CreatFromSerialNumNoRaw.vi"("error in (no error)"=w2733, "APD Serial #"=w2735) -> ("error out"=w2744:errorcluster, "APDClass out"=w2745:refnum<class "APDClass.lvclass">)  [unwired: 8 in]
        n1255 = call "CreatFromSerialNumNoRaw.vi"("error in (no error)"=w2733, "APD Serial #"=w2748) -> ("error out"=w2742:errorcluster, "APDClass out"=w2743:refnum<class "APDClass.lvclass">)  [unwired: 8 in]
        n1256 = call "CreatFromSerialNumNoRaw.vi"("error in (no error)"=w2733, "APD Serial #"=w2734) -> ("error out"=w2731:errorcluster, "APDClass out"=w2732:refnum<class "APDClass.lvclass">)  [unwired: 8 in]
        n1257 = call "APD1FGV.vi"("Error In"=w2746, "Operation (Read)"=w2730, "APDClass in"=w2747) -> ("Error Out"=w2741:errorcluster)  [unwired: 7 in, 1 out]
        n1258 = call "APD2FGV.vi"("Error In"=w2744, "Operation (Read)"=w2730, "APDClass in"=w2745) -> ("Error Out"=w2739:errorcluster)  [unwired: 7 in, 1 out]
        n1259 = call "APD3FGV.vi"("Error In"=w2742, "Operation (Read)"=w2730, "APDClass in"=w2743) -> ("Error Out"=w2740:errorcluster)  [unwired: 7 in, 1 out]
        n1260 = call "APD4FGV.vi"("Error In"=w2731, "Operation (Read)"=w2730, "APDClass in"=w2732) -> ("Error Out"=w2729:errorcluster)  [unwired: 7 in, 1 out]
        n1261 = Merge Errors(w2741, w2739, w2740, w2729) -> (w2738:errorcluster)
        n1262 = call <vilib>:"Add State(s) to Queue__JKI_lib_State_Machine.vi"("State(s) in (\"\")"=w2753) -> ("States Out"=w2752:string)  [unwired: 14 in]
      }
      frame "APD: UpdateCtrlVLimit" {
        w2759 = enum16{"Read", "Write"}."Read" ("Operation (Read)")
        # "Set V limit\n(You can make a copy of, or modify, this frame)"
        n1263 = call "APD1FGV.vi"("Error In"=w2760, "Operation (Read)"=w2759) -> ("Error Out"=w2775:errorcluster, "APDClass out"=w2776:refnum<class "APDClass.lvclass">)  [unwired: 8 in]
        n1264 = call "APD2FGV.vi"("Error In"=w2760, "Operation (Read)"=w2759) -> ("Error Out"=w2773:errorcluster, "APDClass out"=w2774:refnum<class "APDClass.lvclass">)  [unwired: 8 in]
        n1265 = call "APD3FGV.vi"("Error In"=w2760, "Operation (Read)"=w2759) -> ("Error Out"=w2771:errorcluster, "APDClass out"=w2772:refnum<class "APDClass.lvclass">)  [unwired: 8 in]
        n1266 = call "APD4FGV.vi"("Error In"=w2760, "Operation (Read)"=w2759) -> ("Error Out"=w2757:errorcluster, "APDClass out"=w2758:refnum<class "APDClass.lvclass">)  [unwired: 8 in]
        n1267 = call-dynamic "ReadMaxCtrlV.vi"("error in (no error)"=w2775, "APDClass in"=w2776) -> ("error out"=w2766:errorcluster, "Numeric"=w2769:dbl)  [unwired: 7 in, 1 out]
        n1268 = call-dynamic "ReadMaxCtrlV.vi"("error in (no error)"=w2773, "APDClass in"=w2774) -> ("error out"=w2764:errorcluster, "Numeric"=w2768:dbl)  [unwired: 7 in, 1 out]
        n1269 = call-dynamic "ReadMaxCtrlV.vi"("error in (no error)"=w2771, "APDClass in"=w2772) -> ("error out"=w2762:errorcluster, "Numeric"=w2767:dbl)  [unwired: 7 in, 1 out]
        n1270 = call-dynamic "ReadMaxCtrlV.vi"("error in (no error)"=w2757, "APDClass in"=w2758) -> ("error out"=w2755:errorcluster, "Numeric"=w2756:dbl)  [unwired: 7 in, 1 out]
        n1271 = property on="V 1" class="DigNum (strict)"(error in=w2766, "Maximum"=w2769) -> (error out=w2765:errorcluster)  [unwired: 1 in, 1 out]
        n1272 = property on="V 2" class="DigNum (strict)"(error in=w2764, "Maximum"=w2768) -> (error out=w2763:errorcluster)  [unwired: 1 in, 1 out]
        n1273 = property on="V 4" class="DigNum (strict)"(error in=w2755, "Maximum"=w2756) -> (error out=w2754:errorcluster)  [unwired: 1 in, 1 out]
        n1274 = property on="V 3" class="DigNum (strict)"(error in=w2762, "Maximum"=w2767) -> (error out=w2761:errorcluster)  [unwired: 1 in, 1 out]
        n1275 = Merge Errors(w2765, w2763, w2761, w2754) -> (w2770:errorcluster)
        n1276 = call <vilib>:"Add State(s) to Queue__JKI_lib_State_Machine.vi"("State(s) in (\"\")"=w2780) -> ("States Out"=w2779:string)  [unwired: 14 in]
      }
      frame "APD: GetGainLimits" {
        w2785 = enum16{"Read", "Write"}."Read" ("Operation (Read)")
        # "Template Separator\n(You can make a copy of, or modify, this frame)"
        n1277 = call "APD1FGV.vi"("Error In"=w2786, "Operation (Read)"=w2785) -> ("Error Out"=w2791:errorcluster, "APDClass out"=w2792:refnum<class "APDClass.lvclass">)  [unwired: 8 in]
        n1278 = call "APD2FGV.vi"("Error In"=w2786, "Operation (Read)"=w2785) -> ("Error Out"=w2798:errorcluster, "APDClass out"=w2799:refnum<class "APDClass.lvclass">)  [unwired: 8 in]
        n1279 = call "APD3FGV.vi"("Error In"=w2786, "Operation (Read)"=w2785) -> ("Error Out"=w2796:errorcluster, "APDClass out"=w2797:refnum<class "APDClass.lvclass">)  [unwired: 8 in]
        n1280 = call "APD4FGV.vi"("Error In"=w2786, "Operation (Read)"=w2785) -> ("Error Out"=w2783:errorcluster, "APDClass out"=w2784:refnum<class "APDClass.lvclass">)  [unwired: 8 in]
        n1281 = call-dynamic "Read Gain Limits(Log).vi"("error in (no error)"=w2791, "APDClass in"=w2792) -> ("error out"=w2790:errorcluster, "GainLimits(Log)"=w2787:cluster{"GainMax":dbl, "GainMin":dbl})  [unwired: 7 in, 1 out]
        n1282 = call-dynamic "Read Gain Limits(Log).vi"("error in (no error)"=w2798, "APDClass in"=w2799) -> ("error out"=w2794:errorcluster, "GainLimits(Log)"=w2789:cluster{"GainMax":dbl, "GainMin":dbl})  [unwired: 7 in, 1 out]
        n1283 = call-dynamic "Read Gain Limits(Log).vi"("error in (no error)"=w2796, "APDClass in"=w2797) -> ("error out"=w2793:errorcluster, "GainLimits(Log)"=w2788:cluster{"GainMax":dbl, "GainMin":dbl})  [unwired: 7 in, 1 out]
        n1284 = call-dynamic "Read Gain Limits(Log).vi"("error in (no error)"=w2783, "APDClass in"=w2784) -> ("error out"=w2781:errorcluster, "GainLimits(Log)"=w2782:cluster{"GainMax":dbl, "GainMin":dbl})  [unwired: 7 in, 1 out]
        n1285 = Merge Errors(w2790, w2794, w2793, w2781) -> (w2795:errorcluster)
        n1286 = global write "GlobalVariables.vi" "Ch1GainLim(Log)"(w2787) -> ()
        n1287 = global write "GlobalVariables.vi" "Ch2GainLim(Log)"(w2789) -> ()
        n1288 = global write "GlobalVariables.vi" "Ch3GainLim(Log)"(w2788) -> ()
        n1289 = global write "GlobalVariables.vi" "Ch4GainLim(Log)"(w2782) -> ()
        n1290 = call <vilib>:"Add State(s) to Queue__JKI_lib_State_Machine.vi"("State(s) in (\"\")"=w2803) -> ("States Out"=w2802:string)  [unwired: 14 in]
      }
      frame "---------- TCP ----------" {
        # "Template Separator\n(You can make a copy of, or modify, this frame)"
        n1291 = call <vilib>:"Add State(s) to Queue__JKI_lib_State_Machine.vi"("State(s) in (\"\")"=w2808) -> ("States Out"=w2807:string)  [unwired: 14 in]
      }
      frame "TCP: InitializeNew" {
        # "if unsuccessful and count <10, increament count \nand try again"
        # "Initialize TCP connection to aimging beam computer\n(You can make a copy of, or modify, this frame)"
        n1292 = TCP Create Listener(10:u16 2100 ("port"), 11:"RTLT" ("service name")) -> (0:w2817:errorcluster, 3:w2809:refnum<k5>)  [unwired: 3 in, 1 out]
        n1293 = while {
          tunnel: w2809 -> [w2837]
          tunnel: w2817 -> [w2836]
          tunnel: [w2827] -> w2815
          tunnel: [w2824] -> w2811
          i -> [w2833]
          stop <- w2824 stop-if-true
          n1294 = TCP Wait On Listener(8:w2836, 9:100 ("timeout ms (wait forever: -1)"), 11:w2837) -> (0:w2834:errorcluster, 4:w2831:refnum<k5>)  [unwired: 1 in, 3 out]
          n1295 = Less Or Equal?(x=50, y=w2833) -> (x <= y?=w2830:bool)
          n1296 = case shown="No Error" w2834 {
            selector: w2834 -> [w2847 w2857]
            tunnel: w2831 -> [w2848 _]
            tunnel: [errorcluster {"status"=TRUE, "code"=0, "source"=""} ("No error") w2858] -> w2826
            tunnel: [w2839 FALSE ("TCP connected?")] -> w2827
            frame No Error {
              # "connection is ready, read data"
              n1297 = TCP Read(connection ID=w2848, bytes to read=512, error in (no error)=w2847, 7:T21."CRLF" ("mode (standard)"), 9:5000 ("timeout ms (25000)")) -> (connection ID out=w2841:refnum<k5>, data out=w2843:string, error out=w2840:errorcluster)
              n1298 = Concatenate Strings("alive" ("string"), "\r\n" ("End of Line Constant")) -> (w2844:string)
              n1299 = Equal?(x=w2844, y=w2843) -> (x = y?=w2842:bool)
              n1300 = case shown="False" w2842 {
                tunnel: w2841 -> [_ w2853]
                tunnel: w2840 -> [_ _]
                tunnel: [FALSE ("TCP connected?") TRUE ("TCP connected?")] -> w2839
                frame False {
                }
                frame True {
                  n1301 = call "TcpIDFGV.vi"("action"=enum16{"write", "read"}."write", "connection ID in"=w2853) -> ()  [unwired: 8 in, 2 out]
                }
              }
            }
            frame Error {
              # "connection not ready, keep waiting"
              n1302 = Unbundle By Name(w2857) -> ("code"=w2859:i32)
              n1303 = case shown="56" w2859 {
                tunnel: w2857 -> [w2860 _]
                tunnel: [w2860 w2861] -> w2858
                frame Default {
                }
                frame 56 {
                  w2861 = errorcluster {"status"=FALSE, "code"=0, "source"=""}  # No error
                }
              }
            }
          }
          n1304 = Select(t=errorcluster {"status"=TRUE, "code"=5001, "source"=""} ("error in (no error)"), s=w2830, f=errorcluster {"status"=FALSE, "code"=0, "source"=""} ("error in (no error)")) -> (s? t:f=w2825:errorcluster)
          n1305 = Merge Errors(w2826, w2825) -> (w2824:errorcluster)
        }
        n1306 = Unbundle By Name(w2811) -> ("code"=w2814:i32)
        n1307 = Bundle By Name(cluster=w2816, "System Status.TCP/IP"=w2815, "listener ID"=w2809) -> (w2821:T23)
        n1308 = global write "GlobalVariables.vi" "TCP connected?"(w2815) -> ()
        n1309 = Equal To 0?(x=w2814) -> (x = 0?=w2813:bool)
        n1310 = Select(t=errorcluster {"status"=FALSE, "code"=0, "source"=""} ("error in (no error)"), s=w2813, f=w2811) -> (s? t:f=w2810:errorcluster)
        n1311 = call <vilib>:"Add State(s) to Queue__JKI_lib_State_Machine.vi"("State(s) in (\"\")"=w2823) -> ("States Out"=w2822:string)  [unwired: 14 in]
      }
      frame "TCP: checkSource" {
        # "Check visualization PC video source\n(send !video_source message, listen for response, then parse it to binary mask)"
        n1312 = Unbundle By Name(w2868) -> ("System Status.TCP/IP"=w2871:bool)
        n1313 = case shown="True" w2871 {
          tunnel: w2870 -> [w2876 w2899]
          tunnel: [w2876 w2883] -> w2869
          tunnel: [w2875 w2888] -> w2866
          tunnel: [w2875 w2886] -> w2865
          tunnel: [w2875 w2887] -> w2864
          tunnel: [w2875 w2885] -> w2863
          tunnel: [w2875 w2877] -> w2862
          frame False {
            w2875 = FALSE
          }
          frame True {
            n1314 = call "TcpIDFGV.vi"("Error In"=w2899, "action"=enum16{"write", "read"}."read") -> ("Error Out"=w2896:errorcluster, "connection ID out"=w2898:refnum<k5>)  [unwired: 8 in]
            n1315 = call "TCP_WriteRead.vi"("error in (no error)"=w2896, "data in"="!video_source", "connectin ID in"=w2898) -> ("error out"=w2893:errorcluster, "data out"=w2895:string)  [unwired: 4 in, 1 out]
            n1316 = Scan From String(format string="!video_source:%d", input string=w2895, error in=w2893) -> (error out=w2884:errorcluster, output 1=w2882:i32)  [unwired: 2 in, 2 out]
            n1317 = case shown="5..7, 9..11, 13..15" w2882 {
              tunnel: w2884 -> [_ _ _ _]
              tunnel: [errorcluster {"status"=TRUE, "code"=5007, "source"="Visualization PC"} ("error out") errorcluster {"status"=FALSE, "code"=0, "source"=""} ("error out") errorcluster {"status"=FALSE, "code"=0, "source"=""} ("error out") errorcluster {"status"=FALSE, "code"=0, "source"=""} ("error out")] -> w2883
              tunnel: [FALSE FALSE FALSE TRUE] -> w2877
              frame 0, Default {
                # "No video source available or default"
                n1318 = property on="Video Source" class="RadioBtnsControl (strict)"("DisabledEnum"=T11."Disabled and Grayed Out" ("Disabled")) -> ()  [unwired: 2 in, 2 out]
              }
              frame 1..3 {
                # "one or both camera available"
                n1319 = local write "Video Source"(enum32{"Camera", "FrameGrabber"}."Camera" ("Video Source")) -> ()
                n1320 = property on="Video Source" class="RadioBtnsControl (strict)"("DisabledEnum"=T11."Disabled and Grayed Out" ("Disabled")) -> ()  [unwired: 2 in, 2 out]
              }
              frame 4, 8, 12 {
                # "one or both frame grabber available"
                n1321 = local write "Video Source"(enum32{"Camera", "FrameGrabber"}."FrameGrabber" ("Video Source")) -> ()
                n1322 = property on="Video Source" class="RadioBtnsControl (strict)"("DisabledEnum"=T11."Disabled and Grayed Out" ("Disabled")) -> ()  [unwired: 2 in, 2 out]
              }
              frame 5..7, 9..11, 13..15 {
                n1323 = property on="Video Source" class="RadioBtnsControl (strict)"("DisabledEnum"=T11."Enabled" ("Disabled")) -> ()  [unwired: 2 in, 2 out]
              }
            }
            n1324 = Integer to Fixed-Point Cast(fixed-point type=fxp<+,4,4> 0.0, integer=w2882) -> (fixed-point=w2881:fxp<+,4,4>)
            n1325 = Number To Boolean Array(number=w2881) -> (Boolean array=w2879:bool[])
            n1326 = Reverse 1D Array(array=w2879) -> (reversed array=w2878:bool[])
            n1327 = Index Array(array=w2878, index=0) -> (element=w2888:bool)
            n1328 = Index Array(array=w2878, index=1) -> (element=w2886:bool)
            n1329 = Index Array(array=w2878, index=2) -> (element=w2887:bool)
            n1330 = Index Array(array=w2878, index=3) -> (element=w2885:bool)
          }
        }
        n1331 = Bundle By Name(cluster=w2868, "video source.Main Frame Grabber"=w2866, "video source.Side Frame Grabber"=w2865, "video source.Main Camera"=w2864, "video source.Side Camera"=w2863, "bothVidSourceAvail"=w2862) -> (w2867:T23)
        n1332 = call <vilib>:"Add State(s) to Queue__JKI_lib_State_Machine.vi"("State(s) in (\"\")"=w2874) -> ("States Out"=w2873:string)  [unwired: 14 in]
      }
      frame "TCP: SyncTime" {
        # "Template Separator\n(You can make a copy of, or modify, this frame)"
        n1333 = Unbundle By Name(w2916) -> ("System Status.TCP/IP"=w2915:bool)
        n1334 = case shown="True" w2915 {
          tunnel: w2917 -> [_ w2925]
          frame False {
          }
          frame True {
            n1335 = call "TcpIDFGV.vi"("Error In"=w2925, "action"=enum16{"write", "read"}."read") -> ("Error Out"=w2924:errorcluster, "connection ID out"=w2921:refnum<k5>)  [unwired: 8 in]
            n1336 = call <userlib>:"Tick Count (ms)__ogtk.vi"("error in (no error)"=w2924) -> ("error out"=w2923:errorcluster, "millisecond timer value"=w2922:u32)  [unwired: 9 in]
            n1337 = while {
              tunnel: w2923 -> [w2945]
              tunnel: w2921 -> [w2944]
              tunnel: w2922 -> [w2933]
              stop <- w2928 stop-if-true
              n1338 = Concatenate Strings("latencycheck" ("string"), "\r\n" ("End of Line Constant")) -> (w2940:string)
              n1339 = TCP Read(connection ID=w2944, bytes to read=512, error in (no error)=w2945, 7:T21."CRLF" ("mode (standard)"), 9:2000 ("timeout ms (25000)")) -> (connection ID out=w2937:refnum<k5>, data out=w2935:string, error out=w2927:errorcluster)
              n1340 = Tick Count (ms)() -> (millisecond timer value=w2934:u32)
              n1341 = Subtract(x=w2934, y=w2933) -> (x-y=w2932:u32)
              n1342 = Equal?(x=w2935, y=w2940) -> (x = y?=w2936:bool)
              n1343 = case shown="True" w2936 {
                tunnel: w2937 -> [_ w2958]
                tunnel: w2935 -> [w2950 _]
                tunnel: [w2946 FALSE] -> w2930
                tunnel: w2927 -> [_ w2952]
                frame False {
                  n1344 = Concatenate Strings("synctimer" ("string"), "\r\n" ("End of Line Constant")) -> (w2947:string)
                  n1345 = Equal?(x=w2950, y=w2947) -> (x = y?=w2946:bool)
                  "Sync Success?" <- w2946
                }
                frame True {
                  n1346 = Concatenate Strings("latencycheck:" ("string"), "\r\n" ("End of Line Constant")) -> (w2957:string)
                  n1347 = TCP Write(connection ID=w2958, data in=w2957, error in (no error)=w2952, 9:1000 ("timeout ms (25000)")) -> (error out=w2951:errorcluster)  [unwired: 2 out]
                  n1348 = call <vilib>:"Clear Errors.vi"("error in (no error)"=w2951) -> ()  [unwired: 5 in, 2 out]
                }
              }
              n1349 = Greater?(x=w2932, y=u32 10000 ("x-y")) -> (0:w2929:bool)
              n1350 = Or(x=w2930, y=w2929) -> (x .or. y?=w2928:bool)
            }
          }
        }
        n1351 = call <vilib>:"Add State(s) to Queue__JKI_lib_State_Machine.vi"("State(s) in (\"\")"=w2920) -> ("States Out"=w2919:string)  [unwired: 14 in]
      }
      frame "TCP: SendSettingMacro" {
        # "Template Separator\n(You can make a copy of, or modify, this frame)"
        n1352 = Unbundle By Name(w2962) -> ("System Status.TCP/IP"=w2961:bool)
        n1353 = case shown="True" w2961 {
          tunnel: ["" ("Empty String Constant") "TCP: sendSubjectID\nTCP: sendScaleBarSetting\nTCP: sendScaleMaxMin\nTCP: sendDeconChannel\nTCP: sendANSI\nTCP: sendRadius\nTCP: send3Dsetting\nTCP: sendFirefly\nTCP: sendPentero"] -> w2960
          frame False {
          }
          frame True {
          }
        }
        n1354 = call <vilib>:"Add State(s) to Queue__JKI_lib_State_Machine.vi"("State(s) in Front (\"\")"=w2960, "State(s) in (\"\")"=w2965) -> ("States Out"=w2964:string)  [unwired: 13 in]
      }
      frame "TCP: sendRunNum" {
        # "Send run number to AB PC\n(You can make a copy of, or modify, this frame)"
        n1355 = Unbundle By Name(w2972) -> ("System Status.TCP/IP"=w2969:bool, "IDs.RunID"=w2973:i8)
        n1356 = Increment(x=w2973) -> (x+1=w2968:i8)
        n1357 = case shown="True" w2969 {
          tunnel: w2968 -> [_ w2987]
          tunnel: [w2977 w2979] -> w2971
          tunnel: w2970 -> [w2977 w2978]
          frame False {
          }
          frame True {
            n1358 = Number To Decimal String(number=w2987, width (-)=i16 3) -> (decimal integer string=w2982:string)
            n1359 = call "TcpIDFGV.vi"("Error In"=w2978, "action"=enum16{"write", "read"}."read") -> ("Error Out"=w2980:errorcluster, "connection ID out"=w2984:refnum<k5>)  [unwired: 8 in]
            n1360 = Concatenate Strings("!run:", w2982) -> (w2981:string)
            n1361 = call "TCP_WriteRead.vi"("error in (no error)"=w2980, "data in"=w2981, "connectin ID in"=w2984) -> ("error out"=w2979:errorcluster)  [unwired: 4 in, 2 out]
          }
        }
        n1362 = call <vilib>:"Add State(s) to Queue__JKI_lib_State_Machine.vi"("State(s) in (\"\")"=w2976) -> ("States Out"=w2975:string)  [unwired: 14 in]
      }
      frame "TCP: sendVideoSource" {
        # "Send video source \n(You can make a copy of, or modify, this frame)"
        n1363 = Unbundle By Name(w2989) -> ("System Status.TCP/IP"=w2988:bool)
        n1364 = case shown="True" w2988 {
          tunnel: [w2995 w2997] -> w2991
          tunnel: w2990 -> [w2995 w2996]
          frame False {
          }
          frame True {
            n1365 = case shown="\"Camera\", Default" "Video Source" {
              tunnel: [0 1] -> w3002
              frame "Camera", Default {
              }
              frame "FrameGrabber" {
              }
            }
            n1366 = call "TcpIDFGV.vi"("Error In"=w2996, "action"=enum16{"write", "read"}."read") -> ("Error Out"=w2998:errorcluster, "connection ID out"=w3004:refnum<k5>)  [unwired: 8 in]
            n1367 = Number To Decimal String(number=w3002) -> (decimal integer string=w3000:string)  [unwired: 1 in]
            n1368 = Concatenate Strings("!invivo:" ("data in"), w3000) -> (w2999:string)
            n1369 = call "TCP_WriteRead.vi"("error in (no error)"=w2998, "data in"=w2999, "connectin ID in"=w3004) -> ("error out"=w2997:errorcluster)  [unwired: 4 in, 2 out]
          }
        }
        n1370 = call <vilib>:"Add State(s) to Queue__JKI_lib_State_Machine.vi"("State(s) in (\"\")"=w2994) -> ("States Out"=w2993:string)  [unwired: 14 in]
      }
      frame "TCP: startRun" {
        # "Template Separator\n(You can make a copy of, or modify, this frame)"
        n1371 = Unbundle By Name(w3009) -> ("System Status.TCP/IP"=w3008:bool)
        n1372 = case shown="True" w3008 {
          tunnel: [w3015 w3017] -> w3011
          tunnel: w3010 -> [w3015 w3016]
          frame False {
          }
          frame True {
            n1373 = call "TcpIDFGV.vi"("Error In"=w3016, "action"=enum16{"write", "read"}."read") -> ("Error Out"=w3018:errorcluster, "connection ID out"=w3019:refnum<k5>)  [unwired: 8 in]
            n1374 = call "TCP_WriteRead.vi"("error in (no error)"=w3018, "data in"="!acquire:1", "connectin ID in"=w3019) -> ("error out"=w3017:errorcluster)  [unwired: 4 in, 2 out]
          }
        }
        n1375 = call <vilib>:"Add State(s) to Queue__JKI_lib_State_Machine.vi"("State(s) in (\"\")"=w3014) -> ("States Out"=w3013:string)  [unwired: 14 in]
      }
      frame "TCP: stopRun" {
        # "Send stop run to AB PC\n(You can make a copy of, or modify, this frame)"
        n1376 = Unbundle By Name(w3023) -> ("System Status.TCP/IP"=w3022:bool)
        n1377 = case shown="True" w3022 {
          tunnel: [w3029 w3031] -> w3025
          tunnel: w3024 -> [w3029 w3030]
          frame False {
            # "if not connected, do nothing"
          }
          frame True {
            # "If TCP connected, send stop run"
            n1378 = call "TcpIDFGV.vi"("Error In"=w3030, "action"=enum16{"write", "read"}."read") -> ("Error Out"=w3032:errorcluster, "connection ID out"=w3034:refnum<k5>)  [unwired: 8 in]
            n1379 = call "TCP_WriteRead.vi"("error in (no error)"=w3032, "data in"="!acquire:0", "connectin ID in"=w3034) -> ("error out"=w3031:errorcluster)  [unwired: 4 in, 2 out]
          }
        }
        n1380 = call <vilib>:"Add State(s) to Queue__JKI_lib_State_Machine.vi"("State(s) in (\"\")"=w3028) -> ("States Out"=w3027:string)  [unwired: 14 in]
      }
      frame "TCP: CheckConnection" {
        # "Check TCP/IP connection statuse\n(If connection is lost, throw error)"
        n1381 = Unbundle By Name(w3037) -> ("System Status.TCP/IP"=w3036:bool)
        n1382 = case shown="False" w3036 {
          frame False {
          }
          frame True {
            # "If TCP/IP is true check, otherwise skip"
          }
        }
        n1383 = call <vilib>:"Add State(s) to Queue__JKI_lib_State_Machine.vi"("State(s) in (\"\")"=w3041) -> ("States Out"=w3040:string)  [unwired: 14 in]
      }
      frame "TCP: sendSubjectID" {
        # "Send subject ID"
        n1384 = Unbundle By Name(w3043) -> ("System Status.TCP/IP"=w3042:bool, "CaseID"=w3046:string)
        n1385 = case shown="True" w3042 {
          tunnel: w3046 -> [_ w3057]
          tunnel: [w3050 w3052] -> w3045
          tunnel: w3044 -> [w3050 w3051]
          frame False {
          }
          frame True {
            n1386 = call "TcpIDFGV.vi"("Error In"=w3051, "action"=enum16{"write", "read"}."read") -> ("Error Out"=w3053:errorcluster, "connection ID out"=w3055:refnum<k5>)  [unwired: 8 in]
            n1387 = Concatenate Strings("!subject:", w3057) -> (w3054:string)
            n1388 = call "TCP_WriteRead.vi"("error in (no error)"=w3053, "data in"=w3054, "connectin ID in"=w3055) -> ("error out"=w3052:errorcluster)  [unwired: 4 in, 2 out]
          }
        }
        n1389 = call <vilib>:"Add State(s) to Queue__JKI_lib_State_Machine.vi"("State(s) in (\"\")"=w3049) -> ("States Out"=w3048:string)  [unwired: 14 in]
      }
      frame "TCP: sendScaleBarSetting" {
        # "Template Separator\n(You can make a copy of, or modify, this frame)"
        n1390 = Unbundle By Name(w3061) -> ("System Status.TCP/IP"=w3059:bool, "VideoConfig.Scale Bar"=w3060:bool)
        n1391 = case shown="True" w3059 {
          tunnel: [w3067 w3076] -> w3063
          tunnel: w3062 -> [w3067 w3075]
          tunnel: w3060 -> [_ w3074]
          frame False {
          }
          frame True {
            n1392 = Boolean To (0,1)(Boolean=w3074) -> (0, 1=w3073:i16)
            n1393 = call "TcpIDFGV.vi"("Error In"=w3075, "action"=enum16{"write", "read"}."read") -> ("Error Out"=w3077:errorcluster, "connection ID out"=w3078:refnum<k5>)  [unwired: 8 in]
            n1394 = Number To Fractional String(number=w3073, width (-)=i16 1, precision (6)=i16 0) -> (F-format string=w3071:string)  [unwired: 1 in]
            n1395 = Concatenate Strings("!autocolor:" ("data in"), w3071) -> (w3069:string)
            n1396 = call "TCP_WriteRead.vi"("error in (no error)"=w3077, "data in"=w3069, "connectin ID in"=w3078) -> ("error out"=w3076:errorcluster)  [unwired: 4 in, 2 out]
          }
        }
        n1397 = call <vilib>:"Add State(s) to Queue__JKI_lib_State_Machine.vi"("State(s) in (\"\")"=w3066) -> ("States Out"=w3065:string)  [unwired: 14 in]
      }
      frame "TCP: sendScaleMaxMin" {
        # "Send scale bar max and min to AB PC\n(You can make a copy of, or modify, this frame)"
        n1398 = Unbundle By Name(w3083) -> ("System Status.TCP/IP"=w3080:bool, "VideoConfig.Scale Low"=w3082:dbl, "VideoConfig.Scale High"=w3081:dbl)
        n1399 = case shown="True" w3080 {
          tunnel: [w3089 w3102] -> w3085
          tunnel: w3084 -> [w3089 w3101]
          tunnel: w3082 -> [_ w3100]
          tunnel: w3081 -> [_ w3091]
          frame False {
          }
          frame True {
            n1400 = call "TcpIDFGV.vi"("Error In"=w3101, "action"=enum16{"write", "read"}."read") -> ("Error Out"=w3103:errorcluster, "connection ID out"=w3104:refnum<k5>)  [unwired: 8 in]
            n1401 = Number To Fractional String(number=w3100, width (-)=i16 4, precision (6)=i16 2) -> (F-format string=w3096:string)  [unwired: 1 in]
            n1402 = Number To Fractional String(number=w3091, width (-)=i16 4, precision (6)=i16 2) -> (F-format string=w3092:string)  [unwired: 1 in]
            n1403 = Concatenate Strings("!color:" ("string"), w3096, ";" ("string"), w3092) -> (w3090:string)
            n1404 = call "TCP_WriteRead.vi"("error in (no error)"=w3103, "data in"=w3090, "connectin ID in"=w3104) -> ("error out"=w3102:errorcluster)  [unwired: 4 in, 2 out]
          }
        }
        n1405 = call <vilib>:"Add State(s) to Queue__JKI_lib_State_Machine.vi"("State(s) in (\"\")"=w3088) -> ("States Out"=w3087:string)  [unwired: 14 in]
      }
      frame "TCP: sendDeconChannel" {
        # "Send Decon channel\n(You can make a copy of, or modify, this frame)"
        n1406 = Unbundle By Name(w3107) -> ("System Status.TCP/IP"=w3106:bool)
        n1407 = case shown="True" w3106 {
          tunnel: [w3113 w3118] -> w3109
          tunnel: w3108 -> [w3113 w3117]
          frame False {
          }
          frame True {
            n1408 = local read "Radio Buttons"() -> (w3116:T9)
            n1409 = Increment(x=w3116) -> (x+1=w3115:T9)
            n1410 = Number To Decimal String(number=w3115) -> (decimal integer string=w3114:string)  [unwired: 1 in]
            n1411 = call "TcpIDFGV.vi"("Error In"=w3117, "action"=enum16{"write", "read"}."read") -> ("Error Out"=w3119:errorcluster, "connection ID out"=w3122:refnum<k5>)  [unwired: 8 in]
            n1412 = Concatenate Strings("!channel:", w3114) -> (w3120:string)
            n1413 = call "TCP_WriteRead.vi"("error in (no error)"=w3119, "data in"=w3120, "connectin ID in"=w3122) -> ("error out"=w3118:errorcluster)  [unwired: 4 in, 2 out]
          }
        }
        n1414 = call <vilib>:"Add State(s) to Queue__JKI_lib_State_Machine.vi"("State(s) in (\"\")"=w3112) -> ("States Out"=w3111:string)  [unwired: 14 in]
      }
      frame "TCP: sendANSI" {
        # "Template Separator\n(You can make a copy of, or modify, this frame)"
        n1415 = Unbundle By Name(w3126) -> ("System Status.TCP/IP"=w3124:bool, "VideoConfig.ANSI"=w3125:dbl)
        n1416 = case shown="True" w3124 {
          tunnel: [w3132 w3138] -> w3128
          tunnel: w3127 -> [w3132 w3137]
          tunnel: w3125 -> [_ w3136]
          frame False {
          }
          frame True {
            n1417 = Number To Fractional String(number=w3136) -> (F-format string=w3134:string)  [unwired: 3 in]
            n1418 = call "TcpIDFGV.vi"("Error In"=w3137, "action"=enum16{"write", "read"}."read") -> ("Error Out"=w3139:errorcluster, "connection ID out"=w3140:refnum<k5>)  [unwired: 8 in]
            n1419 = Concatenate Strings("!ansi:" ("data in"), w3134) -> (w3133:string)
            n1420 = call "TCP_WriteRead.vi"("error in (no error)"=w3139, "data in"=w3133, "connectin ID in"=w3140) -> ("error out"=w3138:errorcluster)  [unwired: 4 in, 2 out]
          }
        }
        n1421 = call <vilib>:"Add State(s) to Queue__JKI_lib_State_Machine.vi"("State(s) in (\"\")"=w3131) -> ("States Out"=w3130:string)  [unwired: 14 in]
      }
      frame "TCP: sendRadius" {
        # "Send drawing radius to AB PC\n(You can make a copy of, or modify, this frame)"
        n1422 = Unbundle By Name(w3144) -> ("System Status.TCP/IP"=w3142:bool, "VideoConfig.Radius"=w3143:dbl)
        n1423 = case shown="True" w3142 {
          tunnel: [w3150 w3156] -> w3146
          tunnel: w3145 -> [w3150 w3155]
          tunnel: w3143 -> [_ w3154]
          frame False {
          }
          frame True {
            n1424 = Number To Fractional String(number=w3154) -> (F-format string=w3153:string)  [unwired: 3 in]
            n1425 = Concatenate Strings("!radius:" ("data in"), w3153) -> (w3151:string)
            n1426 = call "TcpIDFGV.vi"("Error In"=w3155, "action"=enum16{"write", "read"}."read") -> ("Error Out"=w3157:errorcluster, "connection ID out"=w3158:refnum<k5>)  [unwired: 8 in]
            n1427 = call "TCP_WriteRead.vi"("error in (no error)"=w3157, "data in"=w3151, "connectin ID in"=w3158) -> ("error out"=w3156:errorcluster)  [unwired: 4 in, 2 out]
          }
        }
        n1428 = call <vilib>:"Add State(s) to Queue__JKI_lib_State_Machine.vi"("State(s) in (\"\")"=w3149) -> ("States Out"=w3148:string)  [unwired: 14 in]
      }
      frame "TCP: send3Dsetting" {
        # "Send 3D setting to AB computer\n(You can make a copy of, or modify, this frame)"
        n1429 = Unbundle By Name(w3162) -> ("System Status.TCP/IP"=w3160:bool, "VideoConfig.3D?"=w3161:bool)
        n1430 = case shown="True" w3160 {
          tunnel: [w3168 w3175] -> w3164
          tunnel: w3163 -> [w3168 w3174]
          tunnel: w3161 -> [_ w3173]
          frame False {
          }
          frame True {
            n1431 = Boolean To (0,1)(Boolean=w3173) -> (0, 1=w3172:i16)
            n1432 = Number To Fractional String(number=w3172) -> (F-format string=w3171:string)  [unwired: 3 in]
            n1433 = call "TcpIDFGV.vi"("Error In"=w3174, "action"=enum16{"write", "read"}."read") -> ("Error Out"=w3176:errorcluster, "connection ID out"=w3177:refnum<k5>)  [unwired: 8 in]
            n1434 = Concatenate Strings("!3dset:" ("data in"), w3171) -> (w3169:string)
            n1435 = call "TCP_WriteRead.vi"("error in (no error)"=w3176, "data in"=w3169, "connectin ID in"=w3177) -> ("error out"=w3175:errorcluster)  [unwired: 4 in, 2 out]
          }
        }
        n1436 = call <vilib>:"Add State(s) to Queue__JKI_lib_State_Machine.vi"("State(s) in (\"\")"=w3167) -> ("States Out"=w3166:string)  [unwired: 14 in]
      }
      frame "TCP: sendFirefly" {
        # "Template Separator\n(You can make a copy of, or modify, this frame)"
        n1437 = Unbundle By Name(w3180) -> ("System Status.TCP/IP"=w3179:bool)
        n1438 = case shown="False" w3179 {
          tunnel: [w3186 w3188] -> w3182
          tunnel: w3181 -> [w3186 w3187]
          frame False {
          }
          frame True {
            n1439 = call "TcpIDFGV.vi"("Error In"=w3187, "action"=enum16{"write", "read"}."read") -> ("Error Out"=w3189:errorcluster, "connection ID out"=w3191:refnum<k5>)  [unwired: 8 in]
            n1440 = call "TCP_WriteRead.vi"("error in (no error)"=w3189, "data in"="!firefly:0", "connectin ID in"=w3191) -> ("error out"=w3188:errorcluster)  [unwired: 4 in, 2 out]
          }
        }
        n1441 = call <vilib>:"Add State(s) to Queue__JKI_lib_State_Machine.vi"("State(s) in (\"\")"=w3185) -> ("States Out"=w3184:string)  [unwired: 14 in]
      }
      frame "TCP: sendPentero" {
        # "Send Pentero setting to AB computer\n(You can make a copy of, or modify, this frame)"
        n1442 = Unbundle By Name(w3194) -> ("System Status.TCP/IP"=w3193:bool)
        n1443 = case shown="True" w3193 {
          tunnel: [w3200 w3202] -> w3196
          tunnel: w3195 -> [w3200 w3201]
          frame False {
          }
          frame True {
            n1444 = call "TcpIDFGV.vi"("Error In"=w3201, "action"=enum16{"write", "read"}."read") -> ("Error Out"=w3203:errorcluster, "connection ID out"=w3205:refnum<k5>)  [unwired: 8 in]
            n1445 = call "TCP_WriteRead.vi"("error in (no error)"=w3203, "data in"="!pentero:0", "connectin ID in"=w3205) -> ("error out"=w3202:errorcluster)  [unwired: 4 in, 2 out]
          }
        }
        n1446 = call <vilib>:"Add State(s) to Queue__JKI_lib_State_Machine.vi"("State(s) in (\"\")"=w3199) -> ("States Out"=w3198:string)  [unwired: 14 in]
      }
      frame "TCP: sendChannel" {
        # "Send DeCon Channel to AB computer\n()"
        n1447 = Unbundle By Name(w3208) -> ("System Status.TCP/IP"=w3207:bool)
        n1448 = case shown="True" w3207 {
          tunnel: [w3214 w3218] -> w3210
          tunnel: w3209 -> [w3214 w3217]
          frame False {
          }
          frame True {
            n1449 = local read "Radio Buttons"() -> (w3216:T9)
            n1450 = case shown="\"No Selection\", Default" w3216 {
              tunnel: ["" ("data in") "!channel:1" ("data in") "!channel:2" ("data in") "!channel:3" ("data in")] -> w3215
              frame "No Selection", Default {
              }
              frame "Ch1" {
              }
              frame "Ch2" {
              }
              frame "Ch3" {
              }
            }
            n1451 = call "TcpIDFGV.vi"("Error In"=w3217, "action"=enum16{"write", "read"}."read") -> ("Error Out"=w3219:errorcluster, "connection ID out"=w3220:refnum<k5>)  [unwired: 8 in]
            n1452 = call "TCP_WriteRead.vi"("error in (no error)"=w3219, "data in"=w3215, "connectin ID in"=w3220) -> ("error out"=w3218:errorcluster)  [unwired: 4 in, 2 out]
          }
        }
        n1453 = call <vilib>:"Add State(s) to Queue__JKI_lib_State_Machine.vi"("State(s) in (\"\")"=w3213) -> ("States Out"=w3212:string)  [unwired: 14 in]
      }
      frame "TCP: startCam" {
        # "Send Pentero setting to AB computer\n(You can make a copy of, or modify, this frame)"
        n1454 = Unbundle By Name(w3227) -> ("System Status.TCP/IP"=w3226:bool)
        n1455 = case shown="True" w3226 {
          tunnel: [w3233 w3235] -> w3229
          tunnel: w3228 -> [w3233 w3234]
          frame False {
          }
          frame True {
            n1456 = call "TcpIDFGV.vi"("Error In"=w3234, "action"=enum16{"write", "read"}."read") -> ("Error Out"=w3236:errorcluster, "connection ID out"=w3238:refnum<k5>)  [unwired: 8 in]
            n1457 = call "TCP_WriteRead.vi"("error in (no error)"=w3236, "data in"="!focus:1", "connectin ID in"=w3238) -> ("error out"=w3235:errorcluster)  [unwired: 4 in, 2 out]
          }
        }
        n1458 = call <vilib>:"Add State(s) to Queue__JKI_lib_State_Machine.vi"("State(s) in (\"\")"=w3232) -> ("States Out"=w3231:string)  [unwired: 14 in]
      }
      frame "TCP: stopCam" {
        # "Send Pentero setting to AB computer\n(You can make a copy of, or modify, this frame)"
        n1459 = Unbundle By Name(w3241) -> ("System Status.TCP/IP"=w3240:bool)
        n1460 = case shown="True" w3240 {
          tunnel: [w3247 w3249] -> w3243
          tunnel: w3242 -> [w3247 w3248]
          frame False {
          }
          frame True {
            n1461 = call "TcpIDFGV.vi"("Error In"=w3248, "action"=enum16{"write", "read"}."read") -> ("Error Out"=w3250:errorcluster, "connection ID out"=w3252:refnum<k5>)  [unwired: 8 in]
            n1462 = call "TCP_WriteRead.vi"("error in (no error)"=w3250, "data in"="!focus:0", "connectin ID in"=w3252) -> ("error out"=w3249:errorcluster)  [unwired: 4 in, 2 out]
          }
        }
        n1463 = call <vilib>:"Add State(s) to Queue__JKI_lib_State_Machine.vi"("State(s) in (\"\")"=w3246) -> ("States Out"=w3245:string)  [unwired: 14 in]
      }
      frame "TCP: Close" {
        # "Close TCP connection\n()"
        n1464 = Unbundle By Name(w3256) -> ("System Status.TCP/IP"=w3254:bool)
        n1465 = case shown="True" w3254 {
          tunnel: [w3262 w3264] -> w3257
          tunnel: w3255 -> [w3262 w3263]
          frame False {
          }
          frame True {
            n1466 = call "TcpIDFGV.vi"("Error In"=w3263, "action"=enum16{"write", "read"}."read") -> ("Error Out"=w3266:errorcluster, "connection ID out"=w3267:refnum<k5>)  [unwired: 8 in]
            n1467 = TCP Close Connection(connection ID=w3267, error in (no error)=w3266) -> (error out=w3264:errorcluster)  [unwired: 1 in, 1 out]
          }
        }
        n1468 = case shown="Error .." w3257 {
          tunnel: [w3270 w3271] -> w3258
          tunnel: w3256 -> [w3269 w3271]
          frame No Error {
            w3268 = FALSE ("System Status.TCP/IP")
            n1469 = Bundle By Name(cluster=w3269, "System Status.TCP/IP"=w3268) -> (w3270:T23)
            n1470 = global write "GlobalVariables.vi" "TCP connected?"(w3268) -> ()
          }
          frame Error {
          }
        }
        n1471 = call <vilib>:"Add State(s) to Queue__JKI_lib_State_Machine.vi"("State(s) in (\"\")"=w3261) -> ("States Out"=w3260:string)  [unwired: 14 in]
      }
      frame "---------- PID ----------" {
        # "Template Separator\n(You can make a copy of, or modify, this frame)"
        n1472 = call <vilib>:"Add State(s) to Queue__JKI_lib_State_Machine.vi"("State(s) in (\"\")"=w3276) -> ("States Out"=w3275:string)  [unwired: 14 in]
      }
      frame "PID: loadPID" {
        # "Template Separator\n(You can make a copy of, or modify, this frame)"
        n1473 = call "readPIDSetting.vi"("Error In"=w3280) -> ("Error Out"=w3281:errorcluster, "Ch3 PID out"=w3277:T8, "Ch2 PID out"=w3278:T8, "Ch1 PID out"=w3279:T8)  [unwired: 7 in]
        n1474 = local write "Ch1 PID gains"(w3279) -> ()
        n1475 = local write "Ch2 PID gains"(w3278) -> ()
        n1476 = local write "Ch3 PID gains"(w3277) -> ()
        n1477 = local write "Ch4 PID gains"(w3277) -> ()
        n1478 = call <vilib>:"Add State(s) to Queue__JKI_lib_State_Machine.vi"("State(s) in (\"\")"=w3285) -> ("States Out"=w3284:string)  [unwired: 14 in]
      }
      frame "---------- Temp ----------" {
        # "Template Separator\n(You can make a copy of, or modify, this frame)"
        n1479 = call <vilib>:"Add State(s) to Queue__JKI_lib_State_Machine.vi"("State(s) in (\"\")"=w3290) -> ("States Out"=w3289:string)  [unwired: 14 in]
      }
    }
    n1480 = Not(x=w80) -> (.not. x?=w79:bool)
    n1481 = local write "ML?"(w79) -> ()
    "ML?" <- TRUE ("main loop running?")
  }
  n1482 = while {
    tunnel: w19 -> [w3329]
    tunnel: w18 -> [w3324]
    tunnel: [w3323] -> w17
    tunnel: w13 -> [w3317]
    tunnel: [w3316] -> w16
    shift-right: [w3308] -> _
    shift-left: _ -> [w3309]
    stop <- w3304 stop-if-true
    # "Read data from notifier and deconvolve it and send to Aiming Beam computer"
    n1483 = Wait on Notification(notifier=w3329, ignore previous (F)=TRUE) -> (notification=w3328:T14, error out=w3320:errorcluster)  [unwired: 2 in, 2 out]
    n1484 = Wait Until Next ms Multiple(millisecond multiple=u32 10) -> ()  [unwired: 1 out]
    n1485 = Unbundle(w3328) -> ("idx"=w3294:i32, "CH1&2"=w3327:dbl[][], "CH3"=w3326:dbl[][], "V cluster"=w3312:cluster{"V1":dbl, "V2":dbl, "V3":dbl, "V4":dbl})
    n1486 = call <vilib>:"High Resolution Relative Seconds.vi"() -> ("relative seconds"=w3308:dbl)
    n1487 = call "SeperateChanData.vi"("Input (Ch1&2)"=w3327) -> ("Ch1"=w3300:dbl[][], "Ch2"=w3298:dbl[][])
    n1488 = call "SeperateChanData.vi"("Input (Ch1&2)"=w3326) -> ("Ch1"=w3296:dbl[][], "Ch2"=w3293:dbl[][])
    n1489 = Subtract(x=w3308, y=w3309) -> (x-y=w3311:dbl)
    n1490 = call "AvgArrayTimeCritical.vi"("2D array"=w3300) -> ("1D Avg"=w3299:dbl[])  [unwired: 10 in]
    n1491 = call "AvgArrayTimeCritical.vi"("2D array"=w3298) -> ("1D Avg"=w3297:dbl[])  [unwired: 10 in]
    n1492 = call "AvgArrayTimeCritical.vi"("2D array"=w3296) -> ("1D Avg"=w3295:dbl[])  [unwired: 10 in]
    n1493 = call "AvgArrayTimeCritical.vi"("2D array"=w3293) -> ("1D Avg"=w3292:dbl[])  [unwired: 10 in]
    n1494 = Multiply(x=w3311, y=1000.0) -> (x*y=→"Decon Loop timing (ms)":dbl)
    n1495 = case shown="\"Ch1\"" "Radio Buttons" {
      selector: "Radio Buttons" -> [_ w3342 w3356 w3371 w3388]
      tunnel: w3299 -> [w3339 w3350 w3362 w3376 w3392]
      tunnel: w3297 -> [w3337 w3347 w3364 w3374 w3390]
      tunnel: w3295 -> [w3335 w3345 w3359 w3379 w3382]
      tunnel: FALSE -> [_ w3353 w3367 w3381 w3395]
      tunnel: w3320 -> [w3333 w3352 w3366 w3370 w3387]
      tunnel: [w3333 w3351 w3365 w3380 w3394] -> w3304
      tunnel: [w3338 w3348 w3360 w3375 w3391] -> w3315
      tunnel: [w3336 w3346 w3361 w3373 w3389] -> w3314
      tunnel: [w3334 w3344 w3358 w3377 w3383] -> w3313
      tunnel: [0.0 ("lifetime (ns)") w3343 w3357 w3372 w3386] -> w3319
      tunnel: w3292 -> [w3331 w3341 w3355 w3369 w3385]
      tunnel: [w3330 w3340 w3354 w3368 w3384] -> w3291
      frame "No Selection", Default {
        n1496 = Build Array(w3339) -> (w3338:dbl[][])
        n1497 = Build Array(w3337) -> (w3336:dbl[][])
        n1498 = Build Array(w3335) -> (w3334:dbl[][])
        n1499 = Build Array(w3331) -> (w3330:dbl[][])
      }
      frame "Ch1" {
        n1500 = call "Deconvolution.vi"("DeconChannel"=w3342, "iRF align"=w3353, "error in (no error)"=w3352, "Waveform"=w3350) -> ("error out"=w3351:errorcluster, "lifetime (ns)"=w3343:dbl, "Fitting"=w3349:dbl[])  [unwired: 5 in]
        "Lifetime 1" <- w3343
        n1501 = Build Array(w3350, w3349) -> (w3348:dbl[][])
        n1502 = Build Array(w3347) -> (w3346:dbl[][])
        n1503 = Build Array(w3345) -> (w3344:dbl[][])
        n1504 = Build Array(w3341) -> (w3340:dbl[][])
      }
      frame "Ch2" {
        n1505 = call "Deconvolution.vi"("DeconChannel"=w3356, "iRF align"=w3367, "error in (no error)"=w3366, "Waveform"=w3364) -> ("error out"=w3365:errorcluster, "lifetime (ns)"=w3357:dbl, "Fitting"=w3363:dbl[])  [unwired: 5 in]
        "Lifetime 2" <- w3357
        n1506 = Build Array(w3362) -> (w3360:dbl[][])
        n1507 = Build Array(w3364, w3363) -> (w3361:dbl[][])
        n1508 = Build Array(w3359) -> (w3358:dbl[][])
        n1509 = Build Array(w3355) -> (w3354:dbl[][])
      }
      frame "Ch3" {
        n1510 = call "Deconvolution.vi"("DeconChannel"=w3371, "iRF align"=w3381, "error in (no error)"=w3370, "Waveform"=w3379) -> ("error out"=w3380:errorcluster, "lifetime (ns)"=w3372:dbl, "Fitting"=w3378:dbl[])  [unwired: 5 in]
        "Lifetime 3" <- w3372
        n1511 = Build Array(w3376) -> (w3375:dbl[][])
        n1512 = Build Array(w3374) -> (w3373:dbl[][])
        n1513 = Build Array(w3379, w3378) -> (w3377:dbl[][])
        n1514 = Build Array(w3369) -> (w3368:dbl[][])
      }
      frame "Ch4" {
        n1515 = call "Deconvolution.vi"("DeconChannel"=w3388, "iRF align"=w3395, "error in (no error)"=w3387, "Waveform"=w3385) -> ("error out"=w3394:errorcluster, "lifetime (ns)"=w3386:dbl, "Fitting"=w3393:dbl[])  [unwired: 5 in]
        "Lifetime 4" <- w3386
        n1516 = Build Array(w3392) -> (w3391:dbl[][])
        n1517 = Build Array(w3390) -> (w3389:dbl[][])
        n1518 = Build Array(w3385, w3393) -> (w3384:dbl[][])
        n1519 = Build Array(w3382) -> (w3383:dbl[][])
      }
    }
    n1520 = Bundle(w3315, w3314, w3313, w3291, "V cluster"=w3312) -> (w3318:T47)  [unwired: 1 in]
    n1521 = Bundle("idx"=w3294, "lifetime (ns)"=w3319) -> (w3325:cluster{"idx":i32, "lifetime (ns)":dbl})  [unwired: 1 in]
    n1522 = Send Notification(notification=w3318, notifier=w3317, error in (no error)=w3304) -> (notifier out=w3316:refnum<notifier>, error out=w3303:errorcluster)
    n1523 = Send Notification(notification=w3325, notifier=w3324, error in (no error)=w3304) -> (notifier out=w3323:refnum<notifier>, error out=w3302:errorcluster)
    n1524 = Merge Errors(w3303, w3302) -> (→"decon error out":errorcluster)
  }
  n1525 = while {
    tunnel: w18 -> [w3406]
    shift-right: [w3399] -> _
    shift-left: u32 0 -> [w3400]
    stop <- w3397 stop-if-true
    # "Send data to AB computer here"
    # "if TCP ip is not open loop will run once and stop. To re-establish connection and start this loop. Reboot softwrae."
    # "Data communication loop"
    n1526 = Tick Count (ms)() -> (millisecond timer value=w3399:u32)
    n1527 = Wait on Notification(notifier=w3406, ignore previous (F)=TRUE) -> (notification=w3404:cluster{"idx":i32, "lifetime":dbl}, error out=w3398:errorcluster)  [unwired: 2 in, 2 out]
    n1528 = Unbundle(w3404) -> ("idx"=w3403:i32, "lifetime"=w3402:dbl)
    n1529 = global read "GlobalVariables.vi" "TCP connected?"() -> (w3396:bool)
    n1530 = Subtract(x=w3399, y=w3400) -> (x-y=→"Communication loop(ms)":u32)
    n1531 = case shown="True" w3396 {
      tunnel: w3403 -> [_ w3415]
      tunnel: w3402 -> [_ w3414]
      tunnel: w3398 -> [w3407 w3411]
      tunnel: [w3407 w3408] -> w3397
      frame False {
      }
      frame True {
        n1532 = Number To Decimal String(number=w3415) -> (decimal integer string=w3423:string)  [unwired: 1 in]
        n1533 = call "TcpIDFGV.vi"("Error In"=w3411, "action"=enum16{"write", "read"}."read") -> ("Error Out"=w3410:errorcluster, "connection ID out"=w3421:refnum<k5>)  [unwired: 8 in]
        n1534 = Concatenate Strings("!idx:", w3423) -> (w3424:string)
        n1535 = call "TCP_WriteRead.vi"("error in (no error)"=w3410, "data in"=w3424, "connectin ID in"=w3421) -> ("error out"=w3409:errorcluster, "connectin ID out"=w3422:refnum<k5>)  [unwired: 4 in, 1 out]
        n1536 = Number To Fractional String(number=w3414, precision (6)=i16 2) -> (F-format string=w3413:string)  [unwired: 2 in]
        n1537 = Concatenate Strings("!lifetime:", w3413) -> (w3420:string)
        n1538 = call "TCP_WriteRead.vi"("error in (no error)"=w3409, "data in"=w3420, "connectin ID in"=w3422) -> ("error out"=w3408:errorcluster, "data out"=→"data out(communcation loop)":string)  [unwired: 4 in, 1 out]
      }
    }
  }
  n1539 = while {
    tunnel: w13 -> [w3435]
    shift-right: [w3426] -> _
    shift-left: w15 -> [w3433]
    shift-right: [w3428] -> _
    shift-left: w15 -> [w3427]
    i -> [w3429]
    stop <- w3430 stop-if-true
    # "Data display loop(30Hz)"
    n1540 = Wait on Notification(notifier=w3435, ignore previous (F)=FALSE) -> (notification=w3431:T13, error out=w3430:errorcluster)  [unwired: 2 in, 2 out]
    n1541 = Wait Until Next ms Multiple(millisecond multiple=u32 33) -> ()  [unwired: 1 out]
    n1542 = Tick Count (ms)() -> (millisecond timer value=w3426:u32)
    n1543 = Subtract(x=w3426, y=w3433) -> (x-y=→"display loop timing(ms)":u32)
    n1544 = case shown="No Error" w3430 {
      tunnel: w3431 -> [w3517 _]
      tunnel: w3427 -> [w3478 w3583]
      tunnel: [w3480 w3583] -> w3428
      tunnel: w3426 -> [w3477 _]
      frame No Error {
        w3454 = 0 ("index (row)")
        n1545 = Subtract(x=w3477, y=w3478) -> (x-y=w3479:u32)
        n1546 = Unbundle(w3517) -> ("CH1"=w3511:dbl[][], "CH2"=w3509:dbl[][], "CH3"=w3506:dbl[][], "CH4"=w3449:dbl[][], "Gain cluster"=w3455:cluster{"V1":dbl, "V2":dbl, "V3":dbl, "V4":dbl})
        n1547 = Unbundle By Name(w3455) -> ("V1"=w3473:dbl, "V2"=w3471:dbl, "V3"=w3469:dbl, "V4"=w3447:dbl)
        n1548 = Index Array(array=w3511, index (row)=w3454) -> (element=w3485:dbl[])  [unwired: 1 in]
        n1549 = Index Array(array=w3509, index (row)=w3454) -> (element=w3483:dbl[])  [unwired: 1 in]
        n1550 = Index Array(array=w3506, index (row)=w3454) -> (element=w3484:dbl[])  [unwired: 1 in]
        n1551 = Index Array(array=w3449, index (row)=w3454) -> (element=w3453:dbl[])  [unwired: 1 in]
        n1552 = call "RemoveDCBG.vi"("Channel"=enum16{"DC Only", "Ch1", "Ch2", "Ch3", "Ch4"}."Ch4", "WF in"=w3453) -> ("DC"=w3451:dbl, "WF out"=w3437:dbl[])  [unwired: 7 in, 1 out]
        n1553 = Greater?(x=w3479, y=u32 200) -> (0:w3481:bool)
        n1554 = call "CtrlVtoGain.vi"("CtrlV(V)"=w3447, "Channel"=enum16{"Ch1", "Ch2", "Ch3", "Ch4"}."Ch4") -> ("Gain"=w3436:dbl)  [unwired: 8 in, 1 out]
        n1555 = call "CtrlVtoGain.vi"("CtrlV(V)"=w3473, "Channel"=enum16{"Ch1", "Ch2", "Ch3"}."Ch1") -> ("Gain"=w3467:dbl)  [unwired: 8 in, 1 out]
        n1556 = call "RemoveDCBG.vi"("Channel"=enum16{"DC Only", "Ch1", "Ch2", "Ch3"}."Ch1", "WF in"=w3485) -> ("DC"=w3513:dbl, "WF out"=w3474:dbl[])  [unwired: 7 in, 1 out]
        n1557 = call "RemoveDCBG.vi"("Channel"=enum16{"DC Only", "Ch1", "Ch2", "Ch3"}."Ch2", "WF in"=w3483) -> ("DC"=w3508:dbl, "WF out"=w3475:dbl[])  [unwired: 7 in, 1 out]
        n1558 = call "CtrlVtoGain.vi"("CtrlV(V)"=w3471, "Channel"=enum16{"Ch1", "Ch2", "Ch3"}."Ch2") -> ("Gain"=w3462:dbl)  [unwired: 8 in, 1 out]
        n1559 = call "RemoveDCBG.vi"("Channel"=enum16{"DC Only", "Ch1", "Ch2", "Ch3"}."Ch3", "WF in"=w3484) -> ("DC"=w3505:dbl, "WF out"=w3476:dbl[])  [unwired: 7 in, 1 out]
        n1560 = call "CtrlVtoGain.vi"("CtrlV(V)"=w3469, "Channel"=enum16{"Ch1", "Ch2", "Ch3"}."Ch3") -> ("Gain"=w3458:dbl)  [unwired: 8 in, 1 out]
        n1561 = Add(x=w3437, y=w3451) -> (x+y=w3450:dbl[])
        n1562 = Less?(x=w3436, y=1.2) -> (x < y?=w3445:bool)
        n1563 = case shown="True" w3481 {
          tunnel: w3474 -> [_ w3544]
          tunnel: w3475 -> [_ w3547]
          tunnel: w3476 -> [_ w3546]
          tunnel: w3477 -> [_ w3562]
          tunnel: [w3526 w3562] -> w3480
          tunnel: w3478 -> [w3526 _]
          tunnel: w3467 -> [_ w3540]
          tunnel: w3462 -> [_ w3539]
          tunnel: w3458 -> [_ w3538]
          tunnel: w3437 -> [_ w3534]
          tunnel: w3436 -> [_ w3531]
          frame False {
          }
          frame True {
            n1564 = call "GetSNR(SubVI).vi"("Waveform"=w3544) -> ("SNR"=→"SNR1":dbl)  [unwired: 10 in]
            n1565 = Array Size(array=w3544) -> (size(s)=w3545:i32)
            n1566 = call "GetSNR(SubVI).vi"("Waveform"=w3547) -> ("SNR"=→"SNR2":dbl)  [unwired: 10 in]
            n1567 = call "GetSNR(SubVI).vi"("Waveform"=w3546) -> ("SNR"=→"SNR3":dbl)  [unwired: 10 in]
            n1568 = call "GetSNR(SubVI).vi"("Waveform"=w3534) -> ("SNR"=→"SNR4":dbl)  [unwired: 10 in]
            n1569 = global read "GlobalVariables.vi" "BG Idx2"() -> (w3533:i32)
            n1570 = Subtract(x=w3545, y=w3533) -> (x-y=w3532:i32)
            n1571 = Array Subset(array=w3544, index=w3533, length=w3532) -> (w3551:dbl[])
            n1572 = Array Subset(array=w3547, index=w3533, length=w3532) -> (w3553:dbl[])
            n1573 = Array Subset(array=w3546, index=w3533, length=w3532) -> (w3555:dbl[])
            n1574 = Array Subset(array=w3534, index=w3533, length=w3532) -> (w3535:dbl[])
            n1575 = Add Array Elements(numeric array=w3551) -> (sum=w3552:dbl)
            n1576 = Add Array Elements(numeric array=w3553) -> (sum=w3554:dbl)
            n1577 = Add Array Elements(numeric array=w3555) -> (sum=w3556:dbl)
            n1578 = Add Array Elements(numeric array=w3535) -> (sum=w3536:dbl)
            n1579 = Divide(x=w3552, y=w3540) -> (x/y=w3557:dbl)
            n1580 = Divide(x=w3554, y=w3539) -> (x/y=w3558:dbl)
            n1581 = Divide(x=w3556, y=w3538) -> (x/y=w3559:dbl)
            n1582 = Divide(x=w3536, y=w3531) -> (x/y=w3530:dbl)
            n1583 = Build Array(w3557, w3558, w3559, w3530) -> (w3560:dbl[])
            n1584 = Add Array Elements(numeric array=w3560) -> (sum=w3561:dbl)
            n1585 = Divide(x=w3560, y=w3561) -> (x/y=w3529:dbl[])
            n1586 = Index Array(array=w3529, index=2) -> (element=→"IntR3":dbl)
            n1587 = Index Array(array=w3529, index=1) -> (element=→"IntR2":dbl)
            n1588 = Index Array(array=w3529, index=0) -> (element=→"IntR1":dbl)
            n1589 = Index Array(array=w3529, index=4) -> (element=→"IntR4":dbl)
          }
        }
        n1590 = Add(x=w3474, y=w3513) -> (x+y=w3510:dbl[])
        n1591 = Add(x=w3475, y=w3508) -> (x+y=w3507:dbl[])
        n1592 = Add(x=w3476, y=w3505) -> (x+y=w3504:dbl[])
        n1593 = Less?(x=w3467, y=1.2 ("x")) -> (x < y?=w3465:bool)
        n1594 = Less?(x=w3462, y=1.2 ("x")) -> (x < y?=w3461:bool)
        n1595 = Less?(x=w3458, y=1.2 ("x")) -> (x < y?=w3457:bool)
        n1596 = case shown="False" w3457 {
          tunnel: [u32 16448250 ("Plot.Plot Color") u32 16711680 ("Plot.Plot Color")] -> w3456
          frame False {
          }
          frame True {
          }
        }
        n1597 = case shown="False" "Show BG removed?" {
          tunnel: w3511 -> [w3569 w3581]
          tunnel: w3510 -> [_ w3580]
          tunnel: [w3569 w3579] -> w3503
          tunnel: w3509 -> [w3568 w3578]
          tunnel: [w3568 w3577] -> w3497
          tunnel: w3507 -> [_ w3576]
          tunnel: w3506 -> [w3567 w3575]
          tunnel: [w3567 w3574] -> w3490
          tunnel: w3504 -> [_ w3573]
          tunnel: [w3566 w3572] -> w3443
          tunnel: w3450 -> [_ w3571]
          tunnel: w3449 -> [w3566 w3570]
          frame False {
          }
          frame True {
            n1598 = Build Array (concatenate)(w3575, w3573) -> (w3574:dbl[][])
            n1599 = Build Array (concatenate)(w3581, w3580) -> (w3579:dbl[][])
            n1600 = Build Array (concatenate)(w3578, w3576) -> (w3577:dbl[][])
            n1601 = Build Array (concatenate)(w3570, w3571) -> (w3572:dbl[][])
          }
        }
        "Channel 1" <- w3503
        "Channel 2" <- w3497
        "Channel 3" <- w3490
        "Channel 4" <- w3443
        n1602 = case shown="False" w3465 {
          tunnel: [u32 16448250 ("Plot.Plot Color") u32 16711680 ("Plot.Plot Color")] -> w3464
          frame False {
          }
          frame True {
          }
        }
        n1603 = case shown="False" w3461 {
          tunnel: [u32 16448250 ("Plot.Plot Color") u32 16711680 ("Plot.Plot Color")] -> w3460
          frame False {
          }
          frame True {
          }
        }
        n1604 = case shown="False" w3445 {
          tunnel: [u32 16448250 ("Plot.Plot Color") u32 16711680 ("Plot.Plot Color")] -> w3439
          frame False {
          }
          frame True {
          }
        }
        n1605 = Array Size(array=w3503) -> (size(s)=w3502:i32[])
        n1606 = Array Size(array=w3497) -> (size(s)=w3496:i32[])
        n1607 = Array Size(array=w3443) -> (size(s)=w3444:i32[])
        n1608 = Index Array(array=w3502) -> (element=w3501:i32)  [unwired: 1 in]
        n1609 = Index Array(array=w3496) -> (element=w3495:i32)  [unwired: 1 in]
        n1610 = Array Size(array=w3490) -> (size(s)=w3491:i32[])
        n1611 = Index Array(array=w3444) -> (element=w3438:i32)  [unwired: 1 in]
        n1612 = Index Array(array=w3491) -> (element=w3489:i32)  [unwired: 1 in]
        n1613 = property on="Channel 1" class="WFGraph (strict)"("Active Plot"=w3501, "Plot.Plot Color"=u32 16741120, "Plot.Line Style"=u8 1, "Plot.Line Width"=u8 2, "BG Color"=w3464) -> ()  [unwired: 2 in, 2 out]
        n1614 = property on="Channel 2" class="WFGraph (strict)"("Active Plot"=w3495, "Plot.Plot Color"=u32 16741120, "Plot.Line Style"=u8 1, "Plot.Line Width"=u8 2, "BG Color"=w3460) -> ()  [unwired: 2 in, 2 out]
        n1615 = property on="Channel 4" class="WFGraph (strict)"("Active Plot"=w3438, "Plot.Plot Color"=u32 16741120, "Plot.Line Style"=u8 1, "Plot.Line Width"=u8 2, "BG Color"=w3439) -> ()  [unwired: 2 in, 2 out]
        n1616 = property on="Channel 3" class="WFGraph (strict)"("Active Plot"=w3489, "Plot.Plot Color"=u32 16741120, "Plot.Line Style"=u8 1, "Plot.Line Width"=u8 2, "BG Color"=w3456) -> ()  [unwired: 2 in, 2 out]
      }
      frame Error {
        w3582 = u32 16448250 ("Plot Area:Colors:BG Color")
        n1617 = property on="Channel 1" class="WFGraph (strict)"("BG Color"=w3582) -> ()  [unwired: 2 in, 2 out]
        n1618 = property on="Channel 2" class="WFGraph (strict)"("BG Color"=w3582) -> ()  [unwired: 2 in, 2 out]
        n1619 = property on="Channel 3" class="WFGraph (strict)"("BG Color"=w3582) -> ()  [unwired: 2 in, 2 out]
      }
    }
    "DisplayLoop" <- w3429
  }
  n1620 = disable-structure "Diagram Disable Structure" shown="Disabled" {
    frame Disabled {
      w3584 = T48 {"Horizontal"=500, "Vertical"=100}  # Top Left Corner
      n1621 = Control Help Window(0:w3584, 1:TRUE ("Show")) -> ()
      n1622 = call <vilib>:"TDMS - File Viewer.vi"() -> ()  [unwired: 6 in, 2 out]
    }
    frame Enabled {
    }
  }
  n1623 = while {
    tunnel: w65 -> [w3598]
    tunnel: w55 -> [w3597]
    tunnel: [w3596] -> w63
    tunnel: w19 -> [w3595]
    tunnel: [w3594] -> w59
    tunnel: w39 -> [w3592]
    tunnel: w48 -> [w3591]
    tunnel: w35 -> [w3586]
    stop <- w3589 stop-if-true
    # "acquire data and send it to processing loop"
    # "Data Aquisition Loop"
    n1624 = event shown="[1] <Start digitizer>: User Event" {
      selector: w3597 -> [_ _]
      dyn-events: [_ _] -> w3596
      timeout: 20 -> [_ _]
      tunnel: w3598 -> [w3604 w3614]
      tunnel: [w3599 _] -> w3589
      tunnel: w3595 -> [w3603 w3621]
      tunnel: [w3603 w3620] -> w3594
      tunnel: w3592 -> [_ w3618]
      tunnel: w3591 -> [w3602 w3613]
      tunnel: w3586 -> [_ w3611]
      event Timeout {
        # "use queue to stop data loop\nwhen queue ref is released, error will stop this loop"
        n1625 = event-data() -> ()  [unwired: 1 in, 3 out]
        n1626 = Get Queue Status(queue=w3604) -> (error out=w3601:errorcluster)  [unwired: 2 in, 7 out]
        n1627 = Get Queue Status(queue=w3602) -> (error out=w3600:errorcluster)  [unwired: 2 in, 7 out]
        n1628 = Merge Errors(w3601, w3600) -> (w3599:errorcluster)
      }
      event User Event {
        w3619 = enum16{"Write", "Read"}."Read" ("Operation")
        n1629 = event-data() -> ("Time"=→"RunStartTime":u32)  [unwired: 1 in, 3 out]
        n1630 = call "FLImDAQ_FGV.vi"() -> ("Read data"=w3616:T6)  [unwired: 10 in, 1 out]
        n1631 = call "Digitizer1_FGV.vi"("Operation (Read)"=w3619) -> ("Read data"=w3610:refnum<k15>)  [unwired: 9 in, 1 out]
        n1632 = call "Digitizer2_FGV.vi"("Operation (Read)"=w3619) -> ("Read data"=w3617:refnum<k15>)  [unwired: 9 in, 1 out]
        n1633 = Unbundle By Name(w3616) -> ("Waveform to Avg"=w3615:i16)
        n1634 = property on="Property Node" class="niScope"(reference=w3610) -> (reference out=w3609:refnum<k15>, "Vertical Range"=w3608:dbl, "Vertical Offset"=w3607:dbl)  [unwired: 1 in, 1 out]
        n1635 = Tick Count (ms)() -> (millisecond timer value=w3606:u32)
        n1636 = while {
          tunnel: w3621 -> [w3681]
          tunnel: [w3680] -> w3620
          tunnel: w3617 -> [w3674]
          tunnel: w3609 -> [w3673]
          tunnel: w3618 -> [w3672]
          shift-right: [w3640] -> _
          shift-left: u32 0 ("millisecond timer value") -> [w3666]
          tunnel: w3615 -> [w3664]
          tunnel: w3614 -> [w3662]
          tunnel: w3613 -> [w3660]
          tunnel: w3611 -> [w3653]
          tunnel: w3608 -> [w3650]
          tunnel: w3607 -> [w3651]
          shift-right: [w3645] -> _
          shift-left: w3606 -> [w3644]
          i -> [w3636]
          stop <- w3643 stop-if-true
          w3632 = enum16{"write", "read"}."read" ("action")
          w3667 = 65536
          # "enqueue V"
          # "enqueue ch3 data"
          # "enqueue ch1&2 data"
          # "acquire ch3"
          # "acquire ch1&2"
          # "send data for processing"
          n1637 = Multiply(x=w3664, y=w3636) -> (x*y=w3629:i32)
          "Fetch Record #" <- w3629
          n1638 = property on="Property Node" class="niScope"(reference=w3673, "Fetch Record Number"=w3629) -> (reference out=w3685:refnum<k15>, error out=w3684:errorcluster, "Records Done"=w3652:i32)  [unwired: 1 in]
          n1639 = Subtract(x=w3652, y=w3629) -> (x-y=→"Record Backlog":i32)
          n1640 = call-poly <instrlib>:"niScope Fetch (poly).vi"("timeout"=0.25, "error in"=w3684, "channels"="0,1", "instrument handle"=w3685) -> ("error out"=w3626:errorcluster, "wfm"=w3627:i16[][], "wfm info"=w3649:T49)  [unwired: 4 in, 1 out]
          n1641 = property on="Property Node" class="niScope"(reference=w3674, "Fetch Record Number"=w3629) -> (reference out=w3678:refnum<k15>, error out=w3675:errorcluster, "Records Done"=w3630:i32)  [unwired: 1 in]
          n1642 = Divide(x=w3627, y=w3667) -> (x/y=w3639:dbl[][])
          n1643 = Tick Count (ms)() -> (millisecond timer value=w3640:u32)
          n1644 = Subtract(x=w3630, y=w3629) -> (x-y=→"Record Backlog 2":i32)
          n1645 = Subtract(x=w3640, y=w3666) -> (x-y=→"Aquisition loop timing(ms)":u32)
          n1646 = Subtract(x=w3640, y=w3644) -> (x-y=w3648:u32)
          n1647 = Multiply(x=w3639, y=w3650) -> (x*y=w3671:dbl[][])
          n1648 = call-poly <instrlib>:"niScope Fetch (poly).vi"("timeout"=0.25, "error in"=w3675, "channels"="0,1", "instrument handle"=w3678) -> ("error out"=w3625:errorcluster, "wfm"=w3668:i16[][])  [unwired: 4 in, 2 out]
          n1649 = Greater?(x=w3648, y=u32 1000) -> (0:w3646:bool)
          n1650 = Add(x=w3671, y=w3651) -> (x+y=w3661:dbl[][])
          n1651 = case shown="True" w3646 {
            tunnel: w3649 -> [_ w3694]
            tunnel: w3640 -> [_ w3693]
            tunnel: [w3687 w3693] -> w3645
            tunnel: w3644 -> [w3687 _]
            tunnel: [errorcluster {"status"=FALSE, "code"=0, "source"=""} ("error constant") w3690] -> w3641
            frame False {
            }
            frame True {
              # "[Covers: REQ29]"
              n1652 = call "CheckFrequency(SubVI).vi"("wfm info"=w3694) -> ("f (Hz)"=w3692:dbl)  [unwired: 10 in]
              "Laser f (Hz)" <- w3692
              n1653 = local read "Laser Rep Rate"() -> (w3689:dbl)
              n1654 = Increment(x=w3689) -> (x+1=w3688:dbl)
              n1655 = Greater?(x=w3692, y=w3688) -> (0:w3691:bool)
              n1656 = case shown="True" w3691 {
                tunnel: [errorcluster {"status"=FALSE, "code"=0, "source"=""} ("error constant") errorcluster {"status"=TRUE, "code"=0, "source"=""} ("error constant")] -> w3690
                frame False {
                }
                frame True {
                }
              }
            }
          }
          n1657 = Divide(x=w3668, y=w3667) -> (x/y=w3670:dbl[][])
          n1658 = Enqueue Element(queue=w3662, element=w3661, error in (no error)=w3626) -> (error out=w3624:errorcluster)  [unwired: 1 in, 2 out]
          n1659 = Multiply(x=w3670, y=w3650) -> (x*y=w3669:dbl[][])
          n1660 = Add(x=w3669, y=w3651) -> (x+y=w3659:dbl[][])
          n1661 = Enqueue Element(queue=w3660, element=w3659, error in (no error)=w3625) -> (error out=w3623:errorcluster)  [unwired: 1 in, 2 out]
          n1662 = Merge Errors(w3624, w3623) -> (w3622:errorcluster)
          n1663 = call "V1FGV.vi"("Error In"=w3622, "action (write)"=w3632) -> ("Error Out"=w3657:errorcluster, "V1 out"=w3655:dbl)  [unwired: 8 in]
          n1664 = call "V2FGV.vi"("Error In"=w3657, "action(write)"=w3632) -> ("Error Out"=w3656:errorcluster, "V2 out"=w3654:dbl)  [unwired: 8 in]
          n1665 = call "V3FGV.vi"("Error In"=w3656, "action(write)"=w3632) -> ("Error Out"=w3635:errorcluster, "V3 out"=w3634:dbl)  [unwired: 8 in]
          n1666 = call "V4FGV.vi"("Error In"=w3635, "action(write)"=w3632, "V3 in"=w3634) -> ("Error Out"=w3633:errorcluster, "V3 out"=w3631:dbl)  [unwired: 7 in]
          n1667 = Bundle("V1 out"=w3655, "V2 out"=w3654, "V3 out"=w3634, "V3 out"=w3631) -> (w3638:T50)  [unwired: 1 in]
          n1668 = Bundle(w3636, w3661, w3659, w3638) -> (w3663:T51)  [unwired: 1 in]
          n1669 = Enqueue Element(queue=w3653, element=w3638, error in (no error)=w3633) -> (error out=w3637:errorcluster)  [unwired: 1 in, 2 out]
          n1670 = Send Notification(notification=w3663, notifier=w3681, error in (no error)=w3637) -> (notifier out=w3680:refnum<notifier>, error out=w3642:errorcluster)
          n1671 = Merge Errors(w3641, w3642) -> (w3658:errorcluster)
          n1672 = case shown="Error .." w3658 {
            selector: w3658 -> [w3697 w3698]
            tunnel: w3672 -> [_ w3701]
            tunnel: [w3697 w3698] -> w3643
            frame No Error {
            }
            frame Error {
              # "Send user event to signal aquisition has stoped"
              n1673 = Generate User Event(priority (normal)=usereventprio."high priority", user event=w3701, event data cluster=TRUE ("event data")) -> ()  [unwired: 1 in, 2 out]
            }
          }
          "aquisition loop Error Out" <- w3643
          "Auisition Loop idx" <- w3636
        }
      }
    }
    n1674 = Unbundle By Name(w3589) -> ("status"=w3588:bool)
    n1675 = Not(x=w3588) -> (.not. x?=w3587:bool)
    n1676 = local write "Aq Loop?"(w3587) -> ()
    "Aq Loop?" <- TRUE ("Aq L?")
  }
  n1677 = while {
    tunnel: w19 -> [w3749]
    shift-right: [w3712] -> _
    shift-left: _ -> [w3745]
    tunnel: [w3703] -> w1 mode=indexing
    i -> [w3729]
    stop <- w3709 stop-if-true
    # "Channel 3"
    # "Channel 2"
    # "Channel 1"
    # "use FGV for gain value"
    # "stop on error"
    # "Gain adjustment and Data processing"
    n1678 = Tick Count (ms)() -> (millisecond timer value=w3712:u32)
    n1679 = Wait on Notification(notifier=w3749, ignore previous (F)=TRUE) -> (notification=w3723:T14, error out=w3702:errorcluster)  [unwired: 2 in, 2 out]
    n1680 = Subtract(x=w3712, y=w3745) -> (x-y=→"PID loop timing(ms)":u32)
    n1681 = Unbundle(w3723) -> ("CH1&2"=w3739:dbl[][], "CH3"=w3738:dbl[][])  [unwired: 2 out]
    n1682 = call "SeperateChanData.vi"("Input (Ch1&2)"=w3739) -> ("Ch1"=w3734:dbl[][], "Ch2"=w3732:dbl[][])
    n1683 = call "SeperateChanData.vi"("Input (Ch1&2)"=w3738) -> ("Ch1"=w3728:dbl[][], "Ch2"=w3721:dbl[][])
    n1684 = call "AvgArrayTimeCritical.vi"("2D array"=w3734) -> ("1D Avg"=w3733:dbl[])  [unwired: 10 in]
    n1685 = call "AvgArrayTimeCritical.vi"("2D array"=w3732) -> ("1D Avg"=w3743:dbl[])  [unwired: 10 in]
    n1686 = call "AvgArrayTimeCritical.vi"("2D array"=w3728) -> ("1D Avg"=w3740:dbl[])  [unwired: 10 in]
    n1687 = call "AvgArrayTimeCritical.vi"("2D array"=w3721) -> ("1D Avg"=w3720:dbl[])  [unwired: 10 in]
    n1688 = Array Max & Min(array=w3733) -> (max value=w3731:dbl)  [unwired: 3 out]
    n1689 = Array Max & Min(array=w3743) -> (max value=w3730:dbl)  [unwired: 3 out]
    n1690 = Array Max & Min(array=w3740) -> (max value=w3713:dbl)  [unwired: 3 out]
    n1691 = Array Max & Min(array=w3720) -> (max value=w3718:dbl)  [unwired: 3 out]
    n1692 = local read "Auto gain ch4"() -> (w3719:bool)
    n1693 = local read "Auto gain ch1"() -> (w3737:bool)
    n1694 = local read "Auto gain ch2"() -> (w3736:bool)
    n1695 = local read "Auto gain ch3"() -> (w3735:bool)
    n1696 = case shown="True" w3719 {
      tunnel: w3718 -> [_ w3796]
      tunnel: "V target(1.0)" -> [_ w3794]
      tunnel: [FALSE w3791] -> w3716
      tunnel: [0.0 ("CtrlV") w3786] -> w3717
      frame False {
        # "Manual control"
      }
      frame True {
        # "PID control"
        n1697 = global read "GlobalVariables.vi" "Ch4GainLim(Log)"() -> (w3797:cluster{"GainMax":dbl, "GainMin":dbl})
        n1698 = call-poly <vilib>:"PID.vi"("output range"=w3797, "PID gains"="Ch4 PID gains", "process variable"=w3796, "setpoint"=w3794) -> ("output"=w3795:dbl)  [unwired: 6 in, 1 out]
        n1699 = Power Of 10(x=w3795) -> (10^x=w3787:dbl)
        "Gain4" <- w3787
        n1700 = call "V4FGV.vi"("action(write)"=enum16{"write", "read"}."read") -> ("Error Out"=w3790:errorcluster, "V3 out"=w3792:dbl)  [unwired: 9 in]
        n1701 = call "GainToCtrlV.vi"("Gain"=w3787, "Channel"=enum16{"Ch1", "Ch2", "Ch3", "Ch4"}."Ch4") -> ("CtrlV"=w3786:dbl)  [unwired: 8 in, 1 out]
        n1702 = call "V4FGV.vi"("Error In"=w3790, "V3 in"=w3786) -> ()  [unwired: 8 in, 2 out]
        n1703 = local write "V 4"(w3786) -> ()
        n1704 = Not Equal?(x=w3786, y=w3792) -> (x != y?=w3791:bool)
      }
    }
    n1705 = case shown="True" w3737 {
      tunnel: "V target(1.0)" -> [_ w3811]
      tunnel: w3731 -> [_ w3808]
      tunnel: [0.0 ("CtrlV") w3800] -> w3710
      tunnel: [FALSE w3802] -> w3727
      frame False {
        # "Manual control"
      }
      frame True {
        # "PID control"
        n1706 = global read "GlobalVariables.vi" "Ch1GainLim(Log)"() -> (w3807:cluster{"GainMax":dbl, "GainMin":dbl})
        n1707 = call-poly <vilib>:"PID.vi"("output range"=w3807, "PID gains"="Ch1 PID gains", "process variable"=w3808, "setpoint"=w3811) -> ("output"=w3806:dbl)  [unwired: 6 in, 1 out]
        n1708 = Power Of 10(x=w3806) -> (10^x=w3805:dbl)
        "Gain1" <- w3805
        n1709 = call "V1FGV.vi"("action (write)"=enum16{"write", "read"}."read") -> ("Error Out"=w3801:errorcluster, "V1 out"=w3803:dbl)  [unwired: 9 in]
        n1710 = call "GainToCtrlV.vi"("Gain"=w3805, "Channel"=enum16{"Ch1", "Ch2", "Ch3"}."Ch1") -> ("CtrlV"=w3800:dbl)  [unwired: 8 in, 1 out]
        n1711 = local write "V 1"(w3800) -> ()
        n1712 = call "V1FGV.vi"("Error In"=w3801, "V1 in"=w3800) -> ()  [unwired: 8 in, 2 out]
        n1713 = Not Equal?(x=w3800, y=w3803) -> (x != y?=w3802:bool)
      }
    }
    n1714 = case shown="True" w3736 {
      tunnel: w3730 -> [_ w3838]
      tunnel: "V target(1.0)" -> [_ w3839]
      tunnel: [FALSE w3832] -> w3726
      tunnel: [0.0 ("CtrlV") w3828] -> w3722
      frame False {
        # "Manual control"
      }
      frame True {
        # "PID control"
        n1715 = global read "GlobalVariables.vi" "Ch2GainLim(Log)"() -> (w3836:cluster{"GainMax":dbl, "GainMin":dbl})
        n1716 = call-poly <vilib>:"PID.vi"("output range"=w3836, "PID gains"="Ch2 PID gains", "process variable"=w3838, "setpoint"=w3839) -> ("output"=w3835:dbl)  [unwired: 6 in, 1 out]
        n1717 = Power Of 10(x=w3835) -> (10^x=w3833:dbl)
        "Gain2" <- w3833
        n1718 = call "V2FGV.vi"("action(write)"=enum16{"write", "read"}."read") -> ("Error Out"=w3829:errorcluster, "V2 out"=w3830:dbl)  [unwired: 9 in]
        n1719 = call "GainToCtrlV.vi"("Gain"=w3833, "Channel"=enum16{"Ch1", "Ch2", "Ch3"}."Ch2") -> ("CtrlV"=w3828:dbl)  [unwired: 8 in, 1 out]
        n1720 = local write "V 2"(w3828) -> ()
        n1721 = call "V2FGV.vi"("Error In"=w3829, "V2 in"=w3828) -> ()  [unwired: 8 in, 2 out]
        n1722 = Not Equal?(x=w3828, y=w3830) -> (x != y?=w3832:bool)
      }
    }
    n1723 = case shown="True" w3735 {
      tunnel: w3713 -> [_ w3823]
      tunnel: "V target(1.0)" -> [_ w3820]
      tunnel: [FALSE w3816] -> w3725
      tunnel: [0.0 ("CtrlV") w3814] -> w3724
      frame False {
        # "Manual control"
      }
      frame True {
        # "PID control"
        n1724 = global read "GlobalVariables.vi" "Ch3GainLim(Log)"() -> (w3824:cluster{"GainMax":dbl, "GainMin":dbl})
        n1725 = call-poly <vilib>:"PID.vi"("output range"=w3824, "PID gains"="Ch3 PID gains", "process variable"=w3823, "setpoint"=w3820) -> ("output"=w3822:dbl)  [unwired: 6 in, 1 out]
        n1726 = Power Of 10(x=w3822) -> (10^x=w3819:dbl)
        "Gain3" <- w3819
        n1727 = call "V3FGV.vi"("action(write)"=enum16{"write", "read"}."read") -> ("Error Out"=w3815:errorcluster, "V3 out"=w3817:dbl)  [unwired: 9 in]
        n1728 = call "GainToCtrlV.vi"("Gain"=w3819, "Channel"=enum16{"Ch1", "Ch2", "Ch3"}."Ch3") -> ("CtrlV"=w3814:dbl)  [unwired: 8 in, 1 out]
        n1729 = local write "V 3"(w3814) -> ()
        n1730 = call "V3FGV.vi"("Error In"=w3815, "V3 in"=w3814) -> ()  [unwired: 8 in, 2 out]
        n1731 = Not Equal?(x=w3814, y=w3817) -> (x != y?=w3816:bool)
      }
    }
    n1732 = call "LabJack_FGV.vi"("Operation(Read)"=enum16{"Write", "Read"}."Read" ("Operation"), "error in (no error)"=w3702) -> ("error out"=w3711:errorcluster, "Read data"=w3747:i32)  [unwired: 8 in]
    n1733 = flat-sequence {
      tunnel: [w3751] -> w3708
      tunnel: w3702 -> [_]
      frame #0 {
        n1734 = Tick Count (ms)() -> (millisecond timer value=w3751:u32)
      }
    }
    n1735 = case "Channel 1" shown="True" w3727 {
      tunnel: w3711 -> [w3777 w3783]
      tunnel: w3747 -> [w3776 w3782]
      tunnel: [w3777 w3778] -> w3706
      tunnel: [w3776 w3781] -> w3742
      tunnel: w3710 -> [_ w3779]
      frame False {
        # "Do nothing"
      }
      frame True {
        # "request V\nupdate FGV"
        n1736 = global read "GlobalVariables.vi" "Ch1 LJ pin"() -> (w3780:string)
        n1737 = call "LJM_eWriteName.vi"("Handle In"=w3782, "Name"=w3780, "Value"=w3779, "error in"=w3783) -> ("Handle Out"=w3781:i32, "error out"=w3778:errorcluster)  [unwired: 10 in]
      }
    }
    n1738 = case "Channel 2" shown="True" w3726 {
      tunnel: w3706 -> [w3768 w3775]
      tunnel: [w3768 w3770] -> w3705
      tunnel: w3742 -> [w3769 w3774]
      tunnel: [w3769 w3773] -> w3741
      tunnel: w3722 -> [_ w3771]
      frame False {
        # "Do nothing"
      }
      frame True {
        # "request V\nupdate FGV"
        n1739 = global read "GlobalVariables.vi" "Ch2 LJ pin"() -> (w3772:string)
        n1740 = call "LJM_eWriteName.vi"("Handle In"=w3774, "Name"=w3772, "Value"=w3771, "error in"=w3775) -> ("Handle Out"=w3773:i32, "error out"=w3770:errorcluster)  [unwired: 10 in]
      }
    }
    n1741 = case "Channel 3" shown="True" w3725 {
      tunnel: w3705 -> [w3761 w3767]
      tunnel: [w3761 w3763] -> w3704
      tunnel: w3741 -> [w3760 w3766]
      tunnel: w3724 -> [_ w3764]
      tunnel: [w3760 w3762] -> w3715
      frame False {
        # "Do nothing"
      }
      frame True {
        # "request V\nupdate FGV"
        n1742 = global read "GlobalVariables.vi" "Ch3 LJ pin"() -> (w3765:string)
        n1743 = call "LJM_eWriteName.vi"("Handle In"=w3766, "Name"=w3765, "Value"=w3764, "error in"=w3767) -> ("Handle Out"=w3762:i32, "error out"=w3763:errorcluster)  [unwired: 10 in]
      }
    }
    n1744 = case "Channel 4" shown="True" w3716 {
      tunnel: w3704 -> [w3753 w3759]
      tunnel: w3715 -> [w3752 w3758]
      tunnel: [w3753 w3754] -> w3709
      tunnel: [w3752 w3757] -> _
      tunnel: w3717 -> [_ w3755]
      frame False {
        # "Do nothing"
      }
      frame True {
        # "request V\nupdate FGV"
        n1745 = global read "GlobalVariables.vi" "Ch4 LJ pin"() -> (w3756:string)
        n1746 = call "LJM_eWriteName.vi"("Handle In"=w3758, "Name"=w3756, "Value"=w3755, "error in"=w3759) -> ("Handle Out"=w3757:i32, "error out"=w3754:errorcluster)  [unwired: 10 in]
      }
    }
    "PID loop error out" <- w3709
    n1747 = flat-sequence {
      tunnel: [w3750] -> w3707
      tunnel: w3709 -> [_]
      frame #0 {
        n1748 = Tick Count (ms)() -> (millisecond timer value=w3750:u32)
      }
    }
    n1749 = Subtract(x=w3707, y=w3708) -> (x-y=w3703:u32)
    "LJ process (ms)" <- w3703
    "PID loop" <- w3729
  }
  "LJ time(ms)" <- w1
  n1750 = Release Notifier(notifier=w16, error in (no error)=w49) -> (error out=w50:errorcluster)  [unwired: 1 in, 2 out]
  n1751 = Release Notifier(notifier=w17, error in (no error)=w38) -> (error out=w43:errorcluster)  [unwired: 1 in, 2 out]
  n1752 = call <vilib>:"Simple Error Handler.vi"("error in (no error)"=w50) -> ()  [unwired: 4 in, 5 out]
  n1753 = call <vilib>:"Simple Error Handler.vi"("error in (no error)"=w43) -> ()  [unwired: 4 in, 5 out]
  n1754 = Unregister For Events(event registration refnum=w46, error in=w4) -> (error out=w52:errorcluster)
  n1755 = Destroy User Event(user event=w39, error in=w52) -> (error out=w3:errorcluster)
  n1756 = Close File(refnum=w21, error in=w3) -> ()  [unwired: 2 out]
  n1757 = Release Notifier(notifier=w59, error in (no error)=w58) -> (error out=w57:errorcluster)  [unwired: 1 in, 2 out]
  n1758 = Unregister For Events(event registration refnum=w63, error in=w61) -> (error out=w62:errorcluster)
  n1759 = call <vilib>:"Simple Error Handler.vi"("error in (no error)"=w57) -> ()  [unwired: 4 in, 5 out]
  n1760 = Destroy User Event(user event=w53, error in=w62) -> ()  [unwired: 1 out]
